vi "UHR-Fleezers Control (host) -Leonardo 04-2018 V6_DESTROY.vi"() -> ()   [LabVIEW 2013]
uses:
  <vilib>/Utility/miscctls.llb/LVPoint32TypeDef.ctl
  <vilib>/Utility/miscctls.llb/LVMinMaxIncTypeDef.ctl
  <vilib>/Platform/TimedLoop/XDataNode/timing_clust.ctl
  <vilib>/Platform/TimedLoop/XDataNode/nitl_modes.ctl
  <vilib>/Platform/TimedLoop/XDataNode/wakeup.ctl
  <vilib>/userdefined/High Color/nirio_resource_hc.ctl
  <vilib>/Analysis/baseanly.llb/Mean (DBL).vi
  FPGA VIs Alex/Alex subVIs/Downsample1D.vi
  FPGA VIs Alex/Alex subVIs/Integrate1D.vi
  <vilib>/FPGAPlugInAG/PCIe-7852R/niLvFpga_Open_PCIe-7852R.vi
  <vilib>/FPGAPlugInAG/PCIe-7852R/niLvFpga_Reset_PCIe-7852R.vi
  <vilib>/FPGAPlugInAG/PCIe-7852R/niLvFpga_Run_PCIe-7852R.vi
  <vilib>/FPGAPlugInAG/PCIe-7852R/niLvFpga_Close_PCIe-7852R.vi
  <vilib>/Utility/error.llb/Error Cluster From Error Code.vi
  <vilib>/rvi/errors/niLvFpgaAdjustHostInterfaceError.vi
  <vilib>/rvi/interface/common/niFpgaWaitOnOcc.vi
  downsample 1D array - double.vi
  <vilib>/express/express analysis/Spectral/Block/exnSpectralBlock spectral measurements PSD poly.vi
  <vilib>/express/express analysis/Spectral/Block/exnSpectralBlock spectral measurements PSD WFM.vi
  <vilib>/gmath/statdist.llb/Exp Random.vi
  <vilib>/gmath/statdist.llb/Gamma Random.vi
  <vilib>/FPGAPlugInAG/PCIe-7852R/niLvFpga_Abort_PCIe-7852R.vi
  openfpgaref.8.6.ctl
  <vilib>/Platform/TimedLoop/XDataNode/XDataNode.xnode
  <vilib>/rvi/interface/nirviOpenFPGA/nirviOpenFPGA.xnode
  openfpgaref.initrf.ctl
  FPGA Bitfiles/UHR-FleezersInst_FPGATarget_intitializeRF201804.lvbitx
  <vilib>/rvi/interface/nirviMethod/nirviMethod.xnode
  <vilib>/rvi/interface/nirviCloseFPGA/nirviCloseFPGA.xnode
  FPGA Bitfiles/UHR-FleezersInst_FPGATarget_UHR-FleezersCont_IqK95Pvv9lYv5.3.lvbitx
  <vilib>/rvi/interface/nirviReadWriteControl/nirviReadWriteControl.xnode
  <vilib>/express/express analysis/Spectral/XNode/ExpressSpectralMeasurementsBlockNode.xnode
  <vilib>/Platform/TimedLoop/XDataNode/XDNodeRunTimeDep.lvlib
  <vilib>/Analysis/NI_AALBase.lvlib
  <vilib>/rvi/errors/niLvFpgaMergeErrorWithErrorCode.vi
  <vilib>/gmath/NI_Gmath.lvlib
  <vilib>/FPGAPlugInAG/PCIe-7852R/niLvFpga_ConfigureFifo_PCIe-7852R.vi
  NiFpgaLv.dll
panel:
  in  "Reinit Valve?":bool=TRUE
  out "Data Period (s)":dbl=1.4999999999999999e-05 caption="Trap Data Period (s)" format="%#_6p"
  out "ideal setpoint fpga":dbl
  out "ideal setpoint avgd":dbl
  out "Step duration":dbl
  in  "Number of steps":i32
  out "Step taken":dbl
  in  "Distribution":enum16{"uniform", "Exponential", "Gamma2"}(ring)
  in  "Mean dwell time (s)":dbl=0.001 min=0.001
  in  "Backtrack probability":dbl min=0.0 max=1.0
  in  "Simulate stepping":bool
  in  "Step size (nm)":dbl min=0.0
  out "Actual setpoint":fxp<+/-,16,1> format="%.16g"
  in  "Target Force (pN)":dbl=10.5
  in  "MCL Tracking":bool
  out "Current Trap Delta":dbl=20.03845214843774
  in  "Set SP to Current Frc":bool
  out "Trap X (AI1)":T1={"Trap 1"=0.030792236328125, "Trap 2"=-0.011322021484375}
  in  "Trap Pos FB SP":fxp<+/-,16,1>=0.231353759765625 caption="Setpoint"
  in  "Trap Pos. FB ON":bool
  out "Extension":waveform(dbl)(graph)
  out "Action (%)":dbl(knob)=-100.0 scale=-100.0..100.0
  in  "Trap Pos. FB Out Scale 2^n":u8=23 caption="Action Scale"
  out "Location path":path=path "C:/Users/Fleezers/Desktop/UHR-Fleezers Instrument - Charlie/Locations.txt"
  in  "Location Matrix":string[][](array[string])=[["N.D.\r\n", "N.D.\r\n", "N.D.\r\n"], ["N.D.\r\n", "N.D.\r\n", "N.D.\r\n"], ["N.D.\r\n", "N.D.\r\n", "N.D.\r\n"], ["N.D.\r\n", "N.D.\r\n", "N.D.\r\n"]]
  in  "Tab Action Shortcuts":T2(tab)=enum."Calibration"
  in  "Use Full Offset?":bool=TRUE
  in  "Take Stepping Data":bool
  in  "Cap 1 Flow ON":bool=TRUE
  in  "Move Cap. 1 (DNA Top)":bool
  in  "Cal/Data Acq. Spot":bool
  in  "Cap 1 T ON":bool=TRUE
  in  "Cap 1 Samp Flow ON":bool=TRUE
  in  "Offset 2 Set":dbl=2.0
  in  "Offset 1 Set":dbl=1.0
  in  "Cal @ (MHz)":dbl=20.0
  in  "W/ Offset 1":bool=TRUE
  in  "Offset 1 Start (MHz)":dbl=13.0
  in  "W/ Offset 2":bool
  in  "Offset 2 Start (MHz)":dbl=16.0
  in  "Pause at Closest Delta (s)":dbl
  in  "Move to Delta 2 (MHz)":dbl=41.0
  in  "Attempt Limit":dbl=30.0 caption="Limit"
  out "Attempts":dbl=1.0
  in  "Wait Before Save (s)":u32=1
  in  "Fish for Tether":bool
  in  "Closest Delta (MHz)":dbl=13.0 step=0.25
  in  "Stop F (pN)":dbl=10.0
  in  "Then...":string(combo)="2"
  in  "Move to Delta 1 (MHz)":dbl=15.0
  in  "Tether Alarm?":bool=TRUE
  out "Tether":bool
  in  "Raster Set Upon Tether":u32=1
  in  "Save at end (5, 6)":bool
  in  "N Steps":dbl=20.0
  in  "Step Size (nm)":dbl=0.34
  in  "Save ave factor":dbl=1.0
  in  "APD to Watch":bool
  out "Duration (s)":dbl
  in  "Action":string(combo)="Yank"
  in  "Fl. Triggered...":bool
  in  "Fl. Delta Thresh. (kHz)":dbl=0.6
  out "Waiting":bool
  out "Fl. High":bool
  in  "Yank Delay (s)":dbl=3.5
  in  "Yank to Delta Array (MHz)":dbl[](array[numeric])=[16.3, 15.85, 14.85]
  in  "N Array El":u8=3 min=1 step=1
  in  "Random Choice":bool=TRUE
  in  "Force Yank":bool
  in  "Force Reset":bool
  in  "Toggle AFish":bool
  in  "Extend Min F":dbl=1.0
  in  "Extend Min TD":dbl=8.0
  in  "Extend dTD":dbl=5.0
  out "AF Time":u32
  in  "Wiggle time":dbl
  in  "Wiggle TD":dbl=1.0
  in  "Max TD":dbl=15.0
  in  "Min TD":dbl=8.0
  out "Fish Status":u16(ring) items=["Off", "Approach", "Wiggle", "Extend", "Tether Found"]
  in  "Approach dTD":dbl=-5.0 format="%#_13g"
  out "Messages":string="5:58 PM\tUHR-Fleezers ready.\r"
  in  "Stop All":bool=TRUE
  in  "Tab Control Display":T3(tab)
  out "Force-Extension":cluster{"Y":dbl[], "Y":dbl[]}(graph)
  in  "APD 2 Offset":dbl
  in  "APD 1 Offset":dbl
  out "Mean":dbl=1.039039384389187 caption="Mean (pN)" format="%#_3g"
  out "Force":waveform(dbl)[](graph)
  out "APD Chart":waveform(dbl)[](graph)
  in  "Calibration":u16(ring)=2 items=["None", "Position", "Force"]
  out "T1 X":dbl=-1.511158478291593 caption="T1 X (pN)" format="%0.2f"
  out "T2 X":dbl=0.5669202904867809 caption="T2 X (pN)" format="%0.2f"
  out "Difference":dbl=0.9442381878048121 caption="Difference (pN)" format="%.2g"
  in  "Ext Offset (nm)":dbl
  in  "Rescale on Mean":bool
  in  "Take Detection Laser\nImage":bool
  out "APD 2":T4(plugin-control) caption="APD 2 (Cy5)"
  in  "Flip Green Filter":bool
  in  "Set X Only":bool
  in  "Set Y Only":bool
  out "APD 1":T4(plugin-control) caption="APD 1 (Cy3)"
  out "Detection Laser Y":T4(plugin-control)
  out "Pointer Y (V)":dbl=4.0025870540482815 format="%_3g"
  out "Pointer X (V)":dbl=4.635613485356835 format="%_3g"
  in  "Set Confocal Spot (X-Y)":bool
  out "Detection Laser X":T4(plugin-control)
  out "All Signals":waveform(dbl)[](graph)=[{"t0"=timestamp(2751.0000000002074 s since 1904-01-01), "dt"=0.02, "Y"=[0.0, 0.0, 0.0, 0.0, 0.0, 0.0, 0.0, 0.0, 0.0, 0.0, 0.0, 0.0, 0.0, 0.0, 0.0], "attributes"=variant("NI_ChannelName"=variant(string "APD 1"))}, {"t0"=timestamp(2751.0000000002074 s since 1904-01-01), "dt"=0.02, "Y"=[0.0, 0.0, 0.0, 0.0, 0.0, 0.0, 0.0, 0.0, 0.0, 0.0, 0.0, 0.0, 0.0, 0.0, 0.0], "attributes"=variant("NI_ChannelName"=variant(string "APD 2"))}, {"t0"=timestamp(2751.0000000002074 s since 1904-01-01), "dt"=0.15, "Y"=[-0.020049210394969354, -0.02003592505550746], "attributes"=variant("NI_ChannelName"=variant(string "T1 Y"))}, {"t0"=timestamp(2751.0000000002074 s since 1904-01-01), "dt"=0.15, "Y"=[0.03074231675925172, 0.03074526419399293], "attributes"=variant("NI_ChannelName"=variant(string "T1 X"))}, {"t0"=timestamp(2751.0000000002074 s since 1904-01-01), "dt"=0.15, "Y"=[2.9160941496017294, 2.916128360850853], "attributes"=variant("NI_ChannelName"=variant(string "T1 Sum"))}, {"t0"=timestamp(2751.0000000002074 s since 1904-01-01), "dt"=0.15, "Y"=[-0.002644972968316131, -0.002638961391604115], "attributes"=variant("NI_ChannelName"=variant(string "T2 Y"))}, {"t0"=timestamp(2751.0000000002074 s since 1904-01-01), "dt"=0.15, "Y"=[-0.011335016186436862, -0.011341032214389745], "attributes"=variant("NI_ChannelName"=variant(string "T2 X"))}, {"t0"=timestamp(2751.0000000002074 s since 1904-01-01), "dt"=0.15, "Y"=[2.746599475081634, 2.746642933439132], "attributes"=variant("NI_ChannelName"=variant(string "T2 Sum"))}, {"t0"=timestamp(2751.0000000002074 s since 1904-01-01), "dt"=0.15, "Y"=[-0.526083166086966, -0.5261552546492463], "attributes"=variant("NI_ChannelName"=variant(string "T1 FB X"))}, {"t0"=timestamp(2751.0000000002074 s since 1904-01-01), "dt"=0.15, "Y"=[3.0920304879909737, 3.0920243537705665], "attributes"=variant("NI_ChannelName"=variant(string "T2 FB Sum"))}, {"t0"=timestamp(2751.0000000002074 s since 1904-01-01), "dt"=0.15, "Y"=[-0.7128125059590501, -0.7128388598091219], "attributes"=variant("NI_ChannelName"=variant(string "T2 FB X"))}, {"t0"=timestamp(2751.0000000002074 s since 1904-01-01), "dt"=0.15, "Y"=[2.9122738731040343, 2.91227808465834], "attributes"=variant("NI_ChannelName"=variant(string "T2 FB Sum"))}, {"t0"=timestamp(2751.0000000002074 s since 1904-01-01), "dt"=0.15, "Y"=[-0.0023344523453474137, -0.002339854121524665], "attributes"=variant("NI_ChannelName"=variant(string "PSD Y"))}, {"t0"=timestamp(2751.0000000002074 s since 1904-01-01), "dt"=0.15, "Y"=[-0.0026477858821374683, -0.002642139957884409], "attributes"=variant("NI_ChannelName"=variant(string "PSD X"))}, {"t0"=timestamp(2751.0000000002074 s since 1904-01-01), "dt"=0.15, "Y"=[0.014415417950986964, 0.014429639576402777], "attributes"=variant("NI_ChannelName"=variant(string "PSD Sum"))}]
  in  "Signals to Plot":i32(listbox)=9
  out "Trap Disp. Freq. (Hz)":dbl=6.666666666666667 caption="Freq. (Hz)" format="%#_6p"
  out "Display Period (s)":dbl=0.15 caption="Period (s)" format="%#_6p"
  in  "Trap Disp. Downsample":i32=10000 caption="Downsample" max=20000
  in  "APD Disp. Scale":dbl=0.1 caption="Scale (Divide,\nfor above plot only)"
  in  "APD Disp. dSamp":i32=2 caption="Integrate" min=1 max=30 step=1
  out "APD Display Freq. (Hz)":dbl=50.0 caption="Freq. (Hz)"
  out "APD Display Period (s)":dbl=0.02 caption="Period (s)"
  out "FFT 1":cluster{"f0":dbl, "df":dbl, "magnitude":dbl[]}[](graph)=[{"f0"=0.0, "df"=16.666666666666668, "magnitude"=[-331.1367572010275, -79.05506245821404, -86.61411242440559, -88.4728176091699, -90.3181253945935, -94.12566333707997, -92.52740723119955, -94.92192587982518, -99.60936585245742, -96.87568627870715, -94.02570383337763, -83.8058550151726, -97.57441397235512, -101.59968530846606, -101.523049255742, -103.35038532190343, -101.58594091014982, -102.96098031851216, -91.39759462745924, -103.75019963279499, -104.45030075054324, -103.04245334279298, -104.0720279134107, -106.06482372394834, -103.69131867828104, -104.40395035115309, -105.96420043276396, -107.6735556337804, -106.673030006608, -107.34889066208132, -108.05626565233933, -106.25659018850432, -105.29934513380842, -105.43096056709592, -108.3728498841465, -106.0555440144992, -105.78001282181421, -107.48741857324953, -108.67624970548897, -105.39976667156175, -105.91413119232612, -109.4222808198164, -107.0898971593174, -107.91164191890915, -108.26032038855709, -107.58332347164534, -108.23559688234297, -108.01271040303237, -107.66511723652701, -106.51901583170391, -109.27249501469946, -108.55647681594805, -107.93499259231463, -107.05068166453935, -109.13641475410455, -109.29679733781423, -108.19360835527803, -109.57747591546632, -109.58364591011674, -110.47061433372711, -109.8144340420426, -108.79067462293897, -107.54887553357234, -107.99559866705923, -108.85023923652685, -109.68733225238618, -108.51101278437793, -108.51620475114115, -108.22212402200637, -104.63726950302143, -110.2989919678048, -107.61796444414897, -108.68882962798736, -104.79193983043893, -103.59504263746938, -93.64633660288543, -101.9191640501395, -105.73717393151816, -108.92572458793902, -107.43962662800902, -107.79595323081325, -107.0923101993207, -108.17603277205289, -107.87074270713183, -109.20899066381877, -108.61832060412445, -109.10072003106593, -105.76480632823524, -108.60877649218978, -109.67541158970121, -110.2286232768028, -109.84952155309578, -109.33772024076384, -109.95251642394683, -110.14777282585466, -109.13825677905699, -110.05989365698167, -109.39359990189426, -110.56255614635295, -109.66477183197163, -108.9397158528824, -110.26529907650465, -109.20049464984628, -108.20183857013548, -109.09752250184418, -108.00440442238454, -108.35465963524055, -111.16774134451799, -110.34812550238405, -108.94506763426756, -108.72845542102493, -109.41512344014713, -112.44661664432377, -110.35437330889101, -111.32939440655925, -109.42989530434981, -110.98084669076195, -111.92160561143541, -108.57755551751093, -111.40042616180912, -110.15284955891853, -112.21455132279115, -111.40787773511747, -108.82949641635288, -110.13442122547907, -111.42229298204664, -112.06314940885191, -110.6015308813694, -109.51144097251623, -111.15989713761475, -110.25535755335385, -109.65868178057926, -110.51649885452997, -109.77194745285269, -108.4234206864394, -109.50892632093968, -109.46471287444389, -107.92241289271415, -109.72283805386196, -108.63426821579918, -110.37316681536255, -111.09713996884652, -110.32903619589223, -105.32012665515045, -107.36858557554393, -108.00382215905725, -110.06430686942338, -108.81666625979916, -110.01277074453823, -110.94194741225512, -109.65934609082873, -107.80979136006962, -112.81333866824724, -111.61474300955487, -109.83998277184975, -109.45953946904639, -109.79640584952526, -108.19172301667324, -109.28894656674316, -107.61471301278785, -108.83814006090513, -109.08866847726084, -108.20250571862371, -107.96222236861584, -107.03811197900873, -108.93533000393974, -107.74482548035408, -110.79811544577694, -111.1387476496877, -107.42970105883512, -109.18442281176472, -108.73546184641192, -108.71800246690864, -108.51945944378063, -108.06825856571285, -107.27210712368412, -108.12304695877637, -107.84933283677306, -109.73682373154998, -109.32284761503395, -109.31328817453769, -106.68762108642842, -109.79203616876461, -109.9020278896408, -110.27080024357275, -108.54152101558762, -111.00464391726017, -112.42244020766577, -110.82707315747889, -111.00344011890857, -109.90461839395674, -109.42877207451863, -109.73549298167016, -111.67494793393293, -108.85799077901427, -108.5348443278263, -109.803781083881, -108.30644755543659, -108.5079527456017, -111.2055351312823, -108.53089994340155, -108.01739789012176, -108.70360662855235, -107.95873456794631, -109.58297170693093, -108.9372401694271, -110.15921663527153, -109.22399119911955, -110.89883651739237, -108.92840112258382, -110.0545300523626, -109.05961065387005, -109.45831398589371, -108.61239387653227, -110.13001256174265, -108.80060224137931, -109.46327400696283, -108.0177965824709, -109.29727944627197, -110.3237255895986, -109.03258262543821, -110.97880178489321, -109.70034895077919, -111.16405638194153, -109.17324451464711, -109.65698250854277, -108.96750235822178, -112.00534231585624, -108.69274607723942, -108.98110446396657, -108.40723795464795, -111.44459094807324, -111.74799245277113, -111.1601960491512, -108.92048232753773, -110.30506377784799, -111.33145973979093, -110.91850998672503, -110.33684985776448, -108.90206518366908, -109.28458878227542, -108.98773986023751, -110.85813863075646, -109.00041591105906, -110.84543686681204, -109.84382395806176, -109.69722434763266, -108.50915601095721, -107.80829925826895, -110.59736107582401, -109.75377770317087, -109.3992084496136, -110.51151565846742, -112.49753959826434, -109.7299632589479, -109.54070743868353, -109.90314341132164, -111.05974202976806, -109.03766862152392, -109.46667095459878, -109.52800799036197, -111.3163121356807, -110.07817134522178, -108.69251657453547, -109.40472158898045, -109.71400709815576, -110.60534468715097, -109.46937396724682, -107.70342491418788, -109.86331122597839, -108.64971387994616, -110.90117371097081, -108.34928840565928, -110.04172889660904, -111.52979926554961, -110.34759300823305, -109.62712781837159, -109.24131154553284, -110.23196152450447, -108.68509612326807, -108.0246905483419, -106.61876139289784, -101.5519630114271, -80.57695480953835, -102.03744443354402, -107.1449217193017, -110.0695213407169, -106.61597783999268, -110.79221011808191, -109.58974545931426, -109.1149802216988, -109.20993813088597, -109.63768480465863, -110.10428394219181, -109.08445084271477, -108.83472375362581, -109.69508502050168, -108.05588796178941, -110.62586360101581, -109.95315261676905, -107.52208264977473, -108.80708007514875, -110.43484881098874, -110.45942171588936, -107.83804717866751, -109.98973910294193, -109.3496496054193, -108.425252911127, -110.94579264380809, -108.54181722177951, -108.67696070083541, -108.4150202151644, -109.24973583101504, -112.0454922608961, -111.29046597340738, -110.75018248960077, -109.38326363603683, -109.2033340336957, -109.45076170874889, -109.52878049853727, -109.32340869724774, -110.98123395128233, -110.75736340635505, -109.7218385823809, -107.97422606064993, -109.77313701758703, -110.95948744392717, -110.08996774172691, -108.51011830110778, -109.78063140243836, -110.65996628628228, -109.83684298615616, -110.33329049188029, -110.13755118968292, -110.3717925645783, -108.55302219178951, -106.86811628734195, -108.6302156589162, -108.75341391045045, -108.32589578384841, -108.70061474734084, -112.30742263527534, -109.16842570592085, -109.29767035534508, -108.87829025017463, -108.2255616391397, -108.4316108616088, -108.82995906929271, -110.40135575415563, -109.51623498946435, -109.79409808792403, -107.03832759632121, -108.36534528684132, -109.72010868372905, -107.90933028179892, -106.95643597294047, -111.29929166165778, -110.23001135794706, -108.98838015381585, -109.79115357104436, -108.18627479511115, -108.14988122174307, -109.12074063466532, -109.41904850488358, -111.40409873721113, -108.83156790193294, -108.77032248953847, -108.88363158686694, -108.47515048290681, -105.94172147874599, -109.38146940214403, -109.21277078848794, -108.11309390545507, -110.70840012427504, -109.5504457849329, -109.52330684534209, -110.06776026911132, -108.21949434182314, -111.21266686269992, -108.78581501170974, -108.43115799297222, -109.63260325780062, -109.84070220619535, -109.72041980780126, -110.29615941882527, -110.60316734262464, -108.79165446414692, -110.95840439895592, -109.64926233107009, -109.16526769544322, -108.65292362430982, -109.56113898129935, -109.85693046339026, -108.92316027325207, -109.79492493553914, -109.38157962945887, -110.24545136266825, -109.30031463492487, -109.0795429936869, -111.4091719525013, -108.63499083917162, -108.43863465339358, -109.23207864880891, -111.21947487191643, -109.24525201480154, -109.56842406077318, -109.46711940800672, -111.91389548262572, -108.15655736690546, -108.71882059966947, -111.26328503478568, -110.95027143873176, -108.4853106242357, -110.36902802777546, -109.9314203579182, -108.77686164101732, -108.71871020068312, -111.04829661168574, -109.95072655339462, -109.88221342875462, -109.53241732756136, -108.2625005404823, -108.00677030040697, -110.19659317581693, -108.93858924796267, -109.46817875483995, -110.78063992017232, -111.11066570318451, -110.78774336696706, -109.19199744617812, -108.54914256407436, -109.28414960420909, -110.64143585101183, -110.5855350821307, -109.47578632252726, -108.89705360836223, -109.89214013612292, -107.93271261027171, -109.32631601340563, -108.60274611341092, -109.40110159872573, -110.889237682208, -110.01391165813328, -109.99747108785071, -108.65542819213674, -110.37211847668736, -110.44656500845738, -110.8128133834973, -108.8909299260433, -110.19551227077532, -111.37647266643523, -110.83802189730321, -109.98519377913681, -110.52378970770522, -108.16970420057817, -110.70974729773344, -110.76836765494402, -110.26884275594577, -109.22041044268806, -109.87809744746195, -107.76823252107832, -109.12119474042969, -110.28066108731146, -108.55000033509207, -110.18152097767907, -110.73030521152278, -111.49470908029893, -110.2320929919509, -110.03370979233021, -109.79181668155233, -108.6673501209991, -109.86695766650877, -107.88926518046961, -110.95525003776572, -109.18130359755742, -110.42618009658618, -107.90341931158893, -111.44736855661769, -110.72634267386593, -109.29945988519303, -107.67889101961411, -108.81148059987765, -109.13375212757057, -109.8122873383549, -109.80176697684155, -109.96342275204768, -109.90406635707086, -108.75674342748256, -110.12362902701081, -109.82151095527837, -108.62543344241836, -110.09171852771195, -110.21434637862887, -109.97254504855631, -109.27043209093468, -111.35149588204125, -110.12399876776051, -111.65983675538546, -109.28788875768564, -110.86554069990251, -111.26990906470603, -108.60956517491746, -111.49613890850938, -111.79685722966795, -109.26269485364045, -110.38555615546439, -109.40641023162068, -110.966136593156, -108.78892524584494, -110.29340727375603, -111.44032043281035, -109.95212021173755, -109.79233511584334, -112.41184021118175, -109.73687851881148, -108.65493879781806, -110.76132988919045, -108.43230346094671, -110.32968175895853, -110.29890782023821, -108.77609076424456, -110.3298662333555, -109.47734504217333, -108.2677295732245, -109.21234363352882, -107.83278941978479, -108.85136784424789, -108.43241251530755, -109.76609391460555, -108.53204373005357, -110.9660641972934, -110.3152512161094, -110.72570499399905, -109.23877906286317, -111.72407743101837, -109.20311421918561, -108.06021800233717, -109.29288625761943, -108.78395253409145, -111.85250172876302, -108.78827588901797, -109.79775055719482, -109.12089297455859, -109.49896359356035, -110.34432647103819, -107.94700097960238, -109.30489238477631, -108.89170290869342, -108.82574563272509, -110.11024077194833, -107.37946433552314, -109.60167933458756, -107.80625057819019, -110.11489057210264, -107.35436859378505, -105.69819484613895, -109.11280625683739, -109.27770293057978, -107.7053735252589, -109.75022444894368, -109.3310543596577, -107.87683693707739, -108.19931495338068, -109.26462246191564, -106.71885779297867, -100.00018022217961, -92.54434511397295, -107.20472143807373, -107.39203415155283, -110.04461177268398, -108.48860496315312, -109.0057168110333, -108.37627790492552, -108.4108380728248, -109.65509454313073, -109.64243000632982, -97.04219069306761, -109.0928856629964, -107.9760697315632, -107.52611064047497, -108.87702814778996, -109.08437599027614, -110.70097118837974, -109.00969860961283, -110.38275386163214, -110.0699155421545, -106.91498895181175, -106.22178738309017, -109.36827866896039, -107.59953130968307, -109.19516217272808, -108.31502495393616, -109.384158926223, -107.11670654202719, -108.09436312738853, -110.14559230873704, -109.84997663447679, -107.83465335309926, -108.60947100624459, -108.9932479423645, -109.17174810371898, -108.79457339828916, -109.40909327982367, -109.6328723628302, -109.51081854476179, -107.63054408568418, -109.63728404010122, -108.51163794839918, -107.55002282725216, -108.97796212764939, -107.24648164623483, -112.21470452291085, -108.74294024554423, -109.62070777514892, -108.05768666239368, -109.8224946685739, -109.34575507446003, -108.53536952609525, -109.60789300457671, -107.56681538208278, -109.22777325016398, -108.79047910308894, -110.10332477250668, -108.00206387955672, -108.45604004720035, -109.00645795765472, -109.81039564269616, -108.92785144634745, -108.3978471520567, -107.94411095685999, -110.53486519304262, -108.8773780319227, -109.03345093296107, -107.30746693745031, -108.54277704832029, -108.77629108166091, -108.91111762599647, -107.74965195880401, -109.97375370738439, -109.76326492689246, -107.91717581777407, -109.0730556927617, -107.66804873204664, -110.40438871064791, -108.05794247751498, -108.80206615156494, -107.51329354700796, -108.83687012994949, -107.57713176895379, -107.94774159581414, -109.41894615439651, -107.10869425078764, -110.51480854078629, -108.92221367099775, -109.91358786461535, -110.1744263092835, -109.30795472883494, -107.91359710691006, -109.77888185049835, -109.52060975706438, -108.66686651982212, -108.71041801553639, -110.13619546359467, -108.87957097273856, -109.72150387215271, -109.00776068810654, -109.70251113927438, -110.75769213896399, -108.53234896741436, -109.69439526582246, -110.15412541604617, -108.25183374628219, -107.97402569656481, -110.34920156998648, -108.45106995186384, -108.82031145748209, -111.38690005057539, -107.01968459818563, -110.3044500039584, -110.8755481852125, -111.08915057663255, -107.94824988655199, -110.21669144934839, -109.90539774633154, -109.58985438756767, -110.12258796623348, -109.41689951612143, -109.31128210476795, -109.00258476567323, -109.11093063041056, -108.83347064311234, -108.32685287566952, -109.44770946560935, -108.40145063144861, -109.68448193892085, -108.76525439243828, -107.62837139034596, -107.39300298848994, -109.36993934990318, -109.2465218489418, -106.66307369796812, -110.15891092764934, -109.57151745419041, -108.92425698310808, -109.8036704717834, -108.79751146756549, -109.25926431818017, -108.46260574057584, -109.1967554647261, -110.63319560262356, -109.02343067385144, -111.22073171487528, -109.4731095097105, -109.69335000085164, -109.48782989577005, -107.95204227683271, -108.19468255763758, -111.36195112053247, -109.55696116543685, -110.3130767640534, -108.9621824253354, -109.99735074896789, -109.20198058456344, -108.12100614259485, -111.27227490807289, -110.09248554008288, -109.14395535060149, -110.80882692379708, -109.22632926901655, -108.64497210802793, -111.00030482190711, -111.1317849358033, -107.43140429257826, -107.9783302193555, -109.2639893652291, -108.97008485446163, -108.66556668859064, -108.12995785876932, -109.73001061107855, -108.09691302413727, -110.68391499215569, -112.78583642012705, -108.7093037763389, -110.67868795924797, -109.0190959349128, -108.36247198231372, -109.82829353258869, -108.24916379311045, -109.84154533905823, -108.55470160833775, -109.75438989348815, -108.82865632118325, -107.63622268162582, -111.00943492886312, -110.81824358463759, -109.46028423652966, -107.52479398900992, -108.99087806823736, -109.94494831750349, -110.26788355564504, -109.8954055022304, -106.9478122391182, -108.91705388158901, -107.76095584490312, -109.28456723055147, -109.7982307261767, -108.98552661346622, -109.98937979783426, -110.57907422426224, -108.68113463944836, -108.06257240208589, -110.0707224529617, -109.19515280354733, -109.35868842818849, -110.37311467065695, -109.0404734478992, -108.16686395270187, -108.61859220485148, -109.19986437876149, -108.19707189725302, -110.06564239663074, -108.87850403465154, -110.63824157544798, -107.36918104067212, -108.7008736325543, -110.9359398265406, -111.08529123080929, -108.44209934821818, -109.79529621208783, -108.38917887958179, -108.169117639508, -109.24332926356216, -110.50584058811704, -109.63592524002665, -109.32261039377495, -109.16720880524552, -109.3084314664462, -109.5812223978583, -107.70213196487856, -108.0557884982431, -110.67058020007828, -111.68459781023608, -109.66270627185824, -110.52536245663693, -109.70208409132103, -108.78645420809342, -109.23122088059863, -109.24601474121832, -111.25604763816514, -109.50225851581177, -107.32434217163818, -109.28548556764925, -107.59972621660836, -110.46928774723048, -109.25950101547609, -110.32016453935465, -107.78482761561703, -107.89462895091089, -107.51366154391481, -108.08036891159172, -109.53371809947035, -101.2452927166745, -109.32763325689056, -107.52166868423687, -109.89648659445174, -109.11350200980485, -109.81336712738089, -110.02799517445062, -108.02767143538516, -107.97850220501483, -109.50772934896838, -109.31069875721964, -108.49991657749598, -105.60880911233095, -109.79128597340213, -106.91084537903113, -107.84880087118997, -109.63628170511824, -109.03203967193224, -110.64186113413658, -110.98027990365594, -112.33841002907062, -111.01793075565425, -108.58025797022215, -110.4259296883756, -110.38643255981424, -108.93051671115133, -110.97544177116494, -108.63883100482677, -108.37581711765226, -108.90240163126536, -107.94688047875466, -109.9482937437732, -110.09097112364414, -110.09805032265376, -111.44307114024532, -109.15483789122554, -110.9713708217832, -107.8548737634672, -111.41418477109195, -109.45699779859628, -97.03595099331734, -109.16746744169623, -109.66209204485918, -112.57048704774604, -109.73989735035725, -108.16252575067017, -110.7546980664636, -108.91536673403449, -109.20509151422344, -111.0260632167785, -109.62924582406518, -110.45466277291722, -110.2973970018937, -109.67550222925419, -108.84481022020094, -107.23686414357573, -111.79004633370906, -109.85453094194085, -109.45617270081004, -110.73920606732504, -108.90879956851099, -109.67774425528265, -109.4745715721361, -110.18080454693559, -109.26079184315502, -109.41692499885505, -109.02240975088358, -107.80833423058168, -109.32657361431549, -107.87138278655101, -110.910364670719, -109.70067156846706, -108.55301754282077, -109.4243252157005, -109.77567725161107, -107.83737232063925, -110.36509412773016, -109.6371048811367, -109.49430894422814, -108.55509251499753, -108.03996302911446, -110.4385715838736, -110.08864436068788, -109.48922484379962, -109.90865554258562, -109.7491963238264, -110.04796094537969, -107.413043439116, -108.54229076126079, -108.2522516728666, -109.75464941327974, -110.26795832300996, -109.28073673851144, -108.62990200974927, -109.89408067552287, -109.09160284731726, -109.90740624925795, -109.92534708896517, -109.79578862362752, -109.97278346890566, -107.80679350393824, -112.81728446281548, -108.09689504419987, -109.89549991422173, -108.43930976031248, -109.95153099843282, -108.18277483720716, -111.89607792605433, -109.52567003805, -109.17125106979698, -109.64300739407085, -108.21045178846524, -109.64036472149706, -109.02324448538845, -109.039163008889, -110.41006510134076, -109.50289952116489, -110.4732620447796, -110.08777181504614, -110.15589511434341, -109.55705089158471, -109.2547682932589, -110.86823885471617, -109.96330502176939, -109.85995369810554, -110.63211290903473, -112.08007783432191, -110.24725218052279, -107.62861148917592, -110.08691795849435, -108.89793794632287, -111.07702220466341, -109.46946126482341, -109.19747345337464, -110.70018609416007, -109.66366205691908, -110.78032312133551, -108.05724200456513, -108.195661625627, -110.90724508408255, -110.08307674771669, -110.76863516643007, -110.46620425061583, -109.16986788877276, -109.61921294239114, -108.51159432329543, -109.96308336765689, -107.38178944242856, -111.95930944846394, -109.3329826827624, -109.59119636368249, -108.83148571828912, -110.46194288788257, -105.87694286145472, -107.985886302892, -109.2975019660806, -111.05138725716857, -109.60005889204612, -110.92871351729086, -110.73480546964537, -108.41587420326718, -109.84275465824477, -108.8249071047676, -107.65358887817105, -108.3254150042995, -111.47362100321767, -112.7287536850025, -108.8217125660507, -109.50232320231771, -110.29587061625348, -109.30644535112089, -107.69178032077258, -110.84522325672016, -109.3735891463141, -109.12506388923123, -109.65582307934665, -111.11427272192576, -112.19827973435466, -109.11306367925813, -108.19203577968261, -107.89831568266465, -108.85805249169313, -109.51100049661844, -111.71546684086955, -109.53880495724334, -107.07739286222231, -110.66836728754211, -111.5415170557177, -110.16051267940297, -110.6107546662698, -111.36389129556191, -107.77888179117923, -110.34160392509817, -109.61287125994414, -110.23791773883013, -111.00669159903549, -110.97165069538953, -109.43965413392434, -110.6813161690388, -110.31441293654314, -111.96129906273796, -108.15998218707462, -110.08095912053633, -109.41084567452768, -109.28774416263552, -110.80159950384204, -110.41956747809755, -108.85005186267244, -107.9069227847757, -108.84249369063123, -109.92569208845894, -109.34109797584448, -109.41334788055491, -108.76462023086997, -108.22069272136177, -107.0786679601274, -108.30206755098202, -108.57613406368954, -110.83330887636482, -111.93966942736989, -109.76373713473264, -108.25782074884941, -108.16490627215555, -109.93351470267982, -110.75525684428368, -108.22814762283093, -109.73442331991602, -107.53145627482685, -108.27195221226805, -110.33032779278457, -109.48951857415828, -108.12599093700939, -107.97627415508097, -108.81426859968796, -111.21764717894752, -109.80856212352333, -110.92658779118501, -109.71551885834796, -110.38682741010847, -108.87671328341361, -109.68368600774755, -108.35359806351899, -111.7519400010676, -109.89407081573103, -108.24301180922755, -110.00646944788126, -108.6685299083706, -107.52856885980722, -111.7622363038509, -111.0025144494897, -108.64719599357296, -110.62968467177518, -108.821509935539, -107.94915453463719, -111.53070432277694, -109.87282048586256, -110.71167589371663, -109.79225006081626, -109.96203471712074, -110.29921092232489, -110.10644439440416, -111.28815007382043, -111.19165661703703, -108.46024117100558, -110.22528296512183, -110.32184972386672, -110.05120383416072, -109.78792549362107, -109.00355659956696, -108.85989369286315, -113.00899556732638, -110.91756826567867, -111.25016866167897, -111.84225040552181, -110.54451635944174, -110.72722829912917, -109.60759702177283, -110.49362602516815, -108.74419542915284, -110.3379671069179, -109.66259088220754, -110.45956400953156, -109.13956157147233, -109.27130155486806, -110.83015602667983, -109.17970724944131, -109.09662765889193, -108.0447366108107, -108.9536269357457, -110.35663108940085, -108.73418835472056, -113.42965806805827, -111.81270536656905, -110.06155590173537, -108.76582224646269, -106.7488061675813, -108.5700320158723, -111.11038264410035, -110.41435767488723, -109.12763443489911, -109.30517580756394, -111.61251165371237, -109.8116632664339, -109.36845864976851, -109.00390009629231, -110.54359197165573, -109.52629258465976, -110.75932197632896, -109.50903215359567, -107.42652056246085, -107.81146496533543, -103.22224383145215, -108.53803076819163, -109.78623360072066, -109.66306634612869, -110.80245829141279, -111.87835085452016, -102.27372781471168, -111.27763038431458, -108.45838423437681, -108.79077917058028, -109.31951755762685, -110.05415097017186, -109.5535934823387, -111.62732254641111, -110.73478247119641, -109.9468722686683, -110.39698367573979, -109.30612942398305, -109.7578384694043, -109.34817295524313, -105.56944757301993, -110.1940418750125, -109.27076023513962, -111.03491935225027, -112.2980497521063, -110.65725497955563, -109.0567530102422, -110.31700596563523, -109.64508026365678, -109.6190471404421, -110.52566833759428, -109.68595899227789, -109.7431160985074, -110.4798230300751, -109.45506977604765, -110.69504157940786, -110.63067849573177, -108.06456949500138, -107.99354148885966, -108.11349194720599, -109.15944121207349, -110.61766925164031, -110.14145801314527, -110.67420842201165, -111.91532881806512, -112.15901550030345, -109.94774413630104, -109.2819568305201, -110.94623189179737, -110.17685430287735, -110.39082916961016, -109.53953238698966, -110.76940623620611, -109.89327922318515, -109.10275695043765, -110.21445972656734, -110.58968777252528, -110.57016757660259, -109.59208496373341, -109.07946946465374, -109.10762003745964, -110.36892993974607, -109.81864495218393, -112.12972189864566, -109.26185849434863, -111.56305819991357, -111.36019621828058, -110.3397604159226, -109.58675612753163, -110.58041217474447, -106.34739062044932, -108.6722699609389, -110.03906060709869, -109.16794717548382, -109.65012481802809, -109.35377624077988, -110.51889143862303, -110.03397458059777, -110.7981307056636, -110.56653507062292, -107.61367005067231, -109.99279736988825, -111.79875182878175, -108.60382315996031, -109.71381533228038, -108.60388131505613, -107.0933685540362, -107.86037690830757, -108.40980028847238, -108.83869602763895, -110.76921375395764, -109.96766364716046, -110.8256171465781, -110.13805084291067, -108.5349140035878, -110.57158437465219, -110.8920694413417, -108.71646695477324, -108.33274238445665, -108.96152108305608, -111.03750932994224, -109.48915027983756, -110.29725207211165, -110.79527247268442, -109.47969936716117, -109.79306701834035, -110.16840035577498, -110.29840230783668, -109.15306387075587, -110.72651274964761, -109.08881658764956, -110.8349724030761, -110.64653625576447, -111.40392562616867, -109.94581588927414, -108.85136340231294, -109.77228546607624, -111.48297395390018, -109.7334001251941, -109.30537415590783, -109.63937411233408, -109.69785848648013, -109.3523781030017, -112.04667421182404, -111.56311816195343, -108.18548447362308, -110.63388993686104, -111.39768634137992, -109.87157345395542, -108.6734208287271, -109.46213300216168, -111.75774769437145, -110.10245994173216, -109.52385139033495, -110.96513097775451, -111.8709319163154, -111.54948269614047, -110.29760900080463, -108.52168175904663, -111.09033925738258, -111.14752744054172, -108.83074523709202, -109.05704141259113, -111.74377805749482, -109.57200906899736, -108.84121318623825, -110.86657990204343, -109.54363603755047, -110.89448416316372, -109.58965570570145, -110.21012263847972, -110.4063470702923, -109.5021950342969, -110.33648801598177, -110.90551031296536, -109.69205870504638, -109.8648503154861, -110.28183391384131, -109.65970942950766, -108.43615680946908, -111.11790511866548, -110.89043476451553, -113.64898442872548, -113.08004494963895, -110.81525412051718, -113.91009875719509, -110.95802128672312, -110.40944585634135, -110.33464695414992, -109.98984645778987, -110.18795067005652, -110.62364351231234, -110.44029833291248, -109.01598585569788, -110.95430216511514, -109.77987141110621, -108.54452361812068, -111.41780266439777, -110.47172771858405, -109.06084635984516, -109.30794593246578, -108.8764083815745, -108.18222749506985, -110.31330487887435, -109.04176821738014, -108.8558386035048, -109.47888284507395, -110.01459604573937, -110.48596659065309, -112.6781342298378, -109.85522803775775, -109.0569534499285, -109.08991286548698, -110.89485727880403, -109.18715778948663, -111.50381433568144, -111.3545424730884, -110.07710926239977, -111.99977850157067, -109.47444853853723, -109.81605328527645, -110.74995213151195, -112.56834665925544, -108.52052472391404, -110.89121213995557, -112.02004142355113, -108.66413739656008, -111.10053848695652, -110.41241079991636, -111.80152991764473, -110.21746151515111, -110.63265128607344, -109.483042128511, -112.78639954059729, -109.47114195846122, -109.23309637902875, -108.97133643967169, -110.08909147812822, -111.01105271457081, -111.18602432128249, -110.04633990216801, -109.53453538673071, -108.81939452082017, -111.13486114285661, -111.65877073200598, -111.63763706753498, -112.14107810664572, -113.6231865196724, -109.31743865878806, -109.18551713085722, -108.74951309653638, -109.28206426212142, -112.36687029711229, -110.10933061193728, -111.29501093502684, -108.19021080564794, -109.34497312126749, -110.37228033937312, -108.63277512903049, -110.61033993911002, -111.2975761598062, -111.49780004751436, -109.91019436685814, -109.32789992989028, -111.4482538110117, -110.1538439123475, -110.66347034043578, -110.05055133068794, -108.53002033538341, -111.7522199783972, -113.49108651193104, -108.03793940563418, -110.07108694011555, -110.83958739865201, -109.62805629409038, -112.69637731014087, -109.57996950503268, -110.104850643722, -108.83376203949506, -108.69400304840181, -110.59434352922563, -110.69121011800921, -110.18694553784364, -111.90598571547098, -110.30230802494223, -109.66810649416752, -112.6017099000434, -111.00296745333219, -110.64462650261785, -111.4775358707403, -111.98753241268494, -112.26574909791167, -112.04796822399412, -110.65853064447325, -109.6623218025264, -109.40559579075378, -110.42174451813142, -109.18991987957241, -111.02050178263048, -112.77950487440032, -110.42443751566815, -111.35440372400903, -108.5263524245987, -105.07498063939795, -107.15444425741984, -110.4508720018025, -110.25163264819463, -111.1383261104107, -109.91171620173931, -110.52200560606038, -110.5299174299573, -109.34628087255733, -110.26101817411786, -109.65071853372183, -109.66953335961068, -110.83590602054682, -110.980546313788, -109.4110066989163, -111.47223607390256, -110.00281523859483, -109.4088722967626, -109.00401922839337, -109.59655302543185, -109.7359970854586, -111.46016206343049, -110.23478747568004, -109.29441275295858, -109.82941912510167, -110.43088525283673, -108.21649744751299, -108.70220592702613, -105.2334473604296, -110.60620657984927, -107.97533820921146, -110.7664079806058, -110.56406610911355, -111.76465470250328, -108.84172809688911, -111.03661078143631, -109.85351980370237, -110.70091167176791, -109.52380717508088, -108.4356492672842, -112.25498760397127, -110.69648730540193, -110.36748838594507, -109.99090797924349, -111.2678642544111, -110.42541694325627, -111.4575545259775, -109.3211175669008, -112.7465573314208, -109.56208667784249, -111.59733497772172, -109.42295730962105, -108.55804089331346, -108.71397903286748, -110.09188290952392, -108.90810063278326, -110.31333217069538, -109.69794714542728, -109.06210020835357, -112.42465112160288, -111.74630553904855, -109.99304310093493, -108.93867687355595, -113.1669287525049, -109.09193568851137, -109.27500368450697, -108.99643325722404, -110.53962759110647, -111.2052088429852, -110.05855563908841, -110.30763723153481, -110.03411001268613, -109.6161415052669, -110.6304714466923, -110.17116005754627, -109.0753171640551, -110.92564270851628, -109.60831770517053, -110.25913363817017, -107.76644895378317, -109.2619309023068, -107.64198246311884, -107.37056168314048, -107.31978563121643, -107.68171928702894, -104.57515288104209, -104.75187637758803, -105.27246893266054, -106.96524396060869, -105.93920355631757, -103.66449995825586, -104.08476660009461, -104.53081578265315, -103.0148493379086, -106.74751670818362, -104.92309629919443, -103.98320340724693, -104.81633219413234, -105.77996356028235, -107.12559309216644, -107.28196039053535, -108.84583578337953, -109.4494696919565, -109.15525441177898, -109.7634811359225, -110.79433338587495, -108.44440079452527, -108.79597700117748, -109.98590735173822, -110.72144284267539, -109.30550753718086, -109.70072152916897, -109.65801130162137, -109.65949265997646, -109.82238573025273, -110.30669821947491, -109.83394128869384, -108.90433312205332, -110.664046708231, -110.39926453734134, -110.37725911098757, -112.12508639032839, -110.26795666332589, -108.98741993218054, -107.76168841100478, -109.82334992872889, -110.83516363498563, -112.60649745671253, -111.1960726449926, -111.03919163866381, -112.05129034965563, -108.83187987662883, -109.57240688505179, -109.32857861150738, -109.54934849013647, -108.29359879300195, -111.5179112931669, -109.52702486426027, -109.95429980789645, -110.7011078611564, -109.43204524997455, -105.56031249677113, -107.70609254346495, -108.78303653454363, -108.11457060956113, -110.44215460317537, -110.78267897406572, -110.33119812901934, -109.34449539666907, -108.82636558484161, -107.1834151347969, -108.83808254322192, -108.2542825327446, -108.80298057862501, -107.59922121598055, -108.9131916496929, -109.51519107961856, -107.7704986323755, -108.79678029009878, -111.13791068210752, -110.402746275919, -111.31702623823912, -108.49812727557243, -110.63723264798182, -109.32890666586829, -110.29721723278237, -111.66560929315017, -111.04227698307153, -111.36927505376269, -112.5203298417673, -109.93967930487354, -110.14533835678606, -110.3868348991775, -110.85413569165249, -108.44519725537315, -107.93391978795047, -109.82778679299085, -109.79311153223738, -109.25261055399044, -111.47738679135526, -111.11775495397512, -108.65898844492045, -110.26505495390529, -111.02017977446526, -110.34817965403467, -107.55161094495372, -110.21667403085983, -112.43970497917284, -110.70535338255132, -110.79438078890512, -109.81809822502822, -108.99167960596515, -106.5556893069368, -97.51736665041192, -105.29926513345109, -108.72453297392224, -108.23203912463346, -109.50324111400698, -110.9939986929772, -108.05367524487318, -108.37339392211176, -109.8553291283933, -110.46179639493138, -112.48795697163695, -111.88145079973545, -110.8678969738583, -110.62677605624849, -111.83824818603244, -109.76798658735359, -109.6654742351465, -112.58543522753767, -110.3406716250781, -109.55013159400883, -108.00481229232405, -109.90793236599207, -111.28597960985334, -110.54144527494444, -110.14704702870655, -111.2652554338908, -110.97520848958668, -108.63647576273343, -110.52472680617548, -113.16137826273847, -109.62457037485827, -109.53869420402964, -110.71399284283449, -108.55435337782664, -108.09492728294455, -112.2373886856363, -110.3693019226993, -111.65116752865308, -111.3223986412311, -109.67734725401074, -111.36420709226297, -109.14293108556625, -110.5982939020188, -110.29596476096043, -112.69847120697035, -108.39052787054206, -109.06205229490357, -110.00045399262885, -110.71775009467346, -110.69530760167493, -112.54144940754935, -109.55755373438097, -107.88943697845929, -109.98578587243783, -110.14202980613851, -110.80051915904802, -109.11327182471621, -109.50637030500913, -109.77023677605327, -109.98552825925917, -110.40235854896, -109.37603004890141, -111.36989177909379, -110.8399811877331, -109.30394670937987, -112.2769814990538, -109.10893172594731, -109.17733972841754, -108.35968166480572, -112.64492569586005, -110.13779257328873, -110.64439690778532, -108.45446935516622, -108.97325006911116, -110.54637968933774, -110.66412364132371, -111.38627695224784, -109.8942998516069, -110.36392017322382, -109.92355133054227, -109.61886697310419, -109.71969465343778, -109.85627196259388, -112.1407808286419, -111.1013489416651, -110.70428953307596, -109.3454280179969, -110.22984684615578, -109.53826801613613, -107.83673208330934, -108.72742563398342, -109.5745872123195, -108.83031823548816, -110.89059911076627, -109.87842545384129, -109.21980161063786, -109.07140273870678, -109.04628915564135, -108.79255665097845, -105.20875397856382, -110.0838008881032, -109.68293832806683, -111.24644641302518, -110.01257579497496, -110.99281477454484, -108.99296184719546, -110.96495665514604, -110.70404386182749, -108.25078498739035, -100.77667501455139, -107.61479263900088, -110.06600976399395, -110.02035637581871, -111.45524052052504, -109.975541184397, -111.07333860975358, -108.4808974233161, -109.59513524582242, -110.74711589861774, -109.50005300854993, -105.23071652566294, -111.81094849223531, -109.0168079712372, -111.89029991620679, -109.90672274216391, -109.30959446424889, -108.23718655264584, -110.10868108588909, -109.21139771899594, -110.33333323577992, -110.25792318324204, -110.67825932924109, -112.33148517950511, -108.9724848367048, -110.78371843797613, -111.40913868573313, -110.2930522718577, -111.9538408094371, -108.63639312641844, -112.4462941079034, -110.40266356498321, -108.66617580940074, -109.44306834729083, -111.08962916641603, -110.52132608161017, -110.53757698855654, -111.5587344449704, -109.77722315102946, -110.40060629757771, -109.45395807961631, -108.77558572395142, -109.0151938598724, -109.80739619986889, -108.9332873172888, -112.49933978358132, -111.28667321897437, -110.40629082858706, -109.9829216820938, -108.85102919990373, -110.84179127037925, -110.27309817549309, -109.88857884367955, -112.24517967927224, -110.23377125710859, -111.26951227953063, -110.09782138347559, -109.77508406986834, -110.55359722398646, -110.09534729906368, -109.96333904888587, -110.29372855476366, -111.36651812163072, -109.97141184588116, -110.16701683369045, -112.8562627359291, -110.66651146857079, -108.78873821095968, -108.59208174618087, -110.31784275318834, -109.43177042415276, -112.80272887161644, -111.79874205007107, -111.08216899537892, -110.73699224045636, -111.04738767291953, -110.43395896705012, -111.62106163510778, -111.32599933330843, -110.29360981749807, -109.66562228449096, -109.21316193790335, -110.06363162177448, -110.54480468587292, -109.31791670875509, -112.65386492377107, -109.91857609999171, -110.57233605624137, -110.7597333064856, -111.49767138733276, -109.36548654843229, -112.34145274183716, -110.52831153822652, -111.55802243871352, -111.81399803046556, -110.17680125962372, -111.23811621944807, -110.48042049674514, -112.43786993562033, -109.56507357271987, -110.67030752598993, -110.86377249100713, -109.06001892813467, -111.37023727930494, -109.52881096984436, -112.95107295160436, -110.49467818026214, -109.29804210589607, -109.89270706931751, -109.46354468058833, -112.10350702955014, -111.06083529077077, -110.49996587015904, -111.1617248913634, -108.84725633199014, -111.42852695852422, -110.01433866707184, -109.11616968390972, -110.76961079765468, -111.80403513904453, -109.84442686379181, -109.65447921666167, -111.3378640555306, -110.8882647652338, -112.58014202075226, -109.67128881545659, -111.73429980763389, -110.82258070774773, -110.71895931098041, -112.5117489008152, -109.16182299471309, -109.71651258790612, -109.7770618808562, -111.94294809571427, -111.1629115541574, -109.57489224865171, -109.8402445779754, -111.17931450307283, -110.09045865447595, -109.23658206733491, -112.54929616847242, -110.5150381158864, -111.32296447909377, -111.64472156295191, -111.65832771066007, -111.03359562742956, -110.85303206770837, -110.80655337650862, -109.3712696310075, -110.57313454785879, -111.18525355670417, -111.67423695430561, -112.00829831274282, -111.08915434609605, -110.3298290221436, -108.68552957386795, -112.11377370993225, -110.80288297661977, -110.33640536217185, -109.5907971201988, -107.9195263775506, -108.50223113159429, -111.91191347156142, -110.29585599512956, -109.50902788911351, -110.76819145749467, -108.86899533416589, -112.09963049260891, -110.13374376572433, -110.15881393584463, -110.87392107947531, -109.18658540731009, -109.72734703956934, -110.18732487568724, -108.76554115185057, -109.94122289815374, -110.39583285609643, -111.09540935727229, -110.6618176357367, -111.6281345666718, -109.69686483639367, -110.31633402076315, -110.61246951748903, -111.73300235294965, -111.34221378834899, -109.46708370903485, -110.70412671997354, -110.7007891485379, -110.31685483435038, -111.03016917417074, -110.94517365625376, -109.46580797053619, -111.20935248224806, -109.20661126636224, -109.50147037097533, -110.14241781654353, -109.8510950344643, -111.3794198224028, -111.28966889207122, -110.43347441663424, -109.86759980279523, -111.92101892013198, -109.31594011390644, -112.92253433794441, -110.74000829597605, -110.3690783911604, -111.9386136764295, -111.04196305034188, -110.41800427558245, -110.94287511448232, -111.66035388807579, -107.53723747644062, -110.68014818358719, -111.86628806511304, -110.12097497430523, -109.69880468221378, -111.4312783987915, -109.18240866486639, -111.45649839248873, -110.1242345454651, -113.75911576151633, -112.71747598882953, -110.9614554157337, -110.92294419716129, -110.87229098694876, -111.09943759113875, -109.48107247947176, -108.62783006742795, -110.8108025857779, -111.63342408317932, -112.0221522906341, -109.96411229549527, -111.29821085030613, -110.04566676239914, -108.41674583097112, -107.50256474992416, -108.68086611003493, -110.3738906060137, -108.86763212826641, -109.81681043446049, -111.04539822346567, -111.73290882980949, -109.75238769150758, -110.55268275367449, -110.48423701377924, -112.1116140908134, -109.53952175199518, -108.538611608547, -111.3788321484912, -110.36378736224961, -110.37712171023523, -109.82150687920334, -109.17046632238393, -105.1169578108227, -110.84067642540583, -112.91626789016587, -111.32030958133453, -108.93375913686056, -112.44450956563915, -111.1596840012794, -110.17380444915341, -109.634859036508, -110.68819277718731, -110.0648098825346, -108.87385575091399, -111.99676414571755, -111.32585405719519, -110.59892045991457, -110.32589048340424, -111.1172696292077, -109.79946399891651, -110.10030723919304, -110.71841081343656, -112.23013150012054, -108.94400401141407, -109.71044551701596, -111.77560214164039, -109.68779520039777, -110.96119601299907, -113.66477058855787, -110.17794649102234, -110.30159876509862, -110.11953836266514]}, ...(2 in all)]
  out "FFT 2":cluster{"f0":dbl, "df":dbl, "magnitude":dbl[]}[](graph)=[{"f0"=0.0, "df"=16.666666666666668, "magnitude"=[-324.19011195451765, -78.1272953812706, -85.85545438627958, -89.30587144190069, -92.90590394398903, -93.63083388385274, -91.8644929119412, -95.26924857401164, -97.0710469181336, -98.01148078956652, -99.33043660296804, -95.58776817681839, -99.9570097527269, -101.45494093095093, -101.51838334751548, -101.00386616525799, -103.01963069818913, -103.20223925731209, -103.53783076500916, -103.48065647812659, -103.97797518531912, -104.58942778240602, -104.46991277190502, -104.59813972158683, -104.56685024229951, -104.69893799348945, -105.05669000016238, -106.17061117835001, -106.43303821862656, -107.39468286383597, -106.2899368267905, -105.7863846168199, -105.17170638885071, -104.53818172761852, -106.70340956723133, -106.55444321137247, -106.67654843051936, -107.79888413750199, -107.86424326005849, -106.09722609215336, -107.71648639013972, -107.79500725395155, -106.17330953637067, -105.43663624517525, -108.04970689199158, -109.92106271611999, -106.2505251183406, -110.60221373795562, -107.11377887451098, -108.4126937286195, -108.37794745021417, -113.22457316369011, -106.38281814065472, -107.55385617652075, -108.93026538982782, -106.19334142366085, -108.90462602264525, -107.63084712174981, -109.12192537022624, -107.90627042480016, -109.44472079190832, -108.91731458372392, -105.74102972706788, -105.74407510394178, -107.5989477192235, -106.2838630137392, -107.46190542725505, -107.38881299750702, -109.08024783239452, -104.97871836903269, -106.65424712290651, -107.04966019632134, -106.16202578092883, -102.98374199247179, -99.1568704142098, -87.07383781389657, -96.41471411313154, -102.65176579899618, -107.65674867775193, -102.85397890306213, -107.58658613411464, -104.79044898833125, -106.65282019869865, -108.65027966345534, -109.46169054950127, -108.69969979291741, -110.4048706652988, -108.81020193837274, -109.42808902484134, -108.85398463561398, -108.3849716744813, -109.1844457168716, -109.32787859535676, -111.01992124870878, -106.64843449415699, -108.9926343573667, -111.59837822080355, -110.57121677672183, -111.17280164669164, -110.68901970586144, -111.69013245592781, -109.90200577018311, -109.3554172126163, -110.7515368822992, -109.2863324212524, -109.66209701262974, -108.50795548698007, -110.58126481096504, -112.36093896766921, -109.78612141282203, -108.85120530917233, -109.91424431080952, -109.84698632196245, -110.93960894966105, -109.77214706089354, -110.30762971422381, -108.77791302937449, -110.79522659679036, -108.47242514643455, -111.20629758187835, -109.05996769621125, -111.13574821570619, -107.79388178889101, -111.5768481279296, -110.52058839597171, -111.58729762739313, -108.99000864386126, -111.6585121505227, -110.50715371958135, -108.87151956974363, -110.30486244367107, -108.32392040018144, -108.1769507919999, -110.43198471512189, -109.81454097966842, -110.26717009815644, -110.82924135076777, -110.34103661156989, -110.0692667126265, -109.34555682020833, -109.1694484721415, -109.9940980324044, -110.81940616215803, -108.21162003366862, -107.97087538330561, -107.55312461506225, -110.60339321606872, -110.09004629292225, -109.05860430198882, -113.1412749514818, -109.81628200948371, -108.62343219429849, -109.48172424209761, -110.85978755785311, -109.47778611557064, -108.81728552967951, -107.47864241666747, -107.61735128422292, -109.62511618983821, -110.32417726356636, -108.24287897478176, -108.60460879530194, -110.2181558494026, -107.95550802888957, -110.80234484950323, -111.09955733353904, -109.43923052503506, -108.98949130235951, -110.05778199870154, -110.36224432927585, -108.13523430027999, -110.681114579241, -110.49106131529867, -108.73493328004297, -110.07663907252234, -109.9968931372618, -112.10715231091008, -108.80994125105168, -111.63774865669372, -111.54355694032755, -111.64024217585788, -109.34986300492378, -108.88053713185408, -111.14370830146245, -111.17327416167232, -110.36311492990576, -109.99414559884396, -112.96912007380595, -111.43191437097785, -111.71327312809349, -108.77202323682606, -110.25970374932486, -112.59574277180732, -109.77247894866957, -110.09219852365874, -111.7197662726775, -109.85454092697009, -110.06789440397942, -110.38055758638309, -111.04251386932805, -111.54279434240568, -109.74385329575985, -110.98924544863415, -111.17898077762852, -110.98364252730245, -110.75024385843372, -109.24766708578407, -109.67753987004863, -110.6537235844391, -111.84436313010086, -109.12654337292446, -109.65519521121124, -111.1845162935778, -110.5009101465602, -110.22980642268818, -110.88540043278346, -110.29249073109453, -108.80459864528464, -107.49372141121728, -108.50353962704821, -110.00730069533373, -112.012876492648, -109.01283702976382, -109.07442203290057, -108.2961442983685, -111.60962842680907, -108.84312815413224, -108.6276642979969, -108.75132871638827, -109.30004903844721, -107.20359872252604, -109.12175943862074, -110.43914247337625, -109.55954680842791, -110.37116786618797, -108.55907813251434, -110.19249995041955, -106.95269845697632, -111.07027929458712, -110.1073996792702, -110.61729280468039, -109.6419175310234, -109.47995019876329, -109.66602827275211, -110.01953864498805, -108.45989120418268, -109.79778555296474, -109.94663827736616, -109.52410616839379, -110.58014441463794, -110.09182359045897, -111.0487262011397, -110.49609187214915, -110.6114701312941, -111.17752423063314, -109.74965389041003, -108.58973724447526, -108.84292130035902, -108.90689510645983, -110.69840140049361, -111.30494362640982, -111.00224390075273, -110.50848328538423, -111.59232911931113, -109.30826761863756, -108.44510893127558, -109.63744704504391, -108.95037574307332, -111.36486409910674, -112.74508631930381, -111.03952454593811, -110.57133212903979, -110.59969855145111, -108.25570461975128, -110.44617635200193, -110.32190307214704, -110.95204704643322, -112.0595421753479, -110.45342552693265, -112.50183987758867, -110.08217804938009, -108.90353583389084, -107.02032313792242, -88.3334978919524, -107.92027625495886, -109.83148570028482, -110.30427997450572, -110.92855407802753, -109.67404674397338, -111.03606345823586, -110.58277018943096, -109.77692362669393, -109.39170901729935, -110.20711662408928, -109.41601946806779, -110.34213214925832, -111.2283900972803, -111.51682597931386, -110.47069117801351, -110.93808974285523, -111.11277478000933, -112.50698886748012, -112.12918507523611, -110.46316790252011, -109.9387334819968, -109.78723249688426, -107.13037722044297, -108.16132376075751, -109.07255491017162, -108.85068428558272, -110.28038153100799, -107.77611023481016, -110.69754506886444, -110.09495581837979, -109.21214884561816, -112.62718526248648, -109.22048725312992, -109.17793923163308, -110.87372121410577, -109.71902632604333, -112.61041177225496, -109.6374750969677, -110.74738952366951, -108.93404661877067, -109.84938675700889, -112.25316361679832, -110.30788094875312, -109.26929069321925, -111.20853536783942, -110.05212566057608, -111.72448131932816, -111.55474439772887, -111.81988954424324, -108.44452452934028, -109.21897824914645, -109.55634869894358, -111.36318572800242, -110.05777399011298, -109.64458567712875, -108.73315084760529, -108.93332091319675, -108.4816455312154, -108.80120578498936, -108.1804470361839, -109.7177707524778, -109.31977709844544, -109.33603116022124, -111.46120546572519, -111.7480378245176, -109.17907150677627, -110.47970652472505, -109.73718750984082, -109.7935026884937, -110.40458408612054, -110.91781389491092, -108.39352075861481, -108.27512197925346, -109.59155075404814, -110.40183121737397, -109.25423373270381, -108.37769008625712, -107.91335995938509, -109.5576520703013, -107.27392145737491, -110.98592762117059, -108.41809950647861, -111.48163889400448, -109.70961684769624, -109.22952568656495, -109.76504719131209, -108.86928627177666, -107.97855299877004, -109.8412204399902, -109.6690048999326, -112.28329030175193, -111.54977099314607, -109.55689540119126, -107.93716711232997, -109.84247640855929, -111.5098351445789, -109.14317615215809, -110.28319116384824, -110.57901069942578, -107.2890252845352, -109.66754569546274, -110.15708115946433, -108.83782190109405, -111.60783857760667, -111.46884385151185, -109.21985333366634, -109.63605494317056, -110.87999187262697, -112.26992029775087, -111.05491095860552, -109.22795442529183, -108.99135781712076, -110.46475190704264, -109.35746113713218, -109.29125989270668, -107.40922407684049, -109.24391685563656, -110.41554602144217, -110.68952735085914, -110.62457364102458, -110.39856310555466, -108.84256124354566, -110.01614601335088, -109.8071306678428, -110.2804500736802, -108.76205061238203, -110.3962440297242, -108.98253716257014, -109.32990745926702, -111.17276766165281, -110.41113652364085, -110.36616199963426, -112.09767002991742, -108.43599666470733, -110.91876588140981, -109.05329272502944, -107.07198690769708, -108.72934463903034, -108.6666471996132, -108.97529973794413, -109.68895260146817, -109.2658844652487, -109.75690097249196, -109.38585024123027, -110.17593039468063, -107.87223111061134, -108.15261097418302, -110.09277437980633, -110.8665497655964, -108.43061614348413, -110.3052458526819, -109.22446919161898, -110.51909692711594, -110.06620699121913, -109.53439413051383, -110.31952463872884, -111.4732125902982, -110.41443606663168, -109.9579358088152, -109.930778061577, -108.5473214465574, -109.34719220288939, -109.16964653934396, -110.04824158176345, -109.42616539603762, -108.3556027482992, -110.62331917617789, -111.3652147859356, -110.12362012120938, -110.13175448595814, -111.20110099151856, -111.50643914621541, -108.11659117128028, -111.06037600347967, -109.03822892917451, -108.25678204604324, -110.82608024151122, -109.15887945314851, -109.88255674562845, -111.18322672526185, -110.95836040044516, -107.91535345885436, -110.66285812468733, -109.61906549925033, -109.58059721670746, -109.65198009505977, -109.65950565672951, -108.95264505276342, -109.23343669003113, -110.74308548011575, -106.39170014998685, -109.61471203101753, -108.24258770956924, -109.84609566640096, -107.83834185503922, -108.93052854090027, -107.55568820082641, -109.758551082242, -110.65892780872205, -111.99907420485852, -110.71043004141137, -110.62257237494617, -109.15610413532767, -106.87403836327807, -108.19175324576331, -110.27819583792918, -110.23918003777561, -108.29703377268754, -110.07182881114713, -109.60256111108491, -111.00394752430006, -110.30750337485472, -108.78309624082331, -109.24103013025798, -108.76979253891403, -109.91618737478264, -108.83915940855513, -110.92536150834754, -109.72250903746432, -108.96533939688658, -111.08949280651164, -109.20335070860871, -109.37826578362439, -109.77953166722301, -110.1867310744785, -110.07114559821346, -110.7003631567182, -107.86455899696074, -108.94113264174617, -109.35999427135138, -109.33627364788704, -108.96588828808375, -109.08716536982254, -108.73575375369026, -109.47770132070654, -109.83726171472907, -110.73516506891792, -110.56827134787686, -107.65667508354096, -109.30200115708924, -109.28406803847896, -110.55374624323233, -111.2017766725333, -108.50851279608973, -109.79494403619485, -109.08320018013063, -110.21850624918747, -108.4652936555984, -108.74837610538873, -108.81326140648238, -108.83830180036702, -108.785270477003, -110.01845876259073, -108.76030368637825, -108.57879884880157, -110.6610608456059, -108.74669367794318, -111.55956030460833, -110.22906685783455, -110.48411613865359, -109.48060880085136, -112.77556331479562, -108.2676071206087, -108.8571136162698, -108.56944905160177, -109.16406757131058, -111.42259299295839, -108.25216316582294, -110.48487127684025, -109.69532331373831, -108.13992755196784, -109.2987762526628, -109.82536192480795, -111.28650061088359, -109.12820736404241, -109.37960655471406, -108.96014976926716, -107.97535047619023, -112.31953123574708, -109.06198330523004, -107.52722515967098, -107.31555373665437, -99.89671790804692, -107.44442600896275, -110.6549218761941, -108.02265794322076, -109.63582761762919, -110.00574746987859, -109.51565124961209, -109.3550083591902, -110.4541529175301, -107.85799722437162, -105.1197113090786, -110.25038075579738, -110.39710812865657, -109.3618876098789, -107.6131301952152, -109.21529527621463, -108.7995754403799, -108.48347353145697, -106.45678488065816, -109.60427918561142, -110.81194387812535, -109.52215044127382, -109.88751598659705, -109.30205143590227, -110.74984456751768, -109.03952092986351, -110.69170786328897, -110.39236248162467, -108.65456161733339, -107.60439764386904, -109.97367926606955, -110.2754359970249, -108.81546418006434, -106.99691398176165, -108.42047325825182, -107.24499915944605, -109.28116135603187, -108.70650358781573, -108.05516916105047, -107.20893100196241, -112.07029265690055, -109.38099990478445, -111.53461820465232, -108.11312509555277, -108.76714028655223, -109.89565008459624, -107.71879172001115, -108.08434857420214, -108.79142773619792, -107.25153085963885, -110.05595039449301, -109.31604222314259, -109.94405791565286, -109.04715370361387, -108.89278831045846, -108.84682466376424, -110.0067927716526, -107.63768959294084, -108.98109382020348, -111.4720219575084, -110.76023788797733, -108.78599647633777, -106.59726674064618, -108.66715709719243, -107.99134359630926, -110.11396713841884, -107.21091759882775, -108.08576824949941, -108.80217666857972, -111.72949572713338, -107.33126296136014, -107.33731660097102, -108.04470462977443, -109.42963925921418, -111.03517778720736, -109.55293581015796, -107.99948151285162, -106.59480934999681, -107.63777243313498, -108.96490626068824, -108.8948210299064, -108.30870516747477, -109.13612869658097, -109.59971429402015, -110.2571461001396, -108.7655464686992, -109.81144209568883, -109.80796806645141, -109.20948481699544, -108.68653880881129, -109.26329796696166, -109.22428132233863, -110.12571678351438, -109.14615461144786, -107.08261621308327, -109.11338327144382, -107.75421565039201, -107.45291780756361, -109.00477000647248, -107.41031480478154, -109.98948062864928, -107.45953654921264, -106.37522884807879, -107.7786128523167, -108.03610987358499, -108.05926797128022, -108.59400205554164, -109.89620453365603, -109.03811240487515, -109.96909236705363, -109.28212981785472, -109.6772152101994, -108.26493868190678, -110.55558039199732, -106.6252818398841, -110.19075011176416, -109.56520012524705, -109.8023423576176, -111.2697570480663, -108.26752571816566, -112.00337375484828, -109.85709226796116, -109.36922081321148, -108.8424844298318, -111.2512302139209, -110.61775974680471, -110.22501328999012, -107.76874906708105, -110.71023653476604, -109.4025656165291, -107.66667684986125, -107.59759854092948, -107.94763263251238, -107.3888591871119, -108.62692803125044, -109.18012867988286, -107.78662871481455, -108.5072814073944, -109.50348958982907, -109.95177634938378, -107.78756251182895, -108.03865042797304, -110.1814993556385, -109.34937567548833, -109.52162025123161, -109.50819015441117, -108.20953105254624, -110.52154040214435, -109.3324404469266, -109.2696617050831, -109.54675609195674, -108.5940367000989, -109.40184828664549, -108.2518305610941, -108.55972691669434, -109.03647225394408, -108.48166656251695, -107.42023429066523, -109.42453054302521, -110.09532345960083, -108.78315822119662, -109.97508586102265, -108.22687406536997, -109.17110028890058, -110.15390449992647, -107.88577458651508, -108.28851074361447, -108.52030295163331, -110.03496861709483, -109.40014319167584, -107.73048113044877, -108.17571683963915, -110.34839852994926, -108.55894048192191, -108.74107339998285, -111.17734138993401, -110.22946440841412, -109.45511941802884, -108.0657300641843, -109.33797363184166, -106.95974095511333, -107.93068343723691, -109.78867669512647, -107.2087297624043, -109.542665021243, -110.05035859052961, -110.30235238883523, -109.20586170783808, -109.2796396673401, -109.14260673746566, -108.22019460542734, -109.99011886871159, -109.89103038547285, -110.36964772493243, -108.62340319923602, -109.06779821699769, -109.21830861066148, -107.7402395759509, -107.7178850938205, -113.45665085929117, -109.24039191621704, -109.30387033426037, -107.61849760982835, -109.41430582703529, -109.11482836392241, -111.89328423764577, -111.84653367963301, -109.00674896486915, -109.84488648739638, -109.41914760797953, -108.53442910169935, -109.66883322968232, -107.68762956301386, -109.82583101109167, -107.83405397804887, -108.78052031141966, -107.37842078941692, -105.40843158543845, -108.81430898189338, -109.57374640194516, -109.41111270322058, -108.82621700188898, -110.2552502368822, -110.23903890097205, -110.52171662278697, -108.21249857906324, -109.97268479379733, -108.20088823960992, -108.85682002802234, -110.11642849164285, -109.94087886999255, -111.63180946270296, -108.20899499456195, -106.73341567332112, -109.90003508676807, -110.14688274481229, -109.62259307329889, -107.57811196819495, -106.88584597822792, -109.16132624528932, -109.78677836397806, -108.59319344451784, -108.55877448618652, -109.46883711353044, -108.47309455543844, -108.09487065732198, -109.82219079158135, -109.63780237877428, -109.28348848877269, -107.62893405379826, -109.46986737961593, -108.03089712610223, -110.3931917410696, -106.06970126043262, -109.41866550703786, -105.31710372440419, -109.20218082282653, -108.28467118008108, -108.80026326744611, -107.40729224715713, -111.07322915141532, -107.1057186510818, -107.98286374205958, -108.51298722989311, -108.69632670891366, -107.96509231988331, -108.15882223414738, -106.85862416470376, -109.70705792539056, -108.64519930633055, -106.78708421443504, -109.43552377900174, -109.4474526498122, -109.10135248755788, -111.43316642580763, -109.33457343739448, -110.23547887071898, -108.95690647379442, -109.21159903769149, -108.12969562680841, -110.82751409340537, -108.55724349027832, -109.8796329603075, -108.50369978374582, -107.43145467247209, -108.60003323209516, -108.77155705999647, -109.33806063660796, -108.37500858898439, -109.65641721611547, -109.81905873737344, -108.03483220769625, -110.48028107566635, -108.60527372219985, -109.28768201151478, -99.8804125587218, -108.8913334544964, -108.23534920737794, -111.07646463287153, -108.59029790589766, -110.3405916586831, -107.66387718565608, -108.73793152614131, -110.61440166477816, -108.76211382544581, -110.23236978486065, -109.10669297094852, -109.15247609779597, -109.00539004923506, -110.14424353412238, -110.55445060661157, -109.48721312920799, -108.17040942305823, -108.77592227268228, -108.77130256578067, -107.82494496098512, -109.57266989523707, -108.75767497229612, -108.13688624150026, -107.8280716764963, -105.676279602552, -107.6370316684844, -109.73508547021689, -109.25365178573009, -108.86767843317584, -109.70969944273735, -108.91917504090888, -109.97734866522867, -112.17308993943783, -110.28356299479682, -110.7927103729386, -110.30837645846702, -107.56364161860179, -109.50188349731121, -109.36065627483853, -109.75389877587511, -109.81713476007774, -108.14524057525358, -109.43832376796216, -110.89342891210596, -108.15657882822792, -106.84106061627887, -107.83091759905821, -108.61794662682962, -109.57142366843581, -109.85402645528154, -110.12877022469837, -109.19414429724044, -110.56168468006764, -108.74720588273881, -107.90448559921305, -108.54421401507743, -105.06700039841249, -109.17937358052484, -108.94317576365822, -107.79410219455083, -109.24955437598658, -108.23334395173994, -108.98759227946937, -107.05986359444529, -107.20956512998849, -109.00295831471958, -109.43119556916457, -108.93348410522628, -108.99932477701081, -106.6448790859128, -109.06877251308666, -107.67053918439544, -109.15052780608639, -110.16878033319385, -106.55101141640301, -108.02811045752685, -111.52173447126572, -110.16854119242062, -110.93164036911654, -111.25979320890855, -108.82629030379024, -108.52004501839738, -107.09697056562636, -108.94233383169858, -107.37962568194772, -109.1239201710643, -108.93949898577122, -110.62573772949195, -110.09592372075662, -107.56136391005947, -110.45600430869621, -108.79481000016084, -109.41462449554598, -109.30248158488335, -108.70735295493108, -109.9174743694956, -109.94232543385962, -110.71725446170196, -110.0346196158573, -110.34814317845934, -110.6651078322521, -107.55409880424479, -108.71734776861287, -109.50902203986271, -110.40207542979611, -108.7847687630861, -111.10599488129682, -109.30824728923263, -108.20134064331717, -110.55959112431609, -107.77099734327174, -110.23862843385446, -108.48520797666865, -108.54205896654946, -107.79288769037599, -109.84022250170581, -108.02758364115576, -109.35132492327935, -108.87009749667932, -109.86905123364855, -109.19826752168308, -106.835240323691, -109.37910022114056, -110.80633973102931, -109.12703823829597, -111.07432699570984, -111.8064506085314, -110.09349947650527, -108.66467295777367, -108.75119108236053, -112.63983351316729, -110.90940743670113, -110.27973159222081, -109.57141664526549, -108.61645363771719, -109.31742355616147, -109.5839599160637, -110.01188998365383, -110.01923429741011, -108.94779759137936, -108.26169431000017, -109.24553201026085, -109.95709526422822, -110.68677343596859, -108.7678734483002, -110.47090469179284, -110.31604700116512, -110.10256600741997, -109.76634647265719, -110.8830805828562, -109.94609564072982, -109.20662382740542, -108.12492970530919, -110.5274435478767, -108.02351960398035, -110.6264936805739, -107.14559226383577, -109.13821777857531, -111.05324489472586, -110.15190797512811, -107.96366234783144, -110.03950681967147, -109.17476300510336, -110.41251816187909, -111.39219865477246, -111.32530426869943, -109.97369363558423, -108.98666403063845, -109.62049358645565, -109.58130494498671, -111.72738873188874, -110.39825891106616, -108.57430325757545, -111.28625510212446, -108.77421250595326, -109.75025415031793, -109.51948456745635, -108.82129398637998, -109.81362137198361, -107.86292494316123, -107.49318292857053, -109.66948564589373, -109.54288390056654, -107.99912445612077, -110.3497559614379, -108.00549349666127, -110.01361420523357, -108.4977916421456, -109.67078387286976, -109.85678367732866, -112.01237658746248, -108.4855625950998, -110.84880875737286, -110.9178674382154, -110.44187536727453, -108.75076921971127, -110.04946286646651, -109.99780941000827, -110.14242932305507, -109.56343773672316, -109.6278993388131, -108.77419573790174, -109.10543670530926, -109.7801848627463, -110.30733124104881, -113.13440550301436, -109.32709134514755, -109.74136656933283, -110.01525283266193, -109.43924662938396, -110.25325289253, -107.75460576671303, -110.60057027395933, -110.71458404922404, -110.15788509050662, -110.69167485018224, -110.96006652476157, -111.01156633983031, -111.6058448010008, -109.51364005052672, -109.76058205940885, -108.43421621088261, -109.47973949170208, -109.25533250208288, -109.47422603921065, -111.36411644613841, -107.27566171102698, -110.45098686173688, -109.93589296291184, -109.03803734663714, -110.53118128434016, -110.2408872254969, -110.0532234862915, -109.94185495614619, -110.2662004220774, -109.51094016962288, -108.5210104215432, -108.13691752270934, -110.18460088390265, -108.32609309150783, -109.89652230508281, -109.80923900768477, -109.01917388968883, -110.01248300968739, -109.43415605440147, -108.09823485138017, -107.40637725320931, -109.40632232658412, -111.97981999127656, -111.16609811629485, -111.64500793960192, -110.99793748693381, -109.55531276386903, -110.2535662621666, -108.17429802469516, -109.09425673355422, -110.23187110421917, -110.55358397926925, -109.93461124753053, -109.55604345832225, -109.44569510408274, -109.72185151080762, -109.52963702944834, -109.2303630328152, -109.74819502244243, -109.3932530349457, -109.17096788339686, -110.46153727064616, -113.1073731246639, -109.43753070459397, -108.13332547768168, -109.42294574929969, -108.45798401969856, -110.29453435046327, -112.66249403705643, -108.78314667434937, -105.9634478773668, -109.14327524669528, -108.50645190860273, -100.81571594994128, -104.4482859840643, -110.68926237051092, -109.12362553230196, -109.45234390564677, -107.91461416156068, -110.67788819353727, -110.05744935668449, -111.78333392154664, -106.83628914455993, -110.11115457346548, -109.13434608275826, -110.80006861194663, -110.35323502651462, -112.29149906501372, -109.01656376530778, -109.30871662948859, -109.79736315392456, -109.17848983603582, -108.09752397056482, -111.6039030763455, -109.27008844877828, -110.84475733314184, -109.72393917557073, -111.31060762894991, -110.78858793807466, -107.12841545099752, -109.54510865218204, -105.2805426080281, -106.28514149354733, -109.50656759582803, -110.14700878401054, -110.49737016725709, -109.19811547071924, -109.92527399676051, -110.7961615015146, -109.7447227818197, -109.49432012009893, -108.714081576733, -110.09766801550917, -109.08448507943001, -110.36154838733857, -109.86328656267403, -109.21144237434696, -112.4145136888034, -108.57567151011159, -109.66748589540896, -109.72985837578446, -109.29989238126763, -109.85868902806475, -111.01778182304162, -111.23625326328558, -110.01270868104203, -109.27067928081415, -109.71171312410247, -109.28697459293629, -110.67868067201007, -110.91353786857455, -111.21479955051575, -109.11315965407708, -109.40418681804496, -107.80511819596003, -107.37201025889816, -111.81969609169838, -109.89875624306032, -110.29328043898657, -109.74853280072202, -111.39527865400605, -109.47746221101964, -111.75141177452517, -109.31325306583483, -109.30117448911659, -109.3997781364162, -109.45356931295724, -109.60585285774386, -111.33951689512735, -107.74187210470228, -109.62706021606415, -108.72139655505221, -109.79552836110567, -110.64354037499807, -110.96138240913136, -110.02215059889615, -110.92978442698893, -110.0620778287114, -110.85019647293322, -111.77397403227091, -109.81257196800128, -109.15643451383403, -110.72777566469594, -108.7463769025616, -109.80959395914073, -111.24500986151126, -110.48863498350322, -110.30863780110901, -109.79331354195703, -110.34087081762074, -109.45183222569266, -109.6440990067103, -111.15034876658994, -112.14912485578341, -111.8886180186196, -110.57054820211916, -111.07556239924551, -110.5872832735073, -110.28912501038172, -108.91501133754849, -111.44575118962761, -109.90799859177967, -109.74421995550023, -108.70941446115883, -110.28822893097275, -109.70039554000401, -110.33701797570251, -110.79445894683306, -109.57694314608153, -108.816904416038, -109.66517126767175, -109.39501469321644, -110.85775022889956, -109.3689402795614, -112.09107318723095, -110.67985626248422, -110.32971146814747, -112.08166943494875, -109.93955548712543, -109.31722953035252, -110.2062913031861, -108.22565380081006, -110.680898028151, -111.95386604441454, -110.83354130587097, -108.5873626748948, -111.97536144124408, -109.23944159551515, -111.57859477689586, -110.80135186615524, -110.4800953731021, -110.14040729648133, -109.25873050390551, -108.87000960474569, -110.97091597211167, -110.15787270199012, -111.62434537618091, -108.5421625277294, -110.42258666403919, -110.96896115868603, -108.98253068925274, -109.54245055160168, -110.28051096122468, -109.48060498658319, -109.77618362117276, -111.64513838754992, -111.13945484239875, -110.18094280356001, -110.43757222770748, -110.81588360154201, -110.11656805555333, -108.47936291282355, -109.16476249859961, -109.3549985917136, -110.77753190334253, -111.46065694661178, -110.40387985996301, -109.95673803226478, -111.58660981285446, -108.59894875229345, -109.37333363882607, -110.26849699991793, -109.30500469266264, -109.23789020998296, -110.82000706486865, -109.25927538839868, -111.03285659417519, -111.08899832832414, -110.69361682858042, -109.45187168573815, -109.9614018482838, -109.70209527974106, -112.11903952100165, -109.59713611623246, -110.70292028698111, -110.12743849746808, -110.63315585514292, -108.60450276298175, -109.32832664986026, -109.99753023477764, -109.46644696130294, -109.1781290160558, -111.58830180575129, -111.67229040267557, -111.3750024136205, -108.33616679452298, -109.99797067800029, -110.50892429124391, -108.66074740829372, -111.17094662568759, -109.87538933985836, -109.152526628291, -110.44623159817101, -110.21603106403009, -110.64376935639365, -109.36897426842583, -108.67303022227141, -109.89327693080823, -111.50442955563923, -111.37532237834381, -109.38132821290205, -109.73509680539144, -110.53918379735906, -111.22869870340647, -109.39977573957616, -110.3674665334106, -110.5366125953241, -109.99025356764304, -109.97300035646616, -109.87631077033762, -109.64608829594286, -113.02486102973394, -108.26250283140733, -109.62234918138763, -111.18766216512655, -110.33666026406992, -110.5808115327039, -108.2971671321189, -110.10964334161903, -110.61254021379767, -109.89852549557533, -110.16562049054073, -109.41433790018287, -111.2453823439446, -110.45554802599901, -113.11454453784393, -110.7333866145056, -110.00858191882439, -108.54745315874294, -110.08430415376903, -111.9006972727596, -110.3031506154679, -110.26331790366497, -109.36797925566673, -109.04860552478912, -111.83514212681175, -111.38960737633833, -109.01429665187288, -110.96404839103826, -108.95488871107163, -109.09652004914592, -111.884304581971, -110.57566691021339, -111.95113404442795, -110.13677174050159, -108.10078686353354, -107.69442565416006, -112.42676605669463, -109.12681161784135, -109.23120766087519, -110.57649395555585, -110.22143082743162, -108.40065951773644, -109.46923168308618, -111.39095086729745, -110.46375658526013, -111.45145283328486, -112.22610823637353, -110.61090190564383, -112.22250292674809, -111.7379343196361, -110.18530386733481, -108.93867365671692, -111.89304844956082, -109.06146134986984, -110.98405731832798, -109.76366821333497, -108.08326795663608, -109.95041147835065, -112.94140614324155, -111.79814935135965, -108.07337559063119, -109.13733403265212, -111.74906646037496, -111.12228668433455, -110.02899450462209, -110.22237716929811, -109.0224776891049, -110.18135850497721, -113.32516073881047, -111.3576490243877, -110.60510094465171, -109.6935518470342, -110.36313473154901, -111.95933240129618, -109.49625308071019, -109.18827910216122, -110.54311407822692, -108.4811035913567, -112.81280225723607, -108.86530665787413, -110.85796435061886, -110.40059714639627, -108.19250716343407, -108.96956521802292, -108.61281798886506, -109.78061525370413, -111.58885511891798, -109.06279169160345, -111.43043988466789, -111.63169336321079, -109.54702536206447, -109.62860636296405, -109.47865811135546, -108.02265793654806, -109.97461304995515, -110.72549884050886, -111.57309413919933, -110.03317891949746, -110.39570411598524, -110.27606115470397, -110.63294457306095, -110.71821689302902, -110.38076268941819, -111.51223508887897, -110.40703572670697, -112.24933273737743, -109.74954300082398, -108.46020292937696, -111.05315219575881, -110.38635148390118, -109.58268303790976, -112.34211536832117, -108.45894118755307, -108.96463982695337, -110.56040438523046, -110.67803313671729, -111.07349872375121, -110.42184162876096, -111.82081126435692, -108.85923651136297, -112.57723799596502, -113.65690874668172, -112.62314325834605, -110.70357529341362, -110.959925221544, -111.26336183001875, -108.1350700630152, -107.94545932312926, -111.17610778209841, -110.20386728310686, -108.55646511121591, -109.8400922569145, -111.73466587035968, -110.47272877573613, -108.33011124048193, -107.93042857580332, -108.60928277989103, -109.25240966798974, -108.96403833602028, -106.94222615757475, -109.37086694261907, -106.72743097285155, -109.03160193412796, -107.3549903889451, -106.8543848510082, -107.83503929060929, -106.30745467433752, -108.36915807168845, -107.13065938379303, -107.84769200880969, -106.08004345082777, -108.15244601930225, -108.37254117816573, -106.57863034819223, -108.1283698227614, -108.19776505569902, -107.58283412238643, -108.17365133196301, -108.6794309781181, -107.91552140588759, -111.60122989270022, -107.04360635941174, -111.55535949001795, -109.39870426166594, -109.55937904851662, -111.81389508925734, -109.88957041098786, -110.84764586896561, -110.59130246272693, -111.15944135223884, -110.19496154041607, -111.51861903129362, -110.74798816525838, -111.37312965175558, -110.10842817220238, -110.73198099204856, -111.36708667993291, -110.30840247819665, -110.11744489669044, -110.55237850846444, -108.2073528237766, -112.70750856801911, -110.99917956040802, -109.84949484779976, -111.3403161887679, -110.08924435263565, -110.17749213365616, -112.10849123224503, -110.94270741299202, -109.29350963424746, -110.33477486966507, -112.19620157705627, -111.45484078395934, -111.86858843505124, -110.22491147345858, -108.96177661263177, -108.67862820579893, -107.55155410582937, -108.27984439169573, -108.72682528077233, -110.64231212183269, -109.32873093119183, -112.98564364754564, -110.78933114228725, -108.50921025910479, -107.91087245586935, -112.57350030929283, -111.75871577457525, -108.42095298945462, -112.31266064114303, -110.1295657579673, -109.67444664474456, -110.33749884929306, -109.16098218724147, -109.63554874360221, -109.15892392675141, -111.90580809179818, -108.81196712336858, -111.42223552606656, -109.90571484965518, -109.99739812086352, -111.64103850263211, -111.31463957090885, -110.61247447444549, -110.20960333715526, -110.1707327818923, -109.70412636554525, -110.97278093107532, -110.24386747740314, -109.81378546061525, -110.83784085086458, -109.77357954318757, -111.22663832948885, -111.14563050139252, -110.87152231402447, -110.34246044319893, -109.97174570657546, -110.23599592972218, -111.08206161770731, -110.0073315341242, -111.11748366902188, -112.04005964728601, -109.81290191679287, -109.68543639040858, -112.01143296194752, -110.13641850530031, -108.19348942447623, -109.7534468948808, -109.36697824644176, -97.56454580435337, -104.97829040517887, -108.1539132982256, -110.048991273122, -107.46172505860011, -110.49269280640675, -109.94209901400029, -109.38576869679022, -111.43699124347364, -110.89973083498887, -111.2994445418276, -109.25144782032437, -113.25676258473536, -110.82078737428088, -109.97779571182073, -113.36294799183014, -111.38584551238931, -112.17267897274873, -108.56430946159155, -112.06841286528645, -110.36822473102735, -109.54758527532016, -110.48190506674653, -110.03535695860182, -109.3951469796576, -112.41910682256774, -111.38124138857238, -109.37850389100952, -111.65544568836181, -111.55876881606889, -109.3029209617236, -109.20030046194076, -108.82610577621037, -110.53329453526098, -109.96090595542142, -109.67834229432077, -110.62303603007352, -109.8388817181171, -109.22430039793213, -108.92749786663613, -110.05794249283548, -109.58534943218437, -110.50493887507297, -109.96373022997366, -111.0645036323456, -111.28501675364454, -109.77386932343008, -108.8952247140968, -110.09242801628717, -112.90943444063141, -110.72299296247249, -109.39094335967056, -110.95165384057718, -109.59809519359453, -110.4978602309597, -109.67109981692639, -111.2489619905986, -110.0937750887109, -109.76771021128954, -108.32976315018955, -111.3058145792439, -111.09464974601362, -110.99797900696136, -109.174315000222, -109.630351559617, -110.26289147175856, -110.22688407202517, -109.96748050100612, -112.13247633583758, -110.59994952890855, -110.93023020153811, -109.22457750926695, -110.26162558926984, -110.09713110375579, -111.73858994918328, -109.78183160058515, -109.7603471824367, -110.96016892586911, -111.23309626937036, -109.83093663960678, -114.05354944347246, -111.58202863059464, -110.42281828744524, -110.9521484732059, -112.5120328206343, -111.614891937737, -109.84428787405484, -111.61119567831453, -110.43095563229411, -111.71833448430398, -110.01132196809407, -109.37558169247951, -109.14091380022785, -110.42663661754088, -110.3598013572826, -109.78207135281417, -109.94058843992468, -109.88210328447205, -108.6217811850147, -107.17834387173707, -110.6447226986756, -111.10704778101115, -111.24396771977769, -110.47849395539598, -110.75150631628034, -109.67662689396347, -109.23145032835053, -108.83780193265358, -109.43468321661163, -102.22521103859944, -106.90009867479111, -108.91580608784525, -109.58671397003187, -110.56692028436989, -108.75103142680105, -111.00795573084157, -110.75039085328763, -109.48222099288613, -111.8621134816908, -110.26507966786443, -108.885924716389, -109.30841399453053, -112.3188631425597, -111.05677697153163, -108.8268571902449, -109.63028152237679, -114.82339015806369, -107.03435216376964, -111.34847692589166, -109.61354114874855, -112.32687758049907, -109.59816404231358, -111.64248480241805, -111.84075757907273, -110.44017657636552, -110.15181635726277, -111.93813663582833, -109.11826378836209, -109.99779889778326, -109.927119030584, -109.4389650887841, -111.52448814187727, -111.38736268499642, -110.51920914917922, -108.64230614681055, -108.90307263595304, -110.57246891832371, -109.65575340646116, -109.80359672370373, -108.83368585528197, -111.09385004343437, -108.83430005497769, -112.37784208819113, -109.50005381621696, -109.67421750136593, -111.39664088797532, -109.70867599669316, -109.52498993629875, -111.12341349673187, -110.0484037026941, -109.55138667646308, -111.06614422098669, -109.4785941493091, -110.25724082617013, -110.93950616855716, -110.53487953881397, -111.45722057988401, -110.32393446412904, -110.34361936710438, -108.6610336097813, -109.53631603696368, -108.06930707969195, -107.68056561368934, -108.73860971027449, -108.87111384617579, -108.40433837098611, -110.55999576884835, -106.83832061167207, -108.28786975902513, -109.18482905697472, -107.81071696594883, -107.91047268802457, -108.79613111673706, -111.05361322310213, -109.97897453479862, -109.12920563729425, -111.20538391490288, -109.26286135293664, -111.31400407177502, -109.92167984752287, -110.70854322826071, -108.59406515713611, -109.69371333227458, -109.36664873267313, -110.35521729513704, -110.40667924006368, -112.0181844636846, -111.01529188207431, -110.59246505728431, -109.95068312717868, -110.75807466894047, -109.58596443762707, -111.12127793384956, -109.59041634463125, -111.56255571372793, -110.43405578864342, -108.39660324329928, -111.1420710307505, -113.64788483868595, -111.67645688353934, -111.36878760365944, -109.68523694561108, -110.11608766310304, -109.25670490330123, -110.73546181099229, -111.77855039399805, -107.9662794718261, -109.67483334602832, -109.891258579519, -110.24757768183042, -109.50202895993814, -110.07763831916637, -109.96891925839451, -110.97268925927641, -109.31698133827767, -112.27933593506792, -110.36206721075725, -109.47379463718867, -110.27836850941338, -110.63738280998388, -111.3611682777485, -110.72689155959884, -111.55480904927032, -111.16689658479412, -110.35555645743601, -111.56609319131051, -110.88279459952174, -114.73607246523177, -109.95813757295693, -107.64639932425493, -111.26486783320321, -112.03946356928121, -111.8915972448334, -110.35245920812773, -110.83155104803564, -110.67437747473863, -110.9959682920065, -110.7815352345103, -111.13722283763049, -112.54797265493127, -110.06894780898469, -111.65186554925783, -111.83545188116254, -110.65894756123697, -108.48458025065264, -112.43760714427981, -114.1368408201927, -110.40065777895025, -110.1066998945526, -108.60654239598591, -110.5716060205154, -110.74257357180736, -111.1136089342442, -111.53539811075092, -113.2559601458872, -109.2003227548348, -110.42285840441025, -111.4086884998834, -111.61503050693868, -110.8194303494779, -108.9701587059964, -112.58521089509063, -110.10873915265242, -112.43440038319561, -110.03468788439882, -111.57896603236308, -110.21939233582523, -109.03614470500777, -110.11738923539659, -109.55359574898291, -110.416473622654, -109.4626868574157, -111.17164025076731, -110.3579689035081, -109.04338716157822, -112.36157114517567, -109.32125615922843, -112.71105693789394, -110.11019129547768, -108.96439402555632, -111.107663418839, -111.48306369859839, -110.9317530461794, -107.98628540532181, -111.1636972328743, -110.47837837583148, -109.04649309175733, -110.27110334963734, -111.35803630614352, -110.77259078859605, -111.46352820533895, -111.16789261049541, -109.2376344776325, -111.6795794983659, -111.74292205167644, -109.40835022991612, -111.02163652600731, -108.79482078001607, -110.6718658416566, -111.08747067599332, -112.15383726791498, -109.47049126158717, -109.061574046483, -111.23993049318979, -111.02521156588335, -109.46012868444186, -110.13918914826291, -112.08180381836377, -110.61929875223015, -111.4424805369965, -111.43420275069585, -109.71347556238717, -110.24726273025648, -109.7860268673935, -109.94126895018422, -111.41948668868926, -108.90555991781676, -110.81242861886172, -109.65007052722677, -112.12672329335953, -110.01123170946096, -111.13980448279096, -113.92013682657084, -108.6000853867411, -110.66793592761913, -110.61237681642844, -110.00839105230496, -109.38083187034974, -109.46119372195675, -110.3708067287448, -108.55518656223285, -113.33935987443276, -111.92184778392033, -111.80820718236087, -107.36852757311246, -109.51077803361602, -110.066791721019, -108.756710558672, -107.91391289865918, -110.72851430959301, -111.39074956442978, -112.928843679455, -109.87348280521556, -112.21371750380071, -110.82495902297394, -109.94006136010094, -110.58757785050143, -110.2790091349881, -111.43884888223081, -108.09540986530712, -109.63783244641691, -110.19577975613292, -110.01690033746098, -112.75938920157155, -109.27158857362184, -111.19519821680541, -110.14381902425255, -110.45955291199236, -111.55660330002316, -110.75604254261134, -111.02122553784838, -111.6490091060193, -110.93362819419399, -110.49033159684308, -110.70789549836027, -110.41991882034145, -110.0264093421208, -109.18432746063652, -110.15292268755287, -112.40733942236504, -111.32869665965416, -110.95418667871114, -111.14291568823575, -111.75555369152653, -112.98146297069803, -109.73870744292117, -111.33806139459435, -110.18838799491355, -112.60408243005732, -110.26112648646833, -110.58257045107274, -109.75155437454112]}, ...(2 in all)]
  in  "FFT 1 Choice 1":u16(ring) items=["T1 Y", "T1 X", "T1 Sum", "T2 Y", "T2 X", "T2 Sum", "T1 FB X", "T1 FB Sum", "T2 FB X", "T2 FB Sum", "PSD Y", "PSD X", "PSD Y Sum", "none"]
  in  "FFT 2 Choice 1":u16(ring)=3 items=["T1 Y", "T1 X", "T1 Sum", "T2 Y", "T2 X", "T2 Sum", "T1 FB X", "T1 FB Sum", "T2 FB X", "T2 FB Sum", "PSD Y", "PSD X", "PSD Y Sum", "none"]
  in  "FFT 1 Choice 2":u16(ring)=1 items=["T1 Y", "T1 X", "T1 Sum", "T2 Y", "T2 X", "T2 Sum", "T1 FB X", "T1 FB Sum", "T2 FB X", "T2 FB Sum", "PSD Y", "PSD X", "PSD Y Sum", "none"]
  in  "FFT 2 Choice 2":u16(ring)=4 items=["T1 Y", "T1 X", "T1 Sum", "T2 Y", "T2 X", "T2 Sum", "T1 FB X", "T1 FB Sum", "T2 FB X", "T2 FB Sum", "PSD Y", "PSD X", "PSD Y Sum", "none"]
  in  "Reset FFT":bool
  in  "# Spectra to Ave.":dbl=25.0
  out "Ave. Time (s)":dbl=1.5
  in  "Tab Green FB":T5(tab)=enum."Trap Control (RF)"
  in  "Scale factor":dbl=0.5
  in  "Scale intensities":bool
  out "Feedback overload":bool
  in  "T2 for asymmetric\n(MHz)":dbl=85.0
  in  "Middle freq for \nsymmetric (MHz)":dbl=78.0
  in  "Symmetric manual \ntrap motion":bool
  out "Stage Moving":bool
  in  "Read Cal":bool
  in  "Confocal Linescan":bool
  in  "Confocal Image":bool
  in  "Round T1 X":bool caption="Round"
  in  "T1 offset_x (mV)":dbl=44.132512662199076 format="%#_2g"
  in  "T1 kappa_x (pN/nm)":dbl=0.1608167093260824 min=0.0 step=0.001 format="%#_2g"
  out "Time (s)":dbl=40.5
  out "Total Time (s)":dbl=60.0
  in  "Start Saving":bool
  in  "Cal sets to save":u32=50 min=1 step=1
  in  "Comment":string="testing confocal setup"
  out "Calibrating Trap...":bool
  in  "Trap 2 (ON/OFF)":bool=TRUE
  in  "Trap 1 (ON/OFF)":bool=TRUE
  in  "Save Calibration":bool
  in  "N sets to save":u32=200 caption="N Sets"
  in  "Save N Sets":bool
  out "Save file name":path=path "I:/Data/160525/160525_043.dat"
  in  "Save ave N":i32=500 caption="Averaging Factor"
  out "Saving...":bool
  in  "Stop Saving":bool
  out "Progress":u16(slide) scale=0.0..100.0
  out "Manipulating Trap":bool
  out "Buffer Status":dbl(slide) scale=0.0..1.0
  out "Overflow (data lost)":bool
  in  "Reset":bool
  out "Data Rate (Hz)":dbl=66666.66666666667 caption="Trap Data Rate (Hz)" format="%#_3p"
  out "Save Data Rate (Hz)":dbl=133.33333333333334 caption="Rate (Hz)" format="%#_3p"
  out "Save Data Period (s)":dbl=0.0075 caption="Period (s)" format="%#_6p"
  in  "T1 alpha_x (nm/V)":dbl=701.8425766517444 step=10.0 format="%#_3g"
  in  "T2 alpha_x (nm/V)":dbl=806.869454518421 step=10.0 format="%#_3g"
  in  "T2 kappa_x (pN/nm)":dbl=0.13871102209446912 min=0.0 step=0.001 format="%#_2g"
  in  "T2 offset_x (mV)":dbl=-16.403354316809207 format="%#_2g"
  in  "BD 1 Frq 2 (MHz)":dbl=90.0 caption="T2 X (MHz)" min=60.0 max=90.0 step=1.0 format="%#_6p"
  in  "Round T2 X":bool caption="Round"
  in  "MCL Y":dbl(slide)=4.669617603076266 caption="Confocal Y (V)" min=0.0 max=10.0 step=0.01 scale=0.0..10.0 scale format="%_1f"
  in  "MCL X":dbl(slide)=3.742542191839351 caption="Confocal X (V)" min=0.0 max=10.0 step=0.01 scale=0.0..10.0 scale format="%_1f"
  in  "Trap Raster Scan":bool
  out "Raster Scanning...":bool
  in  "Trap Delta (MHz)":dbl=20.0 step=1.0 format="%05.2g"
  in  "Trap Intensity\nSetpoints (V)":cluster{"Set 1":dbl, "Set 2":dbl}={"Set 1"=5.0, "Set 2"=5.0}
  in  "Index":dbl=43.0 caption="Save File Index" min=1.0 step=1.0
  in  "BD 1 Frq 1 (MHz)":dbl=70.0 caption="T1 X (MHz)" min=60.0 max=90.0 step=1.0 format="%#_6p"
  in  "Goto Top (F6)":bool
  in  "Save":bool
  in  "Capture":bool
  in  "?":cluster{"x":string, "y":string, "z":string}={"x"="N.D.\r\n", "y"="N.D.\r\n", "z"="N.D.\r\n"}
  in  "Capture Locations":i32(listbox)=2
  out "X Pos":string="-0.85624\r\n"
  out "Y Pos":string="0.27735\r\n"
  out "Z Pos Pos":string="0.05734\r\n"
  out "X Motion":string="1\r\n"
  out "Y Motion":string="1\r\n"
  out "Z motion":string="1\r\n"
  in  "Goto Bottom (F7)":bool
  in  "Goto Exp (F8)":bool
  in  "Main:":bool caption="Inject Pump 3"
  in  "Inject Top:":bool caption="Inject Pump 1"
  in  "Shunt:":bool
  in  "Inject Bottom":bool
  in  "Scan Range (nm)":dbl=1683.3000000000002
  in  "Symmetric Raster/Feedback?":bool
  in  "VISA Clear":bool
  in  "Green Laser ON/Interlacing":bool
  in  "Current When FB OFF (%)":dbl=10.0 min=0.0 max=100.0 step=1.0
  in  "Green laser mode":enum32{"Laser ON", "Laser OFF", "Interlace"}(radio)
  in  "Ch 1 Inject Rate (ul/h)":dbl=50.0
  in  "Pump write delay (ms)":dbl=300.0
  in  "All Pump Parameters":T6={"Pump 1"={"Diameter (mm)"=4.61, "Units"=4.0, "Volume"=100.0, "Rate"=50.0}, "Pump 2"={"Diameter (mm)"=4.61, "Units"=3.0, "Volume"=0.0, "Rate"=0.0}, "Pump 3"={"Diameter (mm)"=4.61, "Units"=4.0, "Volume"=100.0, "Rate"=250.0}}
  in  "Ch 2 Inject Volume (uL)":dbl=100.0
  in  "Pump pause delay (ms)":u32
  in  "Ch 3 Inject Volume (uL)":dbl=100.0
  in  "Ch 3 Inject Rate (ul/h)":dbl=250.0
  in  "Flush Center Ch Volume (uL)":dbl=15.0
  in  "Flush Center Ch Rate (ul/m)":dbl=100.0
  in  "Inject Valve B":bool caption="Inject Pump 2\n(Flush Center)"
  in  "Total Volume\nFlushed (uL)":dbl
  in  "Tab IR Control":T7(tab)=enum."Feedback on Trap Position"
  in  "RF phase reset before cycles":bool
  in  "Phase increment trap 2":fxp<+/-,64,32>
  in  "Phase increment trap 1":fxp<+/-,64,32>
  in  "Phase offset method":u8=3
  in  "Next trap write delay (ticks)":u16
  out "FPGA error out":errorcluster
  out "Total Counts (ticks)":u32=600
  in  "Trap ON/OFF X or Y Amp?":bool=TRUE
  in  "Oscillate Set 2":bool
  in  "Trap 1 ON":bool=TRUE
  in  "Number Interlace Sets":u8=3 min=1 max=3
  in  "DIO count 3 (ticks)":u32=200
  in  "DIO count 2 (ticks)":u32=200
  in  "DIO count 1 (ticks)":u32=200
  in  "BD 2 Amp 3 (%)":dbl min=0.0 max=75.0 step=1.0
  in  "BD 2 Amp 2 (%)":dbl min=0.0 max=75.0 step=1.0
  in  "BD 2 Amp 1 (%)":dbl min=0.0 max=75.0 step=1.0
  in  "BD 1 Amp 3 (%)":dbl min=0.0 max=75.0 step=1.0
  in  "BD 1 Amp 2 (%)":dbl=42.0 min=0.0 max=75.0 step=1.0
  in  "BD 1 Amp 1 (%)":dbl=40.0 min=0.0 max=75.0 step=1.0
  in  "BD 2 Frq 3 (MHz)":dbl=26.0 min=60.0 max=90.0 step=1.0 format="%#_6p"
  in  "BD 1 Frq 3 (MHz)":dbl=70.0 min=60.0 max=90.0 step=1.0 format="%#_6p"
  in  "BD 2 Frq 2 (MHz)":dbl=26.0 min=60.0 max=90.0 step=1.0 format="%#_6p"
  in  "BD 2 Frq 1 (MHz)":dbl=26.0 min=60.0 max=90.0 step=1.0 format="%#_6p"
  in  "Not-Interlacing Set":enum32{"Set 1", "Set 2", "Set 3"}(radio)
  in  "Interlace":bool=TRUE
  in  "Trap 2 ON":bool=TRUE
  in  "Trap 3 ON":bool
  in  "Scan axis 2":bool=TRUE
  in  "Osc. freq. (Hz)":dbl=0.25
  in  "Osc. amp. (MHz)":dbl=2.0 format="%1_3g"
  out "Coords":T8
  in  "Manipulation Scaling":cluster{"Horizontal":dbl, "Vertical":dbl}={"Horizontal"=0.075, "Vertical"=0.01}
  in  "Freq or Amp switch first":bool=TRUE
  in  "Swap F1 and F2":bool
  in  "Freq switch delay":u16=9
  in  "Amp switch delay":u16=4
  in  "Period":i64=2
  in  "Raster to target force?":bool
  in  "Raster target force (pN)":dbl=10.0
  in  "MCL Step Increment (V_int)":dbl=3.0
  out "Time to Finish All (min)":dbl=0.666 format="%#_2p"
  in  "Scan Speed (nm/s)":dbl=100.0
  in  "Step Size (nm)":dbl=1.0
  in  "MCL/AOM Scale Tweak":dbl=1.0
  in  "MCL Step Position Ratio":dbl=0.5
  in  "Move MCL Also?":bool
  out "Final sep (nm)":dbl=1590.0
  out "Initial sep (nm)":dbl=360.0
  out "Save index":dbl=43.0
  out "Final delta (MHz)":dbl=30.0
  out "Initial delta (MHz)":dbl=20.0
  out "Final freq. (MHz)":dbl=60.0
  out "Initial freq. (MHz)":dbl=70.0
  in  "Saved AOD Raster Scan Parameter Sets":T9(array[cluster])=[{"Scan Range AOD (nm) 2"=500.0, "Step Size AOD (nm) 2"=1.0, "Scan Speed AOD (nm/s) 2"=100.0, "Number of scans (AOD) 2"=1, "Label"="offset curve"}, {"Scan Range AOD (nm) 2"=1000.0, "Step Size AOD (nm) 2"=1.0, "Scan Speed AOD (nm/s) 2"=100.0, "Number of scans (AOD) 2"=1, "Label"="hp raster check"}, {"Scan Range AOD (nm) 2"=6.8, "Step Size AOD (nm) 2"=0.34, "Scan Speed AOD (nm/s) 2"=0.34, "Number of scans (AOD) 2"=1, "Label"="3.4 kbp - 1 bp steps"}]
  in  "Load parameters":bool
  out "Scan Range (MHz)":dbl=-10.0
  in  "Restart DMA? (AOD)":bool=TRUE caption="Restart DMA?"
  out "Incr. int (AOD)":i64=-5670036101
  out "Time/Scan (s) (AOD)":dbl=19.98 format="%#_2p"
  out "Data points/scans":dbl=2664000.0
  out "Data points/scan (f/b)":dbl=2664000.0
  in  "Save scans":bool=TRUE
  out "AOD Scan I":u64=2 caption="Scan I"
  in  "Continuous AOD Scanning":bool caption="Continuous Scanning"
  in  "Abort AOD Scan":bool caption="Abort Scan"
  in  "Scan BD":bool=TRUE
  out "Cycles/step (AOD)":u64=666 format="%.3p"
  in  "Number of F/B Scans (AOD)":u16=1 min=1
  out "Scan steps (AOD)":u64=2000
  out "Scan Increment (MHz)":dbl=-0.0050025012506253125
  out "AOD Scanning":bool caption="Scanning"
  in  "Start AOD Scan":bool caption="Start Scan"
  out "N sets should be saved":dbl=133.2
  out "Progress 2":u16(slide) caption="Progress" scale=0.0..100.0
  in  "Abort save 2":bool caption="Abort save"
  in  "Trap 1 Bead Size (nm)":dbl=1000.0
  in  "Trap 2 Bead Size (nm)":dbl=1000.0
  out "MCL Count":dbl=782931.6080202644
  out "Trap 2 amplitude":dbl
  out "Trap 1 amplitude":dbl
  in  "PID gains":T10={"proportional gain (Kc)"=0, "integral gain (Kc*Ts/Ti)"=5, "derivative gain (Kc*Td/Ts)"=0}
  in  "All FB On/Off":bool
  in  "AI2 to Setpoint":cluster{"Set 1":bool, "Set 2":bool}
  out "AI2 (V)":cluster{"Set 1":dbl, "Set 2":dbl}={"Set 1"=3.087557603686636, "Set 2"=2.914212469862972}
  in  "Reset Feedback":cluster{"Set 1":bool, "Set 2":bool}
  in  "Feedback On/Off":cluster{"Set 1":bool, "Set 2":bool}={"Set 1"=TRUE, "Set 2"=TRUE}
  in  "Auto read offset\ncorrection":bool=TRUE
  in  "Negate Diff?":bool
  in  "Diff. FB.":bool=TRUE
  in  "Dynamic Force FB":bool=TRUE
  in  "Reset Trap Pos. FB":bool
  in  "Tab FFB Settings":enum32{"Main Setting", "Details"}(tab)
  in  "Use Offset in FFB?":bool=TRUE
  in  "Setpoint correction\noffset file":path
  in  "Negate offset difference":bool
  out "B factor":dbl=0.9916156324677038
  in  "Trap Pos FB Int Count":u16=100
  in  "Trap Pos. FB Gains":T11={"proportional gain (Kc)"=20.0, "integral gain (Kc*Ts/Ti)"=3.0, "derivative gain (Kc*Td/Ts)"=0.0} {"proportional gain (Kc)" format="%.11g"; "integral gain (Kc*Ts/Ti)" format="%.11g"; "derivative gain (Kc*Td/Ts)" format="%.11g"}
  out "Offset file step size":dbl=0.1
  in  "Read setpoint correction\nfile":bool
  in  "Trap Pos. FB Offset Factor":i64
  in  "Trap Pos FB Negate Action":bool=TRUE
  in  "Trap Pos. FB Mult Factor":i64=8388608
  in  "Trap Pos. AI1 X Pre-scale":u16
  in  "Trap Pos. FB Range":T12={"output high"=0.999969482421875, "output low"=-1.0}
  out "Trap Pos FB Int Signal":fxp<+/-,24,9>=42.09515380859375 format="%.18g"
  out "Trap Pos FB Int-Norm Signal":fxp<+/-,16,1>=0.042083740234375 format="%.16g"
  in  "Set SP Using...":bool
  in  "Trap Pos FB Monitor\nT1 or T2":bool
  out "Trap X AI1 (DMA)":T13={"Set 1"=0.030731201171875, "Set 2"=-0.0113525390625}
  in  "N El. to Ave.":i32=10000
  out "Trap Pos FB Action":i64=-32767
  in  "Offset Values":T14={"Trap 1X offset"=array[500 elements], "Trap 2X offset"=array[500 elements]}
  in  "Setpoint offset\nCorrection values":dbl[](array[numeric])=[0.024496601698410773, 0.024671186719617436, 0.024845771740824106, 0.025020356762030765, 0.02519494178323743, 0.025369526804444095, 0.025544111825650764, 0.025718696846857424, 0.025893281868064093, 0.026067866889270756, 0.026242451910477423, 0.026417036931684082, 0.02659162195289075, 0.026766206974097418, 0.02694079199530408, 0.027115377016510744, 0.027289962037717407, 0.027464547058924076, 0.02763913208013074, 0.027813717101337402, 0.027988302122544065, 0.02816288714375073, 0.028337472164957394, 0.02851205718616406, 0.028686642207370723, 0.028861227228577393, 0.02903581224978405, 0.029210397270990722, 0.029384982292197385, 0.02955956731340405, 0.02973415233461071, 0.029908737355817377, 0.030083322377024047, 0.03025790739823071, 0.030432492419437372, 0.030607077440644035, 0.0307816624618507, 0.030956247483057368, 0.03113083250426403, 0.0313054175254707, 0.03148000254667736, 0.03165458756788402, 0.03182917258909068, 0.03200375761029735, 0.032178342631504014, 0.03235292765271068, 0.03252751267391735, 0.03270209769512401, 0.03287668271633068, 0.033051267737537346, 0.033225852758744005, 0.03340043777995067, 0.03357502280115733, 0.033749607822364, 0.033924192843570664, 0.03409877786477733, 0.034273362885983996, 0.034447947907190656, 0.03462253292839732, 0.03479711794960398, 0.03497170297081065, 0.035146287992017314, 0.03532087301322398, 0.035495458034430646, 0.035670043055637306, 0.03584462807684397, 0.036019213098050645, 0.036193798119257305, 0.03636838314046397, 0.03654296816167063, 0.0367175531828773, 0.03689213820408396, 0.03706672322529063, 0.037241308246497296, 0.037415893267703955, 0.03759047828891062, 0.03776506331011729, 0.03793964833132395, 0.03811423335253061, 0.03828881837373728, 0.038463403394943946, 0.038637988416150605, 0.03881257343735727, 0.03898715845856393, 0.0391617434797706, 0.03933632850097726, 0.03951091352218393, 0.039685498543390596, 0.03986008356459726, 0.04003466858580393, 0.040209253607010595, 0.040383838628217254, 0.04055842364942392, 0.04073300867063058, 0.040907593691837246, 0.04108217871304391, 0.04125676373425058, 0.041431348755457245, 0.0416059337766639, 0.041780518797870564, 0.04195510381907723, 0.042129688840283896, 0.04230427386149057, 0.04247885888269723, 0.042653443903903895, 0.04282802892511056, 0.04300261394631722, 0.04317719896752389, 0.043351783988730554, 0.04352636900993721, 0.04370095403114388, 0.043875539052350546, 0.04405012407355721, 0.04422470909476388, 0.04439929411597054, 0.044573879137177204, 0.04474846415838387, 0.044923049179590537, 0.045097634200797196, 0.04527221922200386, 0.04544680424321053, 0.045621389264417195, 0.04579597428562386, 0.04597055930683052, 0.04614514432803718, 0.046319729349243846, 0.04649431437045051, 0.04666889939165718, 0.046843484412863845, 0.04701806943407051, 0.04719256456184452, 0.04736536676840916, 0.04753446267808822, 0.047696991448649737, 0.04784953848765512, 0.04799284096907562, 0.048127712917801824, 0.048257934523222495, 0.04838705366421733, 0.04851995197559876, 0.04865949840047511, 0.04880178465045004, 0.0489357994772595, 0.04905304538798107, 0.0491519464532862, 0.049234486275402736, 0.04930263064515607, 0.04935733149089569, 0.04939552771001872, 0.04941451823245213, 0.04941830757306315, 0.049410747020732684, 0.049392795273013504, 0.049367258833286985, 0.049339629147657244, 0.049311849604908836, 0.04928407006216041, 0.049256290519411994, 0.04922851097666357, 0.04920073143391515, 0.04917295189116673, 0.04914517234841831, 0.049117392805669895, 0.049089613262921473, 0.04906183372017306, 0.04903405417742463, 0.04900627463467622, 0.0489784950919278, 0.048950715549179374, 0.04892293600643097, 0.04889515646368254, 0.048867376920934125, 0.0488395973781857, 0.04881181783543728, 0.04878403829268886, 0.04875625874994044, 0.048728479207192026, 0.0487006996644436, 0.04867292012169519, 0.04864514057894676, 0.04861736103619835, 0.048589581493449926, 0.048561801950701505, 0.04853402240795309, 0.04850624286520466, 0.04847846332245625, 0.04845068377970783, 0.04842290423695941, 0.048395124694210985, 0.04836734515146257, 0.04833956560871415, 0.04831178606596573, 0.048284006523217314, 0.048256226980468886, 0.04822844743772048, 0.04820066789497206, 0.048172888352223636, 0.048145108809475215, 0.048117329266726794, 0.04808954972397837, 0.04806177018122996, 0.048033990638481544, 0.048006211095733116, 0.0479784315529847, 0.04795065201023628, 0.04792287246748786, 0.04789509292473944, 0.04786731338199102, 0.0478395338392426, 0.04781175429649418, 0.04778397475374576, 0.047756195210997346, 0.047728415668248925, 0.047700636125500503, 0.04767285658275208, 0.04764507704000366, 0.04761729749725524, 0.047589517954506826, 0.047561738411758404, 0.04753395886900998, 0.04750617932626157, 0.04747839978351315, 0.047450620240764727, 0.047422840698016305, 0.047395061155267884, 0.04736728161251948, 0.047339502069771056, 0.047311722527022634, 0.04728394298427421, 0.04725616344152579, 0.04722838389877737, 0.047200604356028956, 0.047172824813280535, 0.047145045270532114, 0.0471172657277837, 0.04708948618503528, 0.04706170664228686, 0.047033927099538436, 0.047006147556790015, 0.0469783680140416, 0.04695058847129318, 0.04692280892854476, 0.046895029385796344, 0.04686724984304792, 0.0468394703002995, 0.04681169075755108, 0.04678391121480266, 0.04675613167205424, 0.046728352129305824, 0.0467005725865574, 0.04667279304380899, 0.04664501350106057, 0.046617233958312146, 0.046589454415563725, 0.046561674872815303, 0.04653389533006689, 0.046506115787318475, 0.046478336244570054, 0.04645055670182163, 0.04642277715907321, 0.04639499761632479, 0.04636721807357637, 0.046339438530827955, 0.04631165898807953, 0.04628387944533112, 0.0462560999025827, 0.04622832035983428, 0.046200540817085856, 0.046172761274337434, 0.04614498173158901, 0.04611720218884059, 0.04608942264609218, 0.046061643103343757, 0.04603386356059534, 0.04600608401784692, 0.0459783044750985, 0.04595052493235008, 0.04592274538960166, 0.045894965846853236, 0.045867186304104815, 0.0458394067613564, 0.045811627218607986, 0.045783847675859565, 0.045756068133111144, 0.04572828859036272, 0.0457005090476143, 0.04567272950486588, 0.04564494996211747, 0.04561717041936905, 0.04558939087662063, 0.04556161133387221, 0.04553383179112379, 0.04550605224837537, 0.045478272705626946, 0.045450493162878525, 0.04542271362013011, 0.045394934077381696, 0.045367154534633275, 0.045339374991884854, 0.04531159544913643, 0.04528381590638801, 0.04525603636363959, 0.04522825682089117, 0.045200477278142755, 0.045172697735394333, 0.04514491819264592, 0.0451171386498975, 0.04508935910714908, 0.045061579564400656, 0.045033800021652234, 0.04500602047890381, 0.04497824093615539, 0.044950461393406985, 0.04492268185065856, 0.04489490230791014, 0.04486712276516172, 0.0448393432224133, 0.04481156367966488, 0.044783784136916464, 0.04475600459416805, 0.04472822505141963, 0.04470044550867121, 0.044672665965922786, 0.044644886423174365, 0.044617106880425944, 0.04458932733767752, 0.04456154779492911, 0.044533768252180694, 0.04450598870943227, 0.04447820916668385, 0.04445042962393543, 0.04442265008118701, 0.04439487053843859, 0.04436709099569017, 0.04433931145294175, 0.04431153191019333, 0.04428375236744492, 0.044255972824696496, 0.044228193281948075, 0.044200413739199654, 0.04417263419645123, 0.04414485465370281, 0.0441170751109544, 0.04408929556820598, 0.04406151602545756, 0.04403373648270914, 0.04400595693996072, 0.0439781773972123, 0.043950397854463884, 0.04392261831171546, 0.04389483876896704, 0.04386705922621863, 0.043839279683470206, 0.043811500140721785, 0.04378372059797336, 0.04375594105522494, 0.04372816151247652, 0.04370038196972811, 0.04367260242697968, 0.043644822884231264, 0.04361704334148285, 0.04358926379873443, 0.04356148425598601, 0.043533704713237587, 0.043505925170489165, 0.04347814562774075, 0.04345036608499233, 0.043422586542243916, 0.043394806999495494, 0.04336702745674707, 0.04333924791399865, 0.04331146837125023, 0.043283688828501816, 0.0432559092857534, 0.04322812974300498, 0.04320035020025656, 0.04317257065750814, 0.04314479111475972, 0.043117011572011296, 0.04308923202926288, 0.04306145248651446, 0.04303367294376604, 0.043005893401017625, 0.0429781138582692, 0.04295033431552078, 0.04292255477277236, 0.04289477523002394, 0.04286699568727552, 0.0428392161445271, 0.042811436601778684, 0.04278365705903027, 0.04275587751628185, 0.04272809797353343, 0.042700318430785006, 0.042672538888036585, 0.042644759345288163, 0.04261697980253975, 0.04258920025979133, 0.04256142071704291, 0.04253364117429449, 0.04250586163154607, 0.04247808208879765, 0.04245030254604923, 0.04242252300330081, 0.042394743460552387, 0.04236696391780398, 0.04233918437505556, 0.04231140483230714, 0.042283625289558716, 0.042255845746810294, 0.04222806620406188, 0.04220028666131346, 0.04217250711856504, 0.042144727575816616, 0.0421169480330682, 0.04208916849031978, 0.04206138894757136, 0.04203360940482294, 0.04200582986207452, 0.0419780503193261, 0.041950270776577675, 0.04192249123382926, 0.041894711691080846, 0.041866932148332425, 0.041839152605584004, 0.04181137306283558, 0.04178359352008716, 0.04175581397733874, 0.04172803443459032, 0.0417002548918419, 0.04167247534909349, 0.04164469580634507, 0.04161691626359665, 0.04158913672084823, 0.041561357178099806, 0.0415335776353514, 0.04150579809260298, 0.041478018549854556, 0.041450239007106135, 0.041422459464357714, 0.04139467992160929, 0.04136690037886087, 0.04133912083611246, 0.04131134129336403, 0.04128356175061562, 0.04125578220786719, 0.04122800266511878, 0.04120022312237036, 0.04117244357962194, 0.041144664036873516, 0.041116884494125094, 0.04108910495137668, 0.04106132540862826, 0.04103354586587984, 0.041005766323131417, 0.040977986780383, 0.04095020723763458, 0.04092242769488616, 0.04089464815213774, 0.04086686860938932, 0.0408390890666409, 0.04081130952389249, 0.04078352998114407, 0.040755750438395646, 0.040727970895647225, 0.040700191352898804, 0.04067241181015039, 0.040644632267401976, 0.04061685272465355, 0.04058907318190513, 0.04056129363915671, 0.04053351409640829, 0.04050573455365987, 0.04047795501091145, 0.040450175468163034, 0.04042239592541461, 0.0403946163826662, 0.04036683683991778, 0.04033905729716935, 0.040311277754420935, 0.040283498211672514, 0.0402557186689241, 0.04022793912617567, 0.04020015958342725, 0.040172380040678836, 0.04014460049793042, 0.040116820955182, 0.04008904141243358, 0.04006126186968516, 0.04003348232693674, 0.04000570278418832, 0.03997792324143991, 0.03995014369869149, 0.039922364155943066, 0.039894584613194645, 0.03986680507044622, 0.0398390255276978, 0.03981124598494939, 0.03978346644220096, 0.039755686899452546]
  in  "Tab APD Timing":enum32{"Timing", "MCL Scan", "Analog Out"}(tab)=enum."MCL Scan"
  out "APD 2 Gate Late Counter":u8
  out "APD 2 Gate Relative Phase":i16
  in  "Phase Adj. (APD 2 Gate)":i16=20
  in  "Initial Phase Adjustment (APD 2 Gate)":i16=45
  out "APD 1 Gate Late Counter":u8
  in  "- phase (APD 1 Gate)":bool
  in  "+ phase (APD 1 Gate)":bool
  out "APD 1 Gate Relative Phase":i16
  in  "Phase Adj. (APD 1 Gate)":i16=20
  in  "Initial Phase Adjustment (APD 1 Gate)":i16=50
  in  "Save APD":bool=TRUE
  out "APD FIFO Elements Remaining":u32
  in  "- phase (APD Acq)":bool
  in  "+ phase (APD Acq)":bool
  out "APD Acq Late Counter":u16
  out "APD Acq Relative Phase":i16
  in  "Phase Adj. (APD Acq)":i16=20
  in  "Initial Phase Adjustment (APD Acq)":i16
  in  "Invert APD Gate":bool caption="Invert Gate"
  in  "APD Gate OFF Count":u32=450 caption="Gate OFF Count"
  in  "APD Gate ON Count":u32=150 caption="Gate ON Count"
  in  "APD Gate":enum32{"ON", "OFF", "Interlace"}(radio)=enum."Interlace"
  in  "APD Integration Time (s)":dbl=0.01 caption="Integration Time (s)"
  out "APD Acq Rate (Hz)":dbl=100.0 caption="Rate (Hz)"
  out "APD Samples/FIFO Acq.":dbl=30.0
  out "APD Elements/DMA read":u32=60
  out "APD Int. Count":u32=400000 format="%.0p"
  in  "+ phase (APD 2 Gate)":bool
  in  "- phase (APD 2 Gate)":bool
  in  "APD FIFO Depth (requires restart)":u32=300000 format="%.0p"
  in  "Abort MCL Scan":bool
  out "MCL Scan I":u64=2
  out "MCL Scanning":bool
  in  "Start MCL Scan":bool
  out "wait to reset values":bool
  in  "Tab MCL Scan Settings":enum32{"Scan Settings", "MCL FPGA Loop Timing"}(tab)
  out "Total Time (s)":dbl=48.0
  in  "Scan lines (y)":u64=20
  in  "Fast Scan Dir":bool=TRUE
  in  "2D or 1D Scan":bool=TRUE
  out "Initial X":dbl=1.6310662274449115
  out "Initial Y":dbl=2.5691326639606933
  out "Time/f+b scan (s) (MCL)":dbl=2.4 caption="Time/scan (s)"
  in  "Number of scans (MCL)":u64=1 caption="Scans"
  in  "Scan steps (x)":u64=40
  in  "N APD Samp/step":i32=3
  in  "Scan Range (V)\n(of steps)":dbl=3.5
  in  "Restart DMA? (MCL)":bool=TRUE caption="Restart DMA?"
  in  "Continuous MCL Scanning":bool caption="Cont. Scanning"
  in  "Center Scan":bool=TRUE
  in  "Save Data (MCL)":bool=TRUE caption="Save Data"
  out "Actual Incr. int (MCL)":i16=462 caption="Incr. int"
  out "Desired incr (int)":dbl=462.098717948718
  out "Desired Scan Incr (V)":dbl=0.14102564102564102
  out "N sets should be saved (MCL)":dbl=160.0 caption="N sets should be saved"
  out "Data points/scans (MCL)":dbl=4800.0 caption="Data points/scans"
  out "Data points/scan (f+b)":dbl=240.0 caption="points/scan (f+b)"
  out "Cycles/step (MCL)":u64=2000 caption="Cycles/step" format="%.0p"
  out "Actual MCL Inc (V)":dbl=0.14099551377910702
  in  "Phase adjust (MCL)":i16 caption="Phase adjust"
  out "Relative Phase (MCL)":i16 caption="Relative Phase"
  in  "Initial Phase Adj. (MCL)":i16 caption="Initial Phase Adj."
  in  "Update Count (MCL)":u32=600
  in  "+ phase (MCL)":bool
  in  "- phase (MCL)":bool
  out "MCL Late Counter":u8
  in  "APD 1 AO Mult.":i16=1 min=1
  in  "APD 2 AO Mult.":i16=1 min=1
  in  "Tab Green FB":enum32{"Green FB Signals", "Slow MCL Scan"}(tab)
  out "Green FB Plot":dbl(graph)=-10.00030518509476
  out "MCL Scan 2":cluster{"Begin (V)":dbl, dbl, dbl[]}(graph)
  out "MCL Scan":cluster{"Begin (V)":dbl, dbl, dbl[]}(graph)
  in  "GI Frequency, ON count":u32=150 min=1 step=1
  in  "Invert GI":bool
  out "GI Late Counter":u8
  in  "Phase adj. (GI)":i16=5
  out "GI relative phase":i16
  in  "+ phase (GI)":bool
  in  "Initial Phase Adjustment (GI)":i16=4
  in  "GI Frequency, OFF count":u32=450 min=1 step=1
  in  "- phase (GI)":bool
  out "Green FB Signals (V)":cluster{"Y":dbl, "X":dbl, "Sum":dbl}={"Y"=-0.999969482421875, "X"=1.0, "Sum"=-10.00030518509476}
  out "Relative phase (Green FB)":i16
  in  "+ phase (Green FB)":bool
  in  "- phase (Green FB)":bool
  in  "Green FB Count":u32=600
  in  "Phase adj. (Green FB)":i16=10
  in  "Initial Phase Adjustment (Green FB)":i16=50
  in  "Green FB On/Off":bool
  in  "Green int current ON count adj":u32=150
  in  "Green FB Gains":T10={"proportional gain (Kc)"=10, "integral gain (Kc*Ts/Ti)"=5, "derivative gain (Kc*Td/Ts)"=0}
  in  "Green FB Setpoint (mV)":dbl=100.0
  in  "- phase (GI) 2":bool
  in  "Initial Phase Adjustment (GI) 2":i16=-100
  in  "+ phase (GI) 2":bool
  out "GI relative phase 2":i16
  in  "Phase adj. (GI) 2":i16=20
  out "GI Late Counter 2":u16
  in  "Trap Position FIFO Depth":u32=300000 format="%.0p"
  in  "# Samples/trap":u32=20000 format="%.0p"
  out "Trap AI Elements/DMA read":u32=320000 format="%.0p"
  out "Ave. Rate (Hz)":dbl=200000.0 format="%#_6p"
  out "Trap AI FIFO El. Rem.":u32 format="%.0p"
  in  "Phase adj. (AI1)":i16
  out "Relative phase (AI1)":i16
  in  "+ phase (AI1)":bool
  in  "- phase (AI1)":bool
  out "Late Counter (AI1)":u8
  in  "Initial Phase Adjustment (AI1)":i16=185
  out "AI rate (Hz)":dbl=200000.0 format="%#_6p"
  in  "AI Count (ticks)":u32=200
  out "# Samples/channel":u32=40000 format="%.0p"
  in  "Trap AI FIFO Depth":u32=340000 format="%.0p"
  in  "Detector Type":string(combo)="UCB Fleezers 052511"
  in  "N Acq Sets (Traps + Fl.)":i16=3
  in  "Sets to FIFO (Traps)":T15={"Set 1"=TRUE, "Set 2"=TRUE, "Set 3"=FALSE}
  in  "FPGA Ave.":dbl=1.0 min=1.0 step=1.0
  out "Ave. Period (s)":dbl=5e-06 format="%#_6p"
  out "DMA Update Period (s)":dbl=0.3
  out "FPGA Averaging":bool
  out "Trap Sets":u32=2
  out "Counts/DMA":dbl=12000000.0 format="%#_6p"
  out "Trap Pos FIFO El Remaining":u32=171
  out "Trap Pos Elements/DMA read":u32=120000 format="%.0p"
  out "Trap AI FIFO Timeout":u16
  out "Trap Pos FIFO Timeout":u16
  in  "AOM X Cal (nm/MHz)":dbl=160.0
  in  "MCL X Cal (nm/V)":dbl=1174.0
  out "X RF Amplitude Limits (%)":T16={"Minimum"=0.0, "Maximum"=75.0, "Increment"=1.0}
  out "X RF Frequency Limits (MHz)":T16={"Minimum"=60.0, "Maximum"=90.0, "Increment"=1.0}
  out "Y RF Frequency Limits (MHz)":T16={"Minimum"=60.0, "Maximum"=90.0, "Increment"=1.0}
  out "Y RF Amplitude Limits (%)":T16={"Minimum"=0.0, "Maximum"=75.0, "Increment"=1.0}
  in  "Manip. X?":bool=TRUE
  in  "Manip. Y?":bool
  in  "Force Manip Abort":bool
  out "Read cal error":errorcluster
  in  "DAQ Delay (ms)":u32=1000
  in  "Start Scan":bool
  in  "Scan axis":bool
  in  "Osc. amp. (V)":dbl=5.0
  in  "Osc. center (V)":dbl=5.0
  in  "Osc. freq. (Hz) 2":dbl=1.0
  in  "MCL Mode":u16(ring) items=["Manual Positioning", "Sinusoidal Wave", "Linear Scan"]
  in  "Begin (V)":dbl
  in  "End (V)":dbl=10.0
  in  "N Points":dbl=20.0
  in  "Delay to Interlace (s)":dbl
  in  "Delayed Interlace Start":bool
  in  "Read Lateness and Rel Phase":bool
  in  "Cal read wait (s)":u32=5
  out "Time tether formed":timestamp=timestamp(3371146929.513132 s since 1904-01-01)
  in  "Chemyx Syringe Pump Serial Port":refnum<visa-resource-name>="ASRL3::INSTR"
  in  "Limit Min (MHz)":dbl=10.0 caption="Min (MHz)"
  in  "Limit Max (MHz)":dbl=16.0 caption="Max (MHz)"
  in  "Limits Enable":bool=TRUE caption="Enable"
  out "AI labels":string[](array[string])=["T1 Y", "T1 X", "T1 Sum", "T2 Y", "T2 X", "T2 Sum", "T1 FB X", "T2 FB Sum", "T2 FB X", "T2 FB Sum", "PSD Y", "PSD X", "PSD Sum"]
  in  "Save TPos":bool=TRUE
  in  "ESP Port":refnum<visa-resource-name>="COM4"
  in  "Axis 3":string="0.00500\r\n"
  in  "Axis 2":string="0.00500\r\n"
  in  "Axis 1":string="0.00500\r\n"
  in  "Axis 3":string="0.20000\r\n"
  in  "Axis 2":string="0.20000\r\n"
  in  "Axis 1":string="0.20000\r\n"
  in  "Activate Joystick":bool
  in  "ESP ZL-Limit":string="-0.09900"
  in  "ESP ZR-Limit":string="0.09900"
  in  "error in":errorcluster
  out "error out":errorcluster
  out "Current MCL (V)":dbl=5.657514378627918
  in  "Tracking factor":dbl=-0.45
  out "Zero T1 position":dbl=70.0
  out "Zero MCL x position":dbl=5.6547922360429315
  out "Error Events":errorcluster
  # "Hidden Controls"
  # "TO BE MOVEDDDD"
  # "After"
  # "During"
  # "Trap On?"
  # "BD Flow ON?"
  # "Samp Flow ON?"
  # "1"
  # "2"
  # "Trap Display:"
  # "APD Display:"
  # "originally 10k"
  # "Data Saving"
  # "Trap Manipulation"
  # "DAQ"
  # "Central frequency 80 MHz"
  # "INS"
  # "DEL"
  # "Bead Calibration"
  # "Current Location"
  # "Select the chamber to go to"
  # "Harvard Pump\n(sample channel for flow exp)"
  # "Chemyx Pump 2"
  # "Units: \n1 = ml/m\n2 = ml/h\n3 = ul/m\n4 = ul/h"
  # "Rate param is ul/h\nVolume param is ul"
  # "Trap interlacing RF phase control\n\n0 = no phase control\n1 = offset increments each trap cycle by values below\n2 = offset increment increases by increment factor each cycle\n3 = random phase (no parameters set)"
  # "Oscillate Set 2 freq. (debugging)"
  # "BD 1"
  # "BD 2"
  # "X"
  # "Y"
  # "AOD Raster Scan"
  # "Approx. trap separations"
  # "X"
  # "Y"
  # "DON'T TURN ON\nUNTIL YOU CLOSE\nTHE LOOP"
  # "FPGA\nreading"
  # "DMA\ntransfer"
  # "APD Gates"
  # "APD 2"
  # "APD 1"
  # "X"
  # "2D"
  # "Y"
  # "1D"
  # "Green FB Measurement"
  # "Green Laser Interlacing"
  # "Digital Gate"
  # "Current Analog Control"
  # "was 87"
  # "originally 600k"
  # "Total AI Rates (NOT rates/trap)"
  # "originally 20k"
  # "(Samples/trap x Trap Sets)"
  # "(Samples/channel x\n8 if averaging (8 channels)\n4 if no averaging)"
  # "Trap 1"
  # "Trap 2"
  # "Flour./Trap 3"
  # "MCL Position Debugging"
  # "Temporary Control Storage\n(these used to be somewhere else, still want to keep them)"
  # "Y"
  # "X"
  # "Trap Position Difference Limits"
  # "Joystick Control"
  # "Setting Limit for the z-axis"
  # "Errors detected in determing Current Location"
  # "High Jog Velocity"
  # "Low Jog Velocity"
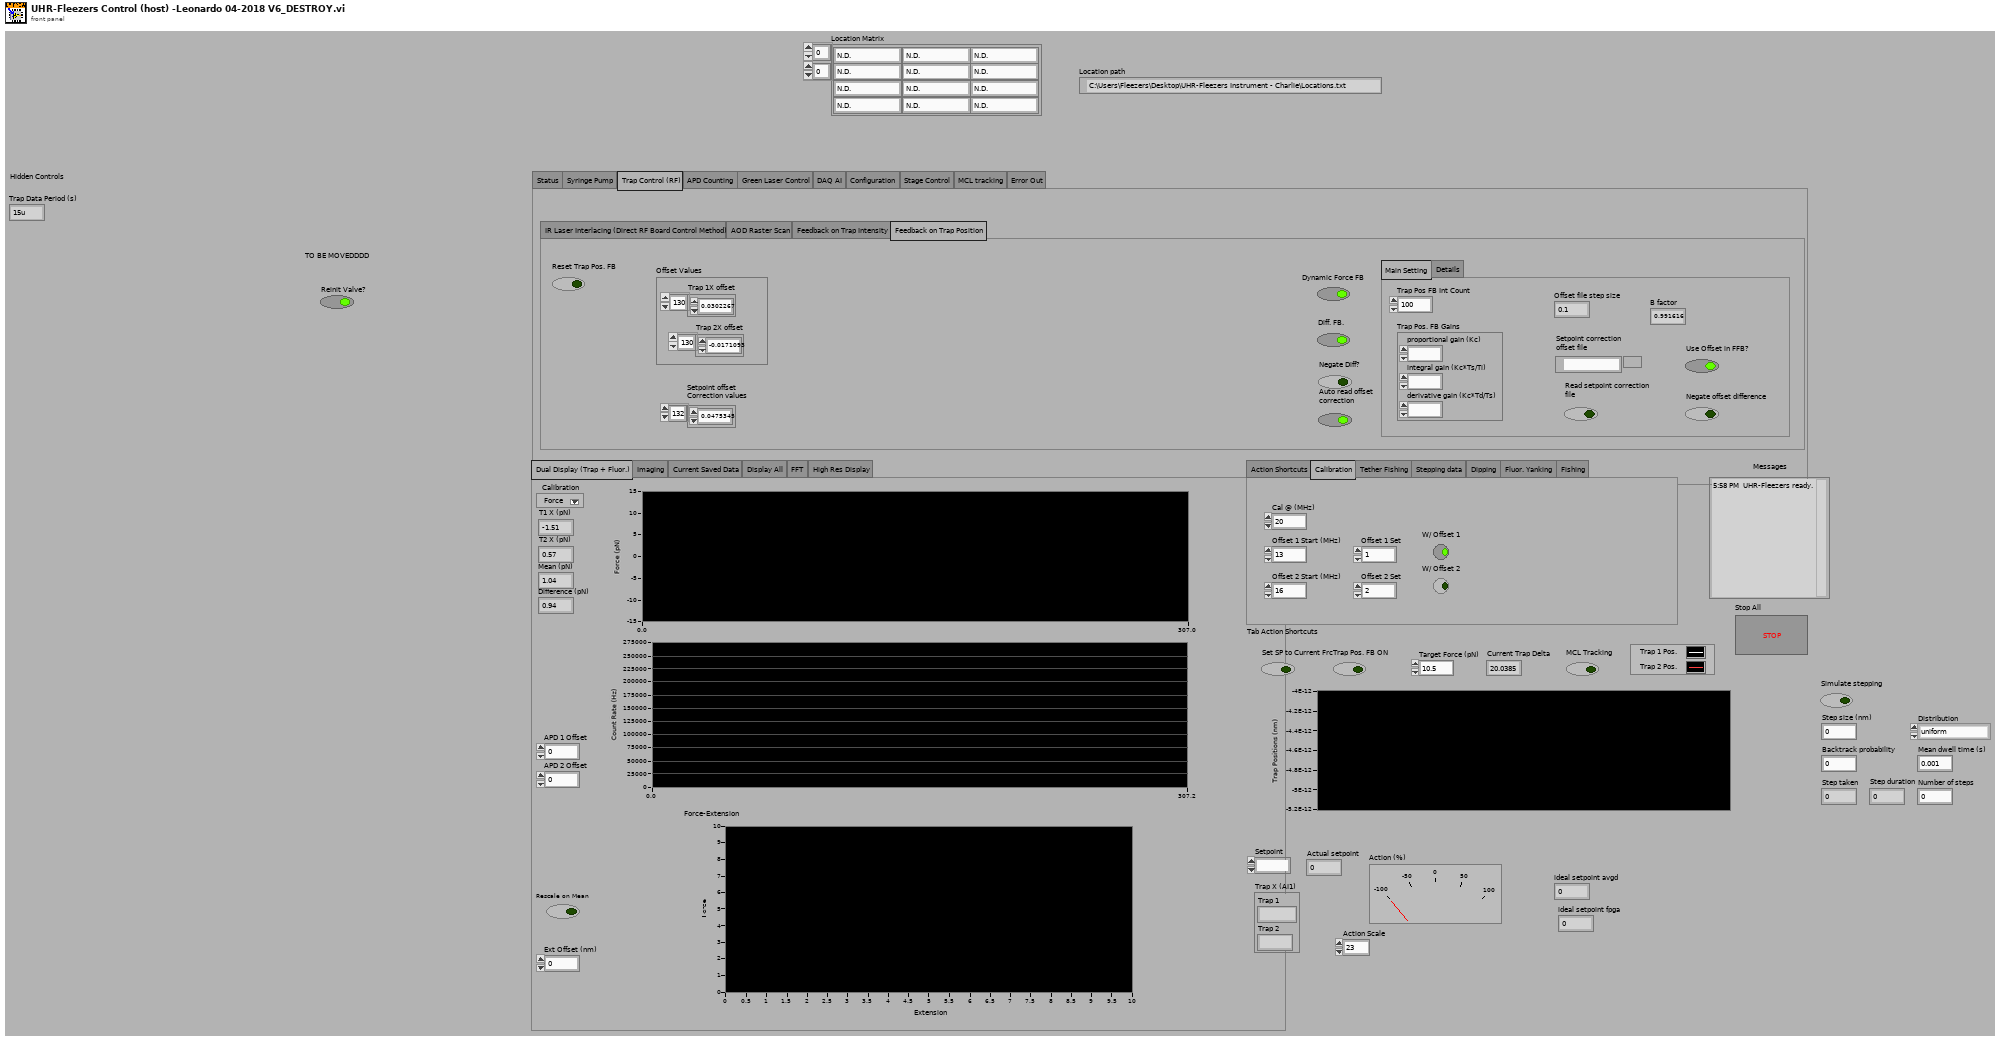
[diagram p1: front panel]
types:
  T1 = cluster{"Trap 1":fxp<+/-,16,1>, "Trap 2":fxp<+/-,16,1>}
  T2 = enum32{"Action Shortcuts", "Calibration", "Tether Fishing", "Stepping data", "Dipping", "Fluor. Yanking", "Fishing"}
  T3 = enum32{"Dual Display (Trap + Fluor.)", "Imaging", "Current Saved Data", "Display All", "FFT", "High Res Display"}
  T4 = typedef "IMAQ Image.ctl" = refnum<image>
  T5 = enum32{"Status", "Syringe Pump", "Trap Control (RF)", "APD Counting", "Green Laser Control", "DAQ AI", "Configuration", "Stage Control", "MCL tracking", "Error Out"}
  T6 = cluster{"Pump 1":cluster{"Diameter (mm)":dbl, "Units":dbl, "Volume":dbl, "Rate":dbl}, "Pump 2":cluster{"Diameter (mm)":dbl, "Units":dbl, "Volume":dbl, "Rate":dbl}, "Pump 3":cluster{"Diameter (mm)":dbl, "Units":dbl, "Volume":dbl, "Rate":dbl}}
  T7 = enum32{"IR Laser Interlacing (Direct RF Board Control Method)", "AOD Raster Scan", "Feedback on Trap Intensity", "Feedback on Trap Position"}
  T8 = typedef "LVPoint32TypeDef.ctl" = cluster{"Horizontal":i32, "Vertical":i32}
  T9 = cluster{"Scan Range AOD (nm) 2":dbl, "Step Size AOD (nm) 2":dbl, "Scan Speed AOD (nm/s) 2":dbl, "Number of scans (AOD) 2":u16, "Label":string}[]
  T10 = cluster{"proportional gain (Kc)":i16, "integral gain (Kc*Ts/Ti)":i16, "derivative gain (Kc*Td/Ts)":i16}
  T11 = cluster{"proportional gain (Kc)":fxp<+/-,16,8>, "integral gain (Kc*Ts/Ti)":fxp<+/-,16,8>, "derivative gain (Kc*Td/Ts)":fxp<+/-,16,8>}
  T12 = cluster{"output high":fxp<+/-,16,1>, "output low":fxp<+/-,16,1>}
  T13 = cluster{"Set 1":fxp<+/-,16,1>, "Set 2":fxp<+/-,16,1>}
  T14 = cluster{"Trap 1X offset":dbl[], "Trap 2X offset":dbl[]}
  T15 = cluster{"Set 1":bool, "Set 2":bool, "Set 3":bool}
  T16 = typedef "LVMinMaxIncTypeDef.ctl" = cluster{"Minimum":dbl, "Maximum":dbl, "Increment":dbl}
  T17 = typedef "Image Type" = u32
  T18 = typedef "nirio_resource_hc.ctl" = tag
  T19 = typedef "openfpgaref.initrf.ctl" = refnum<k20>
  T20 = typedef "openfpgaref.8.6.ctl" = refnum<k20>
  T21 = typedef "XDNodeRunTimeDep.lvlib/timing_clust.ctl" = cluster{"Expected End [f-1]":u64, "Actual End [f-1]":u64, "Finished Late? [f-1]":bool, "Expected End [i-1]":u64, "Actual End [i-1]":u64, "Finished Late? [i-1]":bool, "Expected Start [i]":u64, "Actual Start [i]":u64, "Expected Start [f]":u64, "Actual Start [f]":u64, "Source Name":string, "Structure Name":string, "Period":i64, "Deadline":i64, "Offset":i64, "Start":i64, "Priority":i32, "Timeout":i32, "Mode":T22, "Wakeup Reason":T23, "Error":errorcluster, "Source Type":string, "Secondary Source Type":string, "Global End Time":u64, "Global Start Time":u64, "Frame Duration":u64, "Iteration Duration":u64, "Assigned CPU":i32, "I/O Scan Engine Mode":u32}
  T22 = typedef "XDNodeRunTimeDep.lvlib/nitl_modes.ctl" = enum32{"No Change", "Process missed periods, maintain original phase", "Discard missed periods, maintain original phase", "Process missed periods, ignore original phase", "Discard missed periods, ignore original phase"}
  T23 = typedef "XDNodeRunTimeDep.lvlib/wakeup.ctl" = enum32{"Normal", "Aborted", "Asynchronous wakeup", "Timing source error", "Timed loop error", "Timeout"}
  T24 = cluster{"Location Matrix[0]":string, "Location Matrix[1]":string, "Location Matrix[2]":string}
  T25 = enum16{"CONNECT", "INITIALIZE VALVES", "DISCONNECT", "MOVE VALVE"}
  T26 = cluster{"Left":i32, "Top":i32, "Width":u32, "Height":u32}
  T27 = cluster{cluster{"Left":i32, "Top":i32, "Width":u32, "Height":u32}}[]
  T28 = cluster{"New Image":T4, "New Image":T4, "New Image":T4, "New Image":T4}
  T29 = enum16{"open", "replace", "create", "open or create", "replace or create", "replace or create with confirmation"}
  T30 = enum16{"big-endian, network order", "native, host order", "little-endian"}
  T31 = cluster{"Scan Range AOD (nm) 2":dbl, "Step Size AOD (nm) 2":dbl, "Scan Speed AOD (nm/s) 2":dbl, "Number of scans (AOD) 2":u16, "Label":string}
  T32 = cluster{"[0]":dbl, "[1]":dbl, "[2]":dbl, "[3]":dbl, "[4]":dbl, "[5]":dbl}
  T33 = cluster{"Diameter (mm)":dbl, "Units":dbl, "Volume":dbl, "Rate":dbl}
  T34 = cluster{"averaging mode":u16, "weighting mode":u16, "number of averages":u32}
  T35 = cluster{"dB On (F)":bool, "unwrap phase (F)":bool, "convert to degree (F)":bool}
  T36 = cluster{"Green FB Ch 0":i16, "Green FB Ch 1":i16, "Green FB Ch 2":i16}
  T37 = cluster{"f0":dbl, "df":dbl, "magnitude":dbl[]}[][]
  T38 = cluster{"Green FB Ch 0":dbl, "Green FB Ch 1":dbl, "Green FB Ch 2":dbl}
  T39 = cluster{"Label.Text":string, "Label.Text":string, "Label.Text":string, "Label.Text":string, "Label.Text":string}
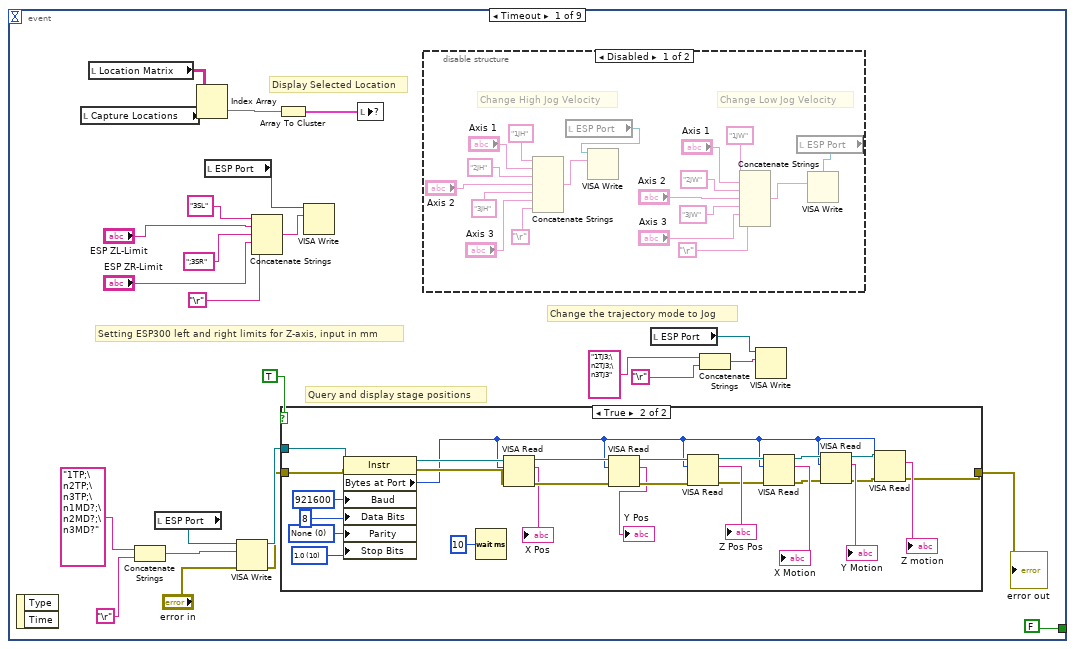
[diagram p2: hidden frame]
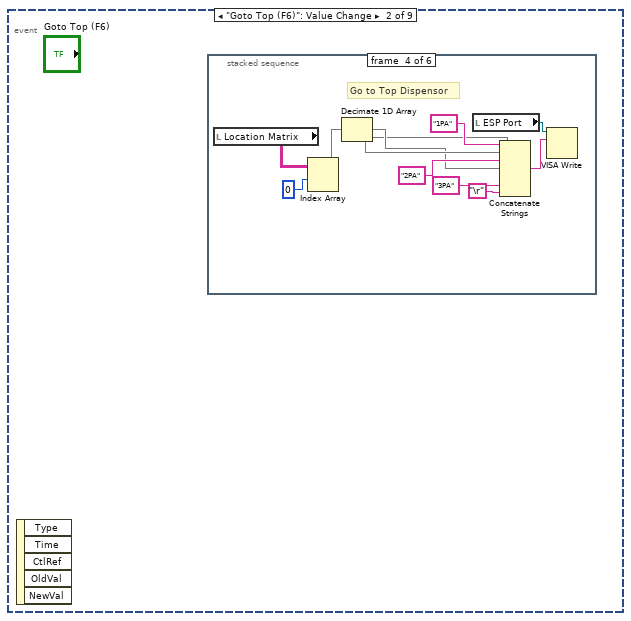
[diagram p5: hidden frame]
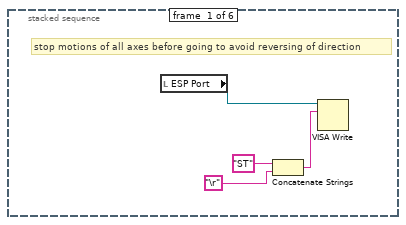
[diagram p6: hidden frame]
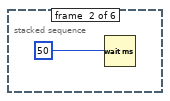
[diagram p7: hidden frame]
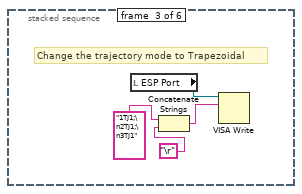
[diagram p8: hidden frame]
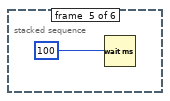
[diagram p9: hidden frame]
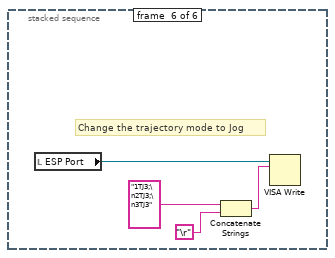
[diagram p10: hidden frame]
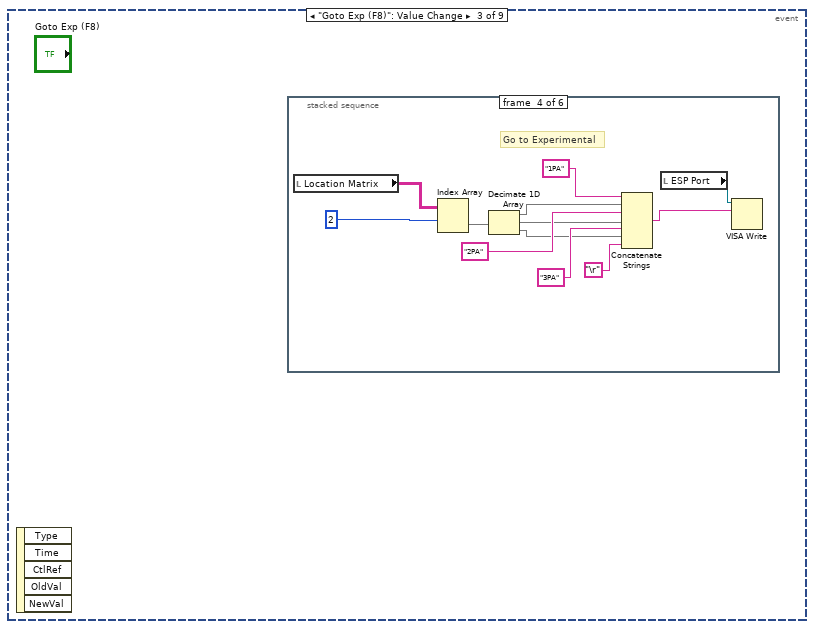
[diagram p11: hidden frame]
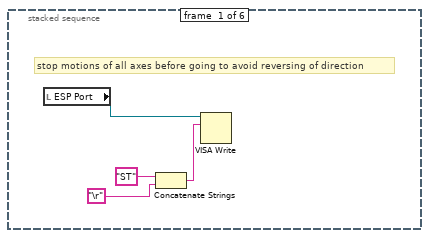
[diagram p12: hidden frame]
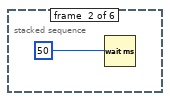
[diagram p13: hidden frame]
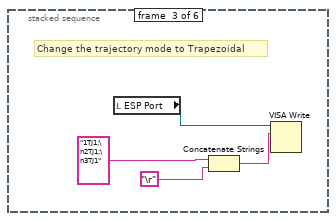
[diagram p14: hidden frame]
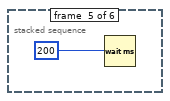
[diagram p15: hidden frame]
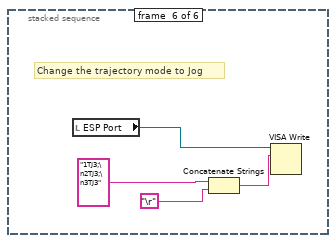
[diagram p16: hidden frame]
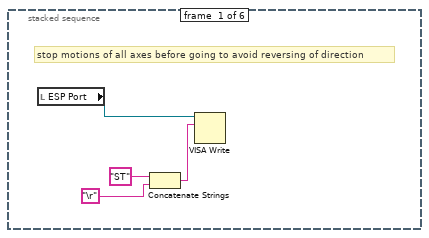
[diagram p17: hidden frame]
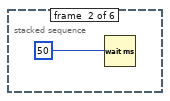
[diagram p18: hidden frame]
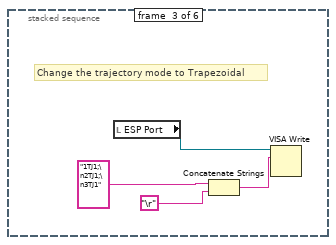
[diagram p19: hidden frame]
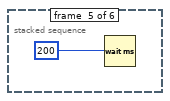
[diagram p20: hidden frame]
diagram:
  w9 = u16 0 items=["Off", "Approach", "Wiggle", "Extend", "Tether Found"] ("Fish Status")
  w79 = T17 2 items=["Grayscale (U8)", "Grayscale (I16)", "Grayscale (SGL)", "Complex (CSG)", "RGB (U32)", "HSL (U32)", "RGB (U64)", "Grayscale (U16)"] ("Image Type")
  w201 = 10.0 ("y")
  w200 = 32767.0 ("y")
  w216 = 6.0  # clock mult.
  w217 = 49152000.0  # TCXO frequ.
  # "Orphaned Controls"
  n1 = flat-sequence "FPGA bitfile init" {
    tunnel: [w248] -> w29
    tunnel: w29 -> [w263]
    tunnel: [w257] -> w148
    tunnel: [w256] -> w131
    frame #0 {
      w248 = T18 "RIO0" ("resource name")
      n2 = xnode "Open FPGA VI Reference"("resource name"=w248) -> ("FPGA VI Reference Out"=w255:T19)  [unwired: 1 in, 1 out]
      n3 = xnode "Invoke Method"("FPGA VI Reference In"=w255) -> ("FPGA VI Reference Out"=w254:T19, "error out"=w253:errorcluster)  [unwired: 1 in]
      n4 = xnode "Invoke Method"("FPGA VI Reference In"=w254, "error in"=w253) -> ("FPGA VI Reference Out"=w251:T19, "error out"=w252:errorcluster)  [unwired: 1 in]
      n5 = call "Initialize RF boards - with FPGA init only vi v1.vi"("error in"=w252, "FPGA Interface"=w251) -> ("error out"=w249:errorcluster, "FPGA Interface 2"=w250:T19)
      n6 = xnode "Close FPGA VI Reference"("FPGA VI Reference In"=w250, "error in"=w249) -> ()  [unwired: 1 out]
    }
    frame #1 {
      w258 = TRUE
      n7 = xnode "Open FPGA VI Reference"("resource name"=w263) -> ("FPGA VI Reference Out"=w262:T20, "error out"=w261:errorcluster)  [unwired: 1 in]
      n8 = xnode "Invoke Method"("FPGA VI Reference In"=w262, "error in"=w261) -> ("FPGA VI Reference Out"=w260:T20, "error out"=w259:errorcluster)
      n9 = xnode "Read/Write Control"("FPGA VI Reference In"=w260, "error in"=w259, "PMODE"=w258, "RD"=w258) -> ("FPGA VI Reference Out"=w256:T20, "error out"=w257:errorcluster)
      "FPGA error out" <- w257
    }
  }
  n10 = Build Array("DIO count 1 (ticks)", "DIO count 2 (ticks)", "DIO count 3 (ticks)") -> (w123:u32[])
  n11 = disable-structure shown="Enabled" {
    disable-tunnel: [w265 _] -> w54
    disable-tunnel: w49 -> [w264 _]
    frame Enabled {
      n12 = node-c288() -> (w267:T21)  [unwired: 4 out]
      n13 = timed-loop "Rough control of MCL mirror stage (debugging)" {
        tunnel: w264 -> [w270]
        tunnel: [w269] -> w265
        timing: w267 -> [_]
        timing-out: [_] -> w266
        stop <- w269 stop-if-true
        n14 = node-c288() -> ()  [unwired: 2 out]
        n15 = case shown="0, Default" "MCL Mode" {
          tunnel: w270 -> [_ w273 w312]
          frame 0, Default {
            # "manual positioning"
          }
          frame 1 {
            # "sinusoidal wave"
            n16 = node-c288() -> (w275:T21)  [unwired: 4 out]
            n17 = timed-loop "Oscillate MCL mirror" {
              timing: w275 -> [_]
              timing-out: [_] -> w274
              tunnel: w273 -> [w306]
              i -> [w305]
              stop <- w280 stop-if-true
              n18 = node-c288() -> (w304:i64)  [unwired: 1 out]
              n19 = call "V2int16.vi"("InV"="MCL X") -> ("Out i16"=w276:i16)  [unwired: 4 in]
              n20 = call "V2int16.vi"("InV"="MCL Y") -> ("Out i16"=w278:i16)  [unwired: 4 in]
              n21 = Divide(x=w304, y=i64 1000) -> (x/y=w287:dbl)
              n22 = Multiply(x=w287, y=w305) -> (x*y=w298:dbl)
              n23 = Multiply(x="Osc. freq. (Hz) 2", y=6.283185307179586) -> (x*y=w299:dbl)
              n24 = Multiply(x=w299, y=w298) -> (x*y=w297:dbl)
              n25 = Sine(x=w297) -> (sin(x)=w296:dbl)
              n26 = Multiply(x=w296, y="Osc. amp. (V)") -> (x*y=w294:dbl)
              n27 = Add(x=w294, y="Osc. center (V)") -> (x+y=w292:dbl)
              n28 = Divide(x=w292, y=10.0) -> (x/y=w290:dbl)
              n29 = Multiply(x=w290, y=32767.0) -> (x*y=w285:dbl)
              n30 = Select(t=w285, s="Scan axis", f=w278) -> (s? t:f=w303:dbl)
              n31 = Select(t=w276, s="Scan axis", f=w285) -> (s? t:f=w302:dbl)
              n32 = local read "MCL Mode"() -> (w284:u16)
              n33 = Not Equal?(x=w284, y=u16 1) -> (x != y?=w281:bool)
              n34 = local read "Stop All"() -> (w282:bool)
              n35 = xnode "Read/Write Control"("FPGA VI Reference In"=w306, "AO1 (Y)"=w303, "AO2 (X)"=w302) -> ()  [unwired: 1 in, 2 out]
              n36 = Compound Arithmetic op=OR(w282, w281) -> (w280:bool)
              n37 = node-c288() -> ()  [unwired: 2 out]
            }
            n38 = node-c288(w274) -> ()  [unwired: 1 out]
          }
          frame 2 {
            # "linear scan"
            n39 = case shown="False" "Start Scan" {
              tunnel: w312 -> [_ w322]
              frame False {
              }
              frame True {
                n40 = Subtract(x="End (V)", y="Begin (V)") -> (x-y=w318:dbl)
                n41 = Decrement(x="N Points") -> (x-1=w317:dbl)
                n42 = Divide(x=w318, y=w317) -> (x/y=w315:dbl)
                n43 = for {
                  N: "N Points" -> [_]
                  tunnel: "Begin (V)" -> [w335]
                  tunnel: w322 -> [w327]
                  tunnel: [w326] -> w321 mode=indexing
                  tunnel: w315 -> [w325]
                  tunnel: [w323] -> w314 mode=indexing
                  i -> [w334]
                  n44 = Multiply(x=w325, y=w334) -> (x*y=w333:dbl)
                  n45 = Add(x=w335, y=w333) -> (x+y=w330:dbl)
                  n46 = local read "MCL Y"() -> (w332:dbl)
                  n47 = local read "MCL X"() -> (w331:dbl)
                  n48 = local read "Scan axis"() -> (w324:bool)
                  n49 = Select(t=w330, s=w324, f=w332) -> (s? t:f=w329:dbl)
                  n50 = Select(t=w331, s=w324, f=w330) -> (s? t:f=w328:dbl)
                  n51 = flat-sequence {
                    tunnel: w329 -> [w339]
                    tunnel: w328 -> [w338]
                    tunnel: w327 -> [w336]
                    tunnel: [w348] -> w326
                    tunnel: [w348] -> w323
                    frame #0 {
                      w342 = 10.0 ("y")
                      w337 = 32767.0 ("y")
                      n52 = Multiply(x=w339, y=w337) -> (x*y=w345:dbl)
                      n53 = Multiply(x=w338, y=w337) -> (x*y=w343:dbl)
                      n54 = Divide(x=w345, y=w342) -> (x/y=w346:dbl)
                      n55 = Divide(x=w343, y=w342) -> (x/y=w344:dbl)
                      n56 = To Word Integer(number=w346) -> (16bit integer=w340:i16)
                      n57 = To Word Integer(number=w344) -> (16bit integer=w341:i16)
                      n58 = xnode "Read/Write Control"("FPGA VI Reference In"=w336, "AO1 (Y)"=w340, "AO2 (X)"=w341) -> ()  [unwired: 1 in, 2 out]
                    }
                    frame #1 {
                      n59 = Wait (ms)(milliseconds to wait="DAQ Delay (ms)") -> ()  [unwired: 1 out]
                    }
                    frame #2 {
                      w348 = 0.0
                      # "BROKE IT\n-AT"
                    }
                  }
                }
                n60 = Bundle("Begin (V)"="Begin (V)", w315, w321) -> ()  [unwired: 2 out]
                n61 = Bundle("Begin (V)"="Begin (V)", w315, w314) -> ()  [unwired: 2 out]
              }
            }
          }
        }
        n62 = local read "Stop All"() -> (w269:bool)
        n63 = node-c288() -> ()  [unwired: 2 out]
      }
      n64 = node-c288(w266) -> ()  [unwired: 1 out]
    }
    frame Disabled {
    }
  }
  n65 = Multiply(x="APD Integration Time (s)", y=40000000.0) -> (x*y=w139:dbl)
  n66 = Reciprocal(x="APD Integration Time (s)") -> (1/x=w136:dbl)
  n67 = local write "APD Acq Rate (Hz)"(w136) -> ()
  n68 = local read "MCL Y"() -> (w195:dbl)
  n69 = local read "MCL X"() -> (w194:dbl)
  n70 = local read "Dynamic Force FB"() -> (w31:bool)
  n71 = local read "Negate Diff?"() -> (w30:bool)
  n72 = To Unsigned Long Integer(number=w139) -> (unsigned 32bit integer=w138:u32)
  "APD Int. Count" <- w138
  n73 = local read "Diff. FB."() -> (w32:bool)
  n74 = local read "Scan Increment (MHz)"() -> (w212:dbl)
  n75 = local read "Continuous MCL Scanning"() -> (w182:bool)
  n76 = local read "Fast Scan Dir"() -> (w181:bool)
  n77 = local read "Trap Intensity\nSetpoints (V)"() -> (w226:cluster{"Set 1":dbl, "Set 2":dbl})
  n78 = local read "Number of scans (MCL)"() -> (w183:u64)
  n79 = Multiply(x=w195, y=w200) -> (x*y=w197:dbl)
  n80 = Multiply(x=w194, y=w200) -> (x*y=w199:dbl)
  n81 = Divide(x=w197, y=w201) -> (x/y=w196:dbl)
  n82 = Divide(x=w199, y=w201) -> (x/y=w198:dbl)
  n83 = flat-sequence "Set RF Freq/Amp Limits" {
    tunnel: w131 -> [w355]
    tunnel: [w355] -> w130
    tunnel: [w352] -> w33
    tunnel: [w354] -> w129
    tunnel: [w351] -> w127
    tunnel: [w353] -> w128
    frame #0 {
      w353 = T16 {"Minimum"=60.0, "Maximum"=90.0, "Increment"=1.0} ("Min Max Inc")
      w351 = T16 {"Minimum"=0.0, "Maximum"=75.0, "Increment"=1.0} ("Data Entry Limits")
      w352 = T16 {"Minimum"=60.0, "Maximum"=90.0, "Increment"=1.0} ("Min Max Inc")
      w354 = T16 {"Minimum"=0.0, "Maximum"=75.0, "Increment"=1.0} ("Data Entry Limits")
      n84 = property on="BD 1 Frq 1 (MHz)" class="DigNum (strict)"("Data Range"=w352) -> ()  [unwired: 2 in, 2 out]
      n85 = property on="BD 1 Frq 2 (MHz)" class="DigNum (strict)"("Data Range"=w352) -> ()  [unwired: 2 in, 2 out]
      n86 = property on="BD 1 Frq 3 (MHz)" class="DigNum (strict)"("Data Range"=w352) -> ()  [unwired: 2 in, 2 out]
      n87 = property on="BD 2 Frq 1 (MHz)" class="DigNum (strict)"("Data Range"=w353) -> ()  [unwired: 2 in, 2 out]
      n88 = property on="BD 2 Frq 2 (MHz)" class="DigNum (strict)"("Data Range"=w353) -> ()  [unwired: 2 in, 2 out]
      n89 = property on="BD 2 Frq 3 (MHz)" class="DigNum (strict)"("Data Range"=w353) -> ()  [unwired: 2 in, 2 out]
      n90 = property on="BD 1 Amp 1 (%)" class="DigNum (strict)"("Data Range"=w354) -> ()  [unwired: 2 in, 2 out]
      n91 = property on="BD 1 Amp 2 (%)" class="DigNum (strict)"("Data Range"=w354) -> ()  [unwired: 2 in, 2 out]
      n92 = property on="BD 1 Amp 3 (%)" class="DigNum (strict)"("Data Range"=w354) -> ()  [unwired: 2 in, 2 out]
      n93 = property on="BD 2 Amp 1 (%)" class="DigNum (strict)"("Data Range"=w351) -> ()  [unwired: 2 in, 2 out]
      n94 = property on="BD 2 Amp 2 (%)" class="DigNum (strict)"("Data Range"=w351) -> ()  [unwired: 2 in, 2 out]
      n95 = property on="BD 2 Amp 3 (%)" class="DigNum (strict)"("Data Range"=w351) -> ()  [unwired: 2 in, 2 out]
      "X RF Frequency Limits (MHz)" <- w352
      "X RF Amplitude Limits (%)" <- w354
      "Y RF Amplitude Limits (%)" <- w351
      "Y RF Frequency Limits (MHz)" <- w353
    }
  }
  n96 = To Word Integer(number=w196) -> (16bit integer=w193:i16)
  n97 = To Word Integer(number=w198) -> (16bit integer=w192:i16)
  n98 = Not(x=w181) -> (.not. x?=w177:bool)
  n99 = local read "Cycles/step (MCL)"() -> (w184:u64)
  n100 = Multiply(x=w212, y=1000.0) -> (x*y=w219:dbl)
  n101 = local write "Trap Pos FIFO Timeout"(u16 0 ("Trap Pos FIFO Timeout")) -> ()
  n102 = local read "Scan steps (x)"() -> (w185:u64)
  n103 = local read "Desired Scan Incr (V)"() -> (w187:dbl)
  n104 = Scale By Power Of 2(n=48, x=w219) -> (x*2^n=w220:dbl)
  n105 = local read "Sets to FIFO (Traps)"() -> (w28:T15)
  n106 = Multiply(x=w217, y=w216) -> (x*y=w215:dbl)
  n107 = Divide(x=w220, y=w215) -> (x/y=w214:dbl)
  n108 = local read "Number Interlace Sets"() -> (w116:u8)
  n109 = Split 1D Array(array=w123, index=w116) -> (first subarray=w125:u32[])  [unwired: 1 out]
  n110 = Add Array Elements(numeric array=w125) -> (sum=w124:u32)
  n111 = property on="AI Count (ticks)" class="DigNum (strict)"("Val(Sgnl)"="AI Count (ticks)") -> ()  [unwired: 2 in, 2 out]
  n112 = local read "# Samples/channel"() -> (w204:u32)
  n113 = local read "Number of F/B Scans (AOD)"() -> (w205:u16)
  n114 = To Quad Integer(1:w214) -> (0:w211:i64)
  n115 = local read "Not-Interlacing Set"() -> (w115:enum32{"Set 1", "Set 2", "Set 3"})
  n116 = To Unsigned Byte Integer(number=w115) -> (unsigned 8bit integer=w121:u8)
  n117 = Index Array(array=w123, index=w121) -> (element=w122:u32)
  n118 = local read "Feedback On/Off"() -> (w229:cluster{"Set 1":bool, "Set 2":bool})
  n119 = Divide(x=40000000.0, y="AI Count (ticks)") -> (x/y=w174:dbl)
  n120 = Multiply(x=w187, y=32767.0) -> (x*y=w189:dbl)
  n121 = local read "Scan steps (AOD)"() -> (w210:u64)
  n122 = local read "All FB On/Off"() -> (w230:bool)
  n123 = local read "Cycles/step (AOD)"() -> (w209:u64)
  n124 = local write "AI rate (Hz)"(w174) -> ()
  n125 = Divide(x=w189, y=10.0) -> (x/y=w188:dbl)
  n126 = Multiply(x=w210, y=w209) -> (x*y=w208:u64)
  n127 = Multiply(x=3276.7, y=w226) -> (x*y=w225:cluster{"Set 1":dbl, "Set 2":dbl})
  n128 = To Word Integer(number=w188) -> (16bit integer=w186:i16)
  n129 = Current VI's Path() -> (path=w34:path)
  n130 = Multiply(x=w208, y=u64 2) -> (x*y=w206:u64)
  n131 = Divide(x=w174, y="FPGA Ave.") -> (x/y=w175:dbl)
  n132 = To Word Integer(number=w225) -> (16bit integer=w224:cluster{"Set 1":i16, "Set 2":i16})
  n133 = Multiply(x=w206, y=w205) -> (x*y=w203:u64)
  n134 = Strip Path(path=w34) -> (stripped path=w35:path)  [unwired: 1 out]
  n135 = local write "Ave. Rate (Hz)"(w175) -> ()
  n136 = Divide(x=w203, y=w204) -> (x/y=w202:dbl)
  n137 = Unbundle By Name(w28) -> ("Set 1"=w27:bool, "Set 2"=w26:bool, "Set 3"=w25:bool)
  n138 = Unbundle By Name(w224) -> ("Set 1"=w223:i16, "Set 2"=w222:i16)
  n139 = local read "2D or 1D Scan"() -> (w133:bool)
  n140 = local write "Data points/scans"(w203) -> ()
  n141 = local read "Scan BD"() -> (w221:bool)
  n142 = And(x=w229, y=w230) -> (x .and. y?=w228:cluster{"Set 1":bool, "Set 2":bool})
  n143 = local write "Data points/scan (f/b)"(w206) -> ()
  n144 = Reciprocal(x=w175) -> (1/x=w176:dbl)
  n145 = local read "N Acq Sets (Traps + Fl.)"() -> (w168:i16)
  n146 = local write "N sets should be saved"(w202) -> ()
  n147 = Build Path(base path=w35, name or relative path="Locations.txt") -> (appended path=→"Location path":path)
  n148 = Unbundle By Name(w228) -> ("Set 1"=w232:bool, "Set 2"=w231:bool)
  n149 = local read "Interlace"() -> (w117:bool)
  n150 = Select(t=w124, s=w117, f=w122) -> (s? t:f=w114:u32)
  n151 = local write "Update Count (MCL)"(w114) -> ()
  n152 = local write "Total Counts (ticks)"(w114) -> ()
  n153 = local write "Ave. Period (s)"(w176) -> ()
  n154 = property on="2D or 1D Scan" class="Bool (strict)"("Val(Sgnl)"=w133) -> ()  [unwired: 2 in, 2 out]
  n155 = while "Stage Control" {
    stop <- w356 stop-if-true
    n156 = event shown="[3] \"Goto Bottom (F7)\": Value Change" {
      selector: _ -> [_ _ _ _ _ _ _ _ _]
      dyn-events: _ -> [_ _ _ _ _ _ _ _ _]
      timeout: 10 -> [_ _ _ _ _ _ _ _ _]
      tunnel: [FALSE _ _ _ _ _ _ _ TRUE] -> w356
      event Timeout {
        # "Change the trajectory mode to Jog"
        # "Query and display stage positions"
        # "Setting ESP300 left and right limits for Z-axis, input in mm"
        # "Display Selected Location"
        n157 = event-data() -> ()  [unwired: 1 in, 2 out]
        n158 = local read "Capture Locations"() -> (w381:i32)
        n159 = local read "Location Matrix"() -> (w382:string[][])
        n160 = Concatenate Strings("1TP;\n2TP;\n3TP;\n1MD?;\n2MD?;\n3MD?" ("Substring"), "\r") -> (w365:string)
        n161 = local read "ESP Port"() -> (w368:refnum<visa-resource-name>)
        n162 = Index Array(array=w382, index (row)=w381) -> (element=w380:string[])  [unwired: 1 in]
        n163 = local read "ESP Port"() -> (w377:refnum<visa-resource-name>)
        n164 = VISA Write(VISA resource name=w368, write buffer=w365, error in (no error)="error in") -> (VISA resource name out=w366:refnum<visa-resource-name>, error out=w364:errorcluster)  [unwired: 1 out]
        n165 = Concatenate Strings("3SL" ("Substring"), "ESP ZL-Limit", ";3SR", "ESP ZR-Limit", "\r") -> (w376:string)
        n166 = Array To Cluster(array=w380) -> (cluster=w379:T24)
        n167 = case shown="True" TRUE ("Case Constant\n(See Context Help)") {
          tunnel: w366 -> [_ w420]
          tunnel: w364 -> [w401 w419]
          tunnel: [w401 w403] -> w370
          frame False {
          }
          frame True {
            w413 = u16 10 items=["1.0"=10, "1.5"=15, "2.0"=20] ("Serial Settings:Stop Bits")
            w414 = u16 0 items=["None", "Odd", "Even", "Mark", "Space"] ("Serial Settings:Parity")
            n168 = property class="Instr"(reference=w420, error in=w419, "Baud"=u32 921600 ("Serial Settings:Baud Rate"), "Data Bits"=u16 8 ("Serial Settings:Data Bits"), "Parity"=w414, "Stop Bits"=w413) -> (reference out=w418:refnum<visa-resource-name>, error out=w417:errorcluster, "Bytes at Port"=w402:u32)
            n169 = Wait (ms)(milliseconds to wait=u32 10) -> ()  [unwired: 1 out]
            n170 = VISA Read(VISA resource name=w418, byte count=w402, error in (no error)=w417) -> (VISA resource name out=w426:refnum<visa-resource-name>, read buffer=→"X Pos":string, error out=w427:errorcluster)  [unwired: 1 out]
            n171 = VISA Read(VISA resource name=w426, byte count=w402, error in (no error)=w427) -> (VISA resource name out=w424:refnum<visa-resource-name>, read buffer=→"Y Pos":string, error out=w425:errorcluster)  [unwired: 1 out]
            n172 = VISA Read(VISA resource name=w424, byte count=w402, error in (no error)=w425) -> (VISA resource name out=w412:refnum<visa-resource-name>, read buffer=→"Z Pos Pos":string, error out=w411:errorcluster)  [unwired: 1 out]
            n173 = VISA Read(VISA resource name=w412, byte count=w402, error in (no error)=w411) -> (VISA resource name out=w408:refnum<visa-resource-name>, read buffer=→"X Motion":string, error out=w409:errorcluster)  [unwired: 1 out]
            n174 = VISA Read(VISA resource name=w408, byte count=w402, error in (no error)=w409) -> (VISA resource name out=w407:refnum<visa-resource-name>, read buffer=→"Y Motion":string, error out=w405:errorcluster)  [unwired: 1 out]
            n175 = VISA Read(VISA resource name=w407, byte count=w402, error in (no error)=w405) -> (read buffer=→"Z motion":string, error out=w403:errorcluster)  [unwired: 2 out]
          }
        }
        "error out" <- w370
        n176 = VISA Write(VISA resource name=w377, write buffer=w376) -> ()  [unwired: 1 in, 3 out]
        n177 = local write item#412(w379) -> ()
        n178 = disable-structure shown="Disabled" {
          frame Disabled {
            # "Change Low Jog Velocity"
            # "Change High Jog Velocity"
            n179 = Concatenate Strings("1JH" ("Substring"), "Axis 1", "2JH" ("Substring"), "Axis 2", "3JH" ("Substring"), "Axis 3", "\r") -> (w400:string)
            n180 = local read "ESP Port"() -> (w399:refnum<visa-resource-name>)
            n181 = VISA Write(VISA resource name=w399, write buffer=w400) -> ()  [unwired: 1 in, 3 out]
            n182 = Concatenate Strings("1JW" ("Substring"), "Axis 1", "2JW" ("Substring"), "Axis 2", "3JW" ("Substring"), "Axis 3", "\r") -> (w391:string)
            n183 = local read "ESP Port"() -> (w390:refnum<visa-resource-name>)
            n184 = VISA Write(VISA resource name=w390, write buffer=w391) -> ()  [unwired: 1 in, 3 out]
          }
          frame Enabled {
          }
        }
        n185 = local read "ESP Port"() -> (w358:refnum<visa-resource-name>)
        n186 = Concatenate Strings("1TJ3;\n2TJ3;\n3TJ3" ("Substring"), "\r") -> (w359:string)
        n187 = VISA Write(VISA resource name=w358, write buffer=w359) -> ()  [unwired: 1 in, 3 out]
      }
      event "Goto Top (F6)": Value Change {
        n188 = event-data() -> ()  [unwired: 1 in, 5 out]
        n189 = stacked-sequence {
          frame #0 {
            # "stop motions of all axes before going to avoid reversing of direction"
            n190 = local read "ESP Port"() -> (w432:refnum<visa-resource-name>)
            n191 = Concatenate Strings("ST" ("Substring"), "\r") -> (w429:string)
            n192 = VISA Write(VISA resource name=w432, write buffer=w429) -> ()  [unwired: 1 in, 3 out]
          }
          frame #1 {
            n193 = Wait (ms)(milliseconds to wait=u32 50) -> ()  [unwired: 1 out]
          }
          frame #2 {
            # "Change the trajectory mode to Trapezoidal"
            n194 = local read "ESP Port"() -> (w437:refnum<visa-resource-name>)
            n195 = Concatenate Strings("1TJ1;\n2TJ1;\n3TJ1" ("Substring"), "\r") -> (w434:string)
            n196 = VISA Write(VISA resource name=w437, write buffer=w434) -> ()  [unwired: 1 in, 3 out]
          }
          frame #3 {
            # "Go to Top Dispensor"
            n197 = local read "Location Matrix"() -> (w449:string[][])
            n198 = Index Array(array=w449, index (row)=0) -> (element=w445:string[])  [unwired: 1 in]
            n199 = Decimate 1D Array(w445) -> (w443:string[], w441:string[], w439:string[])
            n200 = local read "ESP Port"() -> (w446:refnum<visa-resource-name>)
            n201 = Concatenate Strings("1PA" ("Substring"), w443, "2PA" ("Substring"), w441, "3PA" ("Substring"), w439, "\r") -> (w447:string)
            n202 = VISA Write(VISA resource name=w446, write buffer=w447) -> ()  [unwired: 1 in, 3 out]
          }
          frame #4 {
            n203 = Wait (ms)(milliseconds to wait=u32 100) -> ()  [unwired: 1 out]
          }
          frame #5 {
            # "Change the trajectory mode to Jog"
            n204 = local read "ESP Port"() -> (w454:refnum<visa-resource-name>)
            n205 = Concatenate Strings("1TJ3;\n2TJ3;\n3TJ3" ("Substring"), "\r") -> (w451:string)
            n206 = VISA Write(VISA resource name=w454, write buffer=w451) -> ()  [unwired: 1 in, 3 out]
          }
        }
      }
      event "Goto Exp (F8)": Value Change {
        n207 = event-data() -> ()  [unwired: 1 in, 5 out]
        n208 = stacked-sequence {
          frame #0 {
            # "stop motions of all axes before going to avoid reversing of direction"
            n209 = local read "ESP Port"() -> (w458:refnum<visa-resource-name>)
            n210 = Concatenate Strings("ST" ("Substring"), "\r") -> (w455:string)
            n211 = VISA Write(VISA resource name=w458, write buffer=w455) -> ()  [unwired: 1 in, 3 out]
          }
          frame #1 {
            n212 = Wait (ms)(milliseconds to wait=u32 50) -> ()  [unwired: 1 out]
          }
          frame #2 {
            # "Change the trajectory mode to Trapezoidal"
            n213 = local read "ESP Port"() -> (w463:refnum<visa-resource-name>)
            n214 = Concatenate Strings("1TJ1;\n2TJ1;\n3TJ1" ("Substring"), "\r") -> (w460:string)
            n215 = VISA Write(VISA resource name=w463, write buffer=w460) -> ()  [unwired: 1 in, 3 out]
          }
          frame #3 {
            # "Go to Experimental"
            n216 = local read "Location Matrix"() -> (w475:string[][])
            n217 = Index Array(array=w475, index (row)=2) -> (element=w471:string[])  [unwired: 1 in]
            n218 = Decimate 1D Array(w471) -> (w469:string[], w467:string[], w465:string[])
            n219 = Concatenate Strings("1PA" ("Substring"), w469, "2PA" ("Substring"), w467, "3PA" ("Substring"), w465, "\r") -> (w473:string)
            n220 = local read "ESP Port"() -> (w472:refnum<visa-resource-name>)
            n221 = VISA Write(VISA resource name=w472, write buffer=w473) -> ()  [unwired: 1 in, 3 out]
          }
          frame #4 {
            n222 = Wait (ms)(milliseconds to wait=u32 200) -> ()  [unwired: 1 out]
          }
          frame #5 {
            # "Change the trajectory mode to Jog"
            n223 = local read "ESP Port"() -> (w477:refnum<visa-resource-name>)
            n224 = Concatenate Strings("1TJ3;\n2TJ3;\n3TJ3" ("Substring"), "\r") -> (w480:string)
            n225 = VISA Write(VISA resource name=w477, write buffer=w480) -> ()  [unwired: 1 in, 3 out]
          }
        }
      }
      event "Goto Bottom (F7)": Value Change {
        n226 = event-data() -> ()  [unwired: 1 in, 5 out]
        n227 = stacked-sequence {
          frame #0 {
            # "stop motions of all axes before going to avoid reversing of direction"
            n228 = local read "ESP Port"() -> (w484:refnum<visa-resource-name>)
            n229 = Concatenate Strings("ST" ("Substring"), "\r") -> (w481:string)
            n230 = VISA Write(VISA resource name=w484, write buffer=w481) -> ()  [unwired: 1 in, 3 out]
          }
          frame #1 {
            n231 = Wait (ms)(milliseconds to wait=u32 50) -> ()  [unwired: 1 out]
          }
          frame #2 {
            # "Change the trajectory mode to Trapezoidal"
            n232 = local read "ESP Port"() -> (w489:refnum<visa-resource-name>)
            n233 = Concatenate Strings("1TJ1;\n2TJ1;\n3TJ1" ("Substring"), "\r") -> (w486:string)
            n234 = VISA Write(VISA resource name=w489, write buffer=w486) -> ()  [unwired: 1 in, 3 out]
          }
          frame #3 {
            # "Go to Bottom Dispensor"
            n235 = local read "Location Matrix"() -> (w501:string[][])
            n236 = Index Array(array=w501, index (row)=1) -> (element=w497:string[])  [unwired: 1 in]
            n237 = Decimate 1D Array(w497) -> (w495:string[], w493:string[], w491:string[])
            n238 = Concatenate Strings("1PA" ("Substring"), w495, "2PA" ("Substring"), w493, "3PA" ("Substring"), w491, "\r") -> (w499:string)
            n239 = local read "ESP Port"() -> (w498:refnum<visa-resource-name>)
            n240 = VISA Write(VISA resource name=w498, write buffer=w499) -> ()  [unwired: 1 in, 3 out]
          }
          frame #4 {
            n241 = Wait (ms)(milliseconds to wait=u32 200) -> ()  [unwired: 1 out]
          }
          frame #5 {
            # "Change the trajectory mode to Jog"
            n242 = local read "ESP Port"() -> (w503:refnum<visa-resource-name>)
            n243 = Concatenate Strings("1TJ3;\n2TJ3;\n3TJ3" ("Substring"), "\r") -> (w506:string)
            n244 = VISA Write(VISA resource name=w503, write buffer=w506) -> ()  [unwired: 1 in, 3 out]
          }
        }
      }
      event "Capture": Value Change {
        n245 = event-data() -> ()  [unwired: 1 in, 5 out]
        n246 = local read "Capture Locations"() -> (w507:i32)
        n247 = local read "Z Pos Pos"() -> (w508:string)
        n248 = local read "X Pos"() -> (w510:string)
        n249 = local read "Y Pos"() -> (w509:string)
        n250 = case shown="3" w507 {
          selector: w507 -> [w514 w521 w528 w535]
          tunnel: w510 -> [w517 w524 w531 w538]
          tunnel: w509 -> [w516 w523 w530 w537]
          tunnel: w508 -> [w515 w522 w529 w536]
          frame 0, Default {
            # "Capture Top Dispensor Location"
            n251 = local read "Location Matrix"() -> (w513:string[][])
            n252 = Build Array(w517, w516, w515) -> (w512:string[])
            n253 = Replace Array Subset(array=w513, new element=w512, index (row)=w514) -> (w511:string[][])  [unwired: 1 in]
            n254 = local write "Location Matrix"(w511) -> ()
          }
          frame 1 {
            # "Capture Bottom Dispensor Location"
            n255 = local read "Location Matrix"() -> (w520:string[][])
            n256 = Build Array(w524, w523, w522) -> (w519:string[])
            n257 = Replace Array Subset(array=w520, new element=w519, index (row)=w521) -> (w518:string[][])  [unwired: 1 in]
            n258 = local write "Location Matrix"(w518) -> ()
          }
          frame 2 {
            # "Capture Experimental Region Location"
            n259 = local read "Location Matrix"() -> (w527:string[][])
            n260 = Build Array(w531, w530, w529) -> (w526:string[])
            n261 = Replace Array Subset(array=w527, new element=w526, index (row)=w528) -> (w525:string[][])  [unwired: 1 in]
            n262 = local write "Location Matrix"(w525) -> ()
          }
          frame 3 {
            # "Capture Other Location"
            n263 = local read "Location Matrix"() -> (w534:string[][])
            n264 = Build Array(w538, w537, w536) -> (w533:string[])
            n265 = Replace Array Subset(array=w534, new element=w533, index (row)=w535) -> (w532:string[][])  [unwired: 1 in]
            n266 = local write "Location Matrix"(w532) -> ()
          }
        }
      }
      event "Save": Value Change {
        # "reshape Location Matrix to 1-D array to write"
        n267 = event-data() -> ()  [unwired: 1 in, 5 out]
        n268 = local read "Location Matrix"() -> (w542:string[][])
        n269 = local read "Location path"() -> (w539:path)
        n270 = Reshape Array(w542, 12) -> (w540:string[])
        n271 = Write to Text File(file (use dialog)=w539, text=w540) -> ()  [unwired: 2 in, 3 out]
      }
      event "VISA Clear": Value Change {
        n272 = event-data() -> ()  [unwired: 1 in, 5 out]
        n273 = local read "ESP Port"() -> (w543:refnum<visa-resource-name>)
        n274 = VISA Clear(VISA resource name=w543) -> ()  [unwired: 1 in, 2 out]
      }
      event "Activate Joystick": Value Change {
        # "Change the trajectory mode to Jog"
        n275 = event-data() -> ()  [unwired: 1 in, 5 out]
        n276 = disable-structure shown="Disabled" {
          frame Disabled {
            n277 = case shown="True" "Activate Joystick" {
              frame False {
              }
              frame True {
                # "Change the trajectory mode to Jog"
                n278 = local read "ESP Port"() -> (w552:refnum<visa-resource-name>)
                n279 = Concatenate Strings("1TJ3;\n2TJ3;\n3TJ3" ("Substring"), "\r") -> (w549:string)
                n280 = VISA Write(VISA resource name=w552, write buffer=w549) -> ()  [unwired: 1 in, 3 out]
              }
            }
          }
          frame Enabled {
          }
        }
        n281 = local read "ESP Port"() -> (w544:refnum<visa-resource-name>)
        n282 = Concatenate Strings("1TJ3;\n2TJ3;\n3TJ3" ("Substring"), "\r") -> (w547:string)
        n283 = VISA Write(VISA resource name=w544, write buffer=w547) -> ()  [unwired: 1 in, 3 out]
      }
      event "Stop All": Mouse Down {
        n284 = event-data() -> ()  [unwired: 1 in, 5 out]
      }
    }
  }
  n285 = xnode "Read/Write Control"("FPGA VI Reference In"=w130, "error in"=w148, "ai count"="AI Count (ticks)", "Interlace ON/OFF"=w117, "Number Interlace Cycles"=w116, "Set 1"=w27, "Set 2"=w26, "Set 3"=w25, "FB On/Off Set 1"=w232, "FB On/Off Set 2"=w231, "Interlace Off Parameters"=w115, "FB Setpoint Set 1"=w223, "FB Setpoint Set 2"=w222, "FB Gains"="PID gains", "FB output range"=cluster{"output high":i16, "output low":i16} {"output high"=3000, "output low"=0} ("FB output range 1"), "Cycles per step"=w209, "Scan BD"=w221, "Number of scans"=w205, "Scan steps"=w210, "Scan freq.  increment"=w211, "AO1 (Y)"=w193, "AO2 (X)"=w192, "Scan freq.  increment (MCL)"=w186, "Scan steps (MCL)"=w185, "Cycles per step (MCL)"=w184, "Number of scans (MCL)"=w183, "MCL count"=w114, "Cont. Scan (MCL)"=w182, "MCL Scan Axis"=w177, "1D or 2D Scan?"=w133, "N of AI1 Int Acq Sets"=w168, "BD 1 Delay (ticks)"="Freq switch delay", "Amp switch delay"="Amp switch delay", "Swap F1 and F2"="Swap F1 and F2", "APD Acq Rate Count"=w138, "APD to FIFO"=FALSE, "APD Gate Operating Mode"="APD Gate", "APD Gate ON Count"="APD Gate ON Count", "APD Gate OFF Count"="APD Gate OFF Count", "Invert APD Gate"="Invert APD Gate", "DIO count 1 (ticks)"="DIO count 1 (ticks)", "DIO count 2 (ticks)"="DIO count 2 (ticks)", "DIO count 3 (ticks)"="DIO count 3 (ticks)", "APD 1 AO scale factor"="APD 1 AO Mult.", "APD 2 AO scale factor"="APD 2 AO Mult.", "Diff FB Measurement?"=w32, "Dynamic Force FB (Ronen)"=w31, "Negate Diff?"=w30, "Next trap write delay (ticks)"="Next trap write delay (ticks)", "Phase offset method"="Phase offset method", "Phase Trap 1"="Phase increment trap 1", "RF phase reset before cycles"="RF phase reset before cycles", "Phase Trap 2"="Phase increment trap 2") -> ("FPGA VI Reference Out"=w109:T20, "error out"=w111:errorcluster)  [unwired: 1 in]
  n286 = local read "Green Laser ON/Interlacing"() -> (w112:bool)
  n287 = local read "Green laser mode"() -> (w113:enum32{"Laser ON", "Laser OFF", "Interlace"})
  n288 = local read "GI Frequency, OFF count"() -> (w105:u32)
  n289 = local read "GI Frequency, ON count"() -> (w104:u32)
  n290 = Multiply(x="Current When FB OFF (%)", y=655.35) -> (x*y=w96:dbl)
  n291 = local read "Green FB Count"() -> (w103:u32)
  n292 = Multiply(x="Green FB Setpoint (mV)", y=3.2767) -> (x*y=w93:dbl)
  n293 = To Unsigned Word Integer(number=w96) -> (unsigned 16bit integer=w94:u16)
  n294 = local read "Invert GI"() -> (w107:bool)
  n295 = To Word Integer(number=w93) -> (16bit integer=w91:i16)
  n296 = case shown="True" w112 {
    tunnel: w113 -> [_ w555]
    tunnel: [enum32{"Laser ON", "Laser OFF", "Interlace"}."Laser OFF" ("Green laser mode") w555] -> w106
    frame False {
    }
    frame True {
    }
  }
  n297 = local read "Trap Pos. AI1 X Pre-scale"() -> (w63:u16)
  n298 = local read "Trap Pos FB Monitor\nT1 or T2"() -> (w70:bool)
  n299 = local read "Trap Pos FB Int Count"() -> (w60:u16)
  n300 = local read "Trap Pos FB Negate Action"() -> (w69:bool)
  n301 = local read "Trap Pos. FB Offset Factor"() -> (w68:i64)
  n302 = local read "Trap Pos. FB Mult Factor"() -> (w67:i64)
  n303 = local read "Trap Pos. FB Gains"() -> (w65:T11)
  n304 = local read "Trap Pos. FB Range"() -> (w66:T12)
  n305 = xnode "Read/Write Control"("FPGA VI Reference In"=w109, "error in"=w111, "Green interlace ON count 2"=w104, "Green interlace OFF count 2"=w105, "Invert GI 2"=w107, "Operating Mode 2"=w106, "Green FB Gains"="Green FB Gains", "Green FB Setpoint"=w91, "Green FB On/Off"="Green FB On/Off", "Current Out"=w94, "Green int current ON count adj"="Green int current ON count adj", "Green FB Count"=w103, "Operating Mode"=w106, "Green interlace OFF count"=w105, "Green interlace ON count"=w104, "Invert GI"=w107, "Trap Pos FB Monitor T1 or T2"=w70, "Trap Pos FB Negate Action"=w69, "Trap Pos. FB Offset Factor"=w68, "Trap Pos. FB Mult Factor"=w67, "Trap pos. FB Range"=w66, "Trap Pos. FB Gains"=w65, "Force feedback"=FALSE, "AI1 X Scale"=w63, "Trap Pos to FIFO"=TRUE, "Trap Pos FB Int Count"=w60) -> ("FPGA VI Reference Out"=w108:T20, "error out"=w110:errorcluster)
  n306 = xnode "Invoke Method"("FPGA VI Reference In"=w108, "error in"=w110, "Requested Depth"="Trap AI FIFO Depth") -> ("FPGA VI Reference Out"=w73:T20, "error out"=w72:errorcluster)  [unwired: 1 out]
  n307 = xnode "Invoke Method"("FPGA VI Reference In"=w73, "error in"=w72, "Requested Depth"="Trap Position FIFO Depth") -> ("FPGA VI Reference Out"=w15:T20, "error out"=w13:errorcluster)  [unwired: 1 out]
  n308 = xnode "Invoke Method"("FPGA VI Reference In"=w15, "error in"=w13, "Requested Depth"="APD FIFO Depth (requires restart)") -> ("FPGA VI Reference Out"=w14:T20, "error out"=w12:errorcluster)  [unwired: 1 out]
  n309 = xnode "Invoke Method"("FPGA VI Reference In"=w14, "error in"=w12) -> ("FPGA VI Reference Out"=w47:T20, "error out"=w46:errorcluster)  [unwired: 1 in]
  n310 = flat-sequence "Initial FPGA Loop Relative Phase Adjustment" {
    tunnel: w46 -> [w557]
    tunnel: w47 -> [w558]
    tunnel: [w558] -> w51
    tunnel: [w557] -> w50
    tunnel: [w570] -> w154
    tunnel: [w567] -> w152
    tunnel: w51 -> [w569]
    tunnel: w50 -> [w568]
    tunnel: w154 -> [w572]
    tunnel: [w573] -> w153
    tunnel: w152 -> [w573]
    tunnel: [w572] -> w151
    tunnel: w153 -> [w576]
    tunnel: w151 -> [w575]
    tunnel: [w578] -> w150
    tunnel: [w577] -> w149
    tunnel: [w580] -> w45
    tunnel: [w581] -> w48
    tunnel: w150 -> [w581]
    tunnel: w149 -> [w580]
    frame #0 {
      n311 = Wait (ms)(milliseconds to wait=u32 1000) -> ()  [unwired: 1 out]
    }
    frame #1 {
      n312 = xnode "Read/Write Control"("FPGA VI Reference In"=w569, "error in"=w568, "Phase count adjustment"="Initial Phase Adjustment (AI1)", "Phase count adjustment (GI)"="Initial Phase Adjustment (GI)", "Phase count adjustment (MCL)"="Initial Phase Adj. (MCL)", "Phase Count Adjustment (APD Acq)"="Initial Phase Adjustment (APD Acq)", "Phase count adjustment (APD 1 Gate)"="Initial Phase Adjustment (APD 1 Gate)", "Phase count adjustment (APD 2 Gate)"="Initial Phase Adjustment (APD 2 Gate)", "Phase count adjustment (Green FB)"="Initial Phase Adjustment (Green FB)", "Phase count adjustment (GI) 2"="Initial Phase Adjustment (GI) 2") -> ("FPGA VI Reference Out"=w567:T20, "error out"=w570:errorcluster)
    }
    frame #2 {
      n313 = Wait (ms)(milliseconds to wait=u32 1000) -> ()  [unwired: 1 out]
    }
    frame #3 {
      w574 = TRUE
      n314 = xnode "Read/Write Control"("FPGA VI Reference In"=w576, "error in"=w575, "+ phase"=w574, "+ phase (GI)"=w574, "+ phase (MCL)"=w574, "+ phase (APD Acq)"=w574, "+ phase (APD 1 Gate)"=w574, "+ phase (APD 2 Gate)"=w574, "+ phase (Green FB)"=w574, "+ phase (GI) 2"=w574) -> ("FPGA VI Reference Out"=w577:T20, "error out"=w578:errorcluster)
    }
    frame #4 {
      n315 = Wait (ms)(milliseconds to wait=u32 1000) -> ()  [unwired: 1 out]
    }
  }
  n316 = node-c288() -> (w83:T21)  [unwired: 4 in]
  n317 = timed-loop "Run Scripts, including: stage motion" {
    timing: w83 -> [_]
    timing-out: [_] -> w82
    tunnel: w49 -> [_]
    stop <- w583 stop-if-true
    n318 = node-c288() -> ()  [unwired: 1 in, 1 out]
    n319 = event shown="[4] \"Step Size (nm)\": Value Change" {
      selector: _ -> [_ _ _ _ _ _ _]
      dyn-events: _ -> [_ _ _ _ _ _ _]
      timeout: 50 -> [_ _ _ _ _ _ _]
      tunnel: ["Move Cap. 1 (DNA Top)" _ "Cal/Data Acq. Spot" "Take Stepping Data" _ "Take Detection Laser\nImage" _] -> _
      tunnel: [_ _ _ _ _ _ w760] -> w583
      event "Move Cap. 1 (DNA Top)": Value Change {
        n320 = event-data() -> ()  [unwired: 1 in, 5 out]
        n321 = local write "Move Cap. 1 (DNA Top)"(FALSE ("Move Cap. 1 (DNA Right)")) -> ()
        n322 = flat-sequence {
          tunnel: "Cap 1 Samp Flow ON" -> [w589]
          frame #0 {
            n323 = local write "Stage Moving"(FALSE ("Stage Moving")) -> ()
            n324 = case "stop flow" shown="True" w589 {
              frame False {
              }
              frame True {
                n325 = call "hamilton_controller.vi"("Open?"=FALSE, "valve"=enum16{"A", "B", "C", "D", "ALL"}."C", "action"=T25."MOVE VALVE") -> ()  [unwired: 8 in, 1 out]
              }
            }
            n326 = case shown="True" TRUE {
              tunnel: "Cap 1 T ON" -> [w598 w599]
              frame False {
                n327 = property on="Trap 1 (ON/OFF)" class="Bool (strict)"("Val(Sgnl)"=w598) -> ()  [unwired: 2 in, 2 out]
              }
              frame True {
                n328 = property on="Trap 2 (ON/OFF)" class="Bool (strict)"("Val(Sgnl)"=w599) -> ()  [unwired: 2 in, 2 out]
              }
            }
            n329 = call <vilib>:"Beep.vi"() -> ()  [unwired: 3 in, 9 out]
            n330 = case shown="True" "Cap 1 Flow ON" {
              frame False {
              }
              frame True {
                n331 = property on="Main:" class="Bool (strict)"("Val(Sgnl)"=TRUE ("Value (Signaling)")) -> ()  [unwired: 2 in, 2 out]
              }
            }
          }
        }
      }
      event Timeout {
        n332 = event-data() -> ()  [unwired: 1 in, 2 out]
      }
      event "Cal/Data Acq. Spot": Value Change {
        # "wait for calibration file\nto be written"
        # "signal save cal true\nthis tells the data \nacquisition loop to\nstart sending the data\nto a calibration file"
        # "separate traps to\nthe desired trap delta"
        # "move stage to data acquisition spot"
        # "CHANGE FISH FOR TETHER BACK\nTO TRUE VALUE HERE."
        n333 = event-data() -> ()  [unwired: 1 in, 5 out]
        n334 = flat-sequence {
          tunnel: ["Cal @ (MHz)"] -> w600
          tunnel: w600 -> [w612]
          tunnel: w600 -> [w633]
          frame #0 {
            n335 = property on="Trap Delta (MHz)" class="DigNum (strict)"("Val(Sgnl)"="Cal @ (MHz)") -> ()  [unwired: 2 in, 2 out]
            n336 = call <vilib>:"Beep.vi"() -> ()  [unwired: 3 in, 9 out]
          }
          frame #1 {
            n337 = local read "Scale intensities"() -> (w604:bool)
            n338 = case shown="True" w604 {
              frame False {
              }
              frame True {
                n339 = property on="Scale intensities" class="Bool (strict)"("Val(Sgnl)"=FALSE ("Value (Signaling)")) -> ()  [unwired: 2 in, 2 out]
              }
            }
          }
          frame #2 {
            n340 = Wait (ms)(milliseconds to wait=u32 500) -> ()  [unwired: 1 out]
          }
          frame #3 {
            n341 = property on="Save Calibration" class="Bool (strict)"("Val(Sgnl)"=TRUE ("Value (Signaling)")) -> ()  [unwired: 2 in, 2 out]
          }
          frame #4 {
            n342 = Wait (ms)(milliseconds to wait=u32 4000) -> ()  [unwired: 1 out]
          }
          frame #5 {
            n343 = while {
              stop <- w609 stop-if-true
              n344 = local read "Saving..."() -> (w610:bool)
              n345 = Wait (ms)(milliseconds to wait=u32 100) -> ()  [unwired: 1 out]
              n346 = Not(x=w610) -> (.not. x?=w609:bool)
            }
          }
          frame #6 {
            n347 = case shown="True" "W/ Offset 1" {
              tunnel: w612 -> [_ w614]
              frame False {
              }
              frame True {
                n348 = stacked-sequence {
                  tunnel: w614 -> [_ _ _ _ _ _ _ w631]
                  frame #0 {
                    n349 = Replace Array Subset(array=u32[] [0] ("Index Values"), new element="Offset 1 Set", index=0) -> (w615:u32[])
                    n350 = property on="Saved AOD Raster Scan Parameter Sets" class="Arr (strict)"("Index Values"=w615) -> ()  [unwired: 2 in, 2 out]
                    n351 = property on="Trap Delta (MHz)" class="DigNum (strict)"("Val(Sgnl)"="Offset 1 Start (MHz)") -> ()  [unwired: 2 in, 2 out]
                  }
                  frame #1 {
                    n352 = Wait (ms)(milliseconds to wait=u32 200) -> ()  [unwired: 1 out]
                  }
                  frame #2 {
                    n353 = property on="Load parameters" class="Bool (strict)"("Val(Sgnl)"=TRUE ("Value (Signaling)")) -> ()  [unwired: 2 in, 2 out]
                  }
                  frame #3 {
                    n354 = Wait (ms)(milliseconds to wait=u32 200) -> ()  [unwired: 1 out]
                  }
                  frame #4 {
                    n355 = property on="Trap Raster Scan" class="Bool (strict)"("Val(Sgnl)"=TRUE ("Value (Signaling)")) -> ()  [unwired: 2 in, 2 out]
                  }
                  frame #5 {
                    n356 = Wait (ms)(milliseconds to wait=u32 2000) -> ()  [unwired: 1 out]
                  }
                  frame #6 {
                    n357 = while {
                      stop <- w628 stop-if-true
                      n358 = local read "Raster Scanning..."() -> (w630:bool)
                      n359 = local read "Saving..."() -> (w626:bool)
                      n360 = Wait (ms)(milliseconds to wait=u32 100) -> ()  [unwired: 1 out]
                      n361 = Not(x=w626) -> (.not. x?=w625:bool)
                      n362 = Not(x=w630) -> (.not. x?=w627:bool)
                      n363 = And(x=w627, y=w625) -> (x .and. y?=w628:bool)
                    }
                  }
                  frame #7 {
                    n364 = property on="Trap Delta (MHz)" class="DigNum (strict)"("Val(Sgnl)"=w631) -> ()  [unwired: 2 in, 2 out]
                  }
                }
              }
            }
          }
          frame #7 {
            n365 = local read "Save ave N"() -> (w632:i32)
            n366 = case shown="True" "W/ Offset 2" {
              tunnel: w633 -> [_ w639]
              tunnel: w632 -> [_ w638]
              frame False {
                n367 = Multiply(x="Cal read wait (s)", y=u32 1000 ("milliseconds to wait")) -> (x*y=w636:u32)
                n368 = Wait (ms)(milliseconds to wait=w636) -> ()  [unwired: 1 out]
              }
              frame True {
                n369 = stacked-sequence {
                  tunnel: w639 -> [_ _ _ _ _ _ _ _ _ w660 _ _]
                  tunnel: w638 -> [_ _ _ _ _ _ _ _ _ w658 _ _]
                  frame #0 {
                    n370 = property on="Save ave N" class="DigNum (strict)"("Val(Sgnl)"=1.0 ("Value (Signaling)")) -> ()  [unwired: 2 in, 2 out]
                  }
                  frame #1 {
                    n371 = Wait (ms)(milliseconds to wait=u32 500) -> ()  [unwired: 1 out]
                  }
                  frame #2 {
                    n372 = property on="Trap Delta (MHz)" class="DigNum (strict)"("Val(Sgnl)"="Offset 2 Start (MHz)") -> ()  [unwired: 2 in, 2 out]
                    n373 = Replace Array Subset(array=u32[] [0] ("Index Values"), new element="Offset 2 Set", index=0) -> (w644:u32[])
                    n374 = property on="Saved AOD Raster Scan Parameter Sets" class="Arr (strict)"("Index Values"=w644) -> ()  [unwired: 2 in, 2 out]
                  }
                  frame #3 {
                    n375 = Wait (ms)(milliseconds to wait=u32 500) -> ()  [unwired: 1 out]
                  }
                  frame #4 {
                    n376 = property on="Load parameters" class="Bool (strict)"("Val(Sgnl)"=TRUE ("Value (Signaling)")) -> ()  [unwired: 2 in, 2 out]
                  }
                  frame #5 {
                    n377 = Wait (ms)(milliseconds to wait=u32 500) -> ()  [unwired: 1 out]
                  }
                  frame #6 {
                    n378 = property on="Trap Raster Scan" class="Bool (strict)"("Val(Sgnl)"=TRUE ("Value (Signaling)")) -> ()  [unwired: 2 in, 2 out]
                  }
                  frame #7 {
                    n379 = Wait (ms)(milliseconds to wait=u32 2000) -> ()  [unwired: 1 out]
                  }
                  frame #8 {
                    n380 = while {
                      stop <- w653 stop-if-true
                      n381 = local read "Raster Scanning..."() -> (w656:bool)
                      n382 = local read "Saving..."() -> (w654:bool)
                      n383 = Wait (ms)(milliseconds to wait=u32 100) -> ()  [unwired: 1 out]
                      n384 = Not(x=w654) -> (.not. x?=w652:bool)
                      n385 = Not(x=w656) -> (.not. x?=w655:bool)
                      n386 = And(x=w655, y=w652) -> (x .and. y?=w653:bool)
                    }
                  }
                  frame #9 {
                    n387 = property on="Trap Delta (MHz)" class="DigNum (strict)"("Val(Sgnl)"=w660) -> ()  [unwired: 2 in, 2 out]
                    n388 = property on="Saved AOD Raster Scan Parameter Sets" class="Arr (strict)"("Index Values"=u32[] [0]) -> ()  [unwired: 2 in, 2 out]
                    n389 = property on="Save ave N" class="DigNum (strict)"("Val(Sgnl)"=w658) -> ()  [unwired: 2 in, 2 out]
                  }
                  frame #10 {
                    n390 = Wait (ms)(milliseconds to wait=u32 500) -> ()  [unwired: 1 out]
                  }
                  frame #11 {
                    n391 = property on="Load parameters" class="Bool (strict)"("Val(Sgnl)"=TRUE ("Value (Signaling)")) -> ()  [unwired: 2 in, 2 out]
                  }
                }
              }
            }
          }
          frame #8 {
            n392 = property on="Read Cal" class="Bool (strict)"("Val(Sgnl)"=TRUE ("Value (Signaling)")) -> ()  [unwired: 2 in, 2 out]
          }
          frame #9 {
            n393 = Wait (ms)(milliseconds to wait=u32 500) -> ()  [unwired: 1 out]
          }
          frame #10 {
            n394 = property on="Fish for Tether" class="Bool (strict)"("Val(Sgnl)"=FALSE ("Value (Signaling)")) -> ()  [unwired: 2 in, 2 out]
          }
        }
        n395 = local write "Cal/Data Acq. Spot"(FALSE ("Cal/Data Acq. Spot")) -> ()
      }
      event "Take Stepping Data": Value Change {
        n396 = event-data() -> ()  [unwired: 1 in, 5 out]
        n397 = local read "Save ave N"() -> (w674:i32)
        n398 = flat-sequence {
          tunnel: w674 -> [w676]
          tunnel: [w676] -> w669
          tunnel: [w678] -> w670
          tunnel: w669 -> [w678]
          tunnel: [w680] -> w671
          tunnel: w670 -> [w680]
          tunnel: [w683] -> w672
          tunnel: w671 -> [w683]
          tunnel: [w685] -> w673
          tunnel: w672 -> [w685]
          tunnel: [w687] -> w667
          tunnel: w673 -> [w687]
          tunnel: w667 -> [w690]
          tunnel: [w690] -> w666
          tunnel: w666 -> [w691]
          tunnel: [w691] -> w668
          tunnel: w668 -> [w697]
          frame #0 {
            n399 = property on="Save ave N" class="DigNum (strict)"("Val(Sgnl)"="Save ave factor") -> ()  [unwired: 2 in, 2 out]
          }
          frame #1 {
            n400 = Wait (ms)(milliseconds to wait=u32 100) -> ()  [unwired: 1 out]
          }
          frame #2 {
            n401 = local read "Offset 2 Start (MHz)"() -> (w682:dbl)
            n402 = property on="Saved AOD Raster Scan Parameter Sets" class="Arr (strict)"("Index Values"=u32[] [2]) -> ()  [unwired: 2 in, 2 out]
            n403 = property on="Trap Delta (MHz)" class="DigNum (strict)"("Val(Sgnl)"=w682) -> ()  [unwired: 2 in, 2 out]
          }
          frame #3 {
            n404 = property on="Load parameters" class="Bool (strict)"("Val(Sgnl)"=TRUE ("Value (Signaling)")) -> ()  [unwired: 2 in, 2 out]
          }
          frame #4 {
            n405 = Wait (ms)(milliseconds to wait=u32 100) -> ()  [unwired: 1 out]
          }
          frame #5 {
            n406 = property on="Trap Raster Scan" class="Bool (strict)"("Val(Sgnl)"=TRUE ("Value (Signaling)")) -> ()  [unwired: 2 in, 2 out]
          }
          frame #6 {
            n407 = Wait (ms)(milliseconds to wait=u32 1000) -> ()  [unwired: 1 out]
          }
          frame #7 {
            n408 = while {
              stop <- w694 stop-if-true
              n409 = local read "Raster Scanning..."() -> (w696:bool)
              n410 = local read "Saving..."() -> (w695:bool)
              n411 = Not(x=w695) -> (.not. x?=w692:bool)
              n412 = Not(x=w696) -> (.not. x?=w693:bool)
              n413 = And(x=w693, y=w692) -> (x .and. y?=w694:bool)
            }
          }
          frame #8 {
            n414 = property on="Save ave N" class="DigNum (strict)"("Val(Sgnl)"=w697) -> ()  [unwired: 2 in, 2 out]
          }
        }
      }
      event "Step Size (nm)": Value Change {
        n415 = event-data() -> ()  [unwired: 1 in, 5 out]
        n416 = flat-sequence {
          frame #0 {
            n417 = property on="Saved AOD Raster Scan Parameter Sets" class="Arr (strict)"("Index Values"=u32[] [1]) -> ()  [unwired: 2 in, 2 out]
          }
          frame #1 {
            n418 = Multiply(x="N Steps", y="Step Size (nm)") -> (x*y=w699:dbl)
            n419 = property on="Scan Speed AOD (nm/s) 2" class="DigNum (strict)"("Value"="Step Size (nm)") -> ()  [unwired: 2 in, 2 out]
            n420 = property on="Step Size AOD (nm) 2" class="DigNum (strict)"("Value"="Step Size (nm)") -> ()  [unwired: 2 in, 2 out]
            n421 = property on="Scan Range AOD (nm) 2" class="DigNum (strict)"("Value"=w699) -> ()  [unwired: 2 in, 2 out]
          }
        }
      }
      event "Take Detection Laser\nImage": Value Change {
        n422 = event-data() -> ()  [unwired: 1 in, 5 out]
        n423 = flat-sequence {
          tunnel: [w727] -> w717
          tunnel: [w726] -> w710
          tunnel: [w725] -> w702
          tunnel: [w730] -> w718
          tunnel: w717 -> [w730]
          tunnel: [w729] -> w711
          tunnel: w710 -> [w729]
          tunnel: [w728] -> w703
          tunnel: w702 -> [w728]
          tunnel: [w734] -> w719
          tunnel: w718 -> [w734]
          tunnel: [w733] -> w712
          tunnel: w711 -> [w733]
          tunnel: [w732] -> w704
          tunnel: w703 -> [w732]
          tunnel: [w740] -> w720
          tunnel: w719 -> [w740]
          tunnel: [w739] -> w713
          tunnel: w712 -> [w739]
          tunnel: [w738] -> w705
          tunnel: w704 -> [w738]
          tunnel: [w744] -> w721
          tunnel: w720 -> [w744]
          tunnel: [w743] -> w714
          tunnel: w713 -> [w743]
          tunnel: [w742] -> w706
          tunnel: w705 -> [w742]
          tunnel: [w748] -> w722
          tunnel: w721 -> [w748]
          tunnel: [w747] -> w715
          tunnel: w714 -> [w747]
          tunnel: [w746] -> w707
          tunnel: w706 -> [w746]
          tunnel: [w752] -> w723
          tunnel: w722 -> [w752]
          tunnel: [w751] -> w716
          tunnel: w715 -> [w751]
          tunnel: [w750] -> w708
          tunnel: w707 -> [w750]
          tunnel: w723 -> [w758]
          tunnel: w716 -> [w757]
          tunnel: [w755] -> w709
          tunnel: w708 -> [w755]
          tunnel: w709 -> [w759]
          frame #0 {
            n424 = local read "Green Laser ON/Interlacing"() -> (w727:bool)
            n425 = local read "Green laser mode"() -> (w726:enum32{"Laser ON", "Laser OFF", "Interlace"})
            n426 = local read "Green FB On/Off"() -> (w725:bool)
          }
          frame #1 {
            n427 = property on="Green FB On/Off" class="Bool (strict)"("Val(Sgnl)"=FALSE ("Value (Signaling)")) -> ()  [unwired: 2 in, 2 out]
          }
          frame #2 {
            n428 = property on="Green Laser ON/Interlacing" class="Bool (strict)"("Val(Sgnl)"=TRUE ("Value (Signaling)")) -> ()  [unwired: 2 in, 2 out]
            n429 = property on="Flip Green Filter" class="Bool (strict)"("Val(Sgnl)"=TRUE ("Value (Signaling)")) -> ()  [unwired: 2 in, 2 out]
            n430 = property on="Green laser mode" class="RadioBtnsControl (strict)"("Val(Sgnl)"=enum32{"Laser ON", "Laser OFF", "Interlace"}."Laser ON" ("Value (Signaling)")) -> ()  [unwired: 2 in, 2 out]
          }
          frame #3 {
            n431 = Wait (ms)(milliseconds to wait=u32 500) -> ()  [unwired: 1 out]
          }
          frame #4 {
            n432 = property on="Confocal Image" class="Bool (strict)"("Val(Sgnl)"=TRUE ("Value (Signaling)")) -> ()  [unwired: 2 in, 2 out]
          }
          frame #5 {
            n433 = Wait (ms)(milliseconds to wait=u32 2000) -> ()  [unwired: 1 out]
          }
          frame #6 {
            n434 = while {
              stop <- w753 stop-if-true
              n435 = local read "Saving..."() -> (w754:bool)
              n436 = Not(x=w754) -> (.not. x?=w753:bool)
            }
          }
          frame #7 {
            n437 = property on="Flip Green Filter" class="Bool (strict)"("Val(Sgnl)"=TRUE ("Value (Signaling)")) -> ()  [unwired: 2 in, 2 out]
            n438 = property on="Green Laser ON/Interlacing" class="Bool (strict)"("Val(Sgnl)"=w758) -> ()  [unwired: 2 in, 2 out]
            n439 = property on="Green laser mode" class="RadioBtnsControl (strict)"("Val(Sgnl)"=w757) -> ()  [unwired: 2 in, 2 out]
          }
          frame #8 {
            n440 = property on="Green FB On/Off" class="Bool (strict)"("Val(Sgnl)"=w759) -> ()  [unwired: 2 in, 2 out]
          }
        }
      }
      event "Stop All": Value Change {
        n441 = event-data() -> ()  [unwired: 1 in, 5 out]
        n442 = local read "Stop All"() -> (w760:bool)
      }
    }
    n443 = node-c288() -> ()  [unwired: 1 in, 1 out]
  }
  n444 = node-c288() -> (w90:T21)  [unwired: 4 out]
  n445 = timed-loop "Mouse control: trap position (AOM deflection), set confocal spot from image" {
    tunnel: [w762] -> w53
    tunnel: w49 -> [w761]
    timing: w90 -> [_]
    timing-out: [_] -> w89
    stop <- w762 stop-if-true
    n446 = node-c288() -> ()  [unwired: 2 out]
    n447 = event shown="[0] \"Pane\": Mouse Down" {
      selector: _ -> [_ _]
      dyn-events: _ -> [_ _]
      timeout: _ -> [_ _]
      tunnel: w761 -> [w765 _]
      event Mouse Down {
        n448 = event-data() -> ("Time"=w767:u32, "Coords"=w766:T8, "Button"=w768:u16)  [unwired: 6 out]
        n449 = case shown="1" w768 {
          tunnel: w767 -> [_ _ w871]
          tunnel: w766 -> [_ w805 w869]
          tunnel: w765 -> [_ _ w867]
          frame 0, Default {
          }
          frame 1 {
            n450 = property on="APD 2" class="ImageControl"() -> ("Displayed Image Position"=w775:cluster{"Left":i32, "Top":i32})  [unwired: 2 in, 2 out]
            n451 = property on="APD 1" class="ImageControl"() -> ("Displayed Image Position"=w804:cluster{"Left":i32, "Top":i32})  [unwired: 2 in, 2 out]
            n452 = property on="Detection Laser X" class="ImageControl"() -> ("Displayed Image Position"=w801:cluster{"Left":i32, "Top":i32})  [unwired: 2 in, 2 out]
            n453 = property on="Detection Laser Y" class="ImageControl"() -> ("Displayed Image Position"=w800:cluster{"Left":i32, "Top":i32})  [unwired: 2 in, 2 out]
            n454 = property on="APD 2" class="ImageControl"() -> ("Displayed Image Size"=w774:cluster{"Width":u32, "Height":u32})  [unwired: 2 in, 2 out]
            n455 = property on="APD 1" class="ImageControl"() -> ("Displayed Image Size"=w802:cluster{"Width":u32, "Height":u32})  [unwired: 2 in, 2 out]
            n456 = property on="Detection Laser X" class="ImageControl"() -> ("Displayed Image Size"=w803:cluster{"Width":u32, "Height":u32})  [unwired: 2 in, 2 out]
            n457 = property on="Detection Laser Y" class="ImageControl"() -> ("Displayed Image Size"=w799:cluster{"Width":u32, "Height":u32})  [unwired: 2 in, 2 out]
            n458 = Unbundle By Name(w774) -> ("Width"=w771:u32, "Height"=w770:u32)
            n459 = Unbundle By Name(w775) -> ("Left"=w773:i32, "Top"=w772:i32)
            n460 = Unbundle By Name(w802) -> ("Width"=w796:u32, "Height"=w795:u32)
            n461 = Unbundle By Name(w803) -> ("Width"=w792:u32, "Height"=w791:u32)
            n462 = Unbundle By Name(w799) -> ("Width"=w788:u32, "Height"=w787:u32)
            n463 = Unbundle By Name(w804) -> ("Left"=w798:i32, "Top"=w797:i32)
            n464 = Unbundle By Name(w801) -> ("Left"=w794:i32, "Top"=w793:i32)
            n465 = Unbundle By Name(w800) -> ("Left"=w790:i32, "Top"=w789:i32)
            n466 = Bundle("Left"=w773, "Top"=w772, "Width"=w771, "Height"=w770) -> (w769:T26)  [unwired: 1 in]
            n467 = Bundle("Left"=w798, "Top"=w797, "Width"=w796, "Height"=w795) -> (w786:T26)  [unwired: 1 in]
            n468 = Bundle("Left"=w794, "Top"=w793, "Width"=w792, "Height"=w791) -> (w785:T26)  [unwired: 1 in]
            n469 = Bundle("Left"=w790, "Top"=w789, "Width"=w788, "Height"=w787) -> (w784:T26)  [unwired: 1 in]
            n470 = Build Cluster Array(w769, w786, w785, w784) -> (w783:T27)
            n471 = for {
              tunnel: w805 -> [w816]
              tunnel: w783 -> [w817] mode=indexing
              shift-right: [w814] -> w781
              shift-left: TRUE -> [w815]
              shift-right: [w813] -> w779
              shift-left: _ -> [w809]
              shift-right: [w812] -> w778
              shift-left: _ -> [w808]
              shift-right: [w811] -> w777
              shift-left: _ -> [w807]
              shift-right: [w810] -> w776
              shift-left: _ -> [w806]
              n472 = case shown="True" w815 {
                selector: w815 -> [w822 _]
                tunnel: w817 -> [_ w831]
                tunnel: w816 -> [_ w829]
                tunnel: [w822 w827] -> w814
                tunnel: [w821 w826] -> w813
                tunnel: [w820 w825] -> w812
                tunnel: [w819 w824] -> w811
                tunnel: [w818 w823] -> w810
                tunnel: w809 -> [w821 _]
                tunnel: w808 -> [w820 _]
                tunnel: w807 -> [w819 _]
                tunnel: w806 -> [w818 _]
                frame False {
                }
                frame True {
                  n473 = Unbundle(w831) -> (w830:T26)
                  n474 = call "isclickinwindow.vi"("Image Param"=w830, "Point32"=w829) -> ("Y px"=w823:i32, "Height"=w824:i32, "X px"=w825:i32, "Width"=w826:i32, "In image?"=w828:bool)  [unwired: 1 in]
                  n475 = Not(x=w828) -> (.not. x?=w827:bool)
                }
              }
            }
            n476 = Not(x=w781) -> (.not. x?=w780:bool)
            n477 = case shown="True" w780 {
              tunnel: w778 -> [_ w844]
              tunnel: w776 -> [_ w843]
              tunnel: w779 -> [_ w842]
              tunnel: w777 -> [_ w841]
              frame False {
              }
              frame True {
                w837 = FALSE ("Get Point")
                n478 = local read "Scan lines (y)"() -> (w846:u64)
                n479 = local read "Actual MCL Inc (V)"() -> (w838:dbl)
                n480 = local read "Scan steps (x)"() -> (w845:u64)
                n481 = Divide "Y Pix/step"(x=w841, y=w846) -> (x/y=w853:dbl)
                n482 = Divide "Y V/pix"(x=w838, y=w853) -> (x/y=w852:dbl)
                n483 = Divide "Y half step offset"(x=w838, y=2.0) -> (x/y=w854:dbl)
                n484 = Divide "X pix/step"(x=w842, y=w845) -> (x/y=w851:dbl)
                n485 = Negate(x=w854) -> (-x=w855:dbl)
                n486 = local read "Initial Y"() -> (w861:dbl)
                n487 = Multiply(x=w843, y=w852) -> (x*y=w862:dbl)
                n488 = Divide "X half step offset"(x=w838, y=2.0) -> (x/y=w848:dbl)
                n489 = Divide "X V/pix"(x=w838, y=w851) -> (x/y=w850:dbl)
                n490 = Multiply(x=w838, y=w845) -> (x*y=w857:dbl)
                n491 = Compound Arithmetic op=ADD(w855, w862, w861) -> (w839:dbl)
                "Pointer Y (V)" <- w839
                n492 = Multiply(x=w850, y=w844) -> (x*y=w859:dbl)
                n493 = Negate(x=w848) -> (-x=w847:dbl)
                n494 = local read "Initial X"() -> (w860:dbl)
                n495 = Negate(x=w859) -> (-x=w858:dbl)
                n496 = Compound Arithmetic op=ADD(w847, w857, w860, w858) -> (w840:dbl)
                "Pointer X (V)" <- w840
                n497 = Or(x="Set X Only", y="Set Confocal Spot (X-Y)") -> (x .or. y?=w833:bool)
                n498 = Or(x="Set Confocal Spot (X-Y)", y="Set Y Only") -> (x .or. y?=w832:bool)
                n499 = case shown="True" w833 {
                  tunnel: w840 -> [_ w863]
                  frame False {
                  }
                  frame True {
                    n500 = property on="MCL X" class="Slide (strict)"("Val(Sgnl)"=w863) -> ()  [unwired: 2 in, 2 out]
                  }
                }
                n501 = case shown="True" w832 {
                  tunnel: w839 -> [_ w864]
                  frame False {
                  }
                  frame True {
                    n502 = property on="MCL Y" class="Slide (strict)"("Val(Sgnl)"=w864) -> ()  [unwired: 2 in, 2 out]
                  }
                }
                n503 = local write "Set Confocal Spot (X-Y)"(w837) -> ()
                n504 = local write "Set X Only"(w837) -> ()
                n505 = local write "Set Y Only"(w837) -> ()
              }
            }
          }
          frame 3 {
            n506 = local read "BD 2 Frq 1 (MHz)"() -> (w865:dbl)
            n507 = local read "BD 1 Frq 1 (MHz)"() -> (w866:dbl)
            n508 = local write "Manipulating Trap"(TRUE ("Manipulating Trap")) -> ()
            n509 = local write "Coords"(T8 {"Horizontal"=0, "Vertical"=0} ("Coords")) -> ()
            n510 = while {
              tunnel: w871 -> [w876]
              tunnel: w869 -> [w875]
              tunnel: w867 -> [w874]
              tunnel: w866 -> [w873]
              tunnel: w865 -> [w872]
              stop <- w877 stop-if-true
              n511 = event shown="[0] \"Pane\": Mouse Move" {
                selector: _ -> [_ _]
                dyn-events: _ -> [_ _]
                timeout: _ -> [_ _]
                tunnel: ["Force Manip Abort" w941] -> w877
                tunnel: w876 -> [w884 _]
                tunnel: w875 -> [w882 _]
                tunnel: w874 -> [w881 _]
                tunnel: w873 -> [w880 _]
                tunnel: w872 -> [w879 _]
                event Mouse Move {
                  n512 = event-data() -> ("Time"=w885:u32, "Coords"=w886:T8)  [unwired: 3 out]
                  n513 = Less?(x=w885, y=w884) -> (x < y?=w883:bool)
                  n514 = case "Makes sure old motion events prior to mouse click aren't used" shown="False" w883 {
                    tunnel: w886 -> [w928 _]
                    tunnel: w882 -> [w929 _]
                    tunnel: w881 -> [w906 _]
                    tunnel: w880 -> [w902 _]
                    tunnel: w879 -> [w901 _]
                    frame False {
                      n515 = Subtract(x=w928, y=w929) -> (x-y=w927:T8)
                      "Coords" <- w927
                      n516 = local read "Y RF Frequency Limits (MHz)"() -> (w887:T16)
                      n517 = To Double Precision Float(number=w927) -> (double precision float=w926:cluster{"Horizontal":dbl, "Vertical":dbl})
                      n518 = Multiply(x=cluster{"Horizontal":dbl, "Vertical":dbl} {"Horizontal"=-1.0, "Vertical"=1.0}, y="Manipulation Scaling") -> (x*y=w922:cluster{"Horizontal":dbl, "Vertical":dbl})
                      n519 = local read "X RF Frequency Limits (MHz)"() -> (w888:T16)
                      n520 = Multiply(x=w926, y=w922) -> (x*y=w924:cluster{"Horizontal":dbl, "Vertical":dbl})
                      n521 = Unbundle By Name(w924) -> ("Horizontal"=w919:dbl, "Vertical"=w923:dbl)
                      n522 = Unbundle By Name(w887) -> ("Maximum"=w890:dbl, "Minimum"=w889:dbl)
                      n523 = Boolean To (0,1)(Boolean="Manip. X?") -> (0, 1=w917:i16)
                      n524 = Boolean To (0,1)(Boolean="Manip. Y?") -> (0, 1=w914:i16)
                      n525 = Multiply(x=w923, y=w914) -> (x*y=w916:dbl)
                      n526 = Multiply(x=w917, y=w919) -> (x*y=w920:dbl)
                      n527 = local read "BD 1 Frq 2 (MHz)"() -> (w904:dbl)
                      n528 = Unbundle By Name(w888) -> ("Maximum"=w892:dbl, "Minimum"=w891:dbl)
                      n529 = local read "BD 2 Frq 2 (MHz)"() -> (w903:dbl)
                      n530 = Add(x=w901, y=w916) -> (x+y=w894:dbl)
                      n531 = Add(x=w902, y=w920) -> (x+y=w896:dbl)
                      n532 = In Range and Coerce(upper limit=w892, x=w896, lower limit=w891) -> (coerced(x)=w895:dbl)  [unwired: 1 out]
                      n533 = In Range and Coerce(upper limit=w890, x=w894, lower limit=w889) -> (coerced(x)=w893:dbl)  [unwired: 1 out]
                      n534 = Subtract(x=w895, y=w904) -> (x-y=w913:dbl)
                      n535 = Subtract(x=w893, y=w903) -> (x-y=w912:dbl)
                      n536 = Square(x=w913) -> (x^2=w911:dbl)
                      n537 = Square(x=w912) -> (x^2=w910:dbl)
                      n538 = Add(x=w911, y=w910) -> (x+y=w909:dbl)
                      n539 = Square Root(x=w909) -> (sqrt(x)=w905:dbl)
                      n540 = In Range and Coerce(upper limit="Limit Max (MHz)", x=w905, lower limit="Limit Min (MHz)") -> (In Range?=w898:bool)  [unwired: 1 out]
                      n541 = Not(x="Limits Enable") -> (.not. x?=w897:bool)
                      n542 = Or(x=w898, y=w897) -> (x .or. y?=w899:bool)
                      n543 = case shown="True" w899 {
                        tunnel: w906 -> [_ w939]
                        tunnel: w905 -> [_ w930]
                        tunnel: w895 -> [_ w937]
                        tunnel: w904 -> [_ w936]
                        tunnel: w893 -> [_ w935]
                        tunnel: w903 -> [_ w934]
                        tunnel: w888 -> [_ w932]
                        tunnel: w887 -> [_ w931]
                        frame False {
                        }
                        frame True {
                          n544 = local write "Trap Delta (MHz)"(w930) -> ()
                          n545 = local read "BD 1 Frq 3 (MHz)"() -> (w938:dbl)
                          n546 = property on="Initial delta (MHz)" class="DigNum (strict)"("Val(Sgnl)"=w930) -> ()  [unwired: 2 in, 2 out]
                          n547 = local read "BD 2 Frq 3 (MHz)"() -> (w933:dbl)
                          n548 = call "set RF board frequency - interlace.vi"("Board 2 Frequency Limits"=w931, "Board 1 Frequency Limits"=w932, "FPGA VI Reference In"=w939, "Board 2 Frequency 3 (MHz)"=w933, "Board 1 Frequency 3 (MHz)"=w938, "Board 2 Frequency 2 (MHz)"=w934, "Board 2 Frequency 1 (MHz)"=w935, "Board 1 Frequency 2 (MHz)"=w936, "Board 1 Frequency 1  (MHz)"=w937) -> ()  [unwired: 1 in, 2 out]
                          n549 = local write "BD 2 Frq 1 (MHz)"(w935) -> ()
                          n550 = local write "BD 1 Frq 1 (MHz)"(w937) -> ()
                        }
                      }
                    }
                    frame True {
                    }
                  }
                }
                event Mouse Up {
                  n551 = event-data() -> ("Button"=w940:u16)  [unwired: 8 out]
                  n552 = case shown="3" w940 {
                    tunnel: [FALSE TRUE] -> w941
                    frame 0, Default {
                    }
                    frame 3 {
                      n553 = local write "Manipulating Trap"(FALSE ("Manipulating Trap")) -> ()
                    }
                  }
                }
              }
            }
          }
        }
      }
      event Mouse Move {
        n554 = event-data() -> ()  [unwired: 6 out]
      }
    }
    n555 = local read "Stop All"() -> (w762:bool)
    n556 = node-c288() -> ()  [unwired: 2 out]
  }
  n557 = local read "Phase adj. (AI1)"() -> (w180:i16)
  n558 = local read "Phase adj. (GI)"() -> (w179:i16)
  n559 = local read "Phase adjust (MCL)"() -> (w178:i16)
  n560 = local read "Phase adj. (Green FB)"() -> (w126:i16)
  n561 = local read "Phase adj. (GI) 2"() -> (w97:i16)
  n562 = xnode "Read/Write Control"("FPGA VI Reference In"=w45, "error in"=w48, "Phase count adjustment"=w180, "Phase count adjustment (GI)"=w179, "Phase count adjustment (MCL)"=w178, "Phase Count Adjustment (APD Acq)"="Phase Adj. (APD Acq)", "Phase count adjustment (APD 1 Gate)"="Phase Adj. (APD 1 Gate)", "Phase count adjustment (APD 2 Gate)"="Phase Adj. (APD 2 Gate)", "Phase count adjustment (Green FB)"=w126, "Phase count adjustment (GI) 2"=w97) -> ("FPGA VI Reference Out"=w23:T20, "error out"=w22:errorcluster)
  n563 = Unbundle By Name(w33) -> ("Minimum"=w8:dbl, "Maximum"=w6:dbl)
  n564 = call "MHz2uint64.vi"("inMHz"=w8) -> ("outu64"=w7:u64)  [unwired: 4 in]
  n565 = call "MHz2uint64.vi"("inMHz"=w6) -> ("outu64"=w5:u64)  [unwired: 4 in]
  n566 = xnode "Read/Write Control"("FPGA VI Reference In"=w23, "FB Min frequency"=w7, "FB Max Frequency"=w5) -> ()  [unwired: 1 in, 2 out]
  n567 = call "set RF board frequency - interlace.vi"("Board 2 Frequency Limits"=w128, "Board 1 Frequency Limits"=w33, "error in"=w22, "FPGA VI Reference In"=w23, "Board 2 Frequency 3 (MHz)"="BD 2 Frq 3 (MHz)", "Board 1 Frequency 3 (MHz)"="BD 1 Frq 3 (MHz)", "Board 2 Frequency 2 (MHz)"="BD 2 Frq 2 (MHz)", "Board 2 Frequency 1 (MHz)"="BD 2 Frq 1 (MHz)", "Board 1 Frequency 2 (MHz)"="BD 1 Frq 2 (MHz)", "Board 1 Frequency 1  (MHz)"="BD 1 Frq 1 (MHz)") -> ("error out"=w243:errorcluster, "FPGA VI Reference Out"=w244:T20)
  n568 = Subtract(x="BD 1 Frq 1 (MHz)", y="BD 1 Frq 2 (MHz)") -> (x-y=w167:dbl)
  n569 = Subtract(x="BD 2 Frq 1 (MHz)", y="BD 2 Frq 2 (MHz)") -> (x-y=w166:dbl)
  n570 = Square(x=w166) -> (x^2=w164:dbl)
  n571 = Square(x=w167) -> (x^2=w165:dbl)
  n572 = Add(x=w165, y=w164) -> (x+y=w163:dbl)
  n573 = Square Root(x=w163) -> (sqrt(x)=w162:dbl)
  n574 = call "set RF board amplitude - interlace.vi"("Board 2 Amplitude Limits"=w127, "Board 1 Amplitude Limits"=w129, "error in"=w243, "FPGA VI Reference In"=w244, "Board 2 Amplitude 3 (%)"="BD 2 Amp 3 (%)", "Board 1 Amplitude 3 (%)"="BD 1 Amp 3 (%)", "Board 2 Amplitude 2 (%)"="BD 2 Amp 2 (%)", "Board 2 Amplitude 1 (%)"="BD 2 Amp 1 (%)", "Board 1 Amplitude 2 (%)"="BD 1 Amp 2 (%)", "Board 1 Amplitude 1 (%)"="BD 1 Amp 1 (%)") -> ("error out"=w43:errorcluster, "FPGA VI Reference Out"=w44:T20)
  n575 = local write "Trap Delta (MHz)"(w162) -> ()
  n576 = flat-sequence {
    tunnel: w44 -> [w946]
    tunnel: w43 -> [w945]
    tunnel: [w946] -> w236
    tunnel: [w945] -> w235
    tunnel: [w954] -> w234
    tunnel: w236 -> [w954]
    tunnel: [w953] -> w233
    tunnel: w235 -> [w953]
    tunnel: w234 -> [w957]
    tunnel: w233 -> [w956]
    tunnel: [w957] -> w39
    tunnel: [w956] -> w38
    tunnel: [w964] -> w59
    tunnel: [w967] -> w49
    tunnel: w39 -> [w967]
    tunnel: w38 -> [w963]
    frame #0 {
      n577 = local read "Trap 1 (ON/OFF)"() -> (w947:bool)
      n578 = local write "Stop All"(FALSE ("Stop All")) -> ()
      n579 = local write "Saving..."(FALSE ("Saving Data")) -> ()
      n580 = local write "Index"(1.0 ("Index")) -> ()
      n581 = property on="Trap 1 ON" class="Bool (strict)"("Value"=w947) -> ()  [unwired: 2 in, 2 out]
      "Manipulating Trap" <- FALSE ("Manipulating Trap")
    }
    frame #1 {
      n582 = local read "Trap 2 (ON/OFF)"() -> (w952:bool)
      n583 = Wait (ms)(milliseconds to wait=u32 50) -> ()  [unwired: 1 out]
      n584 = property on="Trap 2 ON" class="Bool (strict)"("Val(Sgnl)"=w952) -> ()  [unwired: 2 in, 2 out]
    }
    frame #2 {
      n585 = local read "Scan Range (nm)"() -> (w958:dbl)
      n586 = call "Update messages.vi"("Message to add"="UHR-Fleezers ready.", "Old message string"="") -> ("New message string"=w961:string)
      n587 = property on="Scan Range (nm)" class="DigNum (strict)"("Val(Sgnl)"=w958) -> ()  [unwired: 2 in, 2 out]
      n588 = local write "Messages"(w961) -> ()
    }
    frame #3 {
      n589 = call "hamilton_controller.vi"("error in"=w963, "action"=T25."CONNECT") -> ("error out"=w965:errorcluster)  [unwired: 9 in]
      n590 = case shown="True" "Reinit Valve?" {
        tunnel: w965 -> [w968 w971]
        tunnel: [w968 w970] -> w964
        frame False {
        }
        frame True {
          n591 = local write "Reinit Valve?"(FALSE ("Reinit Valve?")) -> ()
          n592 = call "hamilton_controller.vi"("error in"=w971, "action"=T25."INITIALIZE VALVES") -> ("error out"=w970:errorcluster)  [unwired: 9 in]
        }
      }
    }
  }
  n593 = node-c288(w82) -> ()  [unwired: 1 out]
  n594 = node-c288(w89) -> ()  [unwired: 1 out]
  n595 = call "IMAQ Create"("Image Name"="APD 1 Image", "Image Type"=w79) -> ("New Image"=w78:T4)  [unwired: 3 in, 1 out]
  n596 = call "IMAQ Create"("Image Name"="APD 2 Image", "Image Type"=w79) -> ("New Image"=w77:T4)  [unwired: 3 in, 1 out]
  n597 = call "IMAQ Create"("Image Name"="Det. X Image", "Image Type"=w79) -> ("New Image"=w76:T4)  [unwired: 3 in, 1 out]
  n598 = call "IMAQ Create"("Image Name"="Det. Y Image", "Image Type"=w79) -> ("New Image"=w75:T4)  [unwired: 3 in, 1 out]
  n599 = Bundle("New Image"=w78, "New Image"=w77, "New Image"=w76, "New Image"=w75) -> (w74:T28)  [unwired: 1 in]
  n600 = node-c288(2 ("Processor")) -> (w42:T21)  [unwired: 3 in]
  n601 = node-c288(i64 1 ("Period"), 1 ("Processor")) -> (w170:T21)  [unwired: 2 out]
  n602 = node-c288(3 ("Processor")) -> (w88:T21)  [unwired: 3 out]
  n603 = timed-loop "Control parameters (event loop)" {
    tunnel: w49 -> [w976]
    shift-right: [w975] -> _
    shift-left: errorcluster {"status"=FALSE, "code"=0, "source"=""} ("error out") -> [w974]
    tunnel: [w973] -> w56
    timing: w42 -> [_]
    timing-out: [_] -> w41
    stop <- w973 stop-if-true
    n604 = node-c288() -> ()  [unwired: 1 in, 1 out]
    n605 = event shown="[56] \"Target Force (pN)\", \"Setpoint offset Correction values\", \"Raster target force (pN)\": Value Change" {
      selector: _ -> [_ _ _ _ _ _ _ _ _ _ _ _ _ _ _ _ _ _ _ _ _ _ _ _ _ _ _ _ _ _ _ _ _ _ _ _ _ _ _ _ _ _ _ _ _ _ _ _ _ _ _ _ _ _ _ _ _ _ _ _]
      dyn-events: _ -> [_ _ _ _ _ _ _ _ _ _ _ _ _ _ _ _ _ _ _ _ _ _ _ _ _ _ _ _ _ _ _ _ _ _ _ _ _ _ _ _ _ _ _ _ _ _ _ _ _ _ _ _ _ _ _ _ _ _ _ _]
      timeout: _ -> [_ _ _ _ _ _ _ _ _ _ _ _ _ _ _ _ _ _ _ _ _ _ _ _ _ _ _ _ _ _ _ _ _ _ _ _ _ _ _ _ _ _ _ _ _ _ _ _ _ _ _ _ _ _ _ _ _ _ _ _]
      tunnel: w976 -> [w1017 _ _ w1040 _ w1058 w1064 _ _ _ _ w1141 _ _ w1185 w1191 w1195 w1200 w1236 w1254 w1261 w1279 w1290 w1301 w1312 w1323 w1334 w1352 w1358 w1452 _ w1464 w1502 _ w1572 w1577 w1581 w1592 w1597 w1621 _ w1629 _ _ _ _ _ w1765 w1780 w1795 w1821 w1824 w1847 w1907 _ w1924 w1927 _ _ _]
      tunnel: [w1016 _ _ w1030 _ _ w1063 _ _ w1106 _ w1121 _ _ w1184 w1187 w1194 w1197 w1235 w1252 w1260 w1273 w1284 w1295 w1306 w1317 w1328 w1350 w1357 w1450 _ w1462 w1500 _ _ w1575 w1579 w1582 w1595 w1619 _ w1627 _ _ _ _ _ w1763 _ _ _ _ _ _ _ _ _ _ _ _] -> w975
      tunnel: w974 -> [w1015 _ _ w1039 _ _ w1062 _ _ w1106 _ w1140 _ _ w1183 w1186 w1193 w1196 w1234 w1253 w1259 w1278 w1289 w1300 w1311 w1322 w1333 w1351 w1356 w1451 _ w1463 w1501 _ _ w1576 w1580 w1591 w1596 w1620 _ w1628 _ _ _ _ _ w1764 w1779 w1794 w1820 w1823 w1848 w1906 _ w1923 _ _ _ _]
      tunnel: [_ _ _ _ _ _ _ _ _ w1105 _ _ _ _ _ _ _ _ _ _ _ _ _ _ _ _ _ _ _ _ _ _ _ _ _ _ _ _ _ _ _ _ _ _ _ _ _ _ _ _ _ _ _ _ _ _ _ _ _ _] -> w973
      tunnel: [_ _ _ _ _ _ _ "Round T1 X" _ _ _ _ _ _ _ _ _ _ _ _ _ _ _ _ _ _ _ _ _ _ _ _ _ _ _ _ _ _ _ _ _ _ _ _ _ _ _ _ _ _ _ _ _ _ _ _ _ _ _ _] -> _
      tunnel: [_ _ _ _ _ _ _ _ _ _ _ _ _ _ _ _ _ _ _ _ _ _ _ _ _ _ _ _ _ _ _ _ _ _ _ _ _ _ _ _ _ _ _ _ _ _ _ _ _ _ _ _ _ "Set SP to Current Frc" _ _ _ _ _ _] -> _
      tunnel: [_ _ _ _ _ _ _ _ "Round T2 X" _ "Delayed Interlace Start" _ _ _ _ _ _ _ _ _ _ _ _ _ _ _ _ _ _ _ _ _ _ _ _ _ _ _ _ _ _ _ _ _ _ _ _ _ _ _ _ _ _ _ _ _ _ _ _ _] -> _
      event "AI Count (ticks)", "Sets to FIFO (Traps)", "Save ave N", "FPGA Ave.", "# Samples/channel", "N sets to save": Value Change {
        # "So that if 'Save ave N' is updated, the AOD scanning code updates too."
        n606 = event-data() -> ()  [unwired: 6 out]
        n607 = local read "AI Count (ticks)"() -> (w998:u32)
        n608 = Unbundle By Name("Sets to FIFO (Traps)") -> ("Set 1"=w981:bool, "Set 2"=w980:bool, "Set 3"=w979:bool)
        n609 = Boolean To (0,1)(Boolean="Sets to FIFO (Traps)") -> (0, 1=w1007:cluster{"Set 1":i16, "Set 2":i16, "Set 3":i16})
        n610 = xnode "Read/Write Control"("FPGA VI Reference In"=w1017, "error in"=w1015, "ai count"=w998, "Set 1"=w981, "Set 2"=w980, "Set 3"=w979, "N of AI1 Int Acq Sets"="N Acq Sets (Traps + Fl.)") -> ("error out"=w1016:errorcluster)  [unwired: 1 out]
        n611 = Cluster To Array(cluster=w1007) -> (array=w1006:i16[])
        n612 = To Unsigned Long Integer(number=w1006) -> (unsigned 32bit integer=w987:u32[])
        n613 = local read "Scan steps (AOD)"() -> (w1008:u64)
        n614 = Multiply(x=w998, y="N Acq Sets (Traps + Fl.)") -> (x*y=w996:u32)
        n615 = Divide(x=40000000.0, y=w998) -> (x/y=w990:dbl)
        "AI rate (Hz)" <- w990
        "Ave. Rate (Hz)" <- w990
        n616 = Add Array Elements(numeric array=w987) -> (sum=w999:u32)
        "Trap Sets" <- w999
        n617 = Reciprocal(x=w990) -> (1/x=→"Ave. Period (s)":dbl)
        n618 = property on="Scan steps (AOD)" class="DigNum (strict)"("Val(Sgnl)"=w1008) -> ()  [unwired: 2 in, 2 out]
        n619 = Divide(x=w990, y="N Acq Sets (Traps + Fl.)") -> (x/y=w1012:dbl)
        "Data Rate (Hz)" <- w1012
        n620 = Reciprocal(x=w1012) -> (1/x=→"Data Period (s)":dbl)
        n621 = local read "Save ave N"() -> (w1011:i32)
        n622 = Divide(x=w1012, y=w1011) -> (x/y=w1010:dbl)
        "Save Data Rate (Hz)" <- w1010
        n623 = Reciprocal(x=w1010) -> (1/x=→"Save Data Period (s)":dbl)
        n624 = Multiply(x=w996, y="# Samples/trap") -> (x*y=w994:u32)
        "Counts/DMA" <- w994
        n625 = property on="Trap Disp. Downsample" class="DigNum (strict)"("Maximum"="# Samples/trap") -> ()  [unwired: 2 in, 2 out]
        n626 = Multiply(x=w999, y="# Samples/trap") -> (x*y=w988:u32)
        "# Samples/channel" <- w988
        n627 = Multiply(x=w988, y=u32 8) -> (x*y=→"Trap AI Elements/DMA read":u32)
        n628 = local read "APD Int. Count"() -> (w995:u32)
        n629 = Multiply(x=w988, y=u32 3) -> (x*y=→"Trap Pos Elements/DMA read":u32)
        n630 = Divide(x=w994, y=w995) -> (x/y=w985:dbl)
        "APD Samples/FIFO Acq." <- w985
        n631 = Divide(x=w994, y=40000000.0) -> (x/y=w992:dbl)
        "DMA Update Period (s)" <- w992
        n632 = Multiply(x=2.0, y=w985) -> (x*y=→"APD Elements/DMA read":dbl)
        n633 = property on="APD Disp. dSamp" class="DigNum (strict)"("Maximum"=w985) -> ()  [unwired: 2 in, 2 out]
        n634 = local read "N sets to save"() -> (w1004:u32)
        n635 = Multiply(x=w992, y=w1004) -> (x*y=→"Total Time (s)":dbl)
        "FPGA Averaging" <- FALSE ("FPGA Averaging")
      }
      event "Rescale on Mean": Value Change {
        n636 = event-data() -> ()  [unwired: 7 out]
        n637 = And(x=FALSE, y="Rescale on Mean") -> (x .and. y?=w1019:bool)
        n638 = local write "Rescale on Mean"(w1019) -> ()
      }
      event "Detector Type": Value Change {
        n639 = event-data() -> ()  [unwired: 7 out]
        n640 = local read "AI labels"() -> (w1021:string[])
        n641 = Build Array (concatenate)(w1021, "none") -> (w1022:string[])
        n642 = property on="FFT 1 Choice 1" class="Ring (strict)"("Strings []"=w1022) -> ()  [unwired: 2 in, 2 out]
        n643 = property on="FFT 1 Choice 2" class="Ring (strict)"("Strings []"=w1022) -> ()  [unwired: 2 in, 2 out]
        n644 = property on="FFT 2 Choice 1" class="Ring (strict)"("Strings []"=w1022) -> ()  [unwired: 2 in, 2 out]
        n645 = property on="FFT 2 Choice 2" class="Ring (strict)"("Strings []"=w1022) -> ()  [unwired: 2 in, 2 out]
        n646 = Bundle("APD 1", "APD 2") -> (w1025:cluster{string, string})  [unwired: 1 out]
        n647 = Cluster To Array(cluster=w1025) -> (array=w1023:string[])
        n648 = Build Array (concatenate)(w1023, w1022) -> (w1027:string[])
        n649 = Array Size(array=w1027) -> (size(s)=w1028:i32)
        n650 = property on="Signals to Plot" class="LstBox (strict)"("Item Names"=w1027) -> ()  [unwired: 2 in, 2 out]
        n651 = property on="Signals to Plot" class="LstBox (strict)"("Number of Rows"=w1028) -> ()  [unwired: 2 in, 2 out]
        n652 = property on="All Signals" class="WFChart (strict)"("LegNumRows"=w1028) -> ()  [unwired: 2 in, 2 out]
      }
      event "Phase adj. (AI1)", "+ phase (AI1)", "- phase (AI1)": Value Change {
        n653 = event-data() -> ()  [unwired: 7 out]
        n654 = Negate(x="Phase adj. (AI1)") -> (-x=w1037:i16)
        n655 = Select(t=w1037, s="- phase (AI1)", f="Phase adj. (AI1)") -> (s? t:f=w1036:i16)
        n656 = xnode "Read/Write Control"("FPGA VI Reference In"=w1040, "error in"=w1039, "Phase count adjustment"=w1036) -> ("FPGA VI Reference Out"=w1035:T20, "error out"=w1034:errorcluster)
        n657 = Or(x="- phase (AI1)", y="+ phase (AI1)") -> (x .or. y?=w1031:bool)
        n658 = xnode "Read/Write Control"("FPGA VI Reference In"=w1035, "error in"=w1034, "+ phase"=w1031) -> ("error out"=w1030:errorcluster)  [unwired: 1 out]
      }
      event "Signals to Plot": Double Click {
        w1043 = u32 9868950 ("Color Box")
        n659 = event-data() -> ("Row"=w1045:i32)  [unwired: 9 out]
        n660 = property on="All Signals" class="WFChart (strict)"("Active Plot"=w1045) -> (error out=w1056:errorcluster)  [unwired: 2 in, 1 out]
        n661 = property on="All Signals" class="WFChart (strict)" props=["Plot", "Visible?", "Plot", "Plot Color"](error in=w1056) -> (error out=w1055:errorcluster, "Plot.Visible?"=w1054:bool)  [unwired: 1 in, 2 out]
        n662 = Select(t=FALSE ("Plot.Visible"), s=w1054, f=TRUE ("Plot.Visible")) -> (s? t:f=w1049:bool)
        n663 = property on="All Signals" class="WFChart (strict)"(error in=w1055, "Plot.Visible?"=w1049) -> (error out=w1051:errorcluster)  [unwired: 1 in, 1 out]
        n664 = property on="All Signals" class="WFChart (strict)"(error in=w1051) -> (error out=w1046:errorcluster, "Plot.Plot Color"=w1050:u32)  [unwired: 1 in, 1 out]
        n665 = property on="Signals to Plot" class="LstBox (strict)"(error in=w1046, "Active Row"=w1045) -> (error out=w1044:errorcluster)  [unwired: 1 in, 1 out]
        n666 = Select(t=w1050, s=w1049, f=u32 0) -> (s? t:f=w1047:u32)
        n667 = property on="Signals to Plot" class="LstBox (strict)"(error in=w1044, "CellFontColor"=w1047, "SelColor"=w1043, "CellBG"=w1043, "CellFontSize"=u32 20 ("Active Row:Cell Font:Size"), "CellFontBold"=TRUE ("Active Row:Cell Font:Bold")) -> ()  [unwired: 1 in, 2 out]
      }
      event "Dynamic Force FB": Value Change {
        n668 = event-data() -> ()  [unwired: 7 out]
        n669 = xnode "Read/Write Control"("FPGA VI Reference In"=w1058, "Dynamic Force FB (Ronen)"="Dynamic Force FB") -> ()  [unwired: 1 in, 2 out]
      }
      event "BD 1 Frq 1 (MHz)", "BD 1 Frq 2 (MHz)", "BD 1 Frq 3 (MHz)", "BD 2 Frq 1 (MHz)", "BD 2 Frq 2 (MHz)", "BD 2 Frq 3 (MHz)", "Trap Delta (MHz)": Value Change {
        # "anytime one of the frequencies is changed, write it to the RF board UNLESS Set 2 is being oscillated. The oscillation\nscript writes the frequencies to the RF board."
        n670 = event-data() -> ("CtlRef"=w1061:refnum<vi>)  [unwired: 6 out]
        n671 = control-ref of="Trap Delta (MHz)"() -> (w1060:refnum<vi>)
        n672 = Equal?(x=w1060, y=w1061) -> (x = y?=w1059:bool)
        n673 = case shown="False" "Oscillate Set 2" {
          tunnel: w1064 -> [w1085 _]
          tunnel: [w1084 w1097] -> w1063
          tunnel: w1062 -> [w1083 w1097]
          tunnel: w1059 -> [w1070 _]
          frame False {
            n674 = case shown="True" "Symmetric manual \ntrap motion" {
              tunnel: ["T2 for asymmetric\n(MHz)" w1096] -> w1071
              tunnel: "Trap Delta (MHz)" -> [w1090 w1095]
              tunnel: [w1089 w1092] -> w1067
              frame False {
                n675 = Subtract(x="T2 for asymmetric\n(MHz)", y=w1090) -> (x-y=w1089:dbl)
              }
              frame True {
                n676 = Divide(x=w1095, y=2) -> (x/y=w1093:dbl)
                n677 = Subtract(x="Middle freq for \nsymmetric (MHz)", y=w1093) -> (x-y=w1092:dbl)
                n678 = Add(x="Middle freq for \nsymmetric (MHz)", y=w1093) -> (x+y=w1096:dbl)
              }
            }
            n679 = local read "BD 1 Frq 2 (MHz)"() -> (w1072:dbl)
            n680 = local write "BD 1 Frq 1 (MHz)"(w1067) -> ()
            n681 = Select(t=w1071, s=w1070, f=w1072) -> (s? t:f=w1069:dbl)
            n682 = local read "Y RF Frequency Limits (MHz)"() -> (w1073:T16)
            n683 = local read "X RF Frequency Limits (MHz)"() -> (w1074:T16)
            n684 = local read "BD 1 Frq 3 (MHz)"() -> (w1086:dbl)
            n685 = local write "BD 1 Frq 2 (MHz)"(w1069) -> ()
            n686 = local read "BD 2 Frq 1 (MHz)"() -> (w1077:dbl)
            n687 = local read "BD 2 Frq 2 (MHz)"() -> (w1076:dbl)
            n688 = local read "BD 2 Frq 3 (MHz)"() -> (w1087:dbl)
            n689 = call "set RF board frequency - interlace.vi"("Board 2 Frequency Limits"=w1073, "Board 1 Frequency Limits"=w1074, "error in"=w1083, "FPGA VI Reference In"=w1085, "Board 2 Frequency 3 (MHz)"=w1087, "Board 1 Frequency 3 (MHz)"=w1086, "Board 2 Frequency 2 (MHz)"=w1076, "Board 2 Frequency 1 (MHz)"=w1077, "Board 1 Frequency 2 (MHz)"=w1069, "Board 1 Frequency 1  (MHz)"=w1067) -> ("error out"=w1084:errorcluster)  [unwired: 1 out]
            n690 = Subtract(x=w1077, y=w1076) -> (x-y=w1081:dbl)
            n691 = Subtract(x=w1069, y=w1067) -> (x-y=w1082:dbl)
            n692 = Square(x=w1081) -> (x^2=w1079:dbl)
            n693 = Square(x=w1082) -> (x^2=w1080:dbl)
            n694 = Add(x=w1080, y=w1079) -> (x+y=w1078:dbl)
            n695 = Square Root(x=w1078) -> (sqrt(x)=w1075:dbl)
            n696 = local write "Trap Delta (MHz)"(w1075) -> ()
            n697 = property on="Initial delta (MHz)" class="DigNum (strict)"("Val(Sgnl)"=w1075) -> ()  [unwired: 2 in, 2 out]
          }
          frame True {
          }
        }
      }
      event "Round T1 X": Value Change {
        n698 = event-data() -> ()  [unwired: 7 out]
        n699 = local read "BD 1 Frq 1 (MHz)"() -> (w1100:dbl)
        n700 = Round To Nearest(number=w1100) -> (nearest integer value=w1099:dbl)
        n701 = property on="BD 1 Frq 1 (MHz)" class="DigNum (strict)"("Val(Sgnl)"=w1099) -> ()  [unwired: 2 in, 2 out]
      }
      event "Round T2 X": Value Change {
        n702 = event-data() -> ()  [unwired: 7 out]
        n703 = local read "BD 1 Frq 2 (MHz)"() -> (w1102:dbl)
        n704 = Round To Nearest(number=w1102) -> (nearest integer value=w1101:dbl)
        n705 = property on="BD 1 Frq 2 (MHz)" class="DigNum (strict)"("Val(Sgnl)"=w1101) -> ()  [unwired: 2 in, 2 out]
      }
      event "Stop All": Value Change {
        n706 = event-data() -> ()  [unwired: 7 out]
        n707 = call "hamilton_controller.vi"("action"=T25."DISCONNECT") -> ()  [unwired: 10 in, 1 out]
        n708 = local read "Stop All"() -> (w1105:bool)
      }
      event "Delayed Interlace Start": Value Change {
        n709 = event-data() -> ()  [unwired: 7 out]
        n710 = flat-sequence {
          frame #0 {
            n711 = Multiply(x="Delay to Interlace (s)", y=1000.0) -> (x*y=w1108:dbl)
            n712 = Wait (ms)(milliseconds to wait=w1108) -> ()  [unwired: 1 out]
          }
          frame #1 {
            n713 = property on="Green laser mode" class="RadioBtnsControl (strict)"("Val(Sgnl)"=enum32{"Laser ON", "Laser OFF", "Interlace"}."Interlace" ("Value (Signaling)")) -> ()  [unwired: 2 in, 2 out]
          }
        }
      }
      event "BD 1 Amp 1 (%)", "BD 1 Amp 2 (%)", "BD 1 Amp 3 (%)", "BD 2 Amp 1 (%)", "BD 2 Amp 2 (%)", "BD 2 Amp 3 (%)", "Trap 1 ON", "Trap 2 ON", "Trap 3 ON", "Feedback On/Off", "All FB On/Off": Value Change {
        w1132 = i16 1 ("f")
        n714 = event-data() -> ()  [unwired: 7 out]
        n715 = local write "Trap 1 (ON/OFF)"("Trap 1 ON") -> ()
        n716 = local write "Trap 2 (ON/OFF)"("Trap 2 ON") -> ()
        n717 = Boolean To (0,1)(Boolean="Trap 3 ON") -> (0, 1=w1133:i16)
        n718 = Boolean To (0,1)(Boolean="Trap 1 ON") -> (0, 1=w1134:i16)
        n719 = Boolean To (0,1)(Boolean="Trap 2 ON") -> (0, 1=w1135:i16)
        n720 = Select(t=w1135, s="Trap ON/OFF X or Y Amp?", f=w1132) -> (s? t:f=w1130:i16)
        n721 = Select(t=w1134, s="Trap ON/OFF X or Y Amp?", f=w1132) -> (s? t:f=w1131:i16)
        n722 = Select(t=w1133, s="Trap ON/OFF X or Y Amp?", f=w1132) -> (s? t:f=w1129:i16)
        n723 = Select(t=w1132, s="Trap ON/OFF X or Y Amp?", f=w1135) -> (s? t:f=w1127:i16)
        n724 = Select(t=w1132, s="Trap ON/OFF X or Y Amp?", f=w1134) -> (s? t:f=w1128:i16)
        n725 = Select(t=w1132, s="Trap ON/OFF X or Y Amp?", f=w1133) -> (s? t:f=w1126:i16)
        n726 = And(x="All FB On/Off", y="Feedback On/Off") -> (x .and. y?=w1124:cluster{"Set 1":bool, "Set 2":bool})
        n727 = Unbundle By Name(w1124) -> ("Set 1"=w1120:bool, "Set 2"=w1117:bool)
        n728 = local read "BD 1 Amp 1 (%)"() -> (w1144:dbl)
        n729 = local read "BD 1 Amp 2 (%)"() -> (w1143:dbl)
        n730 = local read "BD 1 Amp 3 (%)"() -> (w1142:dbl)
        n731 = local read "Y RF Amplitude Limits (%)"() -> (w1113:T16)
        n732 = local read "X RF Amplitude Limits (%)"() -> (w1114:T16)
        n733 = local read "BD 2 Amp 1 (%)"() -> (w1145:dbl)
        n734 = local read "BD 2 Amp 2 (%)"() -> (w1146:dbl)
        n735 = local read "BD 2 Amp 3 (%)"() -> (w1147:dbl)
        n736 = And(x="Trap 2 ON", y=w1117) -> (x .and. y?=w1115:bool)
        n737 = And(x="Trap 1 ON", y=w1120) -> (x .and. y?=w1118:bool)
        n738 = Multiply(x=w1131, y=w1144) -> (x*y=w1139:dbl)
        n739 = Multiply(x=w1143, y=w1130) -> (x*y=w1137:dbl)
        n740 = Multiply(x=w1142, y=w1129) -> (x*y=w1138:dbl)
        n741 = Multiply(x=w1145, y=w1128) -> (x*y=w1148:dbl)
        n742 = Multiply(x=w1146, y=w1127) -> (x*y=w1149:dbl)
        n743 = Multiply(x=w1147, y=w1126) -> (x*y=w1150:dbl)
        n744 = call "set RF board amplitude - interlace.vi"("Board 2 Amplitude Limits"=w1113, "Board 1 Amplitude Limits"=w1114, "error in"=w1140, "FPGA VI Reference In"=w1141, "Board 2 Amplitude 3 (%)"=w1150, "Board 1 Amplitude 3 (%)"=w1138, "Board 2 Amplitude 2 (%)"=w1149, "Board 2 Amplitude 1 (%)"=w1148, "Board 1 Amplitude 2 (%)"=w1137, "Board 1 Amplitude 1 (%)"=w1139) -> ("error out"=w1122:errorcluster, "FPGA VI Reference Out"=w1123:T20)
        n745 = xnode "Read/Write Control"("FPGA VI Reference In"=w1123, "error in"=w1122, "FB On/Off Set 1"=w1118, "FB On/Off Set 2"=w1115) -> ("error out"=w1121:errorcluster)  [unwired: 1 out]
        n746 = case shown="True" "All FB On/Off" {
          frame False {
          }
          frame True {
            n747 = local write "Feedback overload"(FALSE) -> ()
          }
        }
      }
      event "Load parameters": Value Change {
        n748 = event-data() -> ()  [unwired: 7 out]
        n749 = property on="Saved AOD Raster Scan Parameter Sets" class="Arr (strict)"() -> ("Index Values"=w1162:u32[])  [unwired: 2 in, 2 out]
        n750 = Index Array(array=w1162, index=0) -> (element=w1159:u32)
        n751 = local write "Load parameters"(FALSE ("Load parameters")) -> ()
        n752 = Index Array(array="Saved AOD Raster Scan Parameter Sets", index=w1159) -> (element=w1158:T31)
        n753 = Unbundle By Name(w1158) -> ("Scan Range AOD (nm) 2"=w1157:dbl, "Step Size AOD (nm) 2"=w1156:dbl, "Scan Speed AOD (nm/s) 2"=w1155:dbl, "Number of scans (AOD) 2"=w1154:u16)
        n754 = flat-sequence {
          tunnel: w1157 -> [w1165]
          tunnel: w1156 -> [w1164]
          tunnel: w1155 -> [w1163]
          tunnel: w1154 -> [w1166]
          frame #0 {
            n755 = local write "Scan Speed (nm/s)"(w1163) -> ()
            n756 = local write "Scan Range (nm)"(w1165) -> ()
            n757 = local write "Step Size (nm)"(w1164) -> ()
          }
          frame #1 {
            n758 = property on="Number of F/B Scans (AOD)" class="DigNum (strict)"("Val(Sgnl)"=w1166) -> ()  [unwired: 2 in, 2 out]
          }
        }
      }
      event "Trap 1 (ON/OFF)", "Trap 2 (ON/OFF)": Value Change {
        n759 = event-data() -> ()  [unwired: 7 out]
        n760 = property on="Trap 2 ON" class="Bool (strict)"("Val(Sgnl)"="Trap 2 (ON/OFF)") -> ()  [unwired: 2 in, 2 out]
        n761 = property on="Trap 1 ON" class="Bool (strict)"("Val(Sgnl)"="Trap 1 (ON/OFF)") -> ()  [unwired: 2 in, 2 out]
      }
      event "DIO count 1 (ticks)", "DIO count 2 (ticks)", "DIO count 3 (ticks)", "Interlace", "Number Interlace Sets", "Not-Interlacing Set": Value Change {
        n762 = event-data() -> ()  [unwired: 7 out]
        n763 = local read "DIO count 3 (ticks)"() -> (w1179:u32)
        n764 = local read "DIO count 1 (ticks)"() -> (w1181:u32)
        n765 = local read "DIO count 2 (ticks)"() -> (w1180:u32)
        n766 = To Unsigned Byte Integer(number="Not-Interlacing Set") -> (unsigned 8bit integer=w1170:u8)
        n767 = Add(x=w1170, y=u8 1) -> (x+y=w1174:u8)
        n768 = xnode "Read/Write Control"("FPGA VI Reference In"=w1185, "error in"=w1183, "DIO count 1 (ticks)"=w1181, "DIO count 2 (ticks)"=w1180, "DIO count 3 (ticks)"=w1179, "Interlace ON/OFF"="Interlace", "Number Interlace Cycles"="Number Interlace Sets", "Interlace Off Parameters"=w1174) -> ("error out"=w1184:errorcluster)  [unwired: 1 out]
        n769 = Build Array(w1181, w1180, w1179) -> (w1172:u32[])
        n770 = Split 1D Array(array=w1172, index="Number Interlace Sets") -> (first subarray=w1182:u32[])  [unwired: 1 out]
        n771 = Index Array(array=w1172, index=w1170) -> (element=w1171:u32)
        n772 = Add Array Elements(numeric array=w1182) -> (sum=w1176:u32)
        n773 = Select(t=w1176, s="Interlace", f=w1171) -> (s? t:f=→"Total Counts (ticks)":u32)
      }
      event "Reset Feedback": Value Change {
        n774 = event-data() -> ()  [unwired: 7 out]
        n775 = Unbundle By Name("Reset Feedback") -> ("Set 1"=w1189:bool, "Set 2"=w1188:bool)
        n776 = xnode "Read/Write Control"("FPGA VI Reference In"=w1191, "error in"=w1186, "FB Reset Set 1"=w1189, "FB Reset Set 2"=w1188) -> ("error out"=w1187:errorcluster)  [unwired: 1 out]
      }
      event "PID gains": Value Change {
        n777 = event-data() -> ()  [unwired: 7 out]
        n778 = local read "PID gains"() -> (w1192:T10)
        n779 = xnode "Read/Write Control"("FPGA VI Reference In"=w1195, "error in"=w1193, "FB Gains"=w1192) -> ("error out"=w1194:errorcluster)  [unwired: 1 out]
      }
      event "AI2 to Setpoint", "Trap Intensity\nSetpoints (V)": Value Change {
        n780 = event-data() -> ()  [unwired: 7 out]
        n781 = xnode "Read/Write Control"("FPGA VI Reference In"=w1200, "error in"=w1196) -> ("FPGA VI Reference Out"=w1199:T20, "error out"=w1198:errorcluster, "AI2 Y Sum Set 1"=w1207:i16, "AI2 Y Sum Set 2"=w1206:i16)
        n782 = Cluster To Array(cluster="AI2 to Setpoint") -> (array=w1210:bool[])
        n783 = local read "AI2 (V)"() -> (w1208:cluster{"Set 1":dbl, "Set 2":dbl})
        n784 = Or Array Elements(Boolean array=w1210) -> (logical OR=w1211:bool)
        n785 = Bundle By Name(cluster=w1208, "Set 1"=w1207, "Set 2"=w1206) -> (w1205:cluster{"Set 1":dbl, "Set 2":dbl})
        n786 = Divide(x=w1205, y=3276.7) -> (x/y=w1204:cluster{"Set 1":dbl, "Set 2":dbl})
        "AI2 (V)" <- w1204
        n787 = case shown="True" w1211 {
          tunnel: [w1214 w1231] -> w1203
          tunnel: "AI2 to Setpoint" -> [_ w1227]
          tunnel: "Trap Intensity\nSetpoints (V)" -> [w1215 w1230]
          tunnel: w1204 -> [_ w1224]
          frame False {
            n788 = Multiply(x=3276.7, y=w1215) -> (x*y=w1216:cluster{"Set 1":dbl, "Set 2":dbl})
            n789 = To Word Integer(number=w1216) -> (16bit integer=w1214:cluster{"Set 1":i16, "Set 2":i16})
          }
          frame True {
            n790 = Unbundle By Name(w1224) -> ("Set 1"=w1223:dbl, "Set 2"=w1222:dbl)
            n791 = Unbundle By Name(w1230) -> ("Set 1"=w1229:dbl, "Set 2"=w1228:dbl)
            n792 = Unbundle By Name(w1227) -> ("Set 1"=w1226:bool, "Set 2"=w1225:bool)
            n793 = Select(t=w1223, s=w1226, f=w1229) -> (s? t:f=w1221:dbl)
            n794 = Select(t=w1222, s=w1225, f=w1228) -> (s? t:f=w1220:dbl)
            n795 = Bundle By Name(cluster=w1230, "Set 1"=w1221, "Set 2"=w1220) -> (w1218:cluster{"Set 1":dbl, "Set 2":dbl})
            n796 = local write "Trap Intensity\nSetpoints (V)"(w1218) -> ()
            n797 = Multiply(x=3276.7, y=w1218) -> (x*y=w1219:cluster{"Set 1":dbl, "Set 2":dbl})
            n798 = To Word Integer(number=w1219) -> (16bit integer=w1231:cluster{"Set 1":i16, "Set 2":i16})
          }
        }
        n799 = Unbundle By Name(w1203) -> ("Set 1"=w1202:i16, "Set 2"=w1201:i16)
        n800 = xnode "Read/Write Control"("FPGA VI Reference In"=w1199, "error in"=w1198, "FB Setpoint Set 1"=w1202, "FB Setpoint Set 2"=w1201) -> ("error out"=w1197:errorcluster)  [unwired: 1 out]
      }
      event "Invert GI": Value Change {
        n801 = event-data() -> ()  [unwired: 7 out]
        n802 = xnode "Read/Write Control"("FPGA VI Reference In"=w1236, "error in"=w1234, "Invert GI"="Invert GI", "Invert GI 2"="Invert GI") -> ("error out"=w1235:errorcluster)  [unwired: 1 out]
      }
      event "Green FB Setpoint (mV)", "Green FB Gains", "Green FB On/Off", "Current When FB OFF (%)", "Green int current ON count adj": Value Change {
        n803 = event-data() -> ()  [unwired: 7 out]
        n804 = local read "Green FB Setpoint (mV)"() -> (w1243:dbl)
        n805 = local read "Current When FB OFF (%)"() -> (w1246:dbl)
        n806 = Multiply(x=w1243, y=3.2767) -> (x*y=w1242:dbl)
        n807 = Multiply(x=w1246, y=655.35) -> (x*y=w1247:dbl)
        n808 = To Unsigned Word Integer(number=w1247) -> (unsigned 16bit integer=w1245:u16)
        n809 = local read "Green int current ON count adj"() -> (w1250:u32)
        n810 = local read "Green FB Gains"() -> (w1249:T10)
        n811 = local read "Green Laser ON/Interlacing"() -> (w1240:bool)
        n812 = local read "Green laser mode"() -> (w1239:enum32{"Laser ON", "Laser OFF", "Interlace"})
        n813 = local read "Green FB On/Off"() -> (w1251:bool)
        n814 = Equal?(x=w1239, y=enum32{"Laser ON", "Laser OFF", "Interlace"}."Interlace") -> (x = y?=w1237:bool)
        n815 = Compound Arithmetic op=AND(w1237, w1251, w1240) -> (w1241:bool)
        n816 = xnode "Read/Write Control"("FPGA VI Reference In"=w1254, "error in"=w1253, "Green FB Setpoint"=w1242, "Green FB On/Off"=w1241, "Current Out"=w1245, "Green int current ON count adj"=w1250, "Green FB Gains"=w1249) -> ("error out"=w1252:errorcluster)  [unwired: 1 out]
      }
      event "Green laser mode", "Green Laser ON/Interlacing": Value Change {
        n817 = event-data() -> ()  [unwired: 7 out]
        n818 = case shown="True" "Green Laser ON/Interlacing" {
          tunnel: "Green laser mode" -> [_ w1268]
          tunnel: [enum32{"Laser ON", "Laser OFF", "Interlace"}."Laser OFF" ("Green laser mode") w1268] -> w1256
          tunnel: [FALSE w1264] -> w1255
          frame False {
          }
          frame True {
            n819 = local read "Green FB On/Off"() -> (w1265:bool)
            n820 = Equal?(x=w1268, y=enum32{"Laser ON", "Laser OFF", "Interlace"}."Interlace") -> (x = y?=w1266:bool)
            n821 = And(x=w1266, y=w1265) -> (x .and. y?=w1264:bool)
          }
        }
        n822 = xnode "Read/Write Control"("FPGA VI Reference In"=w1261, "error in"=w1259, "Operating Mode"=w1256, "Operating Mode 2"=w1256, "Green FB On/Off"=w1255) -> ("error out"=w1260:errorcluster)  [unwired: 1 out]
      }
      event "- phase (APD 1 Gate)", "+ phase (APD 1 Gate)": Value Change {
        n823 = event-data() -> ()  [unwired: 7 out]
        n824 = local read "Phase Adj. (APD 1 Gate)"() -> (w1269:i16)
        n825 = Negate(x=w1269) -> (-x=w1277:i16)
        n826 = Select(t=w1277, s="- phase (APD 1 Gate)", f=w1269) -> (s? t:f=w1276:i16)
        n827 = Or(x="- phase (APD 1 Gate)", y="+ phase (APD 1 Gate)") -> (x .or. y?=w1272:bool)
        n828 = xnode "Read/Write Control"("FPGA VI Reference In"=w1279, "error in"=w1278, "Phase count adjustment (APD 1 Gate)"=w1276) -> ("FPGA VI Reference Out"=w1274:T20, "error out"=w1275:errorcluster)
        n829 = xnode "Read/Write Control"("FPGA VI Reference In"=w1274, "error in"=w1275, "+ phase (APD 1 Gate)"=w1272) -> ("error out"=w1273:errorcluster)  [unwired: 1 out]
      }
      event "+ phase (APD 2 Gate)", "- phase (APD 2 Gate)": Value Change {
        n830 = event-data() -> ()  [unwired: 7 out]
        n831 = local read "Phase Adj. (APD 2 Gate)"() -> (w1280:i16)
        n832 = Negate(x=w1280) -> (-x=w1288:i16)
        n833 = Select(t=w1288, s="- phase (APD 2 Gate)", f=w1280) -> (s? t:f=w1287:i16)
        n834 = Or(x="- phase (APD 2 Gate)", y="+ phase (APD 2 Gate)") -> (x .or. y?=w1283:bool)
        n835 = xnode "Read/Write Control"("FPGA VI Reference In"=w1290, "error in"=w1289, "Phase count adjustment (APD 2 Gate)"=w1287) -> ("FPGA VI Reference Out"=w1285:T20, "error out"=w1286:errorcluster)
        n836 = xnode "Read/Write Control"("FPGA VI Reference In"=w1285, "error in"=w1286, "+ phase (APD 2 Gate)"=w1283) -> ("error out"=w1284:errorcluster)  [unwired: 1 out]
      }
      event "Phase Adj. (APD Acq)", "+ phase (APD Acq)", "- phase (APD Acq)": Value Change {
        n837 = event-data() -> ()  [unwired: 7 out]
        n838 = local read "Phase Adj. (APD Acq)"() -> (w1293:i16)
        n839 = Negate(x=w1293) -> (-x=w1299:i16)
        n840 = Select(t=w1299, s="+ phase (APD Acq)", f=w1293) -> (s? t:f=w1298:i16)
        n841 = Or(x="+ phase (APD Acq)", y="- phase (APD Acq)") -> (x .or. y?=w1294:bool)
        n842 = xnode "Read/Write Control"("FPGA VI Reference In"=w1301, "error in"=w1300, "Phase Count Adjustment (APD Acq)"=w1298) -> ("FPGA VI Reference Out"=w1296:T20, "error out"=w1297:errorcluster)
        n843 = xnode "Read/Write Control"("FPGA VI Reference In"=w1296, "error in"=w1297, "+ phase (APD Acq)"=w1294) -> ("error out"=w1295:errorcluster)  [unwired: 1 out]
      }
      event "Phase adj. (GI)", "+ phase (GI)", "- phase (GI)": Value Change {
        n844 = event-data() -> ()  [unwired: 7 out]
        n845 = Negate(x="Phase adj. (GI)") -> (-x=w1310:i16)
        n846 = Select(t=w1310, s="+ phase (GI)", f="Phase adj. (GI)") -> (s? t:f=w1309:i16)
        n847 = Or(x="+ phase (GI)", y="- phase (GI)") -> (x .or. y?=w1305:bool)
        n848 = xnode "Read/Write Control"("FPGA VI Reference In"=w1312, "error in"=w1311, "Phase count adjustment (GI)"=w1309) -> ("FPGA VI Reference Out"=w1307:T20, "error out"=w1308:errorcluster)
        n849 = xnode "Read/Write Control"("FPGA VI Reference In"=w1307, "error in"=w1308, "+ phase (GI)"=w1305) -> ("error out"=w1306:errorcluster)  [unwired: 1 out]
      }
      event "Phase adj. (GI) 2", "+ phase (GI) 2", "- phase (GI) 2": Value Change {
        n850 = event-data() -> ()  [unwired: 7 out]
        n851 = Negate(x="Phase adj. (GI) 2") -> (-x=w1321:i16)
        n852 = Select(t=w1321, s="+ phase (GI) 2", f="Phase adj. (GI) 2") -> (s? t:f=w1320:i16)
        n853 = Or(x="+ phase (GI) 2", y="- phase (GI) 2") -> (x .or. y?=w1316:bool)
        n854 = xnode "Read/Write Control"("FPGA VI Reference In"=w1323, "error in"=w1322, "Phase count adjustment (GI) 2"=w1320) -> ("FPGA VI Reference Out"=w1318:T20, "error out"=w1319:errorcluster)
        n855 = xnode "Read/Write Control"("FPGA VI Reference In"=w1318, "error in"=w1319, "+ phase (GI) 2"=w1316) -> ("error out"=w1317:errorcluster)  [unwired: 1 out]
      }
      event "Phase adj. (Green FB)", "- phase (Green FB)", "+ phase (Green FB)": Value Change {
        n856 = event-data() -> ()  [unwired: 7 out]
        n857 = Negate(x="Phase adj. (Green FB)") -> (-x=w1332:i16)
        n858 = Select(t=w1332, s="+ phase (Green FB)", f="Phase adj. (Green FB)") -> (s? t:f=w1331:i16)
        n859 = Or(x="+ phase (Green FB)", y="- phase (Green FB)") -> (x .or. y?=w1327:bool)
        n860 = xnode "Read/Write Control"("FPGA VI Reference In"=w1334, "error in"=w1333, "Phase count adjustment (Green FB)"=w1331) -> ("FPGA VI Reference Out"=w1329:T20, "error out"=w1330:errorcluster)
        n861 = xnode "Read/Write Control"("FPGA VI Reference In"=w1329, "error in"=w1330, "+ phase (Green FB)"=w1327) -> ("error out"=w1328:errorcluster)  [unwired: 1 out]
      }
      event "Invert APD Gate", "APD Gate ON Count", "APD Gate OFF Count", "APD Gate", "APD Integration Time (s)", "APD 1 AO Mult.", "APD 2 AO Mult.": Value Change {
        n862 = event-data() -> ()  [unwired: 7 out]
        n863 = local read "APD Integration Time (s)"() -> (w1335:dbl)
        n864 = local read "APD Gate ON Count"() -> (w1348:u32)
        n865 = local read "APD Gate OFF Count"() -> (w1347:u32)
        n866 = local read "Invert APD Gate"() -> (w1349:bool)
        n867 = local read "APD Gate"() -> (w1346:enum32{"ON", "OFF", "Interlace"})
        n868 = Multiply(x=w1335, y=40000000.0) -> (x*y=w1344:dbl)
        n869 = Reciprocal(x=w1335) -> (1/x=→"APD Acq Rate (Hz)":dbl)
        n870 = To Unsigned Long Integer(number=w1344) -> (unsigned 32bit integer=w1343:u32)
        n871 = local read "DMA Update Period (s)"() -> (w1336:dbl)
        n872 = Divide(x=w1336, y=w1335) -> (x/y=w1339:dbl)
        n873 = local read "APD 1 AO Mult."() -> (w1341:i16)
        n874 = local read "APD 2 AO Mult."() -> (w1340:i16)
        n875 = Multiply(x=2.0, y=w1339) -> (x*y=w1338:dbl)
        n876 = local write "APD Samples/FIFO Acq."(w1339) -> ()
        n877 = local write "APD Elements/DMA read"(w1338) -> ()
        n878 = xnode "Read/Write Control"("FPGA VI Reference In"=w1352, "error in"=w1351, "Invert APD Gate"=w1349, "APD Gate ON Count"=w1348, "APD Gate OFF Count"=w1347, "APD Acq Rate Count"=w1343, "APD Gate Operating Mode"=w1346, "APD 1 AO scale factor"=w1341, "APD 2 AO scale factor"=w1340) -> ("error out"=w1350:errorcluster)  [unwired: 1 out]
      }
      event "GI Frequency, ON count", "Green FB Count", "GI Frequency, OFF count": Value Change {
        n879 = event-data() -> ()  [unwired: 7 out]
        n880 = xnode "Read/Write Control"("FPGA VI Reference In"=w1358, "error in"=w1356, "Green interlace ON count"="GI Frequency, ON count", "Green interlace OFF count"="GI Frequency, OFF count", "Green interlace ON count 2"="GI Frequency, ON count", "Green interlace OFF count 2"="GI Frequency, OFF count", "Green FB Count"="Green FB Count") -> ("error out"=w1357:errorcluster)  [unwired: 1 out]
      }
      event "Number of F/B Scans (AOD)", "Scan Speed (nm/s)", "Scan BD", "Initial delta (MHz)", "Step Size (nm)", "Scan Range (nm)": Value Change {
        w1420 = 123.0  # AOM cal (nm/MHz)
        n881 = event-data() -> ()  [unwired: 7 out]
        n882 = local read "AOM X Cal (nm/MHz)"() -> (w1395:dbl)
        n883 = local read "X RF Frequency Limits (MHz)"() -> (w1407:T16)
        n884 = local read "Y RF Frequency Limits (MHz)"() -> (w1404:T16)
        n885 = local read "BD 1 Frq 1 (MHz)"() -> (w1403:dbl)
        n886 = local read "BD 2 Frq 1 (MHz)"() -> (w1409:dbl)
        n887 = Negate(x="Scan Range (nm)") -> (-x=w1373:dbl)
        n888 = Divide(x=w1373, y=w1395) -> (x/y=w1377:dbl)
        n889 = Select(t=w1407, s="Scan BD", f=w1404) -> (s? t:f=w1406:T16)
        n890 = Select(t=w1403, s="Scan BD", f=w1409) -> (s? t:f=w1408:dbl)
        n891 = Unbundle By Name(w1406) -> ("Maximum"=w1415:dbl, "Minimum"=w1414:dbl)
        n892 = Add(x=w1377, y=w1408) -> (x+y=w1412:dbl)
        n893 = Divide(x=w1373, y="Step Size (nm)") -> (x/y=w1392:dbl)
        n894 = Divide(x="Step Size (nm)", y=w1395) -> (x/y=w1401:dbl)
        n895 = Absolute Value(x=w1392) -> (abs(x)=w1376:dbl)
        n896 = Sign(1:w1373) -> (0:w1374:dbl)
        n897 = In Range and Coerce(upper limit=w1415, x=w1412, lower limit=w1414) -> (coerced(x)=w1411:dbl, In Range?=w1413:bool)
        n898 = To Unsigned Quad Integer(1:w1376) -> (0:w1391:u64)
        "Scan steps (AOD)" <- w1391
        n899 = call "IR AOM freq to word.vi"("Frequency In (MHz)"=w1401) -> ("Frequency Word Out (double)"=w1398:dbl)
        n900 = Multiply(x=w1374, y=w1398) -> (x*y=w1375:dbl)
        n901 = Subtract(x=w1412, y=w1411) -> (x-y=w1410:dbl)
        n902 = To Quad Integer(1:w1375) -> (0:w1397:i64)
        "Incr. int (AOD)" <- w1397
        n903 = Subtract(x=w1377, y=w1410) -> (x-y=w1396:dbl)
        "Scan Range (MHz)" <- w1396
        n904 = Select(t=w1377, s=w1413, f=w1396) -> (s? t:f=w1416:dbl)
        n905 = Multiply(x=w1396, y=w1395) -> (x*y=w1394:dbl)
        n906 = Decrement(x=w1391) -> (x-1=w1444:u64)
        n907 = Negate(x=w1394) -> (-x=w1390:dbl)
        n908 = local write "Scan Range (nm)"(w1390) -> ()
        n909 = Divide(x=w1416, y=w1444) -> (x/y=w1400:dbl)
        "Scan Increment (MHz)" <- w1400
        n910 = call "IR AOM freq to word.vi"("Frequency In (MHz)"=w1400) -> ("Frequency Word Out (double)"=w1399:dbl)
        n911 = Divide(x="Step Size (nm)", y="Scan Speed (nm/s)") -> (x/y=w1387:dbl)
        n912 = To Quad Integer(1:w1399) -> ()  [unwired: 1 out]
        n913 = local read "Number Interlace Sets"() -> (w1371:u8)
        n914 = local read "AI Count (ticks)"() -> (w1372:u32)
        n915 = local read "Total Counts (ticks)"() -> (w1370:u32)
        n916 = local read "# Samples/trap"() -> (w1402:u32)
        n917 = Multiply(x=w1372, y=w1371) -> (x*y=w1369:u32)
        n918 = Divide(x=w1370, y=w1369) -> (x/y=w1368:dbl)
        n919 = Select(t=w1403, s="Scan BD", f=w1409) -> (s? t:f=w1441:dbl)
        "Initial freq. (MHz)" <- w1441
        n920 = Add(x=w1416, y=w1441) -> (x+y=→"Final freq. (MHz)":dbl)
        n921 = Divide(x=w1370, y=40000000.0) -> (x/y=w1386:dbl)
        n922 = Divide(x=w1387, y=w1386) -> (x/y=w1385:dbl)
        n923 = To Unsigned Quad Integer(1:w1385) -> (0:w1360:u64)
        n924 = Quotient & Remainder(x=w1360, y=u64 2) -> (x-y*floor(x/y)=w1364:u64)  [unwired: 1 out]
        n925 = Equal?(x=w1364, y=u64 0) -> (x = y?=w1362:bool)
        n926 = Decrement(x=w1360) -> (x-1=w1361:u64)
        n927 = Select(t=w1360, s=w1362, f=w1361) -> (s? t:f=w1359:u64)
        "Cycles/step (AOD)" <- w1359
        n928 = xnode "Read/Write Control"("FPGA VI Reference In"=w1452, "error in"=w1451, "Scan steps"=w1391, "Number of scans"="Number of F/B Scans (AOD)", "Cycles per step"=w1359, "Scan freq.  increment"=w1397, "Scan BD"="Scan BD") -> ("error out"=w1450:errorcluster)  [unwired: 1 out]
        n929 = Multiply(x=w1391, y=w1359) -> (x*y=w1445:u64)
        n930 = Multiply(x=w1445, y=u64 2) -> (x*y=w1367:u64)
        n931 = Multiply(x=w1368, y=w1367) -> (x*y=w1366:dbl)
        "Data points/scan (f/b)" <- w1366
        n932 = Multiply(x=w1366, y="Number of F/B Scans (AOD)") -> (x*y=w1448:dbl)
        "Data points/scans" <- w1448
        n933 = Divide(x=w1448, y=w1402) -> (x/y=→"N sets should be saved":dbl)
        n934 = Multiply(x=w1445, y=w1386) -> (x*y=w1384:dbl)
        "Time/Scan (s) (AOD)" <- w1384
        n935 = Select(t=w1416, s="Scan BD", f=0.0) -> (s? t:f=w1442:dbl)
        n936 = Select(t=0.0, s="Scan BD", f=w1416) -> (s? t:f=w1438:dbl)
        n937 = local read "BD 2 Frq 2 (MHz)"() -> (w1434:dbl)
        n938 = local read "BD 1 Frq 2 (MHz)"() -> (w1437:dbl)
        n939 = Add(x=w1438, y=w1409) -> (x+y=w1435:dbl)
        n940 = Add(x=w1403, y=w1442) -> (x+y=w1436:dbl)
        n941 = Multiply(x=w1384, y=2.0) -> (x*y=w1383:dbl)
        n942 = Multiply(x=w1383, y="Number of F/B Scans (AOD)") -> (x*y=w1380:dbl)
        n943 = Divide(x=w1380, y=60.0) -> (x/y=→"Time to Finish All (min)":dbl)
        n944 = Add(x="Trap 2 Bead Size (nm)", y="Trap 1 Bead Size (nm)") -> (x+y=w1424:dbl)
        n945 = local read "Initial delta (MHz)"() -> (w1421:dbl)
        n946 = Divide(x=w1424, y=2.0) -> (x/y=w1418:dbl)
        n947 = Subtract(x=w1435, y=w1434) -> (x-y=w1432:dbl)
        n948 = Subtract(x=w1436, y=w1437) -> (x-y=w1433:dbl)
        n949 = Square(x=w1432) -> (x^2=w1431:dbl)
        n950 = Square(x=w1433) -> (x^2=w1430:dbl)
        n951 = Add(x=w1430, y=w1431) -> (x+y=w1429:dbl)
        n952 = Square Root(x=w1429) -> (sqrt(x)=w1428:dbl)
        "Final delta (MHz)" <- w1428
        n953 = Multiply(x=w1420, y=w1428) -> (x*y=w1427:dbl)
        n954 = Multiply(x=w1421, y=w1420) -> (x*y=w1419:dbl)
        n955 = Subtract(x=w1419, y=w1418) -> (x-y=→"Initial sep (nm)":dbl)
        n956 = Subtract(x=w1427, y=w1418) -> (x-y=→"Final sep (nm)":dbl)
      }
      event "Raster Scanning...": Value Change {
        n957 = event-data() -> ("NewVal"=w1453:bool)  [unwired: 6 out]
        n958 = case shown="True" w1453 {
          frame False {
          }
          frame True {
            n959 = property on="BD 1 Frq 1 (MHz)" class="DigNum (strict)"("Val(Sgnl)"=65.0 ("Value (Signaling)")) -> ()  [unwired: 2 in, 2 out]
          }
        }
      }
      event "Phase increment trap 1", "Swap F1 and F2", "Freq switch delay", "Amp switch delay", "Phase increment trap 2", "RF phase reset before cycles", "Phase offset method": Value Change {
        n960 = event-data() -> ()  [unwired: 7 out]
        n961 = local read "Amp switch delay"() -> (w1459:u16)
        n962 = local read "Phase increment trap 1"() -> (w1458:fxp<+/-,64,32>)
        n963 = local read "Freq switch delay"() -> (w1461:u16)
        n964 = local read "Phase increment trap 2"() -> (w1457:fxp<+/-,64,32>)
        n965 = local read "RF phase reset before cycles"() -> (w1456:bool)
        n966 = local read "Swap F1 and F2"() -> (w1460:bool)
        n967 = local read "Phase offset method"() -> (w1455:u8)
        n968 = xnode "Read/Write Control"("FPGA VI Reference In"=w1464, "error in"=w1463, "BD 1 Delay (ticks)"=w1461, "Swap F1 and F2"=w1460, "Amp switch delay"=w1459, "Phase Trap 1"=w1458, "Phase Trap 2"=w1457, "RF phase reset before cycles"=w1456, "Phase offset method"=w1455) -> ("error out"=w1462:errorcluster)  [unwired: 1 out]
      }
      event "Scan steps (x)", "Number of scans (MCL)", "Scan Range (V)\n(of steps)", "2D or 1D Scan", "N APD Samp/step", "Fast Scan Dir", "Continuous MCL Scanning", "Scan lines (y)": Value Change {
        w1466 = 32767.0 ("y")
        n969 = event-data() -> ()  [unwired: 7 out]
        n970 = Select(t="Scan lines (y)", s="2D or 1D Scan", f="Number of scans (MCL)") -> (s? t:f=w1471:u64)
        n971 = Decrement(x="Scan steps (x)") -> (x-1=w1487:u64)
        n972 = Divide(x="Scan Range (V)\n(of steps)", y=w1487) -> (x/y=w1486:dbl)
        "Desired Scan Incr (V)" <- w1486
        n973 = local read "APD Integration Time (s)"() -> (w1479:dbl)
        n974 = Multiply(x=w1486, y=w1466) -> (x*y=w1495:dbl)
        n975 = Divide(x=w1495, y=10.0) -> (x/y=w1485:dbl)
        "Desired incr (int)" <- w1485
        n976 = local read "Update Count (MCL)"() -> (w1491:u32)
        n977 = Round Toward -Infinity(1:w1485) -> (0:w1494:dbl)
        n978 = To Word Integer(number=w1494) -> (16bit integer=w1469:i16)
        "Actual Incr. int (MCL)" <- w1469
        n979 = Multiply(x=w1479, y=40000000.0) -> (x*y=w1492:dbl)
        n980 = Divide(x=w1492, y=w1491) -> (x/y=w1490:dbl)
        n981 = Multiply(x=i16 10, y=w1469) -> (x*y=w1467:i16)
        n982 = Multiply(x="N APD Samp/step", y=w1490) -> (x*y=w1489:dbl)
        "Cycles/step (MCL)" <- w1489
        n983 = Divide(x=w1467, y=w1466) -> (x/y=→"Actual MCL Inc (V)":dbl)
        n984 = Multiply(x="N APD Samp/step", y="Scan steps (x)") -> (x*y=w1481:u64)
        n985 = local read "APD Samples/FIFO Acq."() -> (w1478:dbl)
        n986 = Multiply(x=w1481, y=u64 2) -> (x*y=w1480:u64)
        "Data points/scan (f+b)" <- w1480
        n987 = Multiply(x=w1480, y=w1471) -> (x*y=w1498:u64)
        "Data points/scans (MCL)" <- w1498
        n988 = Multiply(x=w1479, y=w1480) -> (x*y=w1472:dbl)
        "Time/f+b scan (s) (MCL)" <- w1472
        n989 = Divide(x=w1498, y=w1478) -> (x/y=→"N sets should be saved (MCL)":dbl)
        n990 = Multiply(x=w1472, y=w1471) -> (x*y=→"Total Time (s)":dbl)
        n991 = Not(x="Fast Scan Dir") -> (.not. x?=w1476:bool)
        n992 = xnode "Read/Write Control"("FPGA VI Reference In"=w1502, "error in"=w1501, "Scan steps (MCL)"="Scan steps (x)", "Number of scans (MCL)"=w1471, "Cycles per step (MCL)"=w1489, "Scan freq.  increment (MCL)"=w1469, "1D or 2D Scan?"="2D or 1D Scan", "MCL Scan Axis"=w1476, "Cont. Scan (MCL)"="Continuous MCL Scanning") -> ("error out"=w1500:errorcluster)  [unwired: 1 out]
      }
      event "Read Cal": Value Change {
        w1539 = 1000.0 ("y")
        w1527 = T30."big-endian, network order" ("byte order (0:big-endian, network order)")
        w1528 = -1 ("count (1)")
        n993 = event-data() -> ()  [unwired: 7 out]
        n994 = local read "Save file name"() -> (w1557:path)
        n995 = local write "Read Cal"(FALSE ("Read Cal")) -> ()
        n996 = Strip Path(path=w1557) -> (stripped path=w1556:path)  [unwired: 1 out]
        n997 = Path To String(path=w1556) -> (string=w1537:string)
        n998 = Concatenate Strings(w1537, "\\current.off" ("string")) -> (w1535:string)
        n999 = Concatenate Strings(w1537, "\\current.cal" ("string")) -> (w1554:string)
        n1000 = local read "Scale intensities"() -> (w1507:bool)
        n1001 = String To Path(string=w1554) -> (path=w1553:path)
        n1002 = String To Path(string=w1535) -> (path=w1534:path)
        n1003 = Open/Create/Replace File(file path (use dialog)=w1553, operation (0:open)=T29."open", access (0:read/write)=enum16{"read/write", "read-only", "write-only"}."read-only") -> (refnum out=w1560:refnum<file>, error out=w1549:errorcluster)  [unwired: 1 in, 3 out]
        n1004 = Deny Access(4:w1549, 7:w1560) -> (0:w1548:errorcluster, 3:w1552:refnum<file>)  [unwired: 1 out]
        n1005 = Open/Create/Replace File(file path (use dialog)=w1534, operation (0:open)=T29."open", access (0:read/write)=enum16{"read/write", "read-only", "write-only"}."read-only") -> (refnum out=w1531:refnum<file>)  [unwired: 1 in, 4 out]
        n1006 = Deny Access(7:w1531) -> (3:w1529:refnum<file>)  [unwired: 1 in, 2 out]
        n1007 = Read from Binary File(5:0.0, 8:w1548, 9:w1527, 10:w1528, 11:w1552) -> (0:w1547:errorcluster, 2:w1545:dbl[], 3:w1550:refnum<file>)  [unwired: 2 out]
        n1008 = Array To Cluster(array=w1545) -> (cluster=w1544:T32)
        n1009 = Unbundle(w1544) -> ("[0]"=w1518:dbl, "[1]"=w1517:dbl, "[2]"=w1504:dbl, "[3]"=w1506:dbl, "[4]"=w1543:dbl, "[5]"=w1542:dbl)
        n1010 = case "Cal is OK if you load a cal with scale intensities on - Alex 081418" shown="True" w1507 {
          tunnel: w1506 -> [w1562 w1565]
          tunnel: [w1562 w1564] -> w1505
          tunnel: w1504 -> [w1561 w1567]
          tunnel: [w1561 w1566] -> w1503
          frame False {
          }
          frame True {
            n1011 = local read "Scale factor"() -> (w1563:dbl)
            n1012 = Multiply(x=w1565, y=w1563) -> (x*y=w1564:dbl)
            n1013 = Multiply(x=w1567, y=w1563) -> (x*y=w1566:dbl)
          }
        }
        n1014 = Close File(refnum=w1550, error in=w1547) -> (error out=→"Read cal error":errorcluster)  [unwired: 1 out]
        n1015 = Multiply(x=w1542, y=w1539) -> (x*y=w1540:dbl)
        n1016 = local write "T2 kappa_x (pN/nm)"(w1505) -> ()
        n1017 = local write "T1 kappa_x (pN/nm)"(w1503) -> ()
        n1018 = local write "T1 alpha_x (nm/V)"(w1518) -> ()
        n1019 = local write "T2 alpha_x (nm/V)"(w1517) -> ()
        n1020 = Read from Binary File(5:0.0, 9:w1527, 10:w1528, 11:w1529) -> (2:w1523:dbl[], 3:w1526:refnum<file>)  [unwired: 1 in, 3 out]
        n1021 = Multiply(x=w1543, y=w1539) -> (x*y=w1541:dbl)
        n1022 = local write "T1 offset_x (mV)"(w1541) -> ()
        n1023 = local write "T2 offset_x (mV)"(w1540) -> ()
        n1024 = Close File(refnum=w1526) -> ()  [unwired: 1 in, 2 out]
        n1025 = Array Subset(array=w1523, index=3) -> (w1521:dbl[])  [unwired: 1 in]
        n1026 = Index Array(array=w1523, index=0) -> (element=→"Offset file step size":dbl)
        n1027 = Multiply(x=w1518, y=w1504) -> (x*y=w1515:dbl)
        n1028 = Multiply(x=w1517, y=w1506) -> (x*y=w1516:dbl)
        n1029 = Divide(x=w1516, y=w1515) -> (x/y=w1509:dbl)
        n1030 = Decimate 1D Array(w1521) -> (w1513:dbl[], w1514:dbl[])  [unwired: 1 out]
        n1031 = disable-structure "Removed B factor to improve position FB -Alex 081418 2of3" shown="Enabled" {
          disable-tunnel: w1509 -> [w1568 _]
          disable-tunnel: [w1568 1.0] -> w1508
          frame Disabled {
          }
          frame Enabled {
          }
        }
        n1032 = Bundle By Name(cluster="Offset Values", "Trap 1X offset"=w1513, "Trap 2X offset"=w1514) -> (w1519:T14)
        n1033 = Multiply(x=w1514, y=w1508) -> (x*y=w1512:dbl[])
        n1034 = Subtract(x=w1513, y=w1512) -> (x-y=w1511:dbl[])
        n1035 = local write "Offset Values"(w1519) -> ()
        n1036 = case shown="True" "Auto read offset\ncorrection" {
          tunnel: w1511 -> [_ w1570]
          frame False {
          }
          frame True {
            n1037 = property on="Setpoint offset\nCorrection values" class="Arr (strict)"("Val(Sgnl)"=w1570) -> ()  [unwired: 2 in, 2 out]
          }
        }
        n1038 = property on="B factor" class="DigNum (strict)"("Val(Sgnl)"=w1508) -> ()  [unwired: 2 in, 2 out]
      }
      event "Symmetric Raster/Feedback?": Value Change {
        n1039 = event-data() -> ()  [unwired: 7 out]
        n1040 = xnode "Read/Write Control"("FPGA VI Reference In"=w1572, "Symmetric FB/Raster"="Symmetric Raster/Feedback?") -> ()  [unwired: 1 in, 2 out]
      }
      event "Abort MCL Scan": Value Change {
        n1041 = event-data() -> ()  [unwired: 7 out]
        n1042 = local write "MCL Scanning"(FALSE ("MCL Scanning")) -> ()
        n1043 = xnode "Read/Write Control"("FPGA VI Reference In"=w1577, "error in"=w1576, "Abort scan (MCL)"="Abort MCL Scan") -> ("error out"=w1575:errorcluster)  [unwired: 1 out]
      }
      event "Update Count (MCL)": Value Change {
        n1044 = event-data() -> ()  [unwired: 7 out]
        n1045 = xnode "Read/Write Control"("FPGA VI Reference In"=w1581, "error in"=w1580, "MCL count"="Update Count (MCL)") -> ("error out"=w1579:errorcluster)  [unwired: 1 out]
      }
      event "Phase adjust (MCL)", "+ phase (MCL)", "- phase (MCL)": Value Change {
        n1046 = event-data() -> ()  [unwired: 7 out]
        n1047 = Negate(x="Phase adjust (MCL)") -> (-x=w1590:i16)
        n1048 = Select(t=w1590, s="- phase (MCL)", f="Phase adjust (MCL)") -> (s? t:f=w1588:i16)
        n1049 = Or(x="- phase (MCL)", y="+ phase (MCL)") -> (x .or. y?=w1583:bool)
        n1050 = xnode "Read/Write Control"("FPGA VI Reference In"=w1592, "error in"=w1591, "Phase count adjustment (MCL)"=w1588) -> ("FPGA VI Reference Out"=w1584:T20, "error out"=w1585:errorcluster)
        n1051 = xnode "Read/Write Control"("FPGA VI Reference In"=w1584, "error in"=w1585, "+ phase (MCL)"=w1583) -> ("error out"=w1582:errorcluster)  [unwired: 1 out]
      }
      event "Abort AOD Scan": Value Change {
        n1052 = event-data() -> ()  [unwired: 7 out]
        n1053 = flat-sequence {
          tunnel: w1597 -> [w1604]
          tunnel: w1596 -> [w1603]
          tunnel: [w1602] -> w1594
          tunnel: [w1598] -> w1593
          tunnel: [w1617] -> w1595
          tunnel: w1594 -> [w1617]
          tunnel: w1593 -> [w1616]
          frame #0 {
            n1054 = local read "Save scans"() -> (w1600:bool)
            n1055 = xnode "Read/Write Control"("FPGA VI Reference In"=w1604, "error in"=w1603, "Abort scan"="Abort AOD Scan") -> ("FPGA VI Reference Out"=w1598:T20, "error out"=w1602:errorcluster)
            n1056 = case shown="True" w1600 {
              frame False {
              }
              frame True {
                n1057 = local write "Stop Saving"(TRUE) -> ()
              }
            }
            n1058 = local write "Raster Scanning..."(FALSE) -> ()
          }
          frame #1 {
            n1059 = xnode "Read/Write Control"("FPGA VI Reference In"=w1616) -> ("BD1 Frequency Out 1"=w1607:u64)  [unwired: 1 in, 2 out]
            n1060 = To Double Precision Float(number=w1607) -> (double precision float=w1613:dbl)
            n1061 = Multiply(x=49125000.0, y=6.0) -> (x*y=w1612:dbl)
            n1062 = Multiply(x=w1613, y=w1612) -> (x*y=w1610:dbl)
            n1063 = Scale By Power Of 2(n=-48, x=w1610) -> (x*2^n=w1609:dbl)
            n1064 = Divide(x=w1609, y=1000000.0) -> (x/y=w1606:dbl)
            n1065 = property on="BD 1 Frq 1 (MHz)" class="DigNum (strict)"("Val(Sgnl)"=w1606) -> ()  [unwired: 2 in, 2 out]
          }
        }
      }
      event "Continuous AOD Scanning": Value Change {
        n1066 = event-data() -> ()  [unwired: 7 out]
        n1067 = xnode "Read/Write Control"("FPGA VI Reference In"=w1621, "error in"=w1620, "Cont. Scan"="Continuous AOD Scanning") -> ("error out"=w1619:errorcluster)  [unwired: 1 out]
      }
      event "Index": Value Change {
        n1068 = event-data() -> ()  [unwired: 7 out]
        n1069 = call "Create new save file.vi"("Insert"="", "Ext"=".dat" ("string"), "Index In"="Index") -> ("Path Out"=→"Save file name":path, "Index Out"=w1622:dbl)
        "Save index" <- w1622
        n1070 = local write "Index"(w1622) -> ()
      }
      event "MCL Y", "MCL X": Value Change {
        w1637 = 10.0 ("y")
        w1636 = 32767.0 ("y")
        n1071 = event-data() -> ()  [unwired: 7 out]
        n1072 = local read "MCL X"() -> (w1635:dbl)
        n1073 = local read "MCL Y"() -> (w1632:dbl)
        n1074 = Multiply(x=w1632, y=w1636) -> (x*y=w1631:dbl)
        n1075 = Multiply(x=w1635, y=w1636) -> (x*y=w1634:dbl)
        n1076 = Divide(x=w1631, y=w1637) -> (x/y=w1630:dbl)
        n1077 = Divide(x=w1634, y=w1637) -> (x/y=w1633:dbl)
        n1078 = To Word Integer(number=w1630) -> (16bit integer=w1638:i16)
        n1079 = To Word Integer(number=w1633) -> (16bit integer=w1639:i16)
        n1080 = xnode "Read/Write Control"("FPGA VI Reference In"=w1629, "error in"=w1628, "AO1 (Y)"=w1638, "AO2 (X)"=w1639) -> ("error out"=w1627:errorcluster)  [unwired: 1 out]
      }
      event "Inject Top:": Value Change {
        n1081 = event-data() -> ()  [unwired: 7 out]
        n1082 = disable-structure shown="Disabled" {
          disable-tunnel: "Inject Top:" -> [w1641 w1681]
          frame Disabled {
            n1083 = local read "Chemyx Syringe Pump Serial Port"() -> (w1642:refnum<visa-resource-name>)
            n1084 = local read "Pump write delay (ms)"() -> (w1643:dbl)
            n1085 = case shown="True" w1641 {
              tunnel: w1643 -> [w1649 w1663]
              tunnel: w1642 -> [w1646 w1662]
              frame False {
                n1086 = flat-sequence {
                  tunnel: w1646 -> [w1650]
                  tunnel: [w1650] -> w1647
                  tunnel: w1649 -> [_]
                  tunnel: [w1653] -> w1648
                  tunnel: w1647 -> [w1653]
                  tunnel: w1648 -> [w1654]
                  tunnel: [w1654] -> w1644
                  tunnel: [w1656] -> w1645
                  tunnel: w1644 -> [w1656]
                  tunnel: w1645 -> [w1658]
                  frame #0 {
                    n1087 = call "Write to pump.vi"("string"="enter pump1", "VISA resource name"=w1650) -> ()  [unwired: 1 out]
                  }
                  frame #1 {
                    n1088 = Wait (ms)(milliseconds to wait="Pump pause delay (ms)") -> ()  [unwired: 1 out]
                  }
                  frame #2 {
                    n1089 = call "Write to pump.vi"("string"="stop", "VISA resource name"=w1654) -> ()  [unwired: 1 out]
                  }
                  frame #3 {
                    n1090 = Wait (ms)(milliseconds to wait=u32 500) -> ()  [unwired: 1 out]
                  }
                  frame #4 {
                    n1091 = call "Write to pump.vi"("string"="stop", "VISA resource name"=w1658) -> ()  [unwired: 1 out]
                  }
                }
              }
              frame True {
                n1092 = flat-sequence {
                  tunnel: w1662 -> [w1672]
                  tunnel: w1663 -> [w1667]
                  tunnel: w1663 -> [w1674]
                  tunnel: w1662 -> [w1675]
                  tunnel: [w1675] -> w1660
                  tunnel: [w1677] -> w1661
                  tunnel: w1660 -> [w1677]
                  tunnel: w1661 -> [w1679]
                  frame #0 {
                    n1093 = local read "All Pump Parameters"() -> (w1666:T6)
                    n1094 = Unbundle By Name(w1666) -> ("Pump 1"=w1673:T33)
                    n1095 = call "Set pump parameters.vi"("Pump write delay (ms)"=w1667, "Volume (uL)"="Ch 2 Inject Volume (uL)", "Rate (uL/h)"="Ch 1 Inject Rate (ul/h)", "Units"=4.0, "Pump #"=1.0, "Pump Parameters In"=w1673, "VISA resource name"=w1672) -> ("Pump Parameters Out"=w1665:T33)  [unwired: 3 in]
                    n1096 = Bundle By Name(cluster=w1666, "Pump 1"=w1665) -> (w1664:T6)
                    n1097 = local write "All Pump Parameters"(w1664) -> ()
                  }
                  frame #1 {
                    n1098 = Wait (ms)(milliseconds to wait=w1674) -> ()  [unwired: 1 out]
                  }
                  frame #2 {
                    n1099 = call "Write to pump.vi"("string"="start", "VISA resource name"=w1675) -> ()  [unwired: 1 out]
                  }
                  frame #3 {
                    n1100 = Wait (ms)(milliseconds to wait=u32 500) -> ()  [unwired: 1 out]
                  }
                  frame #4 {
                    n1101 = call "Write to pump.vi"("string"="start", "VISA resource name"=w1679) -> ()  [unwired: 1 out]
                  }
                }
              }
            }
          }
          frame Enabled {
            n1102 = call "hamilton_controller.vi"("Open?"=w1681, "valve"=enum16{"A", "B", "C", "D", "ALL"}."B", "action"=T25."MOVE VALVE") -> ()  [unwired: 8 in, 1 out]
          }
        }
      }
      event "Main:": Value Change {
        n1103 = event-data() -> ()  [unwired: 7 out]
        n1104 = disable-structure shown="Enabled" {
          disable-tunnel: "Main:" -> [_ w1725]
          frame Disabled {
            n1105 = local read "Pump write delay (ms)"() -> (w1686:dbl)
            n1106 = case shown="False" w1687 {
              tunnel: w1686 -> [w1693 w1707]
              tunnel: "Chemyx Syringe Pump Serial Port" -> [w1690 w1706]
              frame False {
                n1107 = flat-sequence {
                  tunnel: w1690 -> [w1694]
                  tunnel: [w1694] -> w1691
                  tunnel: w1693 -> [_]
                  tunnel: [w1697] -> w1692
                  tunnel: w1691 -> [w1697]
                  tunnel: w1692 -> [w1698]
                  tunnel: [w1698] -> w1688
                  tunnel: [w1700] -> w1689
                  tunnel: w1688 -> [w1700]
                  tunnel: w1689 -> [w1702]
                  frame #0 {
                    n1108 = call "Write to pump.vi"("string"="enter pump3", "VISA resource name"=w1694) -> ()  [unwired: 1 out]
                  }
                  frame #1 {
                    n1109 = local read "Pump pause delay (ms)"() -> (w1696:u32)
                    n1110 = Wait (ms)(milliseconds to wait=w1696) -> ()  [unwired: 1 out]
                  }
                  frame #2 {
                    n1111 = call "Write to pump.vi"("string"="stop", "VISA resource name"=w1698) -> ()  [unwired: 1 out]
                  }
                  frame #3 {
                    n1112 = Wait (ms)(milliseconds to wait=u32 0) -> ()  [unwired: 1 out]
                  }
                  frame #4 {
                    n1113 = call "Write to pump.vi"("string"="stop", "VISA resource name"=w1702) -> ()  [unwired: 1 out]
                  }
                }
              }
              frame True {
                n1114 = flat-sequence {
                  tunnel: w1706 -> [w1716]
                  tunnel: w1707 -> [w1711]
                  tunnel: w1707 -> [w1718]
                  tunnel: w1706 -> [w1719]
                  tunnel: [w1719] -> w1704
                  tunnel: [w1722] -> w1705
                  tunnel: w1704 -> [w1722]
                  tunnel: w1705 -> [w1723]
                  frame #0 {
                    n1115 = local read "All Pump Parameters"() -> (w1710:T6)
                    n1116 = Unbundle By Name(w1710) -> ("Pump 3"=w1717:T33)
                    n1117 = call "Set pump parameters.vi"("Pump write delay (ms)"=w1711, "Volume (uL)"="Ch 3 Inject Volume (uL)", "Rate (uL/h)"="Ch 3 Inject Rate (ul/h)", "Units"=4.0, "Pump #"=3.0, "Pump Parameters In"=w1717, "VISA resource name"=w1716) -> ("Pump Parameters Out"=w1709:T33)  [unwired: 3 in]
                    n1118 = Bundle By Name(cluster=w1710, "Pump 3"=w1709) -> (w1708:T6)
                    n1119 = local write "All Pump Parameters"(w1708) -> ()
                  }
                  frame #1 {
                    n1120 = Wait (ms)(milliseconds to wait=w1718) -> ()  [unwired: 1 out]
                  }
                  frame #2 {
                    n1121 = call "Write to pump.vi"("string"="start", "VISA resource name"=w1719) -> ()  [unwired: 1 out]
                  }
                  frame #3 {
                    n1122 = Wait (ms)(milliseconds to wait=u32 500) -> ()  [unwired: 1 out]
                  }
                  frame #4 {
                    n1123 = call "Write to pump.vi"("string"="start", "VISA resource name"=w1723) -> ()  [unwired: 1 out]
                  }
                }
              }
            }
          }
          frame Enabled {
            n1124 = call "hamilton_controller.vi"("Open?"=w1725, "valve"=enum16{"A", "B", "C", "D", "ALL"}."A", "action"=T25."MOVE VALVE") -> ()  [unwired: 8 in, 1 out]
          }
        }
      }
      event "Inject Valve B": Value Change {
        n1125 = event-data() -> ()  [unwired: 7 out]
        n1126 = disable-structure shown="Enabled" {
          disable-tunnel: "Inject Valve B" -> [w1729 w1749]
          frame Disabled {
            n1127 = local read "Pump write delay (ms)"() -> (w1731:dbl)
            n1128 = flat-sequence {
              tunnel: w1730 -> [w1744]
              tunnel: w1731 -> [w1740]
              tunnel: w1729 -> [_]
              tunnel: w1731 -> [w1746]
              tunnel: w1730 -> [w1747]
              frame #0 {
                n1129 = local read "All Pump Parameters"() -> (w1739:T6)
                n1130 = Multiply(x=60.0, y="Flush Center Ch Rate (ul/m)") -> (x*y=w1736:dbl)
                n1131 = Unbundle By Name(w1739) -> ("Pump 2"=w1745:T33)
                n1132 = call "Set pump parameters.vi"("Pump write delay (ms)"=w1740, "Volume (uL)"="Flush Center Ch Volume (uL)", "Rate (uL/h)"=w1736, "Units"=3.0, "Pump #"=2.0, "Pump Parameters In"=w1745, "VISA resource name"=w1744) -> ("Pump Parameters Out"=w1738:T33)  [unwired: 3 in]
                n1133 = Bundle By Name(cluster=w1739, "Pump 2"=w1738) -> (w1737:T6)
                n1134 = local write "All Pump Parameters"(w1737) -> ()
                n1135 = Add(x="Flush Center Ch Volume (uL)", y="Total Volume\nFlushed (uL)") -> (x+y=w1733:dbl)
                n1136 = local write "Total Volume\nFlushed (uL)"(w1733) -> ()
              }
              frame #1 {
                n1137 = Wait (ms)(milliseconds to wait=w1746) -> ()  [unwired: 1 out]
              }
              frame #2 {
                n1138 = call "Write to pump.vi"("string"="start", "VISA resource name"=w1747) -> ()  [unwired: 1 out]
              }
            }
            n1139 = local read "Chemyx Syringe Pump Serial Port"() -> (w1730:refnum<visa-resource-name>)
          }
          frame Enabled {
            n1140 = call "hamilton_controller.vi"("Open?"=w1749, "valve"=enum16{"A", "B", "C", "D", "ALL"}."B", "action"=T25."MOVE VALVE") -> ()  [unwired: 8 in, 1 out]
          }
        }
      }
      event "Inject Bottom": Value Change {
        n1141 = event-data() -> ()  [unwired: 7 out]
        n1142 = call "hamilton_controller.vi"("Open?"="Inject Bottom", "valve"=enum16{"A", "B", "C", "D", "ALL"}."C", "action"=T25."MOVE VALVE") -> ()  [unwired: 8 in, 1 out]
      }
      event "Shunt:": Value Change {
        n1143 = event-data() -> ()  [unwired: 7 out]
        n1144 = call "hamilton_controller.vi"("Open?"="Shunt:", "valve"=enum16{"A", "B", "C", "D", "ALL"}."D", "action"=T25."MOVE VALVE") -> ()  [unwired: 8 in, 1 out]
      }
      event "Flip Green Filter": Value Change {
        n1145 = event-data() -> ()  [unwired: 7 out]
        n1146 = local write "Flip Green Filter"("Flip Green Filter") -> ()
        n1147 = flat-sequence {
          tunnel: w1765 -> [w1770]
          tunnel: w1764 -> [w1769]
          tunnel: [w1767] -> w1762
          tunnel: [w1766] -> w1761
          tunnel: [w1772] -> w1760
          tunnel: w1762 -> [w1772]
          tunnel: [w1771] -> w1759
          tunnel: w1761 -> [w1771]
          tunnel: w1760 -> [w1776]
          tunnel: w1759 -> [w1775]
          tunnel: [w1774] -> w1763
          frame #0 {
            n1148 = xnode "Read/Write Control"("FPGA VI Reference In"=w1770, "error in"=w1769, "Green Filter Flipper"=TRUE) -> ("FPGA VI Reference Out"=w1767:T20, "error out"=w1766:errorcluster)
          }
          frame #1 {
            n1149 = Wait (ms)(milliseconds to wait=u32 100) -> ()  [unwired: 1 out]
          }
          frame #2 {
            n1150 = xnode "Read/Write Control"("FPGA VI Reference In"=w1776, "error in"=w1775, "Green Filter Flipper"=FALSE) -> ("error out"=w1774:errorcluster)  [unwired: 1 out]
          }
        }
      }
      event "Reset Trap Pos. FB": Value Change {
        n1151 = event-data() -> ()  [unwired: 7 out]
        n1152 = xnode "Read/Write Control"("FPGA VI Reference In"=w1780, "error in"=w1779, "Trap Pos. FB Reset"="Reset Trap Pos. FB") -> ()  [unwired: 2 out]
      }
      event "Trap Pos. FB ON": Value Change {
        n1153 = event-data() -> ()  [unwired: 7 out]
        n1154 = xnode "Read/Write Control"("FPGA VI Reference In"=w1795, "error in"=w1794) -> ("FPGA VI Reference Out"=w1792:T20, "BD1 Frequency Out 1"=w1789:u64)  [unwired: 1 out]
        n1155 = To Double Precision Float(number=w1789) -> (double precision float=w1788:dbl)
        n1156 = Multiply(x=49125000.0, y=6.0) -> (x*y=w1787:dbl)
        n1157 = Multiply(x=w1788, y=w1787) -> (x*y=w1785:dbl)
        n1158 = Scale By Power Of 2(n=-48, x=w1785) -> (x*2^n=w1784:dbl)
        n1159 = Divide(x=w1784, y=1000000.0) -> (x/y=w1781:dbl)
        n1160 = flat-sequence {
          tunnel: [w1798] -> w1793
          tunnel: w1792 -> [w1799]
          tunnel: w1789 -> [w1797]
          tunnel: "Trap Pos. FB ON" -> [w1796]
          tunnel: "Trap Pos. FB ON" -> [w1805]
          tunnel: w1793 -> [w1804]
          tunnel: "Trap Pos. FB ON" -> [w1807]
          tunnel: w1781 -> [w1806]
          frame #0 {
            n1161 = case shown="False" w1796 {
              tunnel: w1799 -> [w1802 w1803]
              tunnel: [w1801 w1803] -> w1798
              tunnel: w1797 -> [w1800 _]
              frame False {
                n1162 = xnode "Read/Write Control"("FPGA VI Reference In"=w1802, "BD 1 Frequency 1"=w1800) -> ("FPGA VI Reference Out"=w1801:T20)  [unwired: 1 in, 1 out]
              }
              frame True {
              }
            }
          }
          frame #1 {
            n1163 = xnode "Read/Write Control"("FPGA VI Reference In"=w1804, "Force feedback"=w1805) -> ()  [unwired: 1 in, 2 out]
          }
          frame #2 {
            n1164 = case shown="False" w1807 {
              tunnel: w1806 -> [w1810 _]
              frame False {
                n1165 = local read "T2 for asymmetric\n(MHz)"() -> (w1808:dbl)
                n1166 = Subtract(x=w1808, y=w1810) -> (x-y=w1809:dbl)
                n1167 = property on="Trap Delta (MHz)" class="DigNum (strict)"("Val(Sgnl)"=w1809) -> ()  [unwired: 2 in, 2 out]
              }
              frame True {
              }
            }
          }
        }
      }
      event "Diff. FB.", "Trap Pos. FB Gains", "Trap Pos. FB Mult Factor", "Trap Pos. FB Offset Factor", "Trap Pos FB Negate Action", "Trap Pos FB Monitor\nT1 or T2", "Negate Diff?": Value Change {
        n1168 = event-data() -> ()  [unwired: 7 out]
        n1169 = xnode "Read/Write Control"("FPGA VI Reference In"=w1821, "error in"=w1820, "Trap pos. FB Range"="Trap Pos. FB Range", "Trap Pos. FB Gains"="Trap Pos. FB Gains", "Trap Pos. FB Mult Factor"="Trap Pos. FB Mult Factor", "Trap Pos. FB Offset Factor"="Trap Pos. FB Offset Factor", "Trap Pos FB Negate Action"="Trap Pos FB Negate Action", "Trap Pos FB Monitor T1 or T2"="Trap Pos FB Monitor\nT1 or T2", "AI1 X Scale"="Trap Pos. AI1 X Pre-scale", "Negate Diff?"="Negate Diff?", "Diff FB Measurement?"="Diff. FB.") -> ()  [unwired: 2 out]
      }
      event "Trap Pos FB SP": Value Change {
        n1170 = event-data() -> ()  [unwired: 7 out]
        n1171 = xnode "Read/Write Control"("FPGA VI Reference In"=w1824, "error in"=w1823, "Trap Pos. FB SP"="Trap Pos FB SP") -> ()  [unwired: 2 out]
        n1172 = disable-structure shown="Disabled" {
          frame Disabled {
            n1173 = local read "Trap X AI1 (DMA)"() -> (w1845:T13)
            n1174 = local read "Trap X (AI1)"() -> (w1846:T1)
            n1175 = local read "Setpoint offset\nCorrection values"() -> (w1839:dbl[])
            n1176 = local read "Trap Delta (MHz)"() -> (w1843:dbl)
            n1177 = local read "B factor"() -> (w1830:dbl)
            n1178 = Unbundle(w1846) -> ("Trap 1"=w1844:fxp<+/-,16,1>, "Trap 2"=w1833:fxp<+/-,16,1>)
            n1179 = Unbundle(w1845) -> ("Set 1"=w1829:fxp<+/-,16,1>, "Set 2"=w1828:fxp<+/-,16,1>)
            n1180 = Negate(x=w1833) -> (-x=w1826:fxp<+/-,17,2>)
            n1181 = Negate(x=w1844) -> (-x=w1827:fxp<+/-,17,2>)
            n1182 = Divide(x=w1843, y=0.1) -> (x/y=w1841:dbl)
            n1183 = Multiply(x=w1828, y=w1830) -> (x*y=w1831:dbl)
            n1184 = Subtract(x=w1829, y=w1831) -> (x-y=w1836:dbl)
            n1185 = To Long Integer(number=w1841) -> (32bit integer=w1840:i32)
            n1186 = Index Array(array=w1839, index=w1840) -> (element=w1835:dbl)
            n1187 = Multiply(x=w1830, y=w1826) -> (x*y=w1832:dbl)
            n1188 = Subtract(x=w1827, y=w1832) -> (x-y=w1838:dbl)
            n1189 = Add(x=w1838, y=w1835) -> (x+y=→"ideal setpoint fpga":dbl)
            n1190 = Add(x=w1836, y=w1835) -> (x+y=→"ideal setpoint avgd":dbl)
          }
          frame Enabled {
          }
        }
        n1191 = disable-structure shown="Enabled" {
          frame Enabled {
          }
          frame Disabled {
            n1192 = local write "B factor"(1.0 ("B factor")) -> ()
          }
        }
      }
      event "Simulate stepping": Value Change {
        n1193 = event-data() -> ()  [unwired: 7 out]
        n1194 = flat-sequence {
          tunnel: w1848 -> [w1851]
          tunnel: [w1850] -> _
          tunnel: w1847 -> [w1849]
          frame #0 {
            n1195 = while {
              tunnel: w1851 -> [w1879]
              tunnel: [w1878] -> w1850 mode=indexing
              tunnel: w1849 -> [w1877]
              i -> [w1863]
              stop <- w1860 stop-if-true
              w1853 = 1000.0
              n1196 = Divide(x="Backtrack probability", y=100) -> (x/y=w1887:dbl)
              n1197 = Random Number (0-1)() -> (number: 0 to 1=w1888:dbl)
              n1198 = Greater?(x=w1888, y=w1887) -> (0:w1886:bool)
              n1199 = Select(t=1, s=w1886, f=-1) -> (s? t:f=w1883:i32)
              n1200 = local read "BD 1 Frq 2 (MHz)"() -> (w1858:dbl)
              n1201 = Multiply(x=w1883, y="Step size (nm)") -> (x*y=w1881:dbl)
              "Step taken" <- w1881
              n1202 = Divide(x=w1881, y=168.33) -> (x/y=w1856:dbl)
              n1203 = local read "X RF Frequency Limits (MHz)"() -> (w1876:T16)
              n1204 = local read "BD 1 Frq 1 (MHz)"() -> (w1857:dbl)
              n1205 = local read "Y RF Frequency Limits (MHz)"() -> (w1875:T16)
              n1206 = Subtract(x=w1857, y=w1856) -> (x-y=w1855:dbl)
              n1207 = local write "BD 1 Frq 1 (MHz)"(w1855) -> ()
              n1208 = local read "BD 2 Frq 1 (MHz)"() -> (w1873:dbl)
              n1209 = local read "BD 2 Frq 2 (MHz)"() -> (w1874:dbl)
              n1210 = call "set RF board frequency - interlace.vi"("Board 2 Frequency Limits"=w1875, "Board 1 Frequency Limits"=w1876, "error in"=w1879, "FPGA VI Reference In"=w1877, "Board 2 Frequency 2 (MHz)"=w1874, "Board 2 Frequency 1 (MHz)"=w1873, "Board 1 Frequency 2 (MHz)"=w1858, "Board 1 Frequency 1  (MHz)"=w1855) -> ("error out"=w1878:errorcluster)  [unwired: 2 in, 1 out]
              n1211 = Subtract(x=w1858, y=w1855) -> (x-y=w1872:dbl)
              n1212 = Subtract(x=w1874, y=w1873) -> (x-y=w1871:dbl)
              n1213 = Square(x=w1871) -> (x^2=w1869:dbl)
              n1214 = Square(x=w1872) -> (x^2=w1870:dbl)
              n1215 = Add(x=w1870, y=w1869) -> (x+y=w1868:dbl)
              n1216 = Square Root(x=w1868) -> (sqrt(x)=w1859:dbl)
              n1217 = local write "Trap Delta (MHz)"(w1859) -> ()
              n1218 = property on="Initial delta (MHz)" class="DigNum (strict)"("Val(Sgnl)"=w1859) -> ()  [unwired: 2 in, 2 out]
              n1219 = Multiply(x="Mean dwell time (s)", y=w1853) -> (x*y=w1865:dbl)
              n1220 = case shown="\"Gamma2\"" "Distribution" {
                tunnel: w1865 -> [w1892 w1896 w1899]
                tunnel: [w1892 w1893 w1900] -> w1854
                frame "uniform", Default {
                }
                frame "Exponential" {
                  n1221 = call-poly <vilib>:"Continuous Random.vi"("b"=w1896, "samples"=1) -> ("exp random data"=w1894:dbl[])  [unwired: 8 in, 1 out]
                  n1222 = Index Array(array=w1894) -> (element=w1893:dbl)  [unwired: 1 in]
                }
                frame "Gamma2" {
                  w1897 = 2.0
                  # "Note: the shape and scale\nparameters of the gamma\nare inverted because LabView..."
                  n1223 = Divide(x=w1899, y=w1897) -> (x/y=w1898:dbl)
                  n1224 = call-poly <vilib>:"Continuous Random.vi"("c"=w1898, "b"=w1897, "samples"=1) -> ("gamma random numbers"=w1901:dbl[])  [unwired: 7 in, 1 out]
                  n1225 = Index Array(array=w1901) -> (element=w1900:dbl)  [unwired: 1 in]
                }
              }
              n1226 = Divide(x=w1854, y=w1853) -> (x/y=→"Step duration":dbl)
              n1227 = To Unsigned Long Integer(number=w1854) -> (unsigned 32bit integer=w1866:u32)
              n1228 = Add(x=w1863, y=1) -> (x+y=w1862:i32)
              n1229 = Wait (ms)(milliseconds to wait=w1866) -> ()  [unwired: 1 out]
              n1230 = Equal?(x=w1862, y="Number of steps") -> (x = y?=w1860:bool)
            }
          }
          frame #1 {
            n1231 = local write "Simulate stepping"(FALSE) -> ()
          }
        }
      }
      event "Set SP to Current Frc": Value Change {
        n1232 = event-data() -> ()  [unwired: 7 out]
        n1233 = local read "Trap Pos FB Monitor\nT1 or T2"() -> (w1911:bool)
        n1234 = local read "Trap X AI1 (DMA)"() -> (w1914:T13)
        n1235 = local read "Trap X (AI1)"() -> (w1917:T1)
        n1236 = Unbundle By Name(w1917) -> ("Trap 1"=w1916:fxp<+/-,16,1>, "Trap 2"=w1915:fxp<+/-,16,1>)
        n1237 = Unbundle By Name(w1914) -> ("Set 1"=w1913:fxp<+/-,16,1>, "Set 2"=w1912:fxp<+/-,16,1>)
        n1238 = Select(t=w1916, s=w1911, f=w1915) -> (s? t:f=w1910:fxp<+/-,16,1>)
        n1239 = Select(t=w1913, s=w1911, f=w1912) -> (s? t:f=w1909:fxp<+/-,16,1>)
        n1240 = Not(x="Set SP Using...") -> (.not. x?=w1904:bool)
        n1241 = Select(t=w1910, s=w1904, f=w1909) -> (s? t:f=w1905:fxp<+/-,16,1>)
        n1242 = xnode "Read/Write Control"("FPGA VI Reference In"=w1907, "error in"=w1906, "Trap Pos. FB SP"=w1905) -> ()  [unwired: 2 out]
        n1243 = local write "Trap Pos FB SP"(w1905) -> ()
      }
      event "Trap Pos. FB Out Scale 2^n": Value Change {
        n1244 = event-data() -> ()  [unwired: 7 out]
        n1245 = Scale By Power Of 2(n="Trap Pos. FB Out Scale 2^n", x=ext 1.0) -> (x*2^n=w1919:ext)
        n1246 = property on="Trap Pos. FB Mult Factor" class="DigNum (strict)"("Val(Sgnl)"=w1919) -> ()  [unwired: 2 in, 2 out]
      }
      event "Trap Pos FB Int Count": Value Change {
        n1247 = event-data() -> ()  [unwired: 7 out]
        n1248 = xnode "Read/Write Control"("FPGA VI Reference In"=w1924, "error in"=w1923, "Trap Pos FB Int Count"="Trap Pos FB Int Count") -> ()  [unwired: 2 out]
      }
      event "Target Force (pN)", "Setpoint offset\nCorrection values", "Raster target force (pN)": Value Change {
        w1933 = 2.0
        n1249 = event-data() -> ()  [unwired: 7 out]
        n1250 = disable-structure "Removed B Factor to improve position feedback - Alex 081418 1of3" shown="Enabled" {
          disable-tunnel: [w1963 fxp<+/-,32,16> 1.0 ("B factor")] -> w1925
          frame Disabled {
            n1251 = local read "B factor"() -> (w1964:dbl)
            n1252 = To Fixed-Point(number=w1964) -> (fixed-point=w1963:fxp<+/-,16,16>)  [unwired: 1 in]
          }
          frame Enabled {
          }
        }
        n1253 = xnode "Read/Write Control"("FPGA VI Reference In"=w1927, "B factor"=w1925) -> ("BD1 Frequency Out 1"=w1954:u64)  [unwired: 1 in, 2 out]
        n1254 = local read "BD 1 Frq 2 (MHz)"() -> (w1953:dbl)
        n1255 = local read "Target Force (pN)"() -> (w1939:dbl)
        n1256 = To Double Precision Float(number=w1954) -> (double precision float=w1960:dbl)
        n1257 = Multiply(x=49125000.0, y=6.0) -> (x*y=w1959:dbl)
        n1258 = Multiply(x=w1960, y=w1959) -> (x*y=w1957:dbl)
        n1259 = Scale By Power Of 2(n=-48, x=w1957) -> (x*2^n=w1956:dbl)
        n1260 = Divide(x=w1956, y=1000000.0) -> (x/y=w1952:dbl)
        n1261 = Subtract(x=w1953, y=w1952) -> (x-y=w1951:dbl)
        n1262 = local read "T1 kappa_x (pN/nm)"() -> (w1940:dbl)
        n1263 = local read "T1 alpha_x (nm/V)"() -> (w1941:dbl)
        n1264 = local read "Negate offset difference"() -> (w1942:bool)
        n1265 = local read "Offset file step size"() -> (w1950:dbl)
        n1266 = Multiply(x="Raster target force (pN)", y=w1933) -> (x*y=w1932:dbl)
        n1267 = Multiply(x=w1939, y=w1933) -> (x*y=w1938:dbl)
        n1268 = local read "Setpoint offset\nCorrection values"() -> (w1947:dbl[])
        n1269 = Divide(x=w1951, y=w1950) -> (x/y=w1949:dbl)
        n1270 = Select(t=-1, s=w1942, f=1) -> (s? t:f=w1943:i32)
        n1271 = To Long Integer(number=w1949) -> (32bit integer=w1948:i32)
        n1272 = Multiply(x=w1941, y=w1940) -> (x*y=w1931:dbl)
        n1273 = Divide(x=w1938, y=w1931) -> (x/y=w1937:dbl)
        n1274 = Index Array(array=w1947, index=w1948) -> (element=w1946:dbl)
        n1275 = Divide(x=w1932, y=w1931) -> (x/y=w1930:dbl)
        n1276 = Multiply(x=w1943, y=w1946) -> (x*y=w1929:dbl)
        n1277 = Add(x=w1937, y=w1929) -> (x+y=w1936:dbl)
        n1278 = Add(x=w1930, y=w1929) -> (x+y=w1928:dbl)
        n1279 = To Fixed-Point(number=w1928) -> (fixed-point=w1926:fxp<+/-,16,1>)  [unwired: 1 in]
        n1280 = To Fixed-Point(number=w1936) -> (fixed-point=w1935:fxp<+/-,16,1>)  [unwired: 1 in]
        n1281 = property on="Trap Pos FB SP" class="DigNum (strict)"("Val(Sgnl)"=w1935) -> ()  [unwired: 2 in, 2 out]
        n1282 = xnode "Read/Write Control"("FPGA VI Reference In"=w1927, "Raster setpoint"=w1926) -> ()  [unwired: 1 in, 2 out]
      }
      event "Read setpoint correction\nfile": Value Change {
        n1283 = event-data() -> ()  [unwired: 7 out]
        n1284 = local write "Read setpoint correction\nfile"(FALSE) -> ()
        n1285 = Open/Create/Replace File(file path (use dialog)="Setpoint correction\noffset file", operation (0:open)=T29."open", access (0:read/write)=enum16{"read/write", "read-only", "write-only"}."read-only") -> (refnum out=w1991:refnum<file>)  [unwired: 1 in, 4 out]
        n1286 = Deny Access(7:w1991) -> (3:w1989:refnum<file>)  [unwired: 1 in, 2 out]
        n1287 = Read from Binary File(5:0.0, 9:T30."big-endian, network order" ("byte order (0:big-endian, network order)"), 10:-1 ("count (1)"), 11:w1989) -> (2:w1982:dbl[], 3:w1988:refnum<file>)  [unwired: 1 in, 3 out]
        n1288 = Close File(refnum=w1988) -> ()  [unwired: 1 in, 2 out]
        n1289 = Index Array(array=w1982, index=0) -> (element=w1978:dbl)
        n1290 = local write "Offset file step size"(w1978) -> ()
        n1291 = Array Subset(array=w1982, index=3) -> (w1981:dbl[])  [unwired: 1 in]
        n1292 = local read "T1 kappa_x (pN/nm)"() -> (w1976:dbl)
        n1293 = local read "T1 alpha_x (nm/V)"() -> (w1977:dbl)
        n1294 = local read "T2 alpha_x (nm/V)"() -> (w1975:dbl)
        n1295 = local read "T2 kappa_x (pN/nm)"() -> (w1974:dbl)
        n1296 = Decimate 1D Array(w1981) -> (w1970:dbl[], w1971:dbl[])  [unwired: 1 out]
        n1297 = local read "Offset Values"() -> (w1980:T14)
        n1298 = Multiply(x=w1977, y=w1976) -> (x*y=w1972:dbl)
        n1299 = Multiply(x=w1975, y=w1974) -> (x*y=w1973:dbl)
        n1300 = Bundle By Name(cluster=w1980, "Trap 1X offset"=w1970, "Trap 2X offset"=w1971) -> (w1979:T14)
        n1301 = Divide(x=w1973, y=w1972) -> (x/y=w1967:dbl)
        n1302 = disable-structure "Removed B Factor to better position FB - Alex 081418 3of3" shown="Enabled" {
          disable-tunnel: w1967 -> [w1995 _]
          disable-tunnel: [w1995 1.0] -> w1966
          frame Disabled {
          }
          frame Enabled {
          }
        }
        n1303 = Multiply(x=w1971, y=w1966) -> (x*y=w1969:dbl[])
        n1304 = local write "Offset Values"(w1979) -> ()
        n1305 = Subtract(x=w1970, y=w1969) -> (x-y=w1968:dbl[])
        n1306 = property on="B factor" class="DigNum (strict)"("Val(Sgnl)"=w1966) -> ()  [unwired: 2 in, 2 out]
        n1307 = property on="Setpoint offset\nCorrection values" class="Arr (strict)"("Val(Sgnl)"=w1968) -> ()  [unwired: 2 in, 2 out]
      }
      event "MCL Tracking": Value Change {
        n1308 = event-data() -> ()  [unwired: 7 out]
        n1309 = case shown="True" "MCL Tracking" {
          frame False {
            n1310 = local read "Current MCL (V)"() -> (w1998:dbl)
            n1311 = local write "MCL X"(w1998) -> ()
          }
          frame True {
            n1312 = local read "BD 1 Frq 1 (MHz)"() -> (→"Zero T1 position":dbl)
            n1313 = local read "MCL X"() -> (→"Zero MCL x position":dbl)
          }
        }
      }
      event "Scale intensities": Value Change {
        n1314 = event-data() -> ()  [unwired: 7 out]
        n1315 = local read "Trap Intensity\nSetpoints (V)"() -> (w2004:cluster{"Set 1":dbl, "Set 2":dbl})
        n1316 = local read "T1 kappa_x (pN/nm)"() -> (w2010:dbl)
        n1317 = local read "T2 kappa_x (pN/nm)"() -> (w2009:dbl)
        n1318 = Unbundle By Name(w2004) -> ("Set 1"=w2006:dbl, "Set 2"=w2005:dbl)
        n1319 = case shown="False" "Scale intensities" {
          tunnel: "Scale factor" -> [w2013 w2022]
          tunnel: w2010 -> [w2021 w2030]
          tunnel: w2009 -> [w2020 w2029]
          tunnel: [w2018 w2028] -> w2008
          tunnel: [w2019 w2027] -> w2007
          tunnel: w2006 -> [w2017 w2026]
          tunnel: w2005 -> [w2016 w2025]
          tunnel: [w2015 w2024] -> w2003
          tunnel: [w2014 w2023] -> w2002
          frame False {
            n1320 = Divide(x=w2017, y=w2013) -> (x/y=w2015:dbl)
            n1321 = Divide(x=w2016, y=w2013) -> (x/y=w2014:dbl)
            n1322 = Divide(x=w2021, y=w2013) -> (x/y=w2018:dbl)
            n1323 = Divide(x=w2020, y=w2013) -> (x/y=w2019:dbl)
          }
          frame True {
            n1324 = Multiply(x=w2026, y=w2022) -> (x*y=w2024:dbl)
            n1325 = Multiply(x=w2025, y=w2022) -> (x*y=w2023:dbl)
            n1326 = Multiply(x=w2030, y=w2022) -> (x*y=w2028:dbl)
            n1327 = Multiply(x=w2022, y=w2029) -> (x*y=w2027:dbl)
          }
        }
        n1328 = Bundle By Name(cluster=w2004, "Set 1"=w2003, "Set 2"=w2002) -> (w2001:cluster{"Set 1":dbl, "Set 2":dbl})
        n1329 = local write "T1 kappa_x (pN/nm)"(w2008) -> ()
        n1330 = local write "T2 kappa_x (pN/nm)"(w2007) -> ()
        n1331 = property on="Trap Intensity\nSetpoints (V)" class="Clust (strict)"("Val(Sgnl)"=w2001) -> ()  [unwired: 2 in, 2 out]
      }
    }
    "Error Events" <- w975
    n1332 = node-c288() -> ()  [unwired: 1 in, 1 out]
  }
  n1333 = timed-loop "Acquire Data" {
    tunnel: w49 -> [w2213]
    tunnel: w59 -> [w2212]
    tunnel: [w2235] -> w52
    tunnel: [w2229] -> w11
    timing: w170 -> [_]
    timing-out: [_] -> w169
    tunnel: w74 -> [w2149]
    stop <- "Stop All" stop-if-true
    # "Need to add a XY chart buffer"
    # "[Semi-passive would go here?]"
    # "Read values from FPGA"
    # "Check if we're done scanning"
    n1334 = node-c288() -> ()  [unwired: 2 out]
    n1335 = First Call?() -> (First Call?: T/F=w2133:bool)
    n1336 = Or(x="Reset", y=w2133) -> (x .or. y?=w2134:bool)
    n1337 = case "Reset FIFOs if asked" shown="True" w2134 {
      tunnel: w2213 -> [w2353 w2361]
      tunnel: w2212 -> [w2352 w2360]
      tunnel: [w2353 w2355] -> w2118
      tunnel: [w2352 w2354] -> w2208
      frame False {
      }
      frame True {
        w2358 = TRUE ("AI to FIFO")
        n1338 = call "reset FPGA DMA.vi"("error in"=w2360, "FPGA VI Reference In"=w2361) -> ("error out"=w2356:errorcluster, "FPGA VI Reference Out"=w2357:T20)
        n1339 = local write "Overflow (data lost)"(FALSE ("Overflow (data lost)")) -> ()
        n1340 = xnode "Read/Write Control"("FPGA VI Reference In"=w2357, "error in"=w2356, "AI to FIFO"=w2358, "APD to FIFO"=w2358) -> ("FPGA VI Reference Out"=w2355:T20, "error out"=w2354:errorcluster)
      }
    }
    n1341 = Or(x="Start AOD Scan", y="Trap Raster Scan") -> (x .or. y?=w2180:bool)
    n1342 = And(x="Save scans", y=w2180) -> (x .and. y?=w2206:bool)
    n1343 = case "Start AOM raster scan" shown="True" w2180 {
      tunnel: w2118 -> [w2496 w2507]
      tunnel: w2208 -> [w2495 w2506]
      tunnel: [w2496 w2500] -> w2117
      tunnel: [w2495 w2499] -> w2207
      frame False {
      }
      frame True {
        n1344 = case shown="True" "Restart DMA? (AOD)" {
          tunnel: [w2547 w2549] -> w2501
          tunnel: [w2546 w2548] -> w2502
          tunnel: w2507 -> [w2547 w2551]
          tunnel: w2506 -> [w2546 w2550]
          frame False {
          }
          frame True {
            n1345 = call "reset FPGA DMA.vi"("error in"=w2550, "FPGA VI Reference In"=w2551) -> ("error out"=w2548:errorcluster, "FPGA VI Reference Out"=w2549:T20)
            n1346 = local write "Overflow (data lost)"(FALSE ("Overflow (data lost)")) -> ()
          }
        }
        n1347 = local write "Trap Raster Scan"(FALSE ("Trap Raster Scan")) -> ()
        n1348 = case shown="True" "Move MCL Also?" {
          tunnel: w2502 -> [w2511 w2541]
          tunnel: w2501 -> [w2512 w2542]
          tunnel: [w2510 w2545] -> w2500
          tunnel: [w2509 w2544] -> w2499
          tunnel: "Raster to target force?" -> [w2508 w2514]
          frame False {
            w2513 = TRUE ("AI to FIFO")
            n1349 = xnode "Read/Write Control"("FPGA VI Reference In"=w2512, "error in"=w2511, "AI to FIFO"=w2513, "APD to FIFO"=w2513, "Start scan"=w2513, "Raster to target force"=w2508) -> ("FPGA VI Reference Out"=w2510:T20, "error out"=w2509:errorcluster)
          }
          frame True {
            w2538 = FALSE ("1D or 2D Scan?")
            w2543 = TRUE ("AI to FIFO")
            # "Count for MCL loop"
            # "N total cycles"
            # "N steps"
            # "V_int"
            n1350 = local read "Scan Range (nm)"() -> (w2520:dbl)
            n1351 = local read "Number of F/B Scans (AOD)"() -> (w2537:u16)
            n1352 = Sign(1:w2520) -> (0:w2519:dbl)
            n1353 = Compound Arithmetic op=MULTIPLY(w2520, "MCL Step Position Ratio", "MCL/AOM Scale Tweak") -> (w2524:dbl)
            n1354 = Negate(x=w2519) -> (-x=w2516:dbl)
            n1355 = Multiply(x=w2516, y="MCL Step Increment (V_int)") -> (x*y=w2518:dbl)
            n1356 = Divide(x=w2524, y="MCL X Cal (nm/V)") -> (x/y=w2530:dbl)
            n1357 = Multiply(x=32767.0 ("y"), y=w2530) -> (x*y=w2536:dbl)
            n1358 = local read "Total Counts (ticks)"() -> (w2521:u32)
            n1359 = local read "Cycles/step (AOD)"() -> (w2532:u64)
            n1360 = local read "Scan steps (AOD)"() -> (w2533:u64)
            n1361 = Divide(x=w2536, y=10.0) -> (x/y=w2529:dbl)
            n1362 = Divide(x=w2529, y="MCL Step Increment (V_int)") -> (x/y=w2527:dbl)
            n1363 = Absolute Value(x=w2527) -> (abs(x)=w2515:dbl)
            n1364 = Compound Arithmetic op=MULTIPLY(w2533, w2532, w2521) -> (w2528:u64)
            n1365 = local write "wait to reset values"(w2543) -> ()
            n1366 = local write "MCL Scanning"(w2543) -> ()
            n1367 = Divide(x=w2528, y=w2515) -> (x/y=w2525:dbl)
            "MCL Count" <- w2525
            n1368 = xnode "Read/Write Control"("FPGA VI Reference In"=w2542, "error in"=w2541, "Scan steps (MCL)"=w2515, "Number of scans (MCL)"=w2537, "Cycles per step (MCL)"=u64 1, "Scan freq.  increment (MCL)"=w2518, "1D or 2D Scan?"=w2538, "MCL Scan Axis"=w2538, "Cont. Scan (MCL)"=w2538, "MCL count"=w2525) -> ("FPGA VI Reference Out"=w2540:T20, "error out"=w2539:errorcluster)
            n1369 = xnode "Read/Write Control"("FPGA VI Reference In"=w2540, "error in"=w2539, "AI to FIFO"=w2543, "APD to FIFO"=w2543, "Start scan"=w2543, "Start scan (MCL)"=w2543, "Raster to target force"=w2514) -> ("FPGA VI Reference Out"=w2545:T20, "error out"=w2544:errorcluster)
          }
        }
        "Raster Scanning..." <- TRUE ("Scanning...")
      }
    }
    n1370 = Compound Arithmetic op=OR("Start MCL Scan", "Confocal Image", "Confocal Linescan") -> (w2178:bool)
    n1371 = And(x="Save Data (MCL)", y=w2178) -> (x .and. y?=w2205:bool)
    n1372 = case "Start MCL raster scan" shown="True" w2178 {
      tunnel: w2117 -> [w2416 w2430]
      tunnel: w2207 -> [w2415 w2429]
      tunnel: [w2416 w2425] -> w2099
      tunnel: [w2415 w2424] -> w2101
      tunnel: [FALSE w2423] -> w2192
      tunnel: "Start MCL Scan" -> [_ w2418]
      tunnel: "Confocal Image" -> [_ w2417]
      frame False {
      }
      frame True {
        w2423 = TRUE
        n1373 = case shown="True" "Restart DMA? (MCL)" {
          tunnel: [w2474 w2476] -> w2428
          tunnel: [w2473 w2475] -> w2427
          tunnel: w2430 -> [w2474 w2479]
          tunnel: w2429 -> [w2473 w2478]
          frame False {
          }
          frame True {
            n1374 = call "reset FPGA DMA.vi"("error in"=w2478, "FPGA VI Reference In"=w2479) -> ("error out"=w2475:errorcluster, "FPGA VI Reference Out"=w2476:T20)
            n1375 = local write "Overflow (data lost)"(FALSE ("Overflow (data lost)")) -> ()
          }
        }
        n1376 = case shown="False" w2418 {
          tunnel: w2417 -> [w2433 _]
          frame False {
            n1377 = property on="Confocal Image" class="Bool (strict)"("Value"=FALSE ("Start Confocal Map")) -> ()  [unwired: 2 in, 2 out]
            n1378 = property on="2D or 1D Scan" class="Bool (strict)"("Val(Sgnl)"=w2433) -> ()  [unwired: 2 in, 2 out]
          }
          frame True {
          }
        }
        n1379 = local write "MCL Scanning"(w2423) -> ()
        n1380 = local read "MCL X"() -> (w2419:dbl)
        n1381 = local read "MCL Y"() -> (w2420:dbl)
        n1382 = case shown="True" "Center Scan" {
          tunnel: w2428 -> [w2440 w2472]
          tunnel: w2427 -> [w2439 w2471]
          tunnel: [w2438 w2470] -> w2425
          tunnel: [w2437 w2469] -> w2424
          tunnel: [w2435 w2444] -> w2422
          tunnel: [w2434 w2441] -> w2421
          tunnel: w2420 -> [w2435 w2461]
          tunnel: w2419 -> [w2434 w2464]
          frame False {
            w2436 = TRUE ("AI to FIFO")
            n1383 = xnode "Read/Write Control"("FPGA VI Reference In"=w2440, "error in"=w2439, "AI to FIFO"=w2436, "APD to FIFO"=w2436, "Start scan (MCL)"=w2436) -> ("FPGA VI Reference Out"=w2438:T20, "error out"=w2437:errorcluster)
          }
          frame True {
            w2468 = TRUE ("AI to FIFO")
            n1384 = local read "Scan steps (x)"() -> (w2451:u64)
            n1385 = local read "Fast Scan Dir"() -> (w2458:bool)
            n1386 = local read "Scan lines (y)"() -> (w2447:u64)
            n1387 = local read "Actual MCL Inc (V)"() -> (w2448:dbl)
            n1388 = Decrement(x=w2447) -> (x-1=w2446:u64)
            n1389 = Decrement(x=w2451) -> (x-1=w2450:u64)
            n1390 = Multiply(x=w2448, y=w2446) -> (x*y=w2445:dbl)
            n1391 = Divide(x=w2445, y=2.0) -> (x/y=w2455:dbl)
            n1392 = local read "2D or 1D Scan"() -> (w2466:bool)
            n1393 = Multiply(x=w2448, y=w2450) -> (x*y=w2449:dbl)
            n1394 = Divide(x=w2449, y=2.0) -> (x/y=w2454:dbl)
            n1395 = Select(t=w2454, s=w2458, f=w2455) -> (s? t:f=w2453:dbl)
            n1396 = Select(t=w2455, s=w2458, f=w2454) -> (s? t:f=w2457:dbl)
            n1397 = Subtract(x=w2461, y=w2457) -> (x-y=w2456:dbl)
            n1398 = Subtract(x=w2464, y=w2453) -> (x-y=w2452:dbl)
            n1399 = Not(x=w2458) -> (.not. x?=w2460:bool)
            n1400 = Not(x=w2466) -> (.not. x?=w2462:bool)
            n1401 = And(x=w2458, y=w2462) -> (x .and. y?=w2463:bool)
            n1402 = And(x=w2462, y=w2460) -> (x .and. y?=w2465:bool)
            n1403 = Select(t=w2464, s=w2465, f=w2452) -> (s? t:f=w2441:dbl)
            n1404 = Select(t=w2461, s=w2463, f=w2456) -> (s? t:f=w2444:dbl)
            n1405 = call "V2int16.vi"("InV"=w2441) -> ("Out i16"=w2442:i16)  [unwired: 4 in]
            n1406 = call "V2int16.vi"("InV"=w2444) -> ("Out i16"=w2443:i16)  [unwired: 4 in]
            n1407 = xnode "Read/Write Control"("FPGA VI Reference In"=w2472, "error in"=w2471, "AI to FIFO"=w2468, "APD to FIFO"=w2468, "Start scan (MCL)"=w2468, "AO1 (Y)"=w2443, "AO2 (X)"=w2442) -> ("FPGA VI Reference Out"=w2470:T20, "error out"=w2469:errorcluster)
          }
        }
        "Initial Y" <- w2422
        "Initial X" <- w2421
        "wait to reset values" <- w2423
      }
    }
    n1408 = local read "Trap Pos Elements/DMA read"() -> (w2105:u32)
    n1409 = local read "Trap AI Elements/DMA read"() -> (w2107:u32)
    n1410 = local read "APD Elements/DMA read"() -> (w2106:u32)
    n1411 = call "ReadFIFOs.vi"("FPGA In"=w2099, "Error In"=w2101, "Trap N Read"=w2107, "APD N Read"=w2106, "TPos N Read"=w2105) -> ("FPGA Out"=w2098:T20, "Error Out"=w2097:errorcluster, "Trap Data"=w2092:i16[], "APD Data"=w2095:u32[], "TPos Data"=w2100:u64[], "Trap N Left"=w2102:u32, "APD N Left"=→"APD FIFO Elements Remaining":u32, "TPos N Left"=→"Trap Pos FIFO El Remaining":u32)  [unwired: 7 in]
    "Trap AI FIFO El. Rem." <- w2102
    n1412 = local read "Trap AI FIFO Depth"() -> (w2244:u32)
    n1413 = xnode "Read/Write Control"("FPGA VI Reference In"=w2098, "error in"=w2097) -> ("FPGA VI Reference Out"=w2114:T20, "error out"=w2096:errorcluster, "BD1 Frequency Out 1"=w2090:u64)
    n1414 = flat-sequence "Save data" {
      tunnel: [w2676] -> w2246
      tunnel: [w2677] -> w2245
      tunnel: w2206 -> [w2672]
      tunnel: w2059 -> [w2675]
      tunnel: w2094 -> [w2651]
      tunnel: [w2670] -> w2217
      tunnel: [w2667] -> w2216
      tunnel: [w2664] -> w2215
      tunnel: w2205 -> [w2666]
      tunnel: [w2656] -> w2132
      tunnel: [w2655] -> w2131
      tunnel: w2054 -> [w2649]
      tunnel: w2246 -> [w2826]
      tunnel: w2245 -> [w2825]
      tunnel: w2088 -> [w2824]
      tunnel: w2217 -> [w2822]
      tunnel: w2216 -> [w2821]
      tunnel: w2215 -> [w2820]
      tunnel: w2132 -> [w2819]
      tunnel: w2131 -> [w2818]
      tunnel: w2100 -> [w2817]
      tunnel: w2095 -> [w2816]
      tunnel: w2054 -> [w2815]
      frame #0 {
        # "Channel Pattern, N Channels, dT"
        n1415 = Or(x="Save N Sets", y="Start Saving") -> (x .or. y?=w2661:bool)
        n1416 = Build Array(w2661, "Save Calibration", w2672, w2666) -> (w2674:bool[])
        n1417 = Boolean Array To Number(Boolean array=w2674) -> (number=w2653:u32)
        n1418 = Not Equal To 0?(x=w2653) -> (x != 0?=w2652:bool)
        n1419 = feedback #1(refnum<k0> refnum) -> (w2678:refnum<file>)
        n1420 = feedback #2(0) -> (w2680:i32)
        n1421 = feedback #3(u32 0 ("Cal sets to save")) -> (w2671:u32)
        n1422 = feedback #4(refnum<k0> refnum) -> (w2668:refnum<file>)
        n1423 = feedback #5(FALSE ("Save APD Data\nwith Trap Data")) -> (w2665:bool)
        n1424 = feedback #6(refnum<k0> refnum) -> (w2659:refnum<file>)
        n1425 = feedback #7(FALSE ("Save APD Data\nwith Trap Data")) -> (w2657:bool)
        n1426 = case shown="True" w2652 {
          tunnel: [w2688 1] -> w2676
          tunnel: w2680 -> [w2689 _]
          tunnel: [w2682 w2704] -> w2677
          tunnel: w2678 -> [w2682 _]
          tunnel: w2675 -> [_ w2698]
          tunnel: w2653 -> [_ w2700]
          tunnel: [w2687 w2715] -> w2670
          tunnel: w2671 -> [w2687 _]
          tunnel: [w2686 w2714] -> w2667
          tunnel: w2668 -> [w2686 _]
          tunnel: [w2685 w2713] -> w2664
          tunnel: w2665 -> [w2685 _]
          tunnel: [w2684 w2709] -> w2655
          tunnel: w2659 -> [w2684 _]
          tunnel: [w2683 w2708] -> w2656
          tunnel: w2657 -> [w2683 _]
          tunnel: "Start Saving" -> [_ w2707]
          tunnel: w2651 -> [_ w2694]
          tunnel: w2649 -> [_ w2692]
          frame False {
            n1427 = Increment(x=w2689) -> (x+1=w2688:i32)
          }
          frame True {
            w2712 = FALSE ("Start Saving")
            w2699 = 9.0  # File Ver.
            n1428 = To Double Precision Float(number=w2694) -> (double precision float=w2693:dbl)
            n1429 = To Double Precision Float(number=w2692) -> (double precision float=w2691:dbl)
            n1430 = case "File Info Header" shown="Default" w2700 {
              tunnel: w2699 -> [w2728 w2735]
              tunnel: w2698 -> [w2727 w2730]
              tunnel: w2691 -> [w2726 w2734]
              tunnel: w2693 -> [w2725 w2733]
              tunnel: [w2724 w2732] -> w2697
              frame 2 {
                n1431 = Build Array(w2728, w2727, w2727, w2726, w2725) -> (w2724:dbl[])
              }
              frame Default {
                n1432 = local read "Save ave N"() -> (w2731:i32)
                n1433 = Multiply(x=w2730, y=w2731) -> (x*y=w2729:dbl)
                n1434 = Build Array(w2735, w2730, w2729, w2734, w2733) -> (w2732:dbl[])
              }
            }
            n1435 = case "Scan Info Header" shown="8" w2700 {
              tunnel: [w2753 "Cal sets to save" w2772 w2803] -> w2715
              tunnel: "Save APD" -> [w2747 _ w2767 w2790]
              tunnel: [w2747 w2759 w2767 w2790] -> w2713
              tunnel: [w2746 w2759 w2766 w2789] -> w2708
              tunnel: "Save TPos" -> [w2746 _ w2766 w2789]
              tunnel: w2707 -> [w2750 _ _ _]
              tunnel: [0.0 ("f") 1.0 ("t") 2.0 ("t") 3.0 ("t")] -> w2696
              tunnel: [w2744 w2756 w2762 w2785] -> w2690
              frame 1, Default {
                w2751 = 0.0 ("f")
                # "Regular Data"
                n1436 = Build Array(w2747, w2746) -> (w2748:bool[])
                n1437 = Boolean Array To Number(Boolean array=w2748) -> (number=w2745:u32)
                n1438 = To Double Precision Float(number=w2745) -> (double precision float=w2755:dbl)
                n1439 = Select(t=u32 4000000000, s=w2750, f="N sets to save") -> (s? t:f=w2753:u32)
                n1440 = Build Array(w2755, w2751, w2751, w2751, w2751) -> (w2744:dbl[])
              }
              frame 2 {
                w2757 = 0.0 ("f")
                w2759 = FALSE ("Save APD Data\nwith Trap Data")
                # "Calibration"
                n1441 = Build Array(w2757, w2757, w2757, w2757, w2757) -> (w2756:dbl[])
                "Calibrating Trap..." <- TRUE ("Calibrating...")
              }
              frame 4 {
                w2770 = 0.0 ("f")
                # "Trap Raster"
                n1442 = local read "Number of F/B Scans (AOD)"() -> (w2776:u16)
                n1443 = Build Array(w2767, w2766) -> (w2765:bool[])
                n1444 = local read "Scan Range (MHz)"() -> (w2781:dbl)
                n1445 = local read "Cycles/step (AOD)"() -> (w2778:u64)
                n1446 = local read "Scan steps (AOD)"() -> (w2780:u64)
                n1447 = Boolean Array To Number(Boolean array=w2765) -> (number=w2768:u32)
                n1448 = To Double Precision Float(number=w2768) -> (double precision float=w2771:dbl)
                n1449 = local read "Scan BD"() -> (w2784:bool)
                n1450 = local read "N sets should be saved"() -> (w2773:dbl)
                n1451 = Build Array(w2771, w2770, w2770, w2770, w2770) -> (w2764:dbl[])
                n1452 = Boolean To (0,1)(Boolean=w2784) -> (0, 1=w2783:i16)
                n1453 = To Double Precision Float(number=w2780) -> (double precision float=w2779:dbl)
                n1454 = To Double Precision Float(number=w2778) -> (double precision float=w2777:dbl)
                n1455 = To Double Precision Float(number=w2776) -> (double precision float=w2775:dbl)
                n1456 = To Double Precision Float(number=w2783) -> (double precision float=w2782:dbl)
                n1457 = Build Array(w2782, w2781, w2779, w2777, w2775) -> (w2763:dbl[])
                n1458 = Round Toward +Infinity(x=w2773) -> (ceil(x): smallest int >= x=w2774:dbl)
                n1459 = Build Array (concatenate)(w2764, w2763) -> (w2762:dbl[])
                n1460 = To Unsigned Long Integer(number=w2774) -> (unsigned 32bit integer=w2772:u32)
              }
              frame 8 {
                w2799 = 0.0 ("f")
                # "MCL raster scan"
                n1461 = local read "2D or 1D Scan"() -> (w2796:bool)
                n1462 = local read "N sets should be saved (MCL)"() -> (w2804:dbl)
                n1463 = Build Array(w2790, w2789) -> (w2791:bool[])
                n1464 = Boolean Array To Number(Boolean array=w2791) -> (number=w2788:u32)
                n1465 = To Double Precision Float(number=w2788) -> (double precision float=w2802:dbl)
                n1466 = local read "Scan Range (V)\n(of steps)"() -> (w2811:dbl)
                n1467 = local read "Number of scans (MCL)"() -> (w2794:u64)
                n1468 = Boolean To (0,1)(Boolean=w2796) -> (0, 1=w2798:i16)
                n1469 = To Double Precision Float(number=w2798) -> (double precision float=w2797:dbl)
                n1470 = local read "Cycles/step (MCL)"() -> (w2808:u64)
                n1471 = Build Array(w2802, w2797, w2799, w2799, w2799) -> (w2787:dbl[])
                n1472 = local read "Scan steps (x)"() -> (w2810:u64)
                n1473 = local read "Scan lines (y)"() -> (w2793:u64)
                n1474 = local read "Fast Scan Dir"() -> (w2814:bool)
                n1475 = local read "Initial X"() -> (w2801:dbl)
                n1476 = local read "Initial Y"() -> (w2800:dbl)
                n1477 = Round Toward +Infinity(x=w2804) -> (ceil(x): smallest int >= x=w2805:dbl)
                n1478 = To Unsigned Long Integer(number=w2805) -> (unsigned 32bit integer=w2803:u32)
                n1479 = To Double Precision Float(number=w2810) -> (double precision float=w2809:dbl)
                n1480 = To Double Precision Float(number=w2808) -> (double precision float=w2807:dbl)
                n1481 = Select(t=w2793, s=w2796, f=w2794) -> (s? t:f=w2795:u64)
                n1482 = Boolean To (0,1)(Boolean=w2814) -> (0, 1=w2813:i16)
                n1483 = To Double Precision Float(number=w2813) -> (double precision float=w2812:dbl)
                n1484 = To Double Precision Float(number=w2795) -> (double precision float=w2806:dbl)
                n1485 = Build Array(w2812, w2811, w2809, w2807, w2806, w2801, w2800) -> (w2786:dbl[])
                n1486 = Build Array (concatenate)(w2787, w2786) -> (w2785:dbl[])
              }
            }
            n1487 = local read "BD 1 Frq 1 (MHz)"() -> (w2721:dbl)
            n1488 = local read "BD 2 Frq 1 (MHz)"() -> (w2720:dbl)
            n1489 = local read "BD 1 Frq 2 (MHz)"() -> (w2719:dbl)
            n1490 = local read "BD 2 Frq 2 (MHz)"() -> (w2718:dbl)
            n1491 = local read "BD 1 Frq 3 (MHz)"() -> (w2717:dbl)
            n1492 = local read "BD 2 Frq 3 (MHz)"() -> (w2716:dbl)
            n1493 = Build Array(w2721, w2720, w2719, w2718, w2717, w2716) -> (w2701:dbl[])
            n1494 = local write "Saving..."(TRUE ("Saving...")) -> ()
            n1495 = local write "Save Calibration"(w2712) -> ()
            n1496 = local write "Start Saving"(w2712) -> ()
            n1497 = Build Array (concatenate)(w2697, w2696) -> (w2695:dbl[])
            n1498 = local read "Index"() -> (w2706:dbl)
            n1499 = call "HeaderTrap.vi"("Index In"=w2706, "File Info"=w2695, "BD Frqs"=w2701, "Scan Data"=w2690, "Comment"="Comment") -> ("Index Out"=w2705:dbl, "Trap Path"=w2703:path, "Trap File Out"=w2704:refnum<file>)  [unwired: 12 in]
            n1500 = local write "Index"(w2705) -> ()
            n1501 = local write "Save index"(w2705) -> ()
            n1502 = local write "Save file name"(w2703) -> ()
            n1503 = case "Fluorescence Header" shown="True" w2713 {
              tunnel: w2703 -> [_ w2741]
              tunnel: [refnum<k0> refnum w2740] -> w2714
              frame False {
              }
              frame True {
                n1504 = local read "APD Integration Time (s)"() -> (w2743:dbl)
                n1505 = local read "N APD Samp/step"() -> (w2742:i32)
                n1506 = call "HeaderFluorescence.vi"("N APD Samp/step"=w2742, "APD Integration Time (s)"=w2743, "Trap Path"=w2741) -> ("Flu File"=w2740:refnum<file>)  [unwired: 8 in]
              }
            }
            n1507 = case "TPos Header" shown="True" w2708 {
              tunnel: w2703 -> [_ w2738]
              tunnel: [refnum<k0> refnum w2737] -> w2709
              frame False {
              }
              frame True {
                n1508 = call "HeaderTPos.vi"("Trap Path"=w2738) -> ("TPos File"=w2737:refnum<file>)  [unwired: 10 in]
              }
            }
          }
        }
        n1509 = feedback-in #1(w2677) -> ()
        n1510 = feedback-in #2(w2676) -> ()
        n1511 = feedback-in #3(w2670) -> ()
        n1512 = feedback-in #4(w2667) -> ()
        n1513 = feedback-in #5(w2664) -> ()
        n1514 = feedback-in #6(w2655) -> ()
        n1515 = feedback-in #7(w2656) -> ()
      }
      frame #1 {
        # "N Channels"
        # "TPos, APD, Trap Data"
        n1516 = local read "Saving..."() -> (w2823:bool)
        n1517 = case shown="True" w2823 {
          tunnel: w2826 -> [_ w2830]
          tunnel: w2825 -> [_ w2849]
          tunnel: w2824 -> [_ w2845]
          tunnel: w2822 -> [_ w2829]
          tunnel: w2821 -> [_ w2841]
          tunnel: w2820 -> [_ w2840]
          tunnel: w2819 -> [_ w2838]
          tunnel: w2818 -> [_ w2837]
          tunnel: w2817 -> [_ w2836]
          tunnel: w2816 -> [_ w2835]
          tunnel: w2815 -> [_ w2834]
          frame False {
          }
          frame True {
            n1518 = local read "DMA Update Period (s)"() -> (w2833:dbl)
            n1519 = Divide(x=w2830, y=w2829) -> (x/y=w2832:dbl)
            n1520 = Multiply(x=w2830, y=w2833) -> (x*y=→"Time (s)":dbl)
            n1521 = Less Or Equal?(x=w2830, y=w2829) -> (x <= y?=w2847:bool)
            n1522 = Multiply(x=w2832, y=100.0) -> (x*y=w2828:dbl)
            n1523 = Or(x="Stop Saving", y="Abort save 2") -> (x .or. y?=w2842:bool)
            n1524 = Not(x=w2842) -> (.not. x?=w2848:bool)
            n1525 = And(x=w2847, y=w2848) -> (x .and. y?=w2846:bool)
            n1526 = case shown="True" w2846 {
              tunnel: w2849 -> [w2856 w2877]
              tunnel: w2845 -> [_ w2874]
              tunnel: w2841 -> [w2855 w2870]
              tunnel: w2840 -> [w2854 w2871]
              tunnel: w2838 -> [w2852 w2869]
              tunnel: w2837 -> [w2853 w2868]
              tunnel: w2836 -> [_ w2866]
              tunnel: w2835 -> [_ w2864]
              tunnel: w2834 -> [_ w2863]
              tunnel: w2828 -> [_ w2859]
              tunnel: [0.0 w2859] -> w2827
              frame False {
                w2851 = FALSE
                n1527 = case shown="True" w2854 {
                  tunnel: w2855 -> [_ w2858]
                  frame False {
                  }
                  frame True {
                    n1528 = Close File(refnum=w2858) -> ()  [unwired: 1 in, 2 out]
                  }
                }
                n1529 = case shown="False" w2852 {
                  tunnel: w2853 -> [_ w2857]
                  frame False {
                  }
                  frame True {
                    n1530 = Close File(refnum=w2857) -> ()  [unwired: 1 in, 2 out]
                  }
                }
                n1531 = Close File(refnum=w2856) -> ()  [unwired: 1 in, 2 out]
                n1532 = call <vilib>:"Beep.vi"() -> ()  [unwired: 3 in, 9 out]
                n1533 = property on="Raster Scanning..." class="Bool (strict)"("Val(Sgnl)"=w2851) -> ()  [unwired: 2 in, 2 out]
                n1534 = local write "Calibrating Trap..."(w2851) -> ()
                n1535 = local write "Stop Saving"(w2851) -> ()
                "Saving..." <- w2851
              }
              frame True {
                n1536 = local read "Calibrating Trap..."() -> (w2862:bool)
                n1537 = Equal?(x=1 ("y"), y="Save ave N") -> (x = y?=w2873:bool)
                n1538 = Or(x=w2862, y=w2873) -> (x .or. y?=w2867:bool)
                n1539 = case "Downsample TPos" shown="True" w2867 {
                  tunnel: w2866 -> [w2878 w2889]
                  tunnel: [w2878 w2881] -> w2865
                  tunnel: "Save ave N" -> [_ w2882]
                  frame False {
                  }
                  frame True {
                    w2879 = 2 ("dimension size")
                    n1540 = Array Size(array=w2889) -> (size(s)=w2883:i32)
                    n1541 = Divide(x=w2883, y=w2879) -> (x/y=w2887:dbl)
                    n1542 = Divide(x=w2883, y=w2882) -> (x/y=w2884:dbl)
                    n1543 = Reshape Array(w2889, w2887, w2879) -> (w2888:u64[][])
                    n1544 = Transpose 2D Array(2D array=w2888) -> (transposed array=w2886:u64[][])
                    n1545 = for {
                      tunnel: w2886 -> [w2891] mode=indexing
                      tunnel: [w2890] -> w2880 mode=indexing
                      tunnel: w2882 -> [w2892]
                      workers-P: _ -> [_]
                      n1546 = call "downsample 1D array - U64.vi"("Ave N"=w2892, "Array In"=w2891) -> ("Array Out"=w2890:u64[])  [unwired: 1 in]
                    }
                    n1547 = Transpose 2D Array(2D array=w2880) -> (transposed array=w2885:u64[][])
                    n1548 = Reshape Array(w2885, w2884) -> (w2881:u64[])
                  }
                }
                n1549 = case "Downsample Trap" shown="True" w2867 {
                  tunnel: w2874 -> [w2901 w2912]
                  tunnel: [w2901 w2904] -> w2872
                  tunnel: "Save ave N" -> [_ w2905]
                  tunnel: w2863 -> [_ w2902]
                  frame False {
                    # "Don't downsample"
                  }
                  frame True {
                    n1550 = Array Size(array=w2912) -> (size(s)=w2906:i32)
                    n1551 = Quotient & Remainder(x=w2906, y=w2902) -> (floor(x/y)=w2910:i32)  [unwired: 1 out]
                    n1552 = Quotient & Remainder(x=w2906, y=w2905) -> (floor(x/y)=w2907:i32)  [unwired: 1 out]
                    n1553 = Reshape Array(w2912, w2910, w2902) -> (w2911:i16[][])
                    n1554 = Transpose 2D Array(2D array=w2911) -> (transposed array=w2909:i16[][])
                    n1555 = for {
                      tunnel: w2909 -> [w2915] mode=indexing
                      tunnel: [w2914] -> w2903 mode=indexing
                      tunnel: w2905 -> [w2913]
                      workers-P: _ -> [_]
                      n1556 = call "downsample 1D array - I16.vi"("Ave N"=w2913, "Array In"=w2915) -> ("Array Out"=w2914:i16[])  [unwired: 1 out]
                    }
                    n1557 = Transpose 2D Array(2D array=w2903) -> (transposed array=w2908:i16[][])
                    n1558 = Reshape Array(w2908, w2907) -> (w2904:i16[])
                  }
                }
                n1559 = case "Write fluorescene" shown="True" w2871 {
                  tunnel: w2870 -> [_ w2898]
                  tunnel: w2864 -> [_ w2897]
                  frame False {
                  }
                  frame True {
                    n1560 = Write to Binary File(file (use dialog)=w2898, data=w2897, 5:FALSE ("prepend array or string size? (T)"), 9:T30."big-endian, network order" ("byte order (0:big-endian, network order)")) -> ()  [unwired: 1 in, 4 out]
                  }
                }
                n1561 = case "Save TPos Data" shown="True" w2869 {
                  tunnel: w2868 -> [_ w2894]
                  tunnel: w2865 -> [_ w2893]
                  frame False {
                  }
                  frame True {
                    n1562 = Write to Binary File(file (use dialog)=w2894, data=w2893, 5:FALSE ("prepend array or string size? (T)"), 9:T30."big-endian, network order" ("byte order (0:big-endian, network order)")) -> ()  [unwired: 1 in, 4 out]
                  }
                }
                n1563 = Write to Binary File "Save Trap Data"(file (use dialog)=w2877, data=w2872, 5:FALSE ("prepend array or string size? (T)"), 9:T30."big-endian, network order" ("byte order (0:big-endian, network order)")) -> ()  [unwired: 1 in, 4 out]
              }
            }
            "Progress" <- w2827
            "Progress 2" <- w2827
          }
        }
      }
    }
    n1564 = local read "BD 1 Frq 2 (MHz)"() -> (w2124:dbl)
    n1565 = local read "MCL Tracking"() -> (w2119:bool)
    n1566 = Subtract(x=w2244, y=w2107) -> (x-y=w2243:u32)
    n1567 = Divide(x=w2102, y=w2243) -> (x/y=w2242:dbl)
    "Buffer Status" <- w2242
    n1568 = call "AODuint642MHz.vi"("In u64"=w2090) -> ("Out MHz"=w2089:dbl)  [unwired: 4 in]
    n1569 = Equal?(x=w2242, y=1.0) -> (x = y?=w2240:bool)
    n1570 = Subtract ("TD")(x=w2124, y=w2089) -> (x-y=w2115:dbl)
    "Current Trap Delta" <- w2115
    n1571 = case shown="True" w2119 {
      tunnel: w2089 -> [_ w2330]
      tunnel: w2117 -> [_ w2320]
      frame False {
      }
      frame True {
        n1572 = local read "Zero T1 position"() -> (w2329:dbl)
        n1573 = local read "AOM X Cal (nm/MHz)"() -> (w2327:dbl)
        n1574 = local read "MCL X Cal (nm/V)"() -> (w2323:dbl)
        n1575 = Subtract(x=w2330, y=w2329) -> (x-y=w2328:dbl)
        n1576 = local read "Zero MCL x position"() -> (w2322:dbl)
        n1577 = Multiply(x=w2328, y=w2327) -> (x*y=w2326:dbl)
        n1578 = Multiply(x=w2326, y="Tracking factor") -> (x*y=w2324:dbl)
        n1579 = Divide(x=w2324, y=w2323) -> (x/y=w2321:dbl)
        n1580 = Add(x=w2322, y=w2321) -> (x+y=w2319:dbl)
        "Current MCL (V)" <- w2319
        n1581 = call "V2int16.vi"("InV"=w2319) -> ("Out i16"=w2318:i16)  [unwired: 4 in]
        n1582 = xnode "Read/Write Control"("FPGA VI Reference In"=w2320, "AO2 (X)"=w2318) -> ()  [unwired: 1 in, 2 out]
      }
    }
    n1583 = call "IR AOM word to freq - vec.vi"("Frequency Word In (double vec)"=w2100) -> ("Frequency Out"=w2147:dbl[])
    n1584 = case "Alert buffer overflow" shown="True" w2240 {
      frame False {
      }
      frame True {
        n1585 = call <vilib>:"Beep.vi"() -> ()  [unwired: 3 in, 9 out]
        "Overflow (data lost)" <- TRUE ("Overflow (data lost)")
      }
    }
    n1586 = Decimate 1D Array(w2147) -> (w2146:dbl[], w2145:dbl[])
    n1587 = Build Array(w2146, w2145) -> (w2072:dbl[][])
    n1588 = local read "Dynamic Force FB"() -> (w2123:bool)
    n1589 = local read "Trap Pos. FB ON"() -> (w2122:bool)
    n1590 = local read "Trap Sets"() -> (w2093:u32)
    n1591 = call "Trapu16toDbl.vi"("Detector Type"="Detector Type", "Trap Sets"=w2093, "Raw Trap Data In"=w2092) -> ("Channel pattern"=w2094:i32, "Channel Names"=w2055:string[], "Trap Data"=w2082:dbl[][], "Trap Data Out"=w2088:i16[])  [unwired: 5 in]
    "AI labels" <- w2055
    n1592 = Compound Arithmetic op=AND(w2123, w2122, "Use Offset in FFB?") -> (w2120:bool)
    n1593 = local read "Trap X AI1 (DMA)"() -> (w2141:T13)
    n1594 = case "Apply Offset to Force Feedback" shown="True" w2120 {
      tunnel: w2115 -> [_ w2333]
      tunnel: w2114 -> [_ w2332]
      frame False {
      }
      frame True {
        n1595 = local read "Setpoint offset\nCorrection values"() -> (w2348:dbl[])
        n1596 = local read "Offset file step size"() -> (w2351:dbl)
        n1597 = local read "Negate offset difference"() -> (w2343:bool)
        n1598 = local read "T1 kappa_x (pN/nm)"() -> (w2341:dbl)
        n1599 = local read "T1 alpha_x (nm/V)"() -> (w2342:dbl)
        n1600 = Divide(x=w2333, y=w2351) -> (x/y=w2350:dbl)
        n1601 = Multiply(x="Target Force (pN)", y=2.0) -> (x*y=w2339:dbl)
        n1602 = Multiply(x=w2342, y=w2341) -> (x*y=w2338:dbl)
        n1603 = To Long Integer(number=w2350) -> (32bit integer=w2349:i32)
        n1604 = Divide(x=w2339, y=w2338) -> (x/y=w2337:dbl)
        n1605 = Select(t=-1, s=w2343, f=1) -> (s? t:f=w2344:i32)
        n1606 = Index Array(array=w2348, index=w2349) -> (element=w2347:dbl)
        n1607 = Multiply(x=w2344, y=w2347) -> (x*y=w2336:dbl)
        n1608 = Add(x=w2337, y=w2336) -> (x+y=w2335:dbl)
        n1609 = To Fixed-Point(number=w2335) -> (fixed-point=w2331:fxp<+/-,16,1>)  [unwired: 1 in]
        "Actual setpoint" <- w2331
        n1610 = xnode "Read/Write Control"("FPGA VI Reference In"=w2332, "Trap Pos. FB SP"=w2331) -> ()  [unwired: 1 in, 2 out]
      }
    }
    n1611 = Array Size(array=w2055) -> (size(s)=w2054:i32)
    n1612 = call "Trapi162FXP.vi"("N El. to Ave."="N El. to Ave.", "Trap Data"=w2088) -> ("Trap 2"=w2085:fxp<+/-,16,1>, "Trap 1"=w2086:fxp<+/-,16,1>)  [unwired: 8 in]
    n1613 = Bundle By Name(cluster=w2141, "Set 1"=w2086, "Set 2"=w2085) -> (→"Trap X AI1 (DMA)":T13)
    n1614 = case shown="True" "Read Lateness and Rel Phase" {
      tunnel: w2114 -> [w2363 w2384]
      tunnel: [w2363 w2383] -> w2169
      tunnel: [w2362 w2382] -> w2168
      tunnel: w2096 -> [w2362 w2366]
      frame False {
      }
      frame True {
        n1615 = xnode "Read/Write Control"("FPGA VI Reference In"=w2384, "error in"=w2366) -> ("FPGA VI Reference Out"=w2383:T20, "error out"=w2382:errorcluster, "GI Relative phase"=→"GI relative phase":i16, "Relative phase"=→"Relative phase (AI1)":i16, "AI Late Counter"=→"Late Counter (AI1)":u8, "GI Late Counter"=→"GI Late Counter":u8, "MCL Late Counter"=→"MCL Late Counter":u8, "MCL Relative Phase"=→"Relative Phase (MCL)":i16, "APD Acq Relative Phase"=→"APD Acq Relative Phase":i16, "APD 1 Gate Relative Phase"=→"APD 1 Gate Relative Phase":i16, "APD 2 Gate Relative Phase"=→"APD 2 Gate Relative Phase":i16, "APD Acq Late Counter"=→"APD Acq Late Counter":u16, "APD 1 Gate Late Counter"=→"APD 1 Gate Late Counter":u8, "APD 2 Gate Late Counter"=→"APD 2 Gate Late Counter":u8, "Green FB Relative Phase"=→"Relative phase (Green FB)":i16, "GI Relative phase"=→"GI relative phase 2":i16, "GI Late Counter 2"=→"GI Late Counter 2":u16, "Trap Pos FIFO Timeout"=→"Trap Pos FIFO Timeout":u16, "Trap AI FIFO Timeout"=→"Trap AI FIFO Timeout":u16)
      }
    }
    n1616 = xnode ("Read/Write Control")("FPGA VI Reference In"=w2169, "error in"=w2168) -> ("FPGA VI Reference Out"=w2236:T20, "error out"=w2230:errorcluster, "AI2 Y Sum Set 1"=w2226:i16, "AI2 Y Sum Set 2"=w2225:i16, "AI1 X Set 1"=w2139:fxp<+/-,16,1>, "AI1 X Set 2"=w2138:fxp<+/-,16,1>, "Trap Pos FB Int Signal"=→"Trap Pos FB Int Signal":fxp<+/-,24,9>, "Trap Pos FB Int-Norm Signal"=→"Trap Pos FB Int-Norm Signal":fxp<+/-,16,1>, "Trap Pos FB Action"=w2136:i64, "Scanning"=→"AOD Scanning":bool, "Scan I"=→"AOD Scan I":u64, "Scanning MCL"=w2228:bool, "Scan I (MCL)"=→"MCL Scan I":u64, "Green FB Signals"=w2187:T36, "BD1 amplitude 1 out"=w2032:u16, "BD1 amplitude 2 out"=w2034:u16)  [unwired: 1 out]
    "MCL Scanning" <- w2228
    "Trap Pos FB Action" <- w2136
    n1617 = local read "Data points/scans (MCL)"() -> (w2052:dbl)
    n1618 = Decimate 1D Array(w2095) -> (w2163:u32[], w2053:u32[])
    n1619 = local read "DMA Update Period (s)"() -> (w2166:dbl)
    n1620 = To Double Precision Float(number=w2163) -> (double precision float=w2049:dbl[])
    n1621 = To Double Precision Float(number=w2053) -> (double precision float=w2050:dbl[])
    n1622 = Array Size(array=w2050) -> (size(s)=w2203:i32)
    n1623 = call "Ampint162Dbl.vi"("In i16"=w2032) -> ("Amp (%)"=w2031:dbl)  [unwired: 4 in]
    "Trap 1 amplitude" <- w2031
    n1624 = call "Ampint162Dbl.vi"("In i16"=w2034) -> ("Amp (%)"=w2033:dbl)  [unwired: 4 in]
    "Trap 2 amplitude" <- w2033
    n1625 = Build Array(w2049, w2050) -> (w2051:dbl[][])
    n1626 = local read "BD 1 Frq 1 (MHz)"() -> (w2075:dbl)
    n1627 = local read "BD 1 Frq 2 (MHz)"() -> (w2074:dbl)
    n1628 = local read "APD Integration Time (s)"() -> (w2081:dbl)
    n1629 = local read "MCL Scanning"() -> (w2195:bool)
    n1630 = Increment(x=w2052) -> (x+1=w2201:dbl)
    n1631 = local read "Data Period (s)"() -> (w2059:dbl)
    n1632 = local read "AI2 (V)"() -> (w2227:cluster{"Set 1":dbl, "Set 2":dbl})
    n1633 = Bundle By Name(cluster=w2227, "Set 1"=w2226, "Set 2"=w2225) -> (w2223:cluster{"Set 1":dbl, "Set 2":dbl})
    n1634 = feedback #8(w2201) -> (w2204:dbl)
    n1635 = Select(t=0, s=w2192, f=w2204) -> (s? t:f=w2198:dbl)
    n1636 = Add(x=w2203, y=w2198) -> (x+y=w2199:dbl)
    n1637 = Greater?(x=w2199, y=w2052) -> (0:w2200:bool)
    n1638 = feedback #9(0.0) -> (w2144:dbl)
    n1639 = Add(x=w2166, y=w2144) -> (x+y=w2219:dbl)
    n1640 = feedback-in #9(w2219) -> ()
    n1641 = Select(t=w2198, s=w2200, f=w2199) -> (s? t:f=w2197:dbl)
    n1642 = feedback-in #8(w2197) -> ()
    n1643 = Not(x=w2200) -> (.not. x?=w2194:bool)
    n1644 = To Time Stamp(1:w2144) -> (0:w2071:timestamp)
    n1645 = Build Array(w2075, w2074) -> (w2073:dbl[])
    n1646 = And(x=w2194, y=w2195) -> (x .and. y?=w2196:bool)
    n1647 = Or(x=w2196, y=w2192) -> (x .or. y?=w2193:bool)
    n1648 = Divide(x=w2223, y=3276.7) -> (x/y=w2222:cluster{"Set 1":dbl, "Set 2":dbl})
    n1649 = Multiply(x=w2059, y="Trap Disp. Downsample") -> (x*y=w2069:dbl)
    "Display Period (s)" <- w2069
    n1650 = call "TPosDSamp.vi"("TPos Data"=w2072, "Data Period (s)"=w2059, "TPos Disp. Dsamp"="Trap Disp. Downsample", "Time Stamp"=w2071, "Trap Pos"=w2073) -> ("TPos dSampd"=w2042:waveform(dbl)[])  [unwired: 14 in]
    n1651 = call "APDDSamp.vi"("APD Data"=w2051, "Data Period (s)"=w2081, "APD Disp. dSamp"="APD Disp. dSamp", "Time Stamp"=w2071) -> ("APD dSampd"=w2078:waveform(dbl)[])  [unwired: 15 in]
    n1652 = call "TrapDSamp.vi"("Trap Data"=w2082, "Data Period (s)"=w2059, "Trap Disp. dSamp"="Trap Disp. Downsample", "Time Stamp"=w2071, "Channel Names"=w2055) -> ("Trap dSampd"=w2084:waveform(dbl)[], "Trap Raw"=w2083:waveform(dbl)[])  [unwired: 13 in]
    n1653 = local read "Trap X (AI1)"() -> (w2143:T1)
    n1654 = Divide(x=w2136, y=327.67) -> (x/y=→"Action (%)":dbl)
    n1655 = Equal?(x="Tab Control Display", y=T3."FFT") -> (x = y?=w2057:bool)
    n1656 = local read "All FB On/Off"() -> (w2111:bool)
    n1657 = local write "AI2 (V)"(w2222) -> ()
    n1658 = Multiply(x=w2081, y="APD Disp. dSamp") -> (x*y=w2079:dbl)
    "APD Display Period (s)" <- w2079
    n1659 = Reciprocal(x=w2069) -> (1/x=→"Trap Disp. Freq. (Hz)":dbl)
    n1660 = case "Update MCL Scan Images" shown="True" w2193 {
      tunnel: w2192 -> [_ w2391]
      tunnel: w2049 -> [_ w2407]
      tunnel: w2083 -> [_ w2409]
      tunnel: w2050 -> [_ w2403]
      tunnel: w2149 -> [_ w2408]
      frame False {
      }
      frame True {
        n1661 = local read "Cycles/step (MCL)"() -> (w2392:u64)
        n1662 = local read "N APD Samp/step"() -> (w2404:i32)
        n1663 = Index Array(array=w2409, index=10) -> (element=w2412:waveform(dbl))
        n1664 = local read "Scan steps (x)"() -> (w2394:u64)
        n1665 = Index Array(array=w2409, index=11) -> (element=w2410:waveform(dbl))
        n1666 = local read "Scan lines (y)"() -> (w2393:u64)
        n1667 = Unbundle By Name(w2412) -> ("Y"=w2395:dbl[])
        n1668 = Unbundle By Name(w2410) -> ("Y"=w2396:dbl[])
        n1669 = Unbundle(w2408) -> ("New Image"=w2406:T4, "New Image"=w2402:T4, "New Image"=w2400:T4, "New Image"=w2397:T4)
        n1670 = call "MCLScanAPD.vi"("Image In"=w2406, "APD Cts"=w2407, "Scan steps (MCL)"=w2394, "Scan lines (y)"=w2393, "N APD Samp/step"=w2404, "NewScan?"=w2391) -> ("Image Out"=→"APD 1":T4)  [unwired: 13 in]
        n1671 = call "MCLScanAPD.vi"("Image In"=w2402, "APD Cts"=w2403, "Scan steps (MCL)"=w2394, "Scan lines (y)"=w2393, "N APD Samp/step"=w2404, "NewScan?"=w2391) -> ("Image Out"=→"APD 2":T4)  [unwired: 13 in]
        n1672 = call "MCLScanPSD.vi"("In Image"=w2397, "Trap Detector"=w2395, "Scan steps (x)"=w2394, "Scan lines (y)"=w2393, "Cycles/step (MCL)"=w2392, "NewScan?"=w2391) -> ("Out Image"=→"Detection Laser Y":T4)  [unwired: 13 in]
        n1673 = call "MCLScanPSD.vi"("In Image"=w2400, "Trap Detector"=w2396, "Scan steps (x)"=w2394, "Scan lines (y)"=w2393, "Cycles/step (MCL)"=w2392, "NewScan?"=w2391) -> ("Out Image"=→"Detection Laser X":T4)  [unwired: 13 in]
      }
    }
    n1674 = case "Display FFT" shown="True" w2057 {
      tunnel: w2083 -> [_ w2580]
      frame False {
      }
      frame True {
        n1675 = Array Size(array=w2580) -> (size(s)=w2579:i32)
        n1676 = Build Array("FFT 1 Choice 1", "FFT 1 Choice 2", "FFT 2 Choice 1", "FFT 2 Choice 2") -> (w2573:u16[])
        n1677 = feedback-in #10(w2573) -> ()
        n1678 = feedback #10(u16[] [100, 100, 100, 100]) -> (w2574:u16[])
        n1679 = feedback-in #11("# Spectra to Ave.") -> ()
        n1680 = feedback #11("# Spectra to Ave.") -> (w2571:dbl)
        n1681 = Not Equal?(x="# Spectra to Ave.", y=w2571) -> (x != y?=w2570:bool)
        n1682 = Not Equal?(x=w2573, y=w2574) -> (x != y?=w2572:bool)
        n1683 = feedback #12(1.0) -> (w2557:dbl)
        n1684 = Compound Arithmetic op=OR("Reset FFT", w2572, w2570) -> (w2555:bool)
        n1685 = Select(t=1.0, s=w2555, f=w2557) -> (s? t:f=w2559:dbl)
        n1686 = Greater?(x=w2559, y="# Spectra to Ave.") -> (0:w2578:bool)
        n1687 = Increment(x=w2559) -> (x+1=w2558:dbl)
        n1688 = feedback-in #12(w2558) -> ()
        n1689 = local read "DMA Update Period (s)"() -> (w2553:dbl)
        n1690 = Multiply(x="# Spectra to Ave.", y=w2553) -> (x*y=→"Ave. Time (s)":dbl)
        n1691 = Build Array(cluster{"f0":dbl, "df":dbl, "magnitude":dbl[]} {"f0"=0.0, "df"=0.0, "magnitude"=[]} ("PSD")) -> (w2562:cluster{"f0":dbl, "df":dbl, "magnitude":dbl[]}[])
        n1692 = Build Array(w2562, w2562, w2562, w2562) -> (w2564:T37)
        n1693 = feedback #13(w2564) -> (w2569:T37)
        n1694 = for {
          N: 4 -> [_]
          tunnel: w2573 -> [w2602] mode=indexing
          tunnel: w2580 -> [w2603]
          tunnel: w2579 -> [w2605]
          tunnel: w2555 -> [w2598]
          tunnel: w2578 -> [w2597]
          tunnel: "# Spectra to Ave." -> [w2596]
          tunnel: [w2595] -> w2568 mode=indexing
          tunnel: w2569 -> [w2600] mode=indexing
          tunnel: [w2599] -> w2556 mode=indexing
          tunnel: w2559 -> [w2594]
          n1695 = Less?(x=w2602, y=w2605) -> (x < y?=w2604:bool)
          n1696 = Index Array(array=w2603, index=w2602) -> (element=w2601:waveform(dbl))
          n1697 = case shown="True" w2604 {
            tunnel: w2601 -> [_ w2622]
            tunnel: w2600 -> [w2607 w2620]
            tunnel: [w2607 w2608] -> w2599
            tunnel: w2598 -> [_ w2619]
            tunnel: w2597 -> [_ w2612]
            tunnel: w2596 -> [_ w2611]
            tunnel: [cluster{"f0":dbl, "df":dbl, "magnitude":dbl[]} {"f0"=0.0, "df"=0.0, "magnitude"=[]} ("PSD") w2613] -> w2595
            tunnel: w2594 -> [_ w2610]
            frame False {
            }
            frame True {
              n1698 = call-poly <vilib>:"Mean.vi"("X"=w2622) -> ("mean"=w2623:dbl)  [unwired: 1 out]
              n1699 = Subtract(x=w2622, y=w2623) -> (x-y=w2621:waveform(dbl))
              n1700 = xnode ("Spectral Measurements")("Signals"=w2621) -> ("PSD"=w2615:cluster{"f0":dbl, "df":dbl, "magnitude":dbl[]})  [unwired: 1 in, 1 out]
              n1701 = case shown="False" w2619 {
                tunnel: w2620 -> [w2632 _]
                tunnel: [w2628 w2637] -> w2608
                tunnel: w2615 -> [w2631 w2638]
                tunnel: w2612 -> [w2630 _]
                frame False {
                  n1702 = Build Array (concatenate)(w2632, w2631) -> (w2629:cluster{"f0":dbl, "df":dbl, "magnitude":dbl[]}[])
                  n1703 = case shown="True" w2630 {
                    tunnel: w2629 -> [w2633 w2636]
                    tunnel: [w2633 w2634] -> w2628
                    frame False {
                    }
                    frame True {
                      n1704 = Delete From Array(array=w2636, index=0) -> (array with subset deleted=w2634:cluster{"f0":dbl, "df":dbl, "magnitude":dbl[]}[])  [unwired: 1 in, 1 out]
                    }
                  }
                }
                frame True {
                  n1705 = Build Array(w2638) -> (w2637:cluster{"f0":dbl, "df":dbl, "magnitude":dbl[]}[])
                }
              }
              n1706 = for {
                tunnel: w2608 -> [w2627] mode=indexing
                tunnel: [w2626] -> w2618 mode=indexing
                workers-P: _ -> [_]
                n1707 = Unbundle By Name(w2627) -> ("magnitude"=w2626:dbl[])
              }
              n1708 = Transpose 2D Array(2D array=w2618) -> (transposed array=w2617:dbl[][])
              n1709 = for {
                tunnel: w2617 -> [w2625] mode=indexing
                tunnel: [w2624] -> w2616 mode=indexing
                workers-P: _ -> [_]
                n1710 = Add Array Elements(numeric array=w2625) -> (sum=w2624:dbl)
              }
              n1711 = Select(t=w2611, s=w2612, f=w2610) -> (s? t:f=w2609:dbl)
              n1712 = Divide(x=w2616, y=w2609) -> (x/y=w2614:dbl[])
              n1713 = Bundle By Name(cluster=w2615, "magnitude"=w2614) -> (w2613:cluster{"f0":dbl, "df":dbl, "magnitude":dbl[]})
            }
          }
        }
        n1714 = case shown="True" w2555 {
          tunnel: w2556 -> [w2587 w2593]
          tunnel: [w2587 w2588] -> w2554
          frame False {
          }
          frame True {
            n1715 = Array Subset(array=w2593, index (row)=0 ("index"), length (row)=4 ("length"), index (col)=0 ("index"), length (col)=1 ("length")) -> (w2588:T37)
          }
        }
        n1716 = feedback-in #13(w2554) -> ()
        n1717 = Split 1D Array(array=w2568, index=2) -> (first subarray=→"FFT 1":cluster{"f0":dbl, "df":dbl, "magnitude":dbl[]}[], second subarray=→"FFT 2":cluster{"f0":dbl, "df":dbl, "magnitude":dbl[]}[])
      }
    }
    n1718 = Reciprocal(x=w2079) -> (1/x=→"APD Display Freq. (Hz)":dbl)
    n1719 = Bundle(cluster=w2143, "Trap 1"=w2139, "Trap 2"=w2138) -> (→"Trap X (AI1)":T1)
    n1720 = Divide(x=w2187, y=3276.7) -> (x/y=w2183:T38)
    n1721 = case "Turn off TPowFB if over 50%" shown="True" w2111 {
      tunnel: w2031 -> [_ w2299]
      tunnel: w2033 -> [_ w2298]
      frame False {
      }
      frame True {
        w2300 = ext 50.0
        n1722 = Greater?(x=w2299, y=w2300) -> (0:w2297:bool)
        n1723 = Greater?(x=w2298, y=w2300) -> (0:w2296:bool)
        n1724 = Or(x=w2297, y=w2296) -> (x .or. y?=w2295:bool)
        n1725 = case shown="True" w2295 {
          frame False {
          }
          frame True {
            n1726 = property on="All FB On/Off" class="Bool (strict)"("Val(Sgnl)"=FALSE) -> ()  [unwired: 2 in, 2 out]
            "Feedback overload" <- TRUE
          }
        }
      }
    }
    n1727 = Unbundle By Name(w2183) -> ("Green FB Ch 0"=w2186:dbl, "Green FB Ch 1"=w2185:dbl, "Green FB Ch 2"=w2184:dbl)
    n1728 = case "Get Offset" shown="True" "Use Full Offset?" {
      tunnel: [w2304 w2310] -> w2062
      tunnel: [w2303 w2309] -> w2065
      tunnel: w2115 -> [_ w2316]
      frame False {
        n1729 = Divide(x="T1 offset_x (mV)", y=1000.0) -> (x/y=w2304:dbl)
        n1730 = Divide(x="T2 offset_x (mV)", y=1000.0) -> (x/y=w2303:dbl)
      }
      frame True {
        n1731 = local read "Offset file step size"() -> (w2315:dbl)
        n1732 = local read "Offset Values"() -> (w2317:T14)
        n1733 = Unbundle By Name(w2317) -> ("Trap 1X offset"=w2312:dbl[], "Trap 2X offset"=w2311:dbl[])
        n1734 = Divide(x=w2316, y=w2315) -> (x/y=w2314:dbl)
        n1735 = To Long Integer(number=w2314) -> (32bit integer=w2313:i32)
        n1736 = Index Array(array=w2312, index=w2313) -> (element=w2310:dbl)
        n1737 = Index Array(array=w2311, index=w2313) -> (element=w2309:dbl)
      }
    }
    n1738 = Multiply(x=w2078, y="APD Disp. Scale") -> (x*y=w2077:waveform(dbl)[])
    n1739 = local read "APD Integration Time (s)"() -> (w2161:dbl)
    n1740 = Divide(x=w2186, y=w2184) -> (x/y=w2182:dbl)
    n1741 = Divide(x=w2185, y=w2184) -> (x/y=w2181:dbl)
    n1742 = Build Array (concatenate)(w2077, w2084) -> (w2159:waveform(dbl)[])
    "All Signals" <- w2159
    n1743 = Bundle By Name(cluster=w2183, "Green FB Ch 0"=w2182, "Green FB Ch 1"=w2181) -> (w2174:T38)
    "Green FB Signals (V)" <- w2174
    n1744 = Multiply(x="APD Disp. dSamp", y=w2161) -> (x*y=w2160:dbl)
    n1745 = Divide(x=w2078, y=w2160) -> (x/y=w2148:waveform(dbl)[])
    n1746 = Unbundle By Name(w2174) -> ("Green FB Ch 2"=→"Green FB Plot":dbl)
    n1747 = local read "Fish Status"() -> (w2109:u16)
    n1748 = Index Array(array=w2159, index=3) -> (element=w2056:waveform(dbl))
    n1749 = Index Array(array=w2159, index=6) -> (element=w2068:waveform(dbl))
    n1750 = local read "wait to reset values"() -> (w2231:bool)
    n1751 = Index Array(array=w2148, index=0) -> (element=w2156:waveform(dbl))
    n1752 = Index Array(array=w2148, index=1) -> (element=w2154:waveform(dbl))
    n1753 = Subtract(x=w2154, y="APD 2 Offset") -> (x-y=w2151:waveform(dbl))
    n1754 = Subtract(x=w2156, y="APD 1 Offset") -> (x-y=w2152:waveform(dbl))
    n1755 = Not(x=w2228) -> (.not. x?=w2232:bool)
    n1756 = Build Array(w2152, w2151) -> (→"APD Chart":waveform(dbl)[])
    n1757 = feedback-in #14("Calibration") -> ()
    n1758 = feedback #14(u16 1 ("Calibration")) -> (w2177:u16)
    n1759 = And(x=w2232, y=w2231) -> (x .and. y?=w2233:bool)
    n1760 = call "CalcForce.vi"("Trap 1X V"=w2056, "T1 alphaX (nm/V)"="T1 alpha_x (nm/V)", "T1 kappaX (pN/nm)"="T1 kappa_x (pN/nm)", "T1 offset X"=w2062, "Trap 2X V"=w2068, "Calibration"="Calibration", "T2 alphaX (nm/V)"="T2 alpha_x (nm/V)", "T2 kappaX (pN/nm)"="T2 kappa_x (pN/nm)", "T2 offsetX"=w2065) -> ("Force 1X"=w2036:waveform(dbl), "Force X"=w2041:waveform(dbl), "Force 2X"=w2035:waveform(dbl), "BeadDeflection"=w2047:waveform(dbl), "Out Names"=w2060:T39)  [unwired: 2 in]
    n1761 = Not Equal?(x=w2177, y="Calibration") -> (x != y?=w2164:bool)
    n1762 = case "Return MCL after MCL Raster" shown="True" w2233 {
      tunnel: w2236 -> [w2483 w2494]
      tunnel: [w2483 w2493] -> w2235
      tunnel: w2230 -> [w2482 w2492]
      tunnel: [w2482 w2491] -> w2229
      frame False {
      }
      frame True {
        n1763 = local read "Total Counts (ticks)"() -> (w2488:u32)
        n1764 = local read "Scan Range (V)\n(of steps)"() -> (w2489:dbl)
        n1765 = local read "MCL Y"() -> (w2487:dbl)
        n1766 = local read "MCL X"() -> (w2486:dbl)
        n1767 = local write "wait to reset values"(FALSE ("wait to reset values")) -> ()
        n1768 = call "V2int16.vi"("InV"=w2487) -> ("Out i16"=w2484:i16)  [unwired: 4 in]
        n1769 = call "V2int16.vi"("InV"=w2486) -> ("Out i16"=w2485:i16)  [unwired: 4 in]
        n1770 = xnode "Read/Write Control"("FPGA VI Reference In"=w2494, "error in"=w2492, "AO1 (Y)"=w2484, "AO2 (X)"=w2485, "MCL count"=w2488) -> ("FPGA VI Reference Out"=w2493:T20, "error out"=w2491:errorcluster)
        n1771 = property on="Scan Range (V)\n(of steps)" class="DigNum (strict)"("Val(Sgnl)"=w2489) -> ()  [unwired: 2 in, 2 out]
      }
    }
    n1772 = case "Update Graph Labels" shown="True" w2164 {
      tunnel: w2060 -> [_ w2390]
      frame False {
      }
      frame True {
        n1773 = Unbundle(w2390) -> ("Label.Text"=w2385:string, "Label.Text"=w2389:string, "Label.Text"=w2388:string, "Label.Text"=w2387:string, "Label.Text"=w2386:string)
        n1774 = property on="T1 X" class="DigNum (strict)"("Caption.Text"=w2385) -> ()  [unwired: 2 in, 2 out]
        n1775 = property on="T2 X" class="DigNum (strict)"("Caption.Text"=w2389) -> ()  [unwired: 2 in, 2 out]
        n1776 = property on="Force" class="WFChart (strict)"("YScale.NameLbl.Text"=w2388) -> ()  [unwired: 2 in, 2 out]
        n1777 = property on="Difference" class="DigNum (strict)"("Caption.Text"=w2387) -> ()  [unwired: 2 in, 2 out]
        n1778 = property on="Mean" class="DigNum (strict)"("Caption.Text"=w2386) -> ()  [unwired: 2 in, 2 out]
      }
    }
    n1779 = local read "Trap 2 Bead Size (nm)"() -> (w2126:dbl)
    n1780 = local read "Trap 1 Bead Size (nm)"() -> (w2125:dbl)
    n1781 = local read "AOM X Cal (nm/MHz)"() -> (w2043:dbl)
    n1782 = Add(x=w2126, y=w2125) -> (x+y=w2127:dbl)
    n1783 = Divide(x=w2127, y=2.0) -> (x/y=w2046:dbl)
    n1784 = Add(x=w2046, y="Ext Offset (nm)") -> (x+y=w2044:dbl)
    n1785 = call "CalcExtension.vi"("Offset"=w2044, "AOM X Cal"=w2043, "Trap Positions"=w2042, "BeadDeflection"=w2047) -> ("Extension"=w2040:waveform(dbl))  [unwired: 7 in]
    "Extension" <- w2040
    n1786 = Build Array(w2036, w2035, w2041) -> (→"Force":waveform(dbl)[])
    n1787 = Unbundle By Name(w2041) -> ("Y"=w2039:dbl[])
    n1788 = Unbundle By Name(w2040) -> ("Y"=w2038:dbl[])
    n1789 = Bundle("Y"=w2038, "Y"=w2039) -> (→"Force-Extension":cluster{"Y":dbl[], "Y":dbl[]})  [unwired: 1 in]
    n1790 = call-poly <vilib>:"Mean.vi"("X"=w2036) -> ("mean"=w2113:dbl)  [unwired: 1 out]
    "T1 X" <- w2113
    n1791 = call-poly <vilib>:"Mean.vi"("X"=w2035) -> ("mean"=w2112:dbl)  [unwired: 1 out]
    "T2 X" <- w2112
    n1792 = Subtract(x=w2113, y=w2112) -> (x-y=w2176:dbl)
    n1793 = Add(x=w2113, y=w2112) -> (x+y=→"Difference":dbl)
    n1794 = Divide(x=w2176, y=2.0) -> (x/y=w2110:dbl)
    "Mean" <- w2110
    n1795 = case "Autofishing" shown="False" "Toggle AFish" {
      tunnel: w2110 -> [w2248 _]
      tunnel: w2109 -> [w2247 w2291]
      frame False {
        n1796 = case "Autofishing - Alex" shown="1" w2247 {
          tunnel: w2248 -> [_ _ _ w2277 _]
          frame 0, Default {
            # "Off"
          }
          frame 1 {
            # "Approach"
            n1797 = local read "Trap Delta (MHz)"() -> (w2251:dbl)
            n1798 = Add(x=w2251, y="Approach dTD") -> (x+y=w2250:dbl)
            n1799 = In Range and Coerce(upper limit=inf, x=w2250, lower limit="Min TD") -> (coerced(x)=w2252:dbl, In Range?=w2253:bool)
            n1800 = case shown="False" w2253 {
              frame False {
                w2257 = u16 2 items=["Off", "Approach", "Wiggle", "Extend", "Tether Found"] ("Fish Status")
                n1801 = Tick Count (ms)() -> (millisecond timer value=→"AF Time":u32)
                n1802 = local write "Fish Status"(w2257) -> ()
              }
              frame True {
              }
            }
            n1803 = property on="Trap Delta (MHz)" class="DigNum (strict)"("Val(Sgnl)"=w2252) -> ()  [unwired: 2 in, 2 out]
          }
          frame 2 {
            # "Wiggle"
            n1804 = local read "AF Time"() -> (w2268:u32)
            n1805 = Random Number (0-1)() -> (number: 0 to 1=w2263:dbl)
            n1806 = Tick Count (ms)() -> (millisecond timer value=w2269:u32)
            n1807 = local read "Min TD"() -> (w2260:dbl)
            n1808 = Subtract(x=w2269, y=w2268) -> (x-y=w2267:u32)
            n1809 = Multiply(x=w2263, y="Wiggle TD") -> (x*y=w2261:dbl)
            n1810 = Divide(x=w2267, y=u32 1000) -> (x/y=w2265:dbl)
            n1811 = Add(x=w2261, y=w2260) -> (x+y=w2258:dbl)
            n1812 = Greater?(x=w2265, y="Wiggle time") -> (0:w2259:bool)
            n1813 = property on="Trap Delta (MHz)" class="DigNum (strict)"("Val(Sgnl)"=w2258) -> ()  [unwired: 2 in, 2 out]
            n1814 = case shown="True" w2259 {
              frame False {
              }
              frame True {
                w2270 = u16 3 items=["Off", "Approach", "Wiggle", "Extend", "Tether Found"] ("Fish Status")
                n1815 = local write "Fish Status"(w2270) -> ()
              }
            }
          }
          frame 3 {
            # "Extend"
            n1816 = local read "Trap Delta (MHz)"() -> (w2283:dbl)
            n1817 = Add(x=w2283, y="Extend dTD") -> (x+y=w2281:dbl)
            n1818 = In Range and Coerce(upper limit="Max TD", x=w2281, lower limit=0.0) -> (coerced(x)=w2272:dbl, In Range?=w2271:bool)
            n1819 = Greater?(x=w2272, y="Extend Min TD") -> (0:w2275:bool)
            n1820 = Greater?(x=w2277, y="Extend Min F") -> (0:w2276:bool)
            n1821 = property on="Trap Delta (MHz)" class="DigNum (strict)"("Val(Sgnl)"=w2272) -> ()  [unwired: 2 in, 2 out]
            n1822 = And(x=w2275, y=w2276) -> (x .and. y?=w2274:bool)
            n1823 = case shown="False" w2274 {
              tunnel: w2271 -> [w2284 _]
              frame False {
                n1824 = case shown="False" w2284 {
                  frame False {
                    w2285 = u16 1 items=["Off", "Approach", "Wiggle", "Extend", "Tether Found"] ("Fish Status")
                    n1825 = local write "Fish Status"(w2285) -> ()
                  }
                  frame True {
                  }
                }
              }
              frame True {
                w2286 = u16 4 items=["Off", "Approach", "Wiggle", "Extend", "Tether Found"] ("Fish Status")
                n1826 = local write "Fish Status"(w2286) -> ()
              }
            }
          }
          frame 4 {
            w2287 = u16 0 items=["Off", "Approach", "Wiggle", "Extend", "Tether Found"] ("Fish Status")
            n1827 = local write "Fish Status"(w2287) -> ()
            n1828 = call <vilib>:"Beep.vi"("use system alert? (T)"=FALSE, "duration (msec)"=u32 100, "frequency (Hz)"=u32 466) -> ()  [unwired: 9 in]
          }
        }
      }
      frame True {
        n1829 = case shown="0" w2291 {
          frame 0 {
            w2293 = u16 1 items=["Off", "Approach", "Wiggle", "Extend", "Tether Found"] ("Fish Status")
            n1830 = local write "Fish Status"(w2293) -> ()
          }
          frame Default {
            w2294 = u16 0 items=["Off", "Approach", "Wiggle", "Extend", "Tether Found"] ("Fish Status")
            n1831 = local write "Fish Status"(w2294) -> ()
          }
        }
        n1832 = local write "Toggle AFish"(FALSE ("Toggle AFish")) -> ()
      }
    }
    n1833 = node-c288() -> ()  [unwired: 2 out]
  }
  n1834 = timed-loop "Oscillate AOD (debugging)" {
    tunnel: w49 -> [w2917]
    tunnel: [w2916] -> w55
    timing: w88 -> [_]
    timing-out: [_] -> w87
    stop <- w2916 stop-if-true
    n1835 = node-c288() -> ()  [unwired: 2 out]
    n1836 = event shown="[0] \"Oscillate Set 2\", \"Fish for Tether\": Value Change" {
      selector: _ -> [_ _ _]
      dyn-events: _ -> [_ _ _]
      timeout: _ -> [_ _ _]
      tunnel: w2917 -> [w2924 _ _]
      tunnel: [FALSE ("Stop All") _ w3189] -> w2916
      event "Oscillate Set 2", "Fish for Tether": Value Change {
        n1837 = event-data() -> ()  [unwired: 6 out]
        n1838 = local read "Oscillate Set 2"() -> (w2923:bool)
        n1839 = Or(x=w2923, y="Fish for Tether") -> (x .or. y?=w2921:bool)
        n1840 = case shown="True" w2921 {
          tunnel: w2924 -> [_ w2927]
          tunnel: "Fish for Tether" -> [_ w2926]
          frame False {
          }
          frame True {
            n1841 = case shown="True" w2926 {
              frame False {
              }
              frame True {
                n1842 = local write "Scan axis 2"(TRUE) -> ()
                n1843 = local write "Tether"(FALSE ("Tether")) -> ()
              }
            }
            n1844 = node-c288("Period") -> (w2929:T21)  [unwired: 3 out]
            n1845 = timed-loop "Oscillate AOD" {
              timing: w2929 -> [_]
              timing-out: [_] -> w2928
              tunnel: w2927 -> [w2939]
              tunnel: w2926 -> [w2938]
              i -> [w2941]
              stop <- w2937 stop-if-true
              n1846 = node-c288() -> (w2940:i64)  [unwired: 1 out]
              n1847 = flat-sequence {
                tunnel: w2941 -> [w2967]
                tunnel: w2940 -> [w2966]
                tunnel: w2939 -> [w2950]
                tunnel: w2938 -> [w2952]
                tunnel: [w2952] -> w2936
                tunnel: [w2951] -> w2935
                tunnel: [w2949] -> w2934
                tunnel: [w2946] -> w2932
                tunnel: w2936 -> [w3002]
                tunnel: w2935 -> [w3000]
                tunnel: w2934 -> [w2999]
                tunnel: [w2998] -> w2933
                tunnel: w2932 -> [w2997]
                tunnel: [w3066] -> w2937
                tunnel: w2933 -> [w3064]
                frame #0 {
                  n1848 = Divide(x=w2966, y=i64 1000) -> (x/y=w2961:dbl)
                  n1849 = Multiply(x=w2961, y=w2967) -> (x*y=w2963:dbl)
                  n1850 = Multiply(x="Osc. freq. (Hz)", y=6.283185307179586) -> (x*y=w2964:dbl)
                  n1851 = Multiply(x=w2964, y=w2963) -> (x*y=w2948:dbl)
                  n1852 = local read "BD 1 Frq 2 (MHz)"() -> (w2945:dbl)
                  n1853 = local read "BD 1 Frq 1 (MHz)"() -> (w2942:dbl)
                  n1854 = case shown="True" w2952 {
                    tunnel: w2948 -> [w2973 w2982]
                    tunnel: w2945 -> [_ w2989]
                    tunnel: [w2970 w2976] -> w2953
                    tunnel: [FALSE w2974] -> w2949
                    tunnel: [0.0 w2978] -> w2946
                    tunnel: w2942 -> [_ w2977]
                    frame False {
                      n1855 = Sine(x=w2973) -> (sin(x)=w2971:dbl)
                      n1856 = Multiply(x=w2971, y="Osc. amp. (MHz)") -> (x*y=w2970:dbl)
                    }
                    frame True {
                      # "I BROKE IT - AT"
                      n1857 = Cosine(x=w2982) -> (cos(x)=w2992:dbl)
                      n1858 = Subtract(x=w2989, y=w2977) -> (x-y=w2988:dbl)
                      n1859 = Decrement(x=w2992) -> (x-1=w2991:dbl)
                      n1860 = Subtract(x=w2988, y="Closest Delta (MHz)") -> (x-y=w2985:dbl)
                      n1861 = Divide(x=w2991, y=2.0) -> (x/y=w2986:dbl)
                      n1862 = Multiply(x=w2986, y=w2985) -> (x*y=w2976:dbl)
                      n1863 = Greater?(x=0.0, y="Stop F (pN)") -> (0:w2974:bool)
                      n1864 = Divide(x=w2982, y=6.283185307179586) -> (x/y=w2981:dbl)
                      n1865 = Round Toward +Infinity(x=w2981) -> (ceil(x): smallest int >= x=w2978:dbl)
                      "Attempts" <- w2978
                      n1866 = Greater?(x=w2978, y="Attempt Limit") -> (0:w2980:bool)
                      n1867 = case shown="True" w2980 {
                        frame False {
                        }
                        frame True {
                          n1868 = local write "Fish for Tether"(FALSE ("Fish for Tether")) -> ()
                          n1869 = call <vilib>:"Beep.vi"() -> ()  [unwired: 3 in, 9 out]
                          n1870 = local read "Messages"() -> (w2994:string)
                          n1871 = call "Update messages.vi"("Message to add"="Tether fishing timeout." ("Messages"), "Old message string"=w2994) -> ("New message string"=→"Messages":string)
                        }
                      }
                    }
                  }
                  n1872 = local read "Y RF Frequency Limits (MHz)"() -> (w2954:T16)
                  n1873 = local read "X RF Frequency Limits (MHz)"() -> (w2955:T16)
                  n1874 = local read "BD 1 Frq 3 (MHz)"() -> (w2960:dbl)
                  n1875 = local read "BD 2 Frq 2 (MHz)"() -> (w2944:dbl)
                  n1876 = Select(t=w2945, s="Scan axis 2", f=w2944) -> (s? t:f=w2956:dbl)
                  n1877 = Add(x=w2953, y=w2956) -> (x+y=w2951:dbl)
                  n1878 = Select(t=w2951, s="Scan axis 2", f=w2945) -> (s? t:f=w2943:dbl)
                  n1879 = Select(t=w2944, s="Scan axis 2", f=w2951) -> (s? t:f=w2958:dbl)
                  n1880 = local read "BD 2 Frq 3 (MHz)"() -> (w2959:dbl)
                  n1881 = call "set RF board frequency - interlace.vi"("Board 2 Frequency Limits"=w2954, "Board 1 Frequency Limits"=w2955, "FPGA VI Reference In"=w2950, "Board 2 Frequency 3 (MHz)"=w2959, "Board 1 Frequency 3 (MHz)"=w2960, "Board 2 Frequency 2 (MHz)"=w2944, "Board 2 Frequency 1 (MHz)"=w2958, "Board 1 Frequency 2 (MHz)"=w2943, "Board 1 Frequency 1  (MHz)"=w2942) -> ()  [unwired: 1 in, 2 out]
                }
                frame #1 {
                  n1882 = And(x=w3002, y=w2999) -> (x .and. y?=w3001:bool)
                  n1883 = case "Only if were fishing and now formed tether" shown="True" w3001 {
                    tunnel: w3000 -> [w3004 w3016]
                    tunnel: [w3003 w3015] -> w2998
                    tunnel: w2997 -> [_ w3011]
                    frame False {
                      n1884 = local read "Fish for Tether"() -> (w3003:bool)
                      n1885 = case shown="True" w3003 {
                        tunnel: w3004 -> [_ _]
                        frame False {
                        }
                        frame True {
                        }
                      }
                    }
                    frame True {
                      w3015 = FALSE ("Fish for Tether")
                      n1886 = call <vilib>:"Beep.vi"() -> ()  [unwired: 3 in, 9 out]
                      n1887 = Number To Decimal String(number=w3011, width (-)=i16 1) -> (decimal integer string=w3009:string)
                      n1888 = case shown="\"2\", \"3\", \"4\", \"5\", \"6\"" "Then..." {
                        selector: "Then..." -> [_ w3019]
                        tunnel: w3016 -> [w3018 _]
                        frame "1", Default {
                          # "do nothing"
                          n1889 = property on="BD 1 Frq 1 (MHz)" class="DigNum (strict)"("Val(Sgnl)"=w3018) -> ()  [unwired: 2 in, 2 out]
                        }
                        frame "2", "3", "4", "5", "6" {
                          n1890 = flat-sequence {
                            tunnel: w3019 -> [w3021]
                            frame #0 {
                              n1891 = property on="Trap Delta (MHz)" class="DigNum (strict)"("Val(Sgnl)"="Move to Delta 1 (MHz)") -> ()  [unwired: 2 in, 2 out]
                            }
                            frame #1 {
                              n1892 = case shown="\"5\", \"6\"" w3021 {
                                selector: w3021 -> [w3024 w3034 _]
                                frame "3", "4" {
                                n1893 = flat-sequence {
                                tunnel: w3024 -> [w3025]
                                tunnel: [w3025] -> w3022
                                tunnel: [w3027] -> w3023
                                tunnel: w3022 -> [w3027]
                                tunnel: w3023 -> [w3031]
                                frame #0 {
                                n1894 = property on="Green Laser ON/Interlacing" class="Bool (strict)"("Val(Sgnl)"=TRUE ("Value (Signaling)")) -> ()  [unwired: 2 in, 2 out]
                                }
                                frame #1 {
                                n1895 = Multiply(x="Wait Before Save (s)", y=u32 1000 ("x")) -> (x*y=w3029:u32)
                                n1896 = Wait (ms)(milliseconds to wait=w3029) -> ()  [unwired: 1 out]
                                }
                                frame #2 {
                                n1897 = property on="Start Saving" class="Bool (strict)"("Value"=TRUE ("Start Saving")) -> ()  [unwired: 2 in, 2 out]
                                n1898 = case shown="Default" w3031 {
                                frame Default {
                                }
                                frame "4" {
                                n1899 = property on="Fl. Triggered..." class="Bool (strict)"("Val(Sgnl)"=TRUE ("Value (Signaling)")) -> ()  [unwired: 2 in, 2 out]
                                }
                                }
                                }
                                }
                                }
                                frame "5", "6" {
                                n1900 = stacked-sequence {
                                tunnel: w3034 -> [_ _ _ _ _ _ _ _ w3051 _ _]
                                frame #0 {
                                n1901 = Replace Array Subset(array=u32[] [0] ("Index Values"), new element="Raster Set Upon Tether", index=0) -> (w3035:u32[])
                                n1902 = property on="Saved AOD Raster Scan Parameter Sets" class="Arr (strict)"("Index Values"=w3035) -> ()  [unwired: 2 in, 2 out]
                                }
                                frame #1 {
                                n1903 = Wait (ms)(milliseconds to wait=u32 500) -> ()  [unwired: 1 out]
                                }
                                frame #2 {
                                n1904 = property on="Load parameters" class="Bool (strict)"("Val(Sgnl)"=TRUE ("Value (Signaling)")) -> ()  [unwired: 2 in, 2 out]
                                }
                                frame #3 {
                                n1905 = Wait (ms)(milliseconds to wait=u32 500) -> ()  [unwired: 1 out]
                                }
                                frame #4 {
                                n1906 = property on="Trap Raster Scan" class="Bool (strict)"("Val(Sgnl)"=TRUE ("Value (Signaling)")) -> ()  [unwired: 2 in, 2 out]
                                }
                                frame #5 {
                                n1907 = Wait (ms)(milliseconds to wait=u32 2000) -> ()  [unwired: 1 out]
                                }
                                frame #6 {
                                n1908 = while {
                                stop <- w3046 stop-if-true
                                n1909 = local read "Raster Scanning..."() -> (w3045:bool)
                                n1910 = local read "Saving..."() -> (w3048:bool)
                                n1911 = Wait (ms)(milliseconds to wait=u32 100) -> ()  [unwired: 1 out]
                                n1912 = Not(x=w3048) -> (.not. x?=w3047:bool)
                                n1913 = Not(x=w3045) -> (.not. x?=w3044:bool)
                                n1914 = And(x=w3047, y=w3044) -> (x .and. y?=w3046:bool)
                                }
                                }
                                frame #7 {
                                n1915 = property on="Trap Delta (MHz)" class="DigNum (strict)"("Val(Sgnl)"="Move to Delta 2 (MHz)") -> ()  [unwired: 2 in, 2 out]
                                }
                                frame #8 {
                                n1916 = local read "Tether"() -> (w3052:bool)
                                n1917 = case shown="True" w3052 {
                                tunnel: w3051 -> [_ w3053]
                                frame False {
                                }
                                frame True {
                                n1918 = flat-sequence {
                                tunnel: w3053 -> [w3055]
                                frame #0 {
                                n1919 = Wait (ms)(milliseconds to wait=u32 500) -> ()  [unwired: 1 out]
                                }
                                frame #1 {
                                n1920 = case shown="\"6\"" w3055 {
                                frame Default {
                                }
                                frame "6" {
                                n1921 = property on="Green Laser ON/Interlacing" class="Bool (strict)"("Val(Sgnl)"=TRUE ("Green Laser ON/Interlacing")) -> ()  [unwired: 2 in, 2 out]
                                }
                                }
                                }
                                frame #2 {
                                n1922 = Wait (ms)(milliseconds to wait=u32 500) -> ()  [unwired: 1 out]
                                }
                                frame #3 {
                                n1923 = local write "Start Saving"("Save at end (5, 6)") -> ()
                                }
                                }
                                }
                                }
                                }
                                frame #9 {
                                # "I BROKE IT - AT"
                                n1924 = Multiply(x=-1.0, y=1000.0) -> (x*y=w3061:dbl)
                                n1925 = Wait (ms)(milliseconds to wait=w3061) -> ()  [unwired: 1 out]
                                }
                                frame #10 {
                                n1926 = property on="Rescale on Mean" class="Bool (strict)"("Val(Sgnl)"=TRUE ("Value (Signaling)")) -> ()  [unwired: 2 in, 2 out]
                                }
                                }
                                }
                                frame "2", Default {
                                }
                              }
                            }
                          }
                        }
                      }
                      n1927 = Concatenate Strings("Formed tether in ", w3009, " attempt(s)." ("string")) -> (w3006:string)
                      n1928 = local read "Messages"() -> (w3013:string)
                      n1929 = local write "Fish for Tether"(w3015) -> ()
                      n1930 = call "Update messages.vi"("Message to add"=w3006, "Old message string"=w3013) -> ("New message string"=w3012:string)
                      n1931 = local write "Messages"(w3012) -> ()
                      n1932 = Get Date/Time In Seconds() -> (seconds since 1Jan1904=→"Time tether formed":timestamp)
                      "Tether" <- "Tether Alarm?"
                    }
                  }
                }
                frame #2 {
                  n1933 = local read "Oscillate Set 2"() -> (w3065:bool)
                  n1934 = local read "Stop All"() -> (w3067:bool)
                  n1935 = Not Or(1:w3064, 2:w3065) -> (0:w3063:bool)
                  n1936 = Compound Arithmetic op=OR(w3067, w3063) -> (w3066:bool)
                }
              }
              n1937 = node-c288() -> ()  [unwired: 2 out]
            }
            n1938 = node-c288(w2928) -> ()  [unwired: 1 out]
          }
        }
      }
      event "Fl. Triggered...": Value Change {
        n1939 = event-data() -> ()  [unwired: 7 out]
        n1940 = case shown="True" "Fl. Triggered..." {
          frame False {
          }
          frame True {
            n1941 = node-c288() -> (w3079:T21)  [unwired: 4 out]
            n1942 = timed-loop {
              timing: w3079 -> [_]
              timing-out: [_] -> w3078
              tunnel: "Action" -> [w3083]
              shift-right: [w3080] -> _
              shift-left: u8 255 -> [w3082]
              stop <- w3084 stop-if-true
              n1943 = node-c288() -> ()  [unwired: 2 out]
              n1944 = flat-sequence {
                tunnel: w3083 -> [w3095]
                tunnel: w3082 -> [w3092]
                tunnel: [w3091] -> w3081
                tunnel: [w3180] -> w3084
                tunnel: w3081 -> [w3179]
                tunnel: [w3179] -> w3080
                frame #0 {
                  w3085 = 1.0 ("t")
                  n1945 = Select(t=w3085, s="APD to Watch", f=w3085) -> (s? t:f=w3087:dbl)
                  n1946 = Multiply(x="Fl. Delta Thresh. (kHz)", y=1000.0) -> (x*y=w3094:dbl)
                  n1947 = Greater?(x=w3087, y=w3094) -> (0:w3089:bool)
                  n1948 = Or(x="Force Yank", y=w3089) -> (x .or. y?=w3090:bool)
                  n1949 = case shown="True" w3090 {
                    tunnel: w3095 -> [_ w3105]
                    tunnel: w3092 -> [w3097 w3101]
                    tunnel: [w3097 w3098] -> w3091
                    frame False {
                    }
                    frame True {
                      # "THIS IS NOW NOT WORKING BC I DELETED SOME THINGS - ALEX"
                      n1950 = flat-sequence {
                        tunnel: w3102 -> [w3111]
                        tunnel: [w3111] -> w3106
                        tunnel: w3105 -> [w3110]
                        tunnel: [w3110] -> w3104
                        tunnel: [w3109] -> w3103
                        tunnel: w3101 -> [w3108]
                        tunnel: [w3107] -> w3100
                        tunnel: w3106 -> [w3136]
                        tunnel: w3104 -> [w3135]
                        tunnel: w3103 -> [w3134]
                        tunnel: w3100 -> [w3133]
                        tunnel: [w3133] -> w3099
                        tunnel: w3099 -> [w3177]
                        tunnel: [w3177] -> w3098
                        frame #0 {
                          n1951 = call <vilib>:"Beep.vi"() -> ()  [unwired: 3 in, 9 out]
                          n1952 = local write "Waiting"(FALSE ("Waiting")) -> ()
                          n1953 = Increment(x=w3108) -> (x+1=w3107:u8)
                          n1954 = case shown="\"Yank\"" w3110 {
                            tunnel: w3107 -> [_ _ w3117]
                            frame "Image" {
                              n1955 = property on="Confocal Image" class="Bool (strict)"("Val(Sgnl)"=TRUE ("Value (Signaling)")) -> ()  [unwired: 2 in, 2 out]
                            }
                            frame "Alarm", Default {
                            }
                            frame "Yank" {
                              n1956 = flat-sequence {
                                tunnel: w3117 -> [w3120]
                                tunnel: [w3119] -> w3116
                                tunnel: ["N Array El"] -> w3115
                                tunnel: w3116 -> [w3130]
                                tunnel: w3115 -> [w3126]
                                frame #0 {
                                n1957 = Multiply(x="Yank Delay (s)", y=1000.0) -> (x*y=w3123:dbl)
                                n1958 = Quotient & Remainder(x=w3120, y="N Array El") -> (x-y*floor(x/y)=w3119:u8)  [unwired: 1 out]
                                n1959 = Wait (ms)(milliseconds to wait=w3123) -> ()  [unwired: 1 out]
                                }
                                frame #1 {
                                n1960 = Random Number (0-1)() -> (number: 0 to 1=w3127:dbl)
                                n1961 = Multiply(x=w3126, y=w3127) -> (x*y=w3125:dbl)
                                n1962 = Round Toward -Infinity(1:w3125) -> (0:w3124:dbl)
                                n1963 = Select(t=w3124, s="Random Choice", f=w3130) -> (s? t:f=w3128:dbl)
                                n1964 = Index Array(array="Yank to Delta Array (MHz)", index=w3128) -> (element=w3131:dbl)
                                n1965 = property on="Trap Delta (MHz)" class="DigNum (strict)"("Val(Sgnl)"=w3131) -> ()  [unwired: 2 in, 2 out]
                                }
                              }
                            }
                          }
                          n1966 = local read "Time (s)"() -> (w3109:dbl)
                          "Fl. High" <- TRUE ("Yanking")
                        }
                        frame #1 {
                          n1967 = node-c288() -> (w3138:T21)  [unwired: 4 out]
                          n1968 = timed-loop {
                            timing: w3138 -> [_]
                            timing-out: [_] -> w3137
                            tunnel: w3136 -> [w3153]
                            tunnel: w3135 -> [w3151]
                            tunnel: w3134 -> [w3150]
                            stop <- w3152 stop-if-true
                            w3139 = 1.0 ("t")
                            n1969 = node-c288() -> ()  [unwired: 2 out]
                            n1970 = local read "Fl. Delta Thresh. (kHz)"() -> (w3145:dbl)
                            n1971 = local read "Fl. Triggered..."() -> (w3154:bool)
                            n1972 = local read "Stop All"() -> (w3148:bool)
                            n1973 = local read "APD to Watch"() -> (w3141:bool)
                            n1974 = Select(t=w3139, s=w3141, f=w3139) -> (s? t:f=w3140:dbl)
                            n1975 = Not(x=w3154) -> (.not. x?=w3149:bool)
                            n1976 = Multiply(x=w3145, y=1000.0) -> (x*y=w3144:dbl)
                            n1977 = Negate(x=w3144) -> (-x=w3143:dbl)
                            n1978 = Less?(x=w3140, y=w3143) -> (x < y?=w3147:bool)
                            n1979 = Compound Arithmetic op=OR(w3147, w3148, w3149, "Force Reset") -> (w3152:bool)
                            n1980 = case shown="True" w3152 {
                              tunnel: w3153 -> [_ w3165]
                              tunnel: w3151 -> [_ w3164]
                              tunnel: w3150 -> [_ w3162]
                              frame False {
                              }
                              frame True {
                                n1981 = case shown="\"Yank\"" w3164 {
                                tunnel: w3165 -> [_ w3166]
                                frame "Image", Default {
                                }
                                frame "Yank" {
                                n1982 = flat-sequence {
                                tunnel: [w3171] -> w3167
                                tunnel: w3166 -> [w3171]
                                tunnel: w3167 -> [w3172]
                                frame #0 {
                                n1983 = local read "Yank Delay (s)"() -> (w3170:dbl)
                                n1984 = Multiply(x=w3170, y=1000.0) -> (x*y=w3168:dbl)
                                n1985 = Wait (ms)(milliseconds to wait=w3168) -> ()  [unwired: 1 out]
                                }
                                frame #1 {
                                n1986 = property on="Trap Delta (MHz)" class="DigNum (strict)"("Val(Sgnl)"=w3172) -> ()  [unwired: 2 in, 2 out]
                                }
                                }
                                }
                                }
                                n1987 = local read "Time (s)"() -> (w3163:dbl)
                                n1988 = Subtract(x=w3163, y=w3162) -> (x-y=w3159:dbl)
                                "Duration (s)" <- w3159
                                n1989 = Number To Decimal String(number=w3159, width (-)=i16 0) -> (decimal integer string=w3157:string)
                                n1990 = Concatenate Strings(w3157, " s fluorescence event." ("string")) -> (w3155:string)
                                n1991 = local read "Messages"() -> (w3161:string)
                                n1992 = call "Update messages.vi"("Message to add"=w3155, "Old message string"=w3161) -> ("New message string"=w3160:string)
                                n1993 = call <vilib>:"Beep.vi"() -> ()  [unwired: 3 in, 9 out]
                                n1994 = local write "Messages"(w3160) -> ()
                              }
                            }
                            n1995 = node-c288() -> ()  [unwired: 2 out]
                          }
                          n1996 = node-c288(w3137) -> ()  [unwired: 1 out]
                        }
                        frame #2 {
                          n1997 = local write "Fl. High"(FALSE ("Yanking")) -> ()
                        }
                      }
                      n1998 = local read "Trap Delta (MHz)"() -> (w3102:dbl)
                    }
                  }
                }
                frame #1 {
                  n1999 = local read "Stop All"() -> (w3183:bool)
                  n2000 = local read "Fl. Triggered..."() -> (w3181:bool)
                  n2001 = Not(x=w3181) -> (.not. x?=w3182:bool)
                  n2002 = Or(x=w3182, y=w3183) -> (x .or. y?=w3180:bool)
                  n2003 = Not(x=w3180) -> (.not. x?=→"Waiting":bool)
                }
              }
              n2004 = node-c288() -> ()  [unwired: 2 out]
            }
            n2005 = node-c288(w3078) -> ()  [unwired: 1 out]
          }
        }
      }
      event "Stop All": Value Change {
        n2006 = event-data() -> ()  [unwired: 7 out]
        n2007 = local read "Stop All"() -> (w3189:bool)
      }
    }
    n2008 = node-c288() -> ()  [unwired: 2 out]
  }
  n2009 = node-c288(w41) -> ()  [unwired: 1 out]
  n2010 = node-c288(w87) -> ()  [unwired: 1 out]
  n2011 = node-c288(w169) -> ()  [unwired: 1 out]
  n2012 = flat-sequence "@Alex - Set stage to 0,0,0 on exit" {
    tunnel: w11 -> [w3191]
    tunnel: [w3190] -> w10
    frame #0 {
      n2013 = local read "ESP Port"() -> (w3195:refnum<visa-resource-name>)
      n2014 = Concatenate Strings("1PA0;\n2PA0;\n3PA0" ("write buffer"), "\r") -> (w3192:string)
      n2015 = VISA Write(VISA resource name=w3195, write buffer=w3192, error in (no error)=w3191) -> (error out=w3190:errorcluster)  [unwired: 2 out]
    }
  }
  n2016 = flat-sequence {
    tunnel: w52 -> [w3200]
    tunnel: [w3199] -> w58
    tunnel: [w3196] -> w57
    tunnel: w56 -> [_]
    tunnel: w55 -> [_]
    tunnel: w54 -> [_]
    tunnel: w53 -> [_]
    tunnel: w10 -> [w3197]
    tunnel: w58 -> [w3203]
    tunnel: w57 -> [w3202]
    frame #0 {
      w3198 = FALSE ("APD to FIFO")
      n2017 = xnode "Read/Write Control"("FPGA VI Reference In"=w3200, "error in"=w3197, "APD to FIFO"=w3198, "AI to FIFO"=w3198) -> ("FPGA VI Reference Out"=w3199:T20, "error out"=w3196:errorcluster)
    }
    frame #1 {
      n2018 = xnode "Invoke Method"("FPGA VI Reference In"=w3203, "error in"=w3202) -> ("FPGA VI Reference Out"=w3201:T20)  [unwired: 1 out]
      n2019 = xnode "Close FPGA VI Reference"("FPGA VI Reference In"=w3201) -> ()  [unwired: 1 in, 1 out]
    }
  }
  "Fish Status" <- w9
